vi "Lab Panel V4.7.vi"() -> ()   [LabVIEW 2013]
uses:
  <vilib>/Platform/TimedLoop/XDataNode/timing_clust.ctl
  <vilib>/Platform/TimedLoop/XDataNode/nitl_modes.ctl
  <vilib>/Platform/TimedLoop/XDataNode/wakeup.ctl
  Global 1.vi
  <vilib>/platform/TimedLoop/XDataNode/XDataNode.xnode
  <vilib>/Platform/TimedLoop/XDataNode/XDNodeRunTimeDep.lvlib
panel:
  in  "ADMIN PAGE":bool
  out "TEMP update":bool
  out "AI update":bool
  in  "Tab Control 2":T1(tab)
  out "SIG LAB05-2":T2 {"PF" format="%.2f"; "AMPS" format="%.1f"}
  out "SIG LAB05-1":T2 {"PF" format="%.2f"; "AMPS" format="%.1f"}
  out "SIG LAB04-2":T2 {"PF" format="%.2f"; "AMPS" format="%.1f"}
  out "SIG LAB04-1":T2 {"PF" format="%.2f"; "AMPS" format="%.1f"}
  out "SIG LAB03-2":T2 {"PF" format="%.2f"; "AMPS" format="%.1f"}
  out "SIG LAB03-1":T2 {"PF" format="%.2f"; "AMPS" format="%.1f"}
  out "SIG LAB02-2":T2 {"PF" format="%.2f"; "AMPS" format="%.1f"}
  in  "RUN LAB01-1":bool
  in  "O/I  LAB05-1":bool
  in  "O/I  LAB05-2":bool
  in  "O/I  LAB04-1":bool
  in  "O/I  LAB04-2":bool
  in  "O/I  LAB02-1":bool
  in  "O/I  LAB02-2":bool
  in  "O/I  LAB01-2":bool
  in  "O/I  LAB01-1":bool
  in  "O/I  LAB03-1":bool
  in  "RUN LAB05-2":bool
  in  "RUN LAB05-1":bool
  in  "RUN LAB04-2":bool
  in  "RUN LAB04-1":bool
  in  "RUN LAB03-2":bool
  in  "RUN LAB03-1":bool
  in  "RUN LAB02-2":bool
  in  "RUN LAB02-1":bool
  in  "RUN LAB01-2":bool
  in  "SELECT LAB05-2":T3(radio)
  in  "SELECT LAB05-1":T3(radio)
  in  "SELECT LAB04-2":T3(radio)
  in  "SELECT LAB04-1":T3(radio)
  in  "SELECT LAB03-2":T3(radio)
  in  "SELECT LAB03-1":T3(radio)
  in  "SELECT LAB02-2":T3(radio)
  in  "SELECT LAB02-1":T3(radio)
  in  "SELECT LAB01-2":T3(radio)
  in  "SELECT LAB01-1":T3(radio)
  in  "O/I  LAB03-2":bool
  out "SIG LAB01-1":T2 {"PF" format="%.2f"; "AMPS" format="%.1f"}
  out "SIG LAB01-2":T2 {"PF" format="%.2f"; "AMPS" format="%.1f"}
  out "SIG LAB02-1":T2 {"PF" format="%.2f"; "AMPS" format="%.1f"}
  out "DISP LAB05-2":T4 {"MINS" format="%.2g"}
  out "DISP LAB05-1":T4 {"MINS" format="%.2g"}
  out "DISP LAB04-2":T4 {"MINS" format="%.2g"}
  out "DISP LAB04-1":T4 {"MINS" format="%.2g"}
  out "DISP LAB03-2":T4 {"MINS" format="%.2g"}
  out "DISP LAB03-1":T4 {"MINS" format="%.2g"}
  in  "SET LAB05-2":T5={"NAME"="", "DESCRIPTION"="", "CYCLES"=5.0, "T-RISE mins"=0.0, "T-RISE deg C"=0.0} {"CYCLES" min=5.0 step=1.0}
  in  "SET LAB05-1":T5={"NAME"="", "DESCRIPTION"="", "CYCLES"=5.0, "T-RISE mins"=0.0, "T-RISE deg C"=0.0} {"CYCLES" min=5.0 step=1.0}
  in  "SET LAB04-2":T5={"NAME"="", "DESCRIPTION"="", "CYCLES"=5.0, "T-RISE mins"=0.0, "T-RISE deg C"=0.0} {"CYCLES" min=5.0 step=1.0}
  in  "SET LAB04-1":T5={"NAME"="", "DESCRIPTION"="", "CYCLES"=5.0, "T-RISE mins"=0.0, "T-RISE deg C"=0.0} {"CYCLES" min=5.0 step=1.0}
  in  "SET LAB03-2":T5={"NAME"="", "DESCRIPTION"="", "CYCLES"=5.0, "T-RISE mins"=0.0, "T-RISE deg C"=0.0} {"CYCLES" min=5.0 step=1.0}
  in  "SET LAB03-1":T5={"NAME"="", "DESCRIPTION"="", "CYCLES"=5.0, "T-RISE mins"=0.0, "T-RISE deg C"=0.0} {"CYCLES" min=5.0 step=1.0}
  out "DISP LAB02-2":T4 {"MINS" format="%.2g"}
  out "DISP LAB02-1":T4 {"MINS" format="%.2g"}
  in  "SET LAB02-2":T5={"NAME"="", "DESCRIPTION"="", "CYCLES"=5.0, "T-RISE mins"=0.0, "T-RISE deg C"=0.0} {"CYCLES" min=5.0 step=1.0}
  in  "SET LAB02-1":T5={"NAME"="", "DESCRIPTION"="", "CYCLES"=5.0, "T-RISE mins"=0.0, "T-RISE deg C"=0.0} {"CYCLES" min=5.0 step=1.0}
  out "RESULT LAB05-2":bool
  out "RESULT LAB05-1":bool
  out "RESULT LAB04-2":bool
  out "RESULT LAB04-1":bool
  out "RESULT LAB03-2":bool
  out "RESULT LAB03-1":bool
  out "RESULT LAB02-2":bool
  out "RESULT LAB02-1":bool
  out "RESULT LAB01-2":bool
  out "RESULT LAB01-1":bool
  in  "SET LAB01-1":T5={"NAME"="", "DESCRIPTION"="", "CYCLES"=5.0, "T-RISE mins"=0.0, "T-RISE deg C"=0.0} {"CYCLES" min=5.0 step=1.0}
  in  "SET LAB01-2":T5={"NAME"="", "DESCRIPTION"="", "CYCLES"=5.0, "T-RISE mins"=0.0, "T-RISE deg C"=0.0} {"CYCLES" min=5.0 step=1.0}
  out "DISP LAB01-1":T4 {"MINS" format="%.2g"}
  out "DISP LAB01-2":T4 {"MINS" format="%.2f"}
  out "TEMP RISE LAB05-2":cluster{"TL":dbl, "TN":dbl}
  out "TEMP RISE LAB05-1":cluster{"TL":dbl, "TN":dbl}
  out "TEMP RISE LAB04-2":cluster{"TL":dbl, "TN":dbl}
  out "TEMP RISE LAB04-1":cluster{"TL":dbl, "TN":dbl}
  out "TEMP RISE LAB03-2":cluster{"TL":dbl, "TN":dbl}
  out "TEMP RISE LAB03-1":cluster{"TL":dbl, "TN":dbl}
  out "TEMP RISE LAB02-2":cluster{"TL":dbl, "TN":dbl}
  out "TEMP RISE LAB02-1":cluster{"TL":dbl, "TN":dbl}
  out "TEMP RISE LAB01-2":cluster{"TL":dbl, "TN":dbl}
  out "TEMP RISE LAB01-1":cluster{"TL":dbl, "TN":dbl}
  in  "JIG OFF TIME (S)":dbl=2.0 min=2.0 max=10.0 step=0.5 format="%.1g"
  in  "JIG ON TIME (S)":dbl=1.0 min=1.0 max=10.0 step=0.5 format="%.1g"
  out "JIG LAB05-2":bool
  out "JIG LAB05-1":bool
  out "JIG LAB04-2":bool
  out "JIG LAB04-1":bool
  out "JIG LAB03-2":bool
  out "JIG LAB03-1":bool
  out "JIG LAB02-2":bool
  out "JIG LAB02-1":bool
  out "JIG LAB01-2":bool
  out "JIG LAB01-1":bool
  out "TEMP START LAB01-1":cluster{"TL":dbl, "TN":dbl}
  out "TEMP START LAB02-1":cluster{"TL":dbl, "TN":dbl}
  out "TEMP START LAB03-1":cluster{"TL":dbl, "TN":dbl}
  out "TEMP START LAB04-1":cluster{"TL":dbl, "TN":dbl}
  out "TEMP START LAB01-2":cluster{"TL":dbl, "TN":dbl}
  out "TEMP START LAB02-2":cluster{"TL":dbl, "TN":dbl}
  out "TEMP START LAB03-2":cluster{"TL":dbl, "TN":dbl}
  out "TEMP START LAB04-2":cluster{"TL":dbl, "TN":dbl}
  out "TEMP START LAB05-2":cluster{"TL":dbl, "TN":dbl}
  out "TEMP START LAB05-1":cluster{"TL":dbl, "TN":dbl}
  out "TEST VOLTS CHART":T6(graph)
  in  "Select  Cycle":enum32{"ON CYCLE", "OFF CYCLE"}(radio)
  out "TEST AMPS CHART":T6(graph)
  out "TEMPERATURE (N) CHART":T6(graph)
  out "TEMPERATURE (L) CHART":T6(graph)
  out "Message":string
  in  "MAIL SETTINGS":T7
  out "MAIL REPORT":string
  in  "TO (string):":string
  in  "Send Mail Now":bool
  in  "Auto Mail Send":bool
  in  "Network Directory":path
  out "CAL LAB01":T8 {"2 (TN) cal" min=0.0 step=0.01 format="%.2f"; "2 (TL) cal" min=0.0 step=0.01 format="%.2f"; "2 (PF) cal" min=0.0 step=0.01 format="%.2f"; "2 (V) cal" min=0.0 step=0.01 format="%.2f"; "2 (A) cal" min=0.0 step=0.01 format="%.2f"; "1 (TN) cal" min=0.0 step=0.01 format="%.2f"; "1 (TL) cal" min=0.0 step=0.01 format="%.2f"; "1 (PF) cal" min=0.0 step=0.01 format="%.2f"; "1 (V) cal" min=0.0 step=0.01 format="%.2f"; "1  (A) cal" min=0.0 step=0.01 format="%.2f"}
  out "CAL LAB03":T8 {"2 (TN) cal" min=0.0 step=0.01 format="%.2f"; "2 (TL) cal" min=0.0 step=0.01 format="%.2f"; "2 (PF) cal" min=0.0 step=0.01 format="%.2f"; "2 (V) cal" min=0.0 step=0.01 format="%.2f"; "2 (A) cal" min=0.0 step=0.01 format="%.2f"; "1 (TN) cal" min=0.0 step=0.01 format="%.2f"; "1 (TL) cal" min=0.0 step=0.01 format="%.2f"; "1 (PF) cal" min=0.0 step=0.01 format="%.2f"; "1 (V) cal" min=0.0 step=0.01 format="%.2f"; "1  (A) cal" min=0.0 step=0.01 format="%.2f"}
  out "CAL LAB02":T9 {"2 (TN) cal" min=0.0 step=0.01 format="%.2f"; "2 (TL) cal" min=0.0 step=0.01 format="%.2f"; "2 (PF) cal" min=0.0 step=0.01 format="%.2f"; "2 (V) cal" min=0.0 step=0.01 format="%.2f"; "2 (A) cal" min=0.0 step=0.01 format="%.2f"; "1 (TN) cal" min=0.0 step=0.01 format="%.2f"; "1 (TL) cal" min=0.0 step=0.01 format="%.2f"; "1 (PF) cal" min=0.0 step=0.01 format="%.2f"; "1 (V) cal" min=0.0 step=0.01 format="%.2f"; "1 (A) cal" min=0.0 step=0.01 format="%.2f"}
  out "CAL LAB05":T8 {"2 (TN) cal" min=0.0 step=0.01 format="%.2f"; "2 (TL) cal" min=0.0 step=0.01 format="%.2f"; "2 (PF) cal" min=0.0 step=0.01 format="%.2f"; "2 (V) cal" min=0.0 step=0.01 format="%.2f"; "2 (A) cal" min=0.0 step=0.01 format="%.2f"; "1 (TN) cal" min=0.0 step=0.01 format="%.2f"; "1 (TL) cal" min=0.0 step=0.01 format="%.2f"; "1 (PF) cal" min=0.0 step=0.01 format="%.2f"; "1 (V) cal" min=0.0 step=0.01 format="%.2f"; "1  (A) cal" min=0.0 step=0.01 format="%.2f"}
  out "CAL LAB04":T8 {"2 (TN) cal" min=0.0 step=0.01 format="%.2f"; "2 (TL) cal" min=0.0 step=0.01 format="%.2f"; "2 (PF) cal" min=0.0 step=0.01 format="%.2f"; "2 (V) cal" min=0.0 step=0.01 format="%.2f"; "2 (A) cal" min=0.0 step=0.01 format="%.2f"; "1 (TN) cal" min=0.0 step=0.01 format="%.2f"; "1 (TL) cal" min=0.0 step=0.01 format="%.2f"; "1 (PF) cal" min=0.0 step=0.01 format="%.2f"; "1 (V) cal" min=0.0 step=0.01 format="%.2f"; "1  (A) cal" min=0.0 step=0.01 format="%.2f"}
  out "calibration file error out":errorcluster
  in  "CALIBRATE":bool
  out "ON L05-2":cluster{"amps":dbl, "volts":dbl, "pf":dbl}
  out "ON L05-1":cluster{"amps":dbl, "volts":dbl, "pf":dbl}
  out "FAIL LAB05-2":cluster{"LO":dbl, "HI":dbl}
  out "FAIL LAB05-1":cluster{"LO":dbl, "HI":dbl}
  out "FAIL LAB04-2":cluster{"LO":dbl, "HI":dbl}
  out "FAIL LAB04-1":cluster{"LO":dbl, "HI":dbl}
  out "FAIL LAB03-2":cluster{"LO":dbl, "HI":dbl}
  out "FAIL LAB03-1":cluster{"LO":dbl, "HI":dbl}
  out "FAIL LAB02-2":cluster{"LO":dbl, "HI":dbl}
  out "FAIL LAB02-1":cluster{"LO":dbl, "HI":dbl}
  out "FAIL LAB01-2":cluster{"LO":dbl, "HI":dbl}
  out "FAIL LAB01-1":cluster{"LO":dbl, "HI":dbl}
  out "ON L01-1":cluster{"amps":dbl, "volts":dbl, "pf":dbl}
  out "ON L01-2":cluster{"amps":dbl, "volts":dbl, "pf":dbl}
  out "ON L02-1":cluster{"amps":dbl, "volts":dbl, "pf":dbl}
  out "ON L02-2":cluster{"amps":dbl, "volts":dbl, "pf":dbl}
  out "ON L03-1":cluster{"amps":dbl, "volts":dbl, "pf":dbl}
  out "ON L03-2":cluster{"amps":dbl, "volts":dbl, "pf":dbl}
  out "ON L04-1":cluster{"amps":dbl, "volts":dbl, "pf":dbl}
  out "ON L04-2":cluster{"amps":dbl, "volts":dbl, "pf":dbl}
  out "TEMP LA05":T10
  out "TEMP LA04":T10
  out "TEMP LA03":T10
  out "TEMP LA02":T10
  out "TEMP LA01":T10
  in  "Temp Value":dbl
  in  "Temp Delay Lps":dbl
  in  "SAMPLES":dbl
  in  "RATE (Hz)":dbl
  in  "JIG TEST":T11
  in  "C drive data root dir":path
  out "run lab05-2":bool
  out "run lab05-1":bool
  out "run lab04-2":bool
  out "run lab04-1":bool
  out "run lab03-2":bool
  out "run lab03-1":bool
  out "run lab02-2":bool
  out "run lab02-1":bool
  out "run lab01-2":bool
  out "run lab01-1":bool
  out "stop2":bool
  in  "Tab Control":T12(tab)
  out "LAB01-2 (GRAPH)":dynamicdata(graph)
  out "LAB01-1 (GRAPH)":dynamicdata(graph)
  out "LAB02-2 (GRAPH)":dynamicdata(graph)
  out "LAB02-1 (GRAPH)":dynamicdata(graph)
  out "LAB03-2 (GRAPH)":dynamicdata(graph)
  out "LAB03-1 (GRAPH)":dynamicdata(graph)
  out "LAB04-2 (GRAPH)":dynamicdata(graph)
  out "LAB04-1 (GRAPH)":dynamicdata(graph)
  out "LAB05-2 (GRAPH)":dynamicdata(graph)
  out "LAB05-1 (GRAPH)":dynamicdata(graph)
  out "LAB05 TEMP":T13
  out "LAB04 TEMP":T13
  out "LAB02 TEMP":T13
  out "LAB01 TEMP":T13
  out "LAB03 TEMP":T13
  out "Analog Error Array":errorcluster[](array[cluster])
  out "AI loop time":dbl format="%.6g"
  out "loops":dbl
  in  "loop  delay(mS)":dbl
  out "on loops":dbl
  out "off loops":dbl
  out "jig cycle":dbl
  out "TDMS LAB01-1":refnum<k34>
  out "data file error":errorcluster
  out "TDMS LAB02-1":refnum<k34>
  out "TDMS LAB01-2":refnum<k34>
  out "TDMS LAB02-2":refnum<k34>
  out "TDMS LAB03-1":refnum<k34>
  out "TDMS LAB03-2":refnum<k34>
  out "TDMS LAB04-1":refnum<k34>
  out "TDMS LAB04-2":refnum<k34>
  out "TDMS LAB05-1":refnum<k34>
  out "TDMS LAB05-2":refnum<k34>
  out "mail control":string
  out "File Time Stamp":timestamp
  in  "stop":bool
  in  "Select COM port":refnum<visa-resource-name>="COM6"
  out "COM port":refnum<visa-resource-name>="COM6"
  # "LAB01"
  # "LAB02"
  # "LAB05"
  # "LAB03"
  # "LAB04"
  # "LAB01"
  # "LAB02"
  # "LAB03"
  # "LAB04"
  # "LAB05"
  # "JIG SET"
  # "(Enter recipients address seperated by comma)"
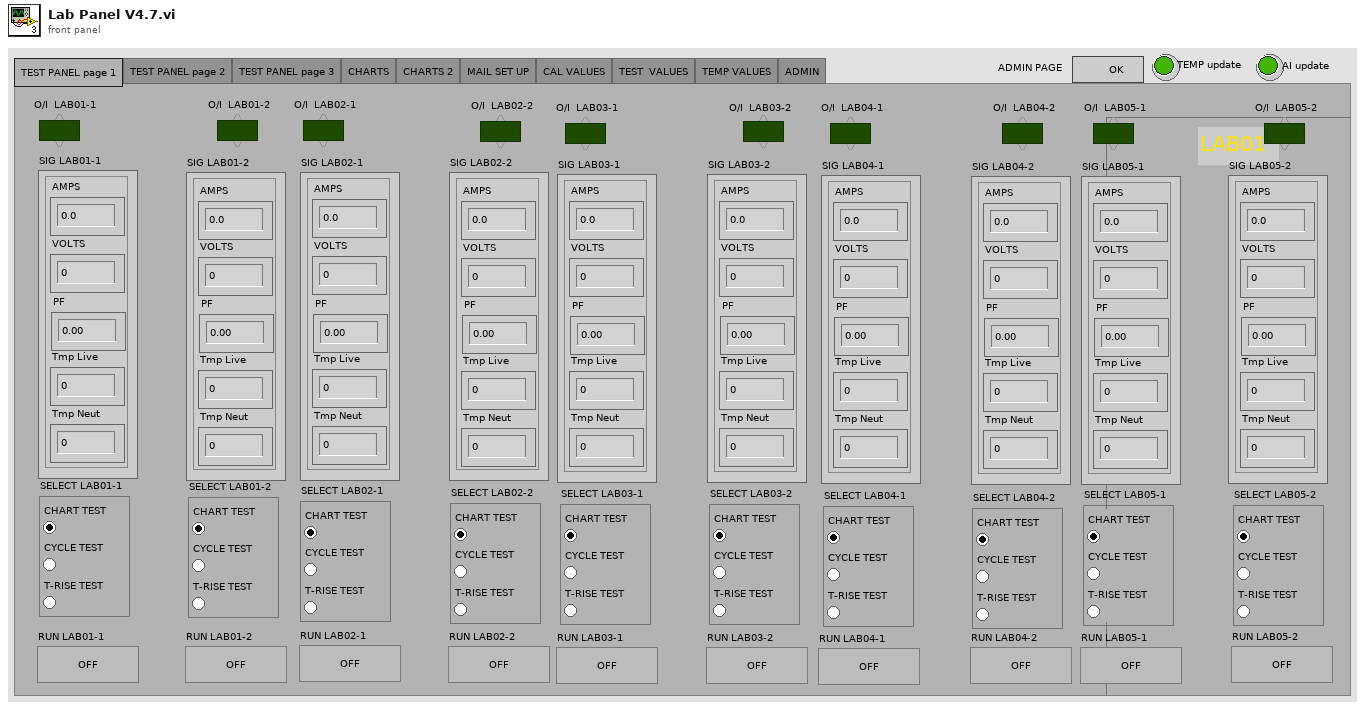
[diagram p1: front panel]
types:
  T1 = enum32{"TEST PANEL page 1", "TEST PANEL page 2", "TEST PANEL page 3", "CHARTS", "CHARTS 2", "MAIL SET UP", "CAL VALUES", "TEST  VALUES", "TEMP VALUES", "ADMIN"}
  T2 = cluster{"AMPS":dbl, "VOLTS":dbl, "PF":dbl, "Tmp Live":dbl, "Tmp Neut":dbl}
  T3 = enum32{"CHART TEST", "CYCLE TEST", "T-RISE TEST"}
  T4 = cluster{"CYCLE":dbl, "MINS":dbl, "STATUS":string}
  T5 = cluster{"NAME":string, "DESCRIPTION":string, "CYCLES":dbl, "T-RISE mins":dbl, "T-RISE deg C":dbl}
  T6 = cluster{"AMPS":dbl, "AMPS":dbl, "AMPS":dbl, "AMPS":dbl, "AMPS":dbl, "AMPS":dbl, "AMPS":dbl, "AMPS":dbl, "AMPS":dbl, "AMPS":dbl}
  T7 = cluster{"OUT SERVER ADDRESS":string, "FROM ACCOUNT":string, "USER NAME":string, "PASSWORD":string, "TEST MAIL":bool, "TEST MAIL STATUS":string, "mail error":errorcluster}
  T8 = cluster{"1  (A) cal":dbl, "1 (V) cal":dbl, "1 (PF) cal":dbl, "1 (TL) cal":dbl, "1 (TN) cal":dbl, "2 (A) cal":dbl, "2 (V) cal":dbl, "2 (PF) cal":dbl, "2 (TL) cal":dbl, "2 (TN) cal":dbl}
  T9 = cluster{"1 (A) cal":dbl, "1 (V) cal":dbl, "1 (PF) cal":dbl, "1 (TL) cal":dbl, "1 (TN) cal":dbl, "2 (A) cal":dbl, "2 (V) cal":dbl, "2 (PF) cal":dbl, "2 (TL) cal":dbl, "2 (TN) cal":dbl}
  T10 = cluster{"TL-1":dbl, "TN-1":dbl, "TL-2":dbl, "TN-2":dbl, "TL -1COUNT":dbl, "TN-1 COUNT":dbl, "TL-2 COUNT":dbl, "TN-2 COUNT":dbl}
  T11 = cluster{" LAB01-1":bool, " LAB01-2":bool, "LAB02-1":bool, " LAB02-2":bool, "LAB03-1":bool, "LAB03-2":bool, "LAB04-1":bool, "LAB04-2":bool, "LAB05-1":bool, "LAB05-2":bool}
  T12 = enum32{"LAB01", "LAB02", "LAB03", "LAB04", "LAB05", "TEMPERATURE", "ERROR"}
  T13 = cluster{"T1 Live":dbl, "T1 Neut":dbl, "T2 Live":dbl, "T2 Neut":dbl, "ID":dbl, "ER":dbl}
  T14 = enum8{"Enabled", "Disabled", "Disabled and Grayed Out"}
  T15 = typedef "XDNodeRunTimeDep.lvlib/timing_clust.ctl" = cluster{"Expected End [f-1]":u64, "Actual End [f-1]":u64, "Finished Late? [f-1]":bool, "Expected End [i-1]":u64, "Actual End [i-1]":u64, "Finished Late? [i-1]":bool, "Expected Start [i]":u64, "Actual Start [i]":u64, "Expected Start [f]":u64, "Actual Start [f]":u64, "Source Name":string, "Structure Name":string, "Period":i64, "Deadline":i64, "Offset":i64, "Start":i64, "Priority":i32, "Timeout":i32, "Mode":T16, "Wakeup Reason":T17, "Error":errorcluster, "Source Type":string, "Secondary Source Type":string, "Global End Time":u64, "Global Start Time":u64, "Frame Duration":u64, "Iteration Duration":u64, "Assigned CPU":i32, "I/O Scan Engine Mode":u32}
  T16 = typedef "XDNodeRunTimeDep.lvlib/nitl_modes.ctl" = enum32{"No Change", "Process missed periods, maintain original phase", "Discard missed periods, maintain original phase", "Process missed periods, ignore original phase", "Discard missed periods, ignore original phase"}
  T17 = typedef "XDNodeRunTimeDep.lvlib/wakeup.ctl" = enum32{"Normal", "Aborted", "Asynchronous wakeup", "Timing source error", "Timed loop error", "Timeout"}
  T18 = enum16{"open", "open or create", "create or replace", "create", "open (read-only)"}
  T19 = enum16{"open", "replace", "create", "open or create", "replace or create", "replace or create with confirmation"}
  T20 = cluster{"SET LAB01-1":cluster{"NAME":string, "DESCRIPTION":string, "CYCLES":dbl, "T-RISE mins":dbl, "T-RISE deg C":dbl}, "SET LAB01-2":cluster{"NAME":string, "DESCRIPTION":string, "CYCLES":dbl, "T-RISE mins":dbl, "T-RISE deg C":dbl}, "SET LAB02-1":cluster{"NAME":string, "DESCRIPTION":string, "CYCLES":dbl, "T-RISE mins":dbl, "T-RISE deg C":dbl}, "SET LAB02-2":cluster{"NAME":string, "DESCRIPTION":string, "CYCLES":dbl, "T-RISE mins":dbl, "T-RISE deg C":dbl}, "SET LAB03-1":cluster{"NAME":string, "DESCRIPTION":string, "CYCLES":dbl, "T-RISE mins":dbl, "T-RISE deg C":dbl}, "SET LAB03-2":cluster{"NAME":string, "DESCRIPTION":string, "CYCLES":dbl, "T-RISE mins":dbl, "T-RISE deg C":dbl}, "SET LAB04-1":cluster{"NAME":string, "DESCRIPTION":string, "CYCLES":dbl, "T-RISE mins":dbl, "T-RISE deg C":dbl}, "SET LAB04-2":cluster{"NAME":string, "DESCRIPTION":string, "CYCLES":dbl, "T-RISE mins":dbl, "T-RISE deg C":dbl}, "SET LAB05-1":cluster{"NAME":string, "DESCRIPTION":string, "CYCLES":dbl, "T-RISE mins":dbl, "T-RISE deg C":dbl}, "SET LAB05-2":cluster{"NAME":string, "DESCRIPTION":string, "CYCLES":dbl, "T-RISE mins":dbl, "T-RISE deg C":dbl}, "Network Directory":path, "C drive data root dir":path, "RATE (Hz)":dbl, "SAMPLES":dbl, "Select COM port":refnum<visa-resource-name>, "Temp Delay Lps":dbl, "Temp Value":dbl}
  T21 = cluster{"MAIL SETTINGS":cluster{"OUT SERVER ADDRESS":string, "FROM ACCOUNT":string, "USER NAME":string, "PASSWORD":string, "TEST MAIL":bool, "TEST MAIL STATUS":string, "mail error":errorcluster}, "Auto Mail Send":bool, string}
  T22 = cluster{"T1":dbl, "T2":dbl, "T3":dbl, "T4":dbl, "ID":dbl, "ER":dbl}
  T23 = cluster{"TP1-L":dbl, "TP1-N":dbl, "TP2-L":dbl, "TP2-N":dbl, "TP1-L COUNT":dbl, "TP1-N COUNT":dbl, "TP2-L COUNT":dbl, "TP2-N COUNT":dbl}
  T24 = cluster{"LAB01-1 (A)":dbl, "LAB01-1 (V)":dbl, "LAB01-1 (PF)":dbl, "LAB01-2 (A)":dbl, "LAB01-2 (V)":dbl, "LAB01-2 (PF)":dbl}
  T25 = cluster{"LAB02-1 (A)":dbl, "LAB02-1 (V)":dbl, "LAB02-1 (PF)":dbl, "LAB02-2 (A)":dbl, "LAB02-2 (V)":dbl, "LAB02-2 (PF)":dbl}
  T26 = cluster{"LAB03-1 (A)":dbl, "LAB03-1 (V)":dbl, "LAB03-1 (PF)":dbl, "LAB03-2 (A)":dbl, "LAB03-2 (V)":dbl, "LAB03-2 (PF)":dbl}
  T27 = cluster{"LAB04-1 (A)":dbl, "LAB04-1 (V)":dbl, "LAB04-1 (PF)":dbl, "LAB04-2 (A)":dbl, "LAB04-2 (V)":dbl, "LAB04-2 (PF)":dbl}
  T28 = cluster{"LAB05-1 (A)":dbl, "LAB05-1 (V)":dbl, "LAB05-1 (PF)":dbl, "LAB05-2 (A)":dbl, "LAB05-2 (V)":dbl, "LAB05-2 (PF)":dbl}
  T29 = cluster{"VOLTS":dbl, "VOLTS":dbl, "VOLTS":dbl, "VOLTS":dbl, "VOLTS":dbl, "VOLTS":dbl, "VOLTS":dbl, "VOLTS":dbl, "VOLTS":dbl, "VOLTS":dbl}
  T30 = cluster{"Tmp Live":dbl, "Tmp Live":dbl, "Tmp Live":dbl, "Tmp Live":dbl, "Tmp Live":dbl, "Tmp Live":dbl, "Tmp Live":dbl, "Tmp Live":dbl, "Tmp Live":dbl, "Tmp Live":dbl}
  T31 = cluster{"Tmp Neut":dbl, "Tmp Neut":dbl, "Tmp Neut":dbl, "Tmp Neut":dbl, "Tmp Neut":dbl, "Tmp Neut":dbl, "Tmp Neut":dbl, "Tmp Neut":dbl, "Tmp Neut":dbl, "Tmp Neut":dbl}
  T32 = cluster{"FAIL LAB01-1":cluster{"LO":dbl, "HI":dbl}, "SIG LAB01-1":cluster{"AMPS":dbl, "VOLTS":dbl, "PF":dbl, "Tmp Live":dbl, "Tmp Neut":dbl}, "TEMP START LAB01-1":cluster{"TL":dbl, "TN":dbl}, "DISP LAB01-1":cluster{"CYCLE":dbl, "MINS":dbl, "STATUS":string}, "SET LAB01-1":cluster{"NAME":string, "DESCRIPTION":string, "CYCLES":dbl, "T-RISE mins":dbl, "T-RISE deg C":dbl}, "TDMS LAB01-1":refnum<k34>}
  T33 = cluster{"FAIL LAB01-2":cluster{"LO":dbl, "HI":dbl}, "SIG LAB01-2":cluster{"AMPS":dbl, "VOLTS":dbl, "PF":dbl, "Tmp Live":dbl, "Tmp Neut":dbl}, "TEMP START LAB01-2":cluster{"TL":dbl, "TN":dbl}, "DISP LAB01-2":cluster{"CYCLE":dbl, "MINS":dbl, "STATUS":string}, "SET LAB01-2":cluster{"NAME":string, "DESCRIPTION":string, "CYCLES":dbl, "T-RISE mins":dbl, "T-RISE deg C":dbl}, "TDMS LAB01-2":refnum<k34>}
  T34 = cluster{"FAIL LAB02-1":cluster{"LO":dbl, "HI":dbl}, "SIG LAB02-1":cluster{"AMPS":dbl, "VOLTS":dbl, "PF":dbl, "Tmp Live":dbl, "Tmp Neut":dbl}, "TEMP START LAB02-1":cluster{"TL":dbl, "TN":dbl}, "DISP LAB02-1":cluster{"CYCLE":dbl, "MINS":dbl, "STATUS":string}, "SET LAB02-1":cluster{"NAME":string, "DESCRIPTION":string, "CYCLES":dbl, "T-RISE mins":dbl, "T-RISE deg C":dbl}, "TDMS LAB02-1":refnum<k34>}
  T35 = cluster{"FAIL LAB02-2":cluster{"LO":dbl, "HI":dbl}, "SIG LAB02-2":cluster{"AMPS":dbl, "VOLTS":dbl, "PF":dbl, "Tmp Live":dbl, "Tmp Neut":dbl}, "TEMP START LAB02-2":cluster{"TL":dbl, "TN":dbl}, "DISP LAB02-2":cluster{"CYCLE":dbl, "MINS":dbl, "STATUS":string}, "SET LAB02-2":cluster{"NAME":string, "DESCRIPTION":string, "CYCLES":dbl, "T-RISE mins":dbl, "T-RISE deg C":dbl}, "TDMS LAB02-2":refnum<k34>}
  T36 = cluster{"FAIL LAB03-1":cluster{"LO":dbl, "HI":dbl}, "SIG LAB03-1":cluster{"AMPS":dbl, "VOLTS":dbl, "PF":dbl, "Tmp Live":dbl, "Tmp Neut":dbl}, "TEMP START LAB03-1":cluster{"TL":dbl, "TN":dbl}, "DISP LAB03-1":cluster{"CYCLE":dbl, "MINS":dbl, "STATUS":string}, "SET LAB03-1":cluster{"NAME":string, "DESCRIPTION":string, "CYCLES":dbl, "T-RISE mins":dbl, "T-RISE deg C":dbl}, "TDMS LAB03-1":refnum<k34>}
  T37 = cluster{"FAIL LAB03-2":cluster{"LO":dbl, "HI":dbl}, "SIG LAB03-2":cluster{"AMPS":dbl, "VOLTS":dbl, "PF":dbl, "Tmp Live":dbl, "Tmp Neut":dbl}, "TEMP START LAB03-2":cluster{"TL":dbl, "TN":dbl}, "DISP LAB03-2":cluster{"CYCLE":dbl, "MINS":dbl, "STATUS":string}, "SET LAB03-2":cluster{"NAME":string, "DESCRIPTION":string, "CYCLES":dbl, "T-RISE mins":dbl, "T-RISE deg C":dbl}, "TDMS LAB03-2":refnum<k34>}
  T38 = cluster{"FAIL LAB04-1":cluster{"LO":dbl, "HI":dbl}, "SIG LAB04-1":cluster{"AMPS":dbl, "VOLTS":dbl, "PF":dbl, "Tmp Live":dbl, "Tmp Neut":dbl}, "TEMP START LAB04-1":cluster{"TL":dbl, "TN":dbl}, "DISP LAB04-1":cluster{"CYCLE":dbl, "MINS":dbl, "STATUS":string}, "SET LAB04-1":cluster{"NAME":string, "DESCRIPTION":string, "CYCLES":dbl, "T-RISE mins":dbl, "T-RISE deg C":dbl}, "TDMS LAB04-1":refnum<k34>}
  T39 = cluster{"FAIL LAB04-2":cluster{"LO":dbl, "HI":dbl}, "SIG LAB04-2":cluster{"AMPS":dbl, "VOLTS":dbl, "PF":dbl, "Tmp Live":dbl, "Tmp Neut":dbl}, "TEMP START LAB04-2":cluster{"TL":dbl, "TN":dbl}, "DISP LAB04-2":cluster{"CYCLE":dbl, "MINS":dbl, "STATUS":string}, "SET LAB04-2":cluster{"NAME":string, "DESCRIPTION":string, "CYCLES":dbl, "T-RISE mins":dbl, "T-RISE deg C":dbl}, "TDMS LAB04-2":refnum<k34>}
  T40 = cluster{"FAIL LAB05-1":cluster{"LO":dbl, "HI":dbl}, "SIG LAB05-1":cluster{"AMPS":dbl, "VOLTS":dbl, "PF":dbl, "Tmp Live":dbl, "Tmp Neut":dbl}, "TEMP START LAB05-1":cluster{"TL":dbl, "TN":dbl}, "DISP LAB05-1":cluster{"CYCLE":dbl, "MINS":dbl, "STATUS":string}, "SET LAB05-1":cluster{"NAME":string, "DESCRIPTION":string, "CYCLES":dbl, "T-RISE mins":dbl, "T-RISE deg C":dbl}, "TDMS LAB05-1":refnum<k34>}
  T41 = cluster{"FAIL LAB05-2":cluster{"LO":dbl, "HI":dbl}, "SIG LAB05-2":cluster{"AMPS":dbl, "VOLTS":dbl, "PF":dbl, "Tmp Live":dbl, "Tmp Neut":dbl}, "TEMP START LAB05-2":cluster{"TL":dbl, "TN":dbl}, "DISP LAB05-2":cluster{"CYCLE":dbl, "MINS":dbl, "STATUS":string}, "SET LAB05-2":cluster{"NAME":string, "DESCRIPTION":string, "CYCLES":dbl, "T-RISE mins":dbl, "T-RISE deg C":dbl}, "TDMS LAB05-2":refnum<k34>}
  T42 = cluster{"MAIL SETTINGS":cluster{"OUT SERVER ADDRESS":string, "FROM ACCOUNT":string, "USER NAME":string, "PASSWORD":string, "TEST MAIL":bool, "TEST MAIL STATUS":string, "mail error":errorcluster}, "Auto Mail Send":bool, "TO (string):":string}
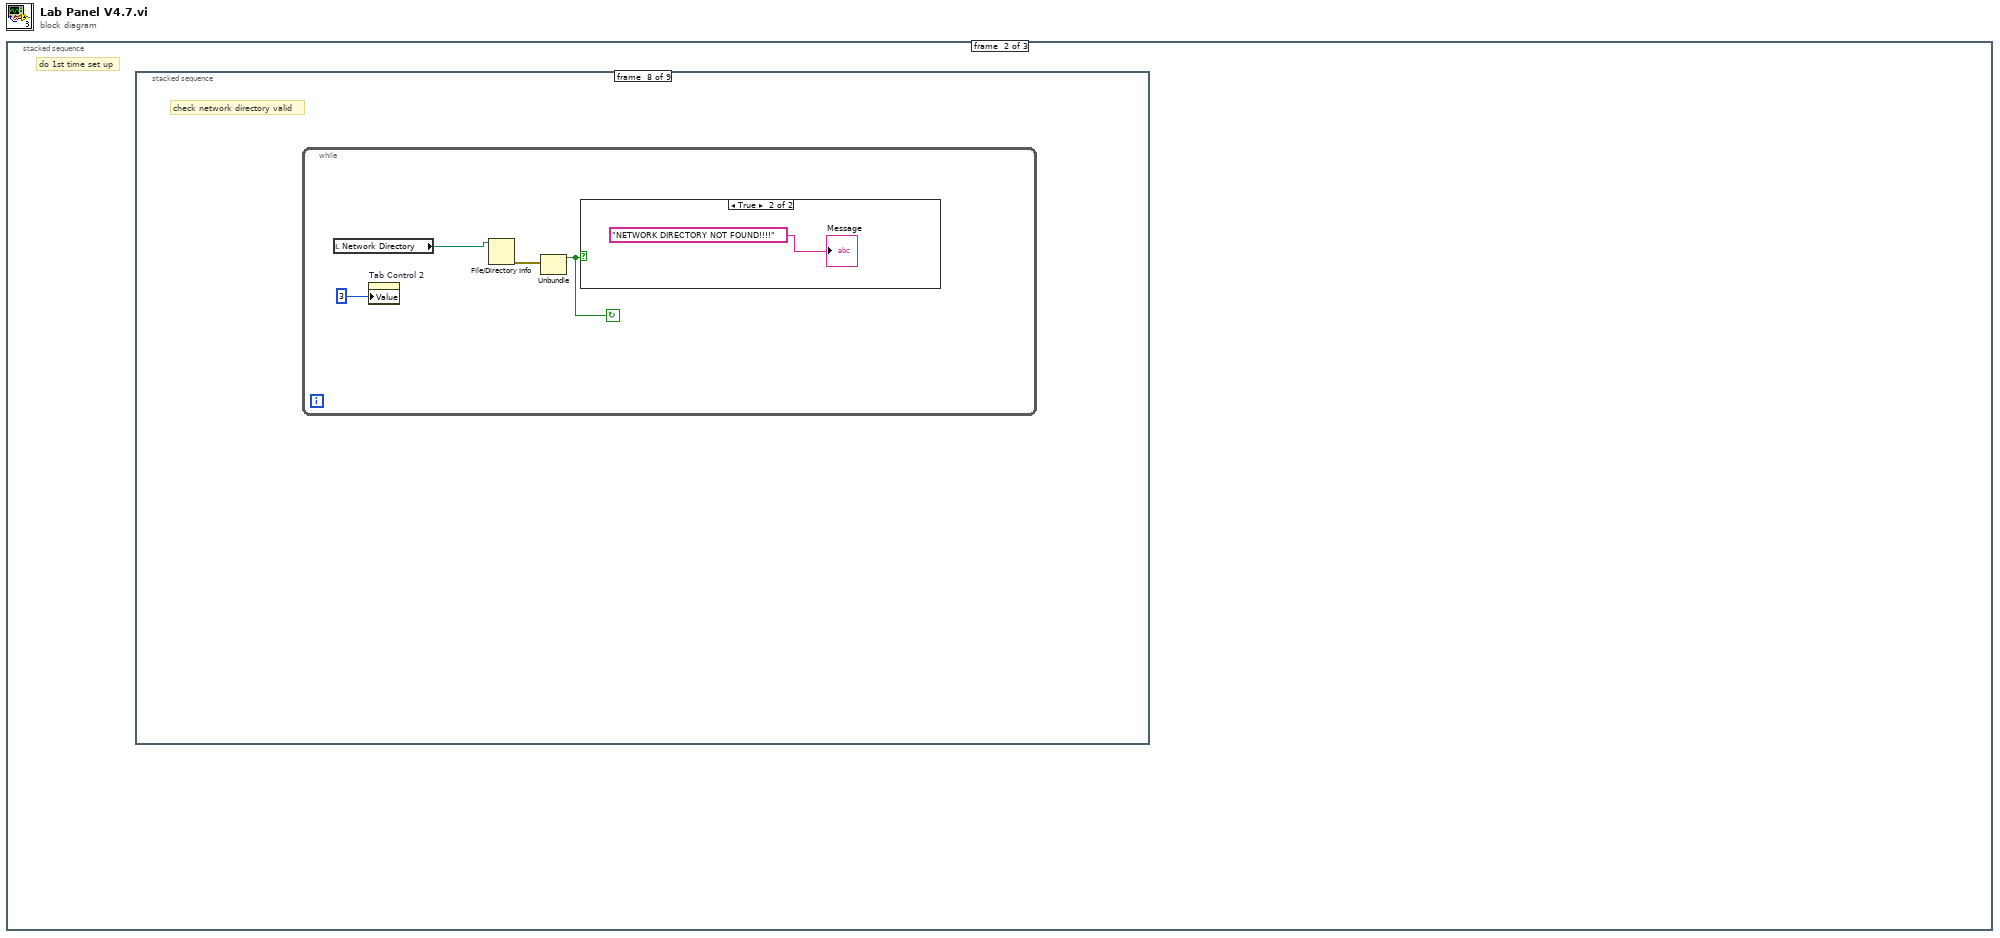
[diagram p0: block diagram]
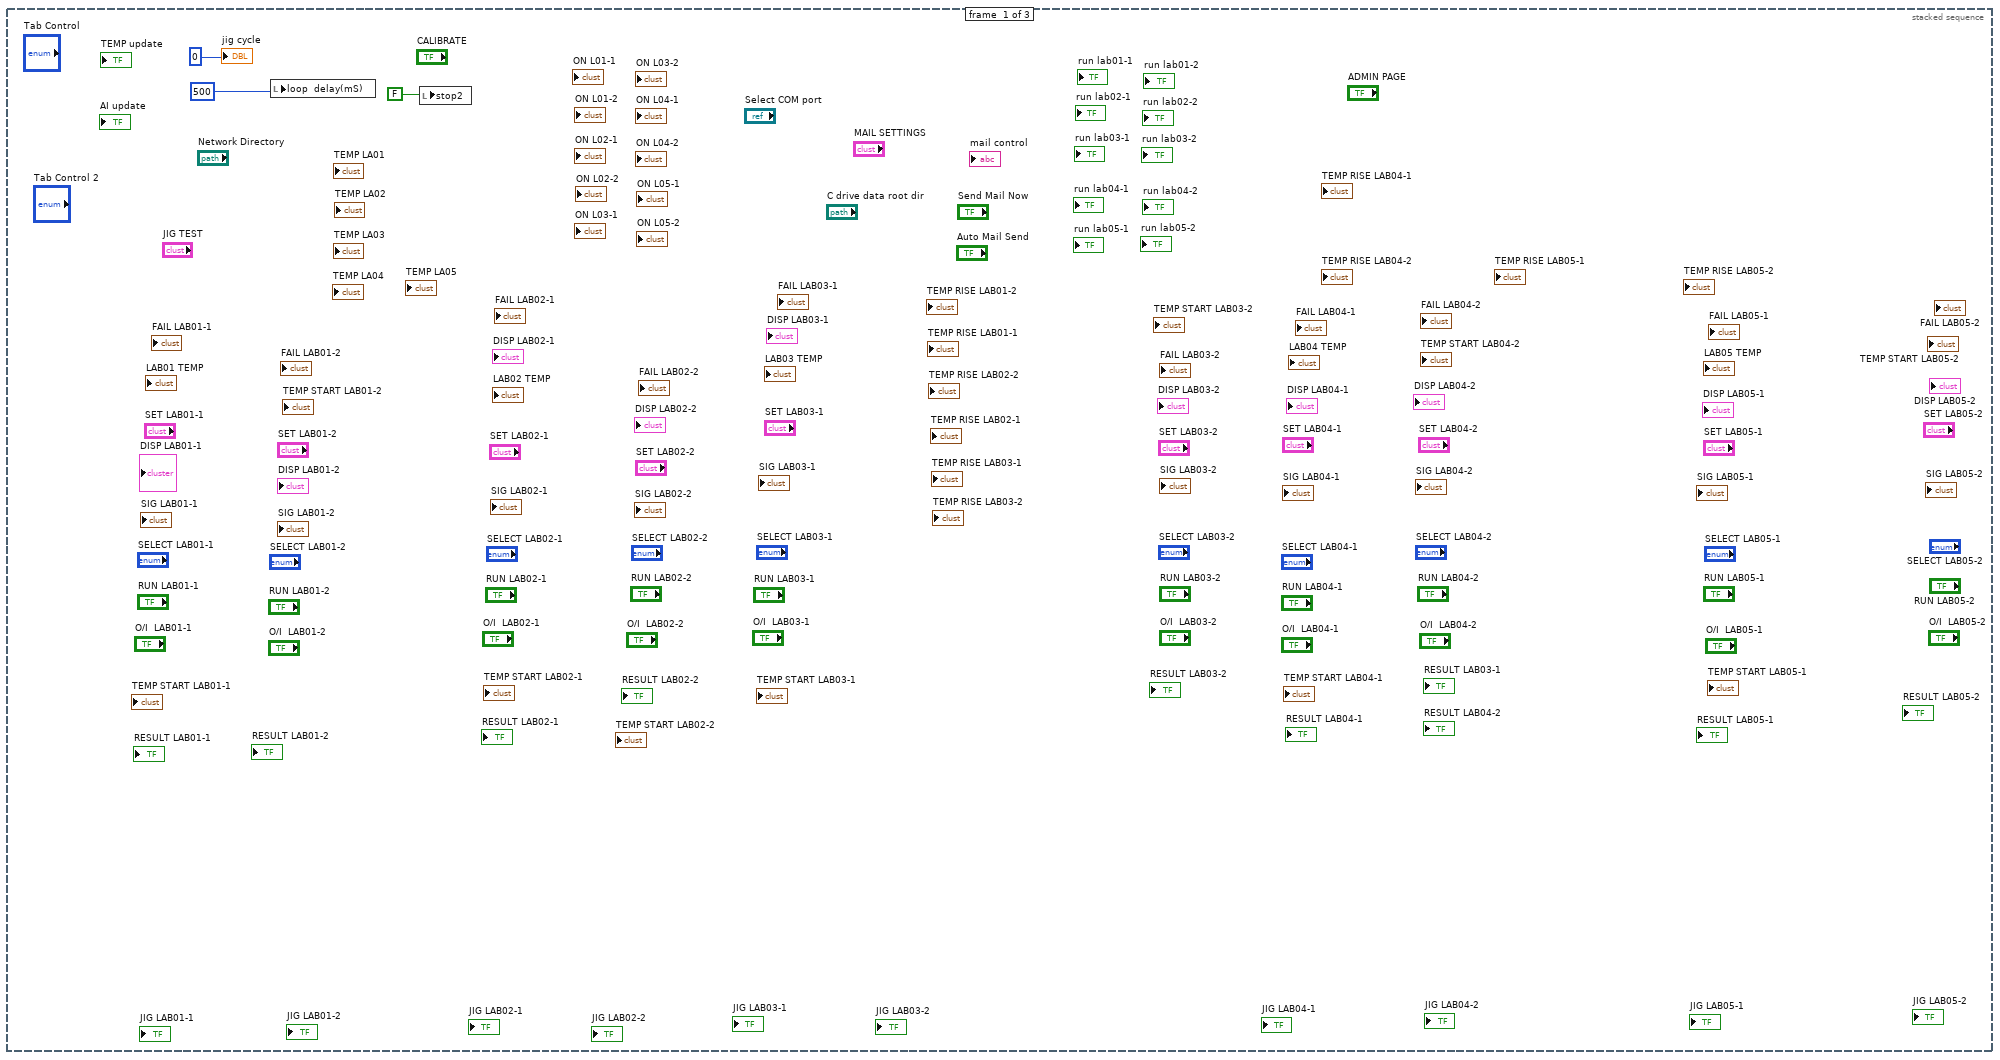
[diagram p2: hidden frame]
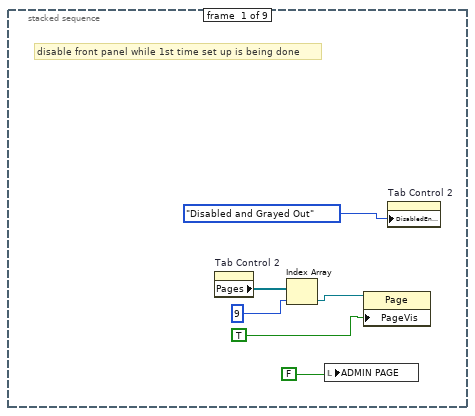
[diagram p3: hidden frame]
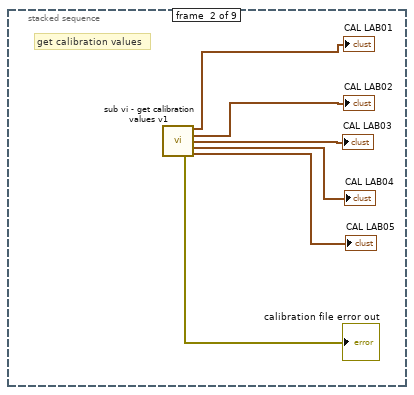
[diagram p4: hidden frame]
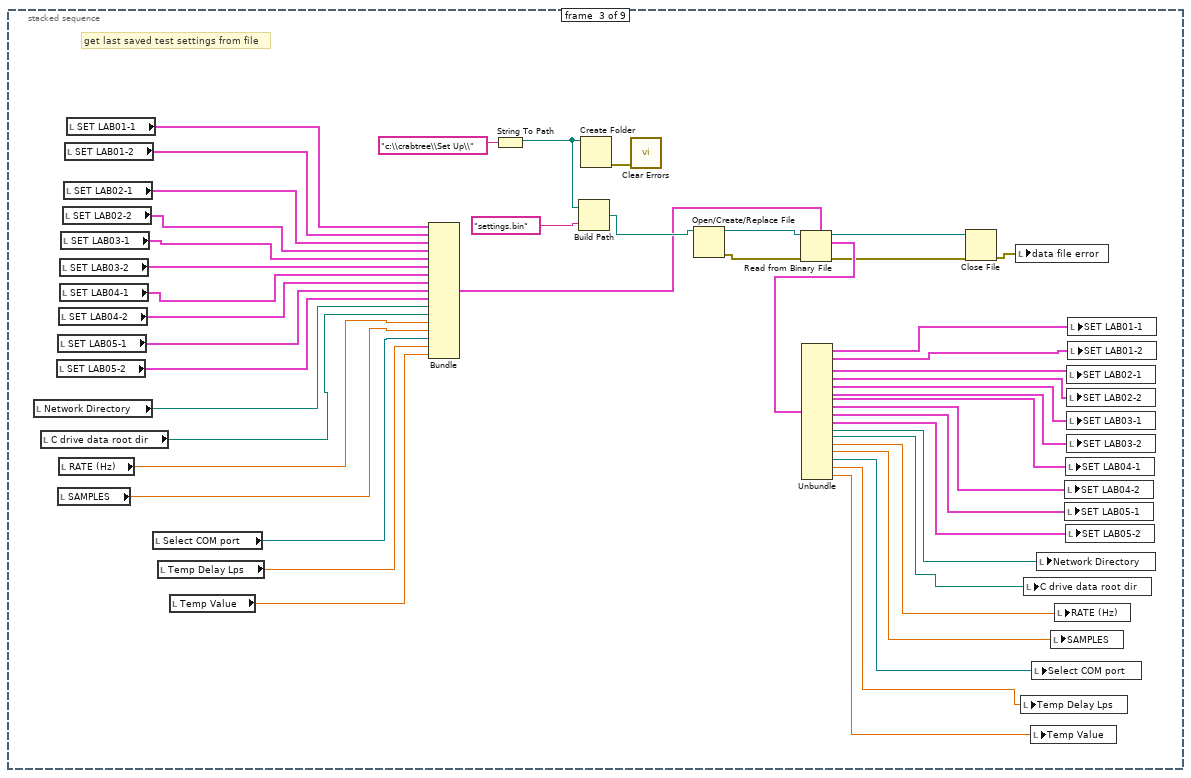
[diagram p5: hidden frame]
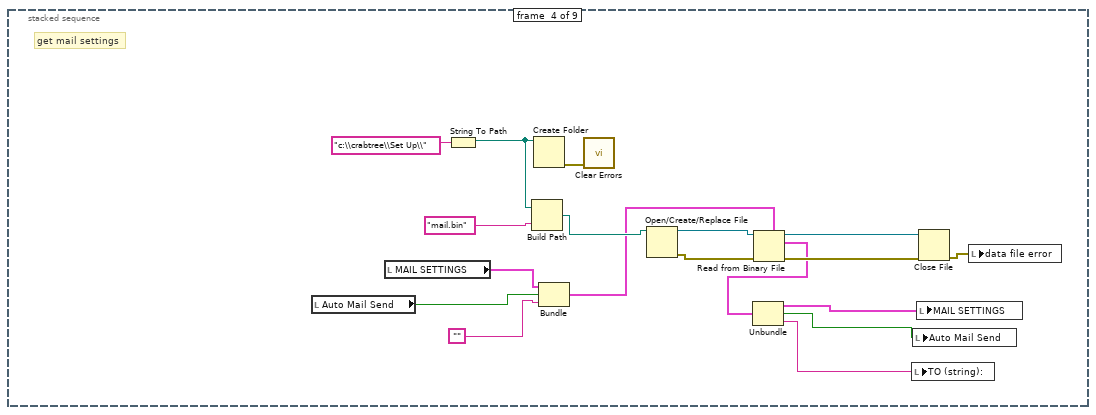
[diagram p6: hidden frame]
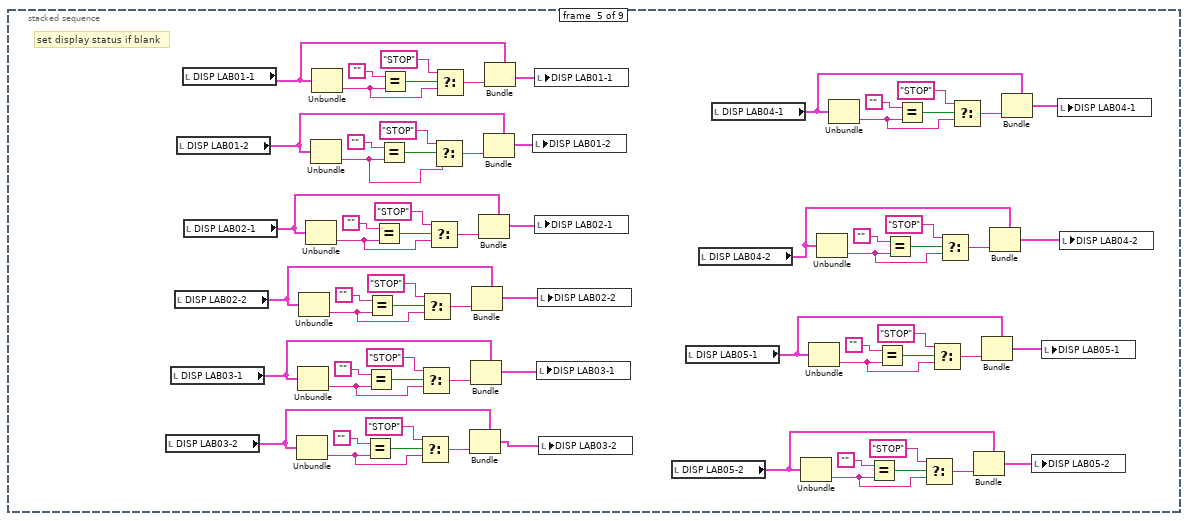
[diagram p7: hidden frame]
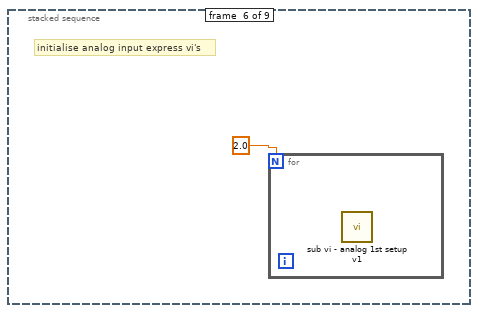
[diagram p8: hidden frame]
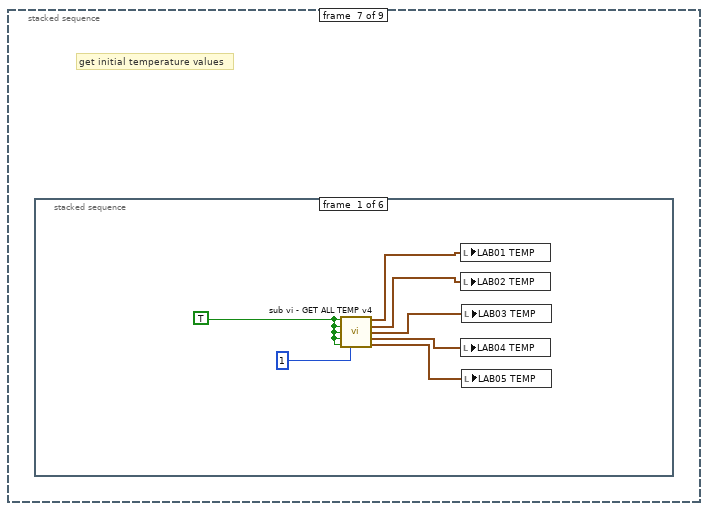
[diagram p9: hidden frame]
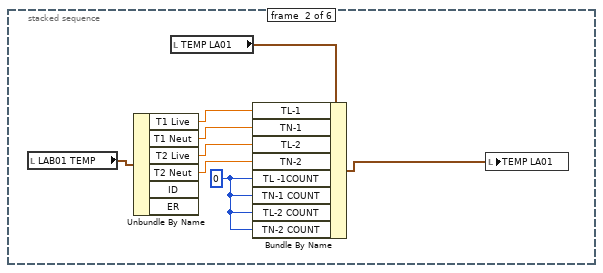
[diagram p10: hidden frame]
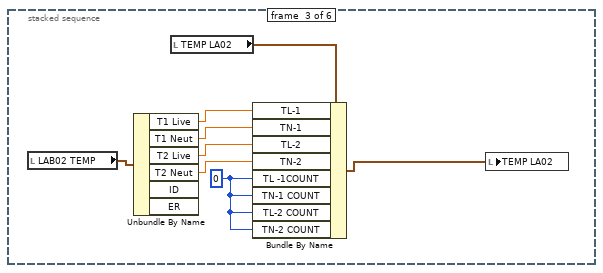
[diagram p11: hidden frame]
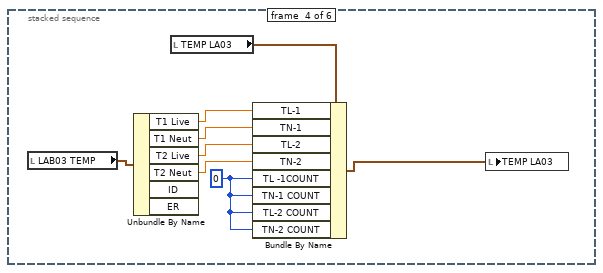
[diagram p12: hidden frame]
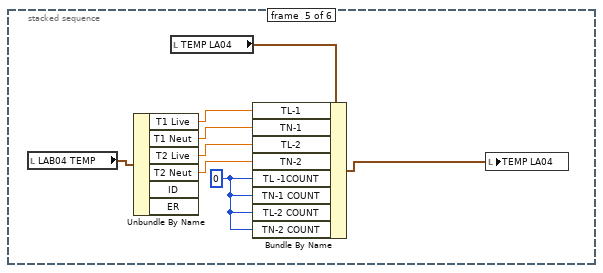
[diagram p13: hidden frame]
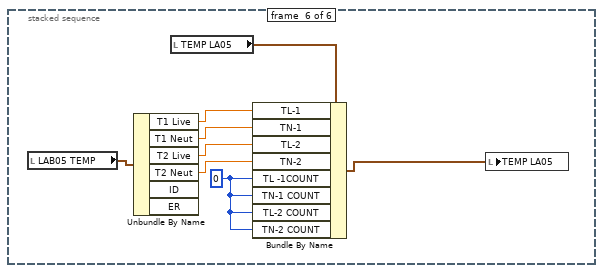
[diagram p14: hidden frame]
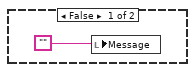
[diagram p15: hidden frame]
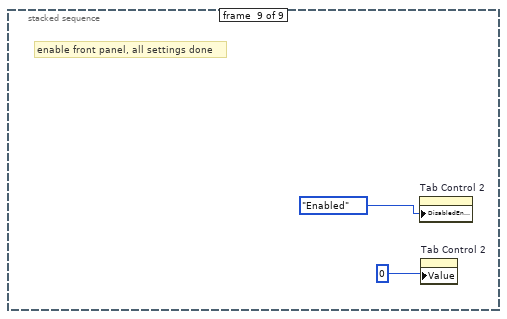
[diagram p16: hidden frame]
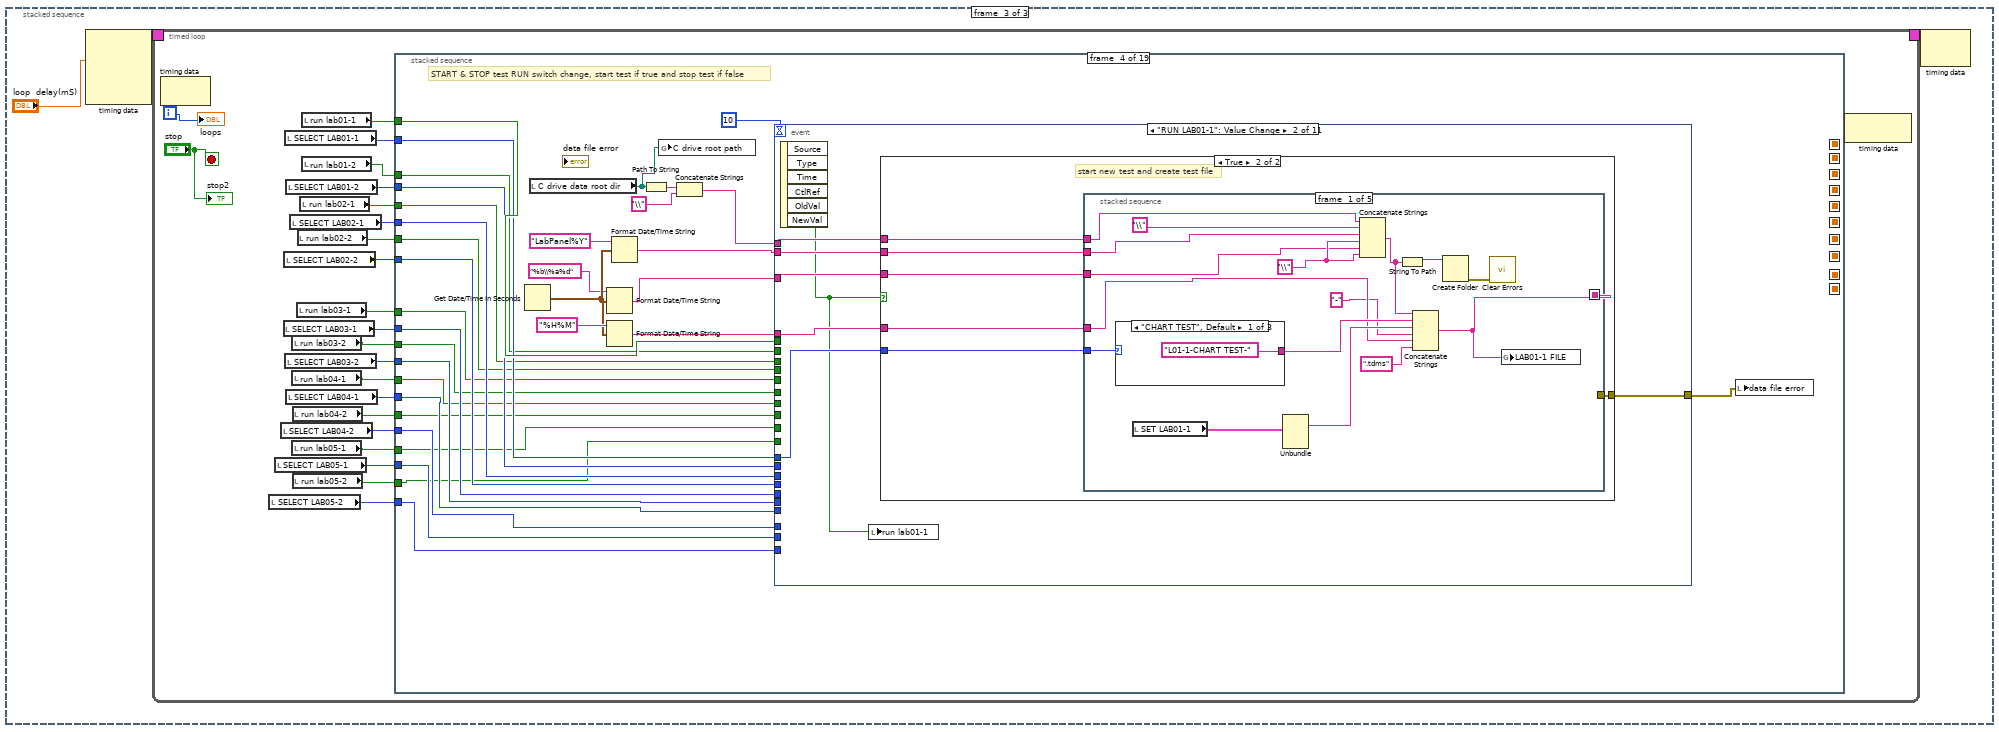
[diagram p17: hidden frame]
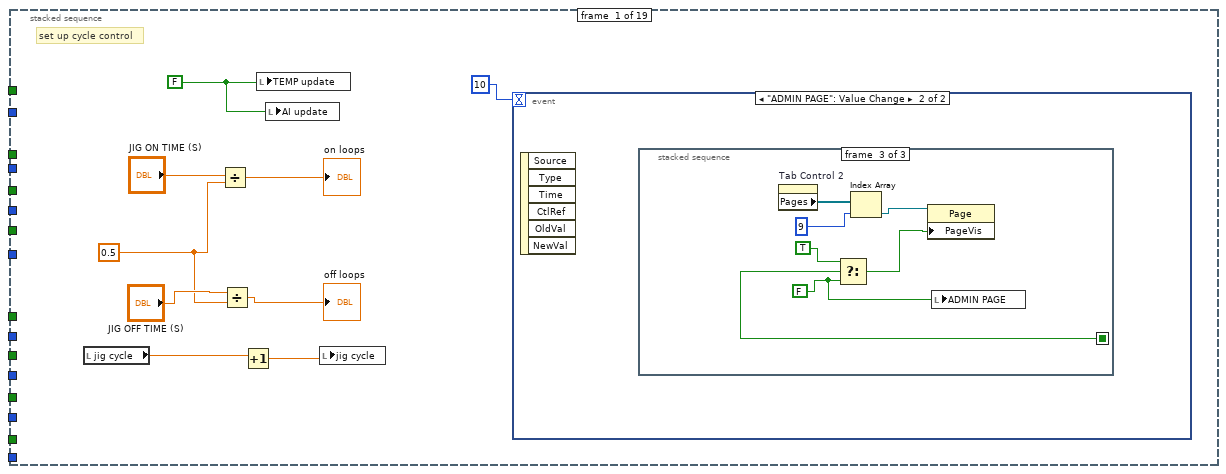
[diagram p18: hidden frame]
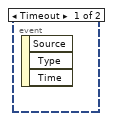
[diagram p19: hidden frame]
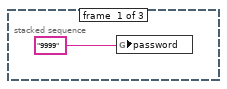
[diagram p20: hidden frame]
diagram:
  n1 = stacked-sequence {
    frame #0 {
      n2 = local write "loop  delay(mS)"(500) -> ()
      n3 = local write "stop2"(FALSE) -> ()
      "jig cycle" <- 0
    }
    frame #1 {
      # "do 1st time set up"
      n4 = stacked-sequence {
        frame #0 {
          # "disable front panel while 1st time set up is being done"
          n5 = property on="Tab Control 2" class="TabCtl (strict)"() -> ("Pages"=w8:refnum<vi>[])  [unwired: 2 in, 2 out]
          n6 = Index Array(array=w8, index=9) -> (element=w6:refnum<vi>)
          n7 = local write "ADMIN PAGE"(FALSE) -> ()
          n8 = property class="Page"(reference=w6, "PageVis"=TRUE) -> ()  [unwired: 1 in, 2 out]
          n9 = property on="Tab Control 2" class="TabCtl (strict)"("DisabledEnum"=T14."Disabled and Grayed Out" ("Disabled")) -> ()  [unwired: 2 in, 2 out]
        }
        frame #1 {
          # "get calibration values"
          n10 = call "sub vi - get calibration values v1.vi"() -> ("LAB01 (CAL)"=→"CAL LAB01":T8, "LAB02 (CAL)"=→"CAL LAB02":T9, "LAB03 (CAL)"=→"CAL LAB03":T8, "LAB04 (CAL)"=→"CAL LAB04":T8, "calibration file error out"=→"calibration file error out":errorcluster, "LAB05 (CAL)"=→"CAL LAB05":T8)  [unwired: 10 in]
        }
        frame #2 {
          # "get last saved test settings from file"
          n11 = local read "Network Directory"() -> (w28:path)
          n12 = local read "C drive data root dir"() -> (w26:path)
          n13 = local read "SET LAB05-2"() -> (w58:T5)
          n14 = local read "SET LAB05-1"() -> (w59:T5)
          n15 = local read "SAMPLES"() -> (w24:dbl)
          n16 = local read "SET LAB04-2"() -> (w60:T5)
          n17 = local read "RATE (Hz)"() -> (w25:dbl)
          n18 = local read "SET LAB03-2"() -> (w57:T5)
          n19 = local read "SET LAB04-1"() -> (w61:T5)
          n20 = local read "SET LAB03-1"() -> (w56:T5)
          n21 = local read "SET LAB02-2"() -> (w55:T5)
          n22 = local read "SET LAB02-1"() -> (w54:T5)
          n23 = local read "SET LAB01-2"() -> (w53:T5)
          n24 = local read "SET LAB01-1"() -> (w52:T5)
          n25 = local read "Select COM port"() -> (w20:refnum<visa-resource-name>)
          n26 = local read "Temp Delay Lps"() -> (w19:dbl)
          n27 = local read "Temp Value"() -> (w18:dbl)
          n28 = Bundle("SET LAB01-1"=w52, "SET LAB01-2"=w53, "SET LAB02-1"=w54, "SET LAB02-2"=w55, "SET LAB03-1"=w56, "SET LAB03-2"=w57, "SET LAB04-1"=w61, "SET LAB04-2"=w60, "SET LAB05-1"=w59, "SET LAB05-2"=w58, "Network Directory"=w28, "C drive data root dir"=w26, "RATE (Hz)"=w25, "SAMPLES"=w24, "Select COM port"=w20, "Temp Delay Lps"=w19, "Temp Value"=w18) -> (w45:T20)  [unwired: 1 in]
          n29 = String To Path(string="c:\\crabtree\\Set Up\\") -> (path=w49:path)
          n30 = Build Path(base path=w49, name or relative path="settings.bin") -> (appended path=w47:path)
          n31 = Create Folder(path (use dialog)=w49) -> (error out=w51:errorcluster)  [unwired: 2 in, 2 out]
          n32 = call <vilib>:"Clear Errors.vi"("error in (no error)"=w51) -> ()  [unwired: 6 in, 1 out]
          n33 = Open/Create/Replace File(file path (use dialog)=w47) -> (refnum out=w44:refnum<file>, error out=w46:errorcluster)  [unwired: 5 in, 1 out]
          n34 = Read from Binary File(5:w45, 8:w46, 11:w44) -> (0:w41:errorcluster, 2:w43:T20, 3:w42:refnum<file>)  [unwired: 3 in, 1 out]
          n35 = Unbundle(w43) -> ("SET LAB01-1"=w39:T5, "SET LAB01-2"=w38:T5, "SET LAB02-1"=w37:T5, "SET LAB02-2"=w36:T5, "SET LAB03-1"=w35:T5, "SET LAB03-2"=w34:T5, "SET LAB04-1"=w33:T5, "SET LAB04-2"=w32:T5, "SET LAB05-1"=w31:T5, "SET LAB05-2"=w30:T5, "Network Directory"=w29:path, "C drive data root dir"=w27:path, "RATE (Hz)"=w22:dbl, "SAMPLES"=w23:dbl, "Select COM port"=w21:refnum<visa-resource-name>, "Temp Delay Lps"=w17:dbl, "Temp Value"=w16:dbl)
          n36 = Close File(refnum=w42, error in=w41) -> (error out=w40:errorcluster)  [unwired: 1 out]
          n37 = local write "data file error"(w40) -> ()
          n38 = local write "Temp Delay Lps"(w17) -> ()
          n39 = local write "C drive data root dir"(w27) -> ()
          n40 = local write "Temp Value"(w16) -> ()
          n41 = local write "Select COM port"(w21) -> ()
          n42 = local write "Network Directory"(w29) -> ()
          n43 = local write "SAMPLES"(w23) -> ()
          n44 = local write "RATE (Hz)"(w22) -> ()
          n45 = local write "SET LAB04-2"(w32) -> ()
          n46 = local write "SET LAB05-1"(w31) -> ()
          n47 = local write "SET LAB04-1"(w33) -> ()
          n48 = local write "SET LAB05-2"(w30) -> ()
          n49 = local write "SET LAB02-1"(w37) -> ()
          n50 = local write "SET LAB02-2"(w36) -> ()
          n51 = local write "SET LAB03-1"(w35) -> ()
          n52 = local write "SET LAB03-2"(w34) -> ()
          n53 = local write "SET LAB01-1"(w39) -> ()
          n54 = local write "SET LAB01-2"(w38) -> ()
        }
        frame #3 {
          # "get mail settings"
          n55 = local read "Auto Mail Send"() -> (w65:bool)
          n56 = local read "MAIL SETTINGS"() -> (w69:T7)
          n57 = String To Path(string="c:\\crabtree\\Set Up\\") -> (path=w77:path)
          n58 = Build Path(base path=w77, name or relative path="mail.bin") -> (appended path=w75:path)
          n59 = Create Folder(path (use dialog)=w77) -> (error out=w79:errorcluster)  [unwired: 2 in, 2 out]
          n60 = Bundle("MAIL SETTINGS"=w69, "Auto Mail Send"=w65, "") -> (w68:T21)  [unwired: 1 in]
          n61 = call <vilib>:"Clear Errors.vi"("error in (no error)"=w79) -> ()  [unwired: 6 in, 1 out]
          n62 = Open/Create/Replace File(file path (use dialog)=w75) -> (refnum out=w73:refnum<file>, error out=w74:errorcluster)  [unwired: 5 in, 1 out]
          n63 = Read from Binary File(5:w68, 8:w74, 11:w73) -> (0:w71:errorcluster, 2:w67:T21, 3:w72:refnum<file>)  [unwired: 3 in, 1 out]
          n64 = Unbundle(w67) -> ("MAIL SETTINGS"=w66:T7, "Auto Mail Send"=w64:bool, w63:string)
          n65 = local write "TO (string):"(w63) -> ()
          n66 = local write "Auto Mail Send"(w64) -> ()
          n67 = local write "MAIL SETTINGS"(w66) -> ()
          n68 = Close File(refnum=w72, error in=w71) -> (error out=w70:errorcluster)  [unwired: 1 out]
          n69 = local write "data file error"(w70) -> ()
        }
        frame #4 {
          # "set display status if blank"
          n70 = local read "DISP LAB03-2"() -> (w109:T4)
          n71 = local read "DISP LAB03-1"() -> (w116:T4)
          n72 = local read "DISP LAB02-2"() -> (w123:T4)
          n73 = local read "DISP LAB01-2"() -> (w136:T4)
          n74 = local read "DISP LAB01-1"() -> (w145:T4)
          n75 = local read "DISP LAB02-1"() -> (w130:T4)
          n76 = Unbundle(w109) -> ("STATUS"=w111:string)  [unwired: 2 out]
          n77 = Unbundle(w116) -> ("STATUS"=w118:string)  [unwired: 2 out]
          n78 = Unbundle(w123) -> ("STATUS"=w125:string)  [unwired: 2 out]
          n79 = Unbundle(w130) -> ("STATUS"=w132:string)  [unwired: 2 out]
          n80 = Unbundle(w136) -> ("STATUS"=w139:string)  [unwired: 2 out]
          n81 = Unbundle(w145) -> ("STATUS"=w146:string)  [unwired: 2 out]
          n82 = Equal?(x="", y=w111) -> (x = y?=w113:bool)
          n83 = Equal?(x="", y=w118) -> (x = y?=w120:bool)
          n84 = Equal?(x="", y=w125) -> (x = y?=w127:bool)
          n85 = Equal?(x="", y=w132) -> (x = y?=w134:bool)
          n86 = Equal?(x="", y=w139) -> (x = y?=w141:bool)
          n87 = Equal?(x="", y=w146) -> (x = y?=w148:bool)
          n88 = Select(t="STOP", s=w113, f=w111) -> (s? t:f=w110:string)
          n89 = Select(t="STOP", s=w120, f=w118) -> (s? t:f=w117:string)
          n90 = Select(t="STOP", s=w127, f=w125) -> (s? t:f=w124:string)
          n91 = Select(t="STOP", s=w134, f=w132) -> (s? t:f=w131:string)
          n92 = Select(t="STOP", s=w141, f=w139) -> (s? t:f=w138:string)
          n93 = Select(t="STOP", s=w148, f=w146) -> (s? t:f=w144:string)
          n94 = Bundle(cluster=w109, "STATUS"=w110) -> (w108:T4)  [unwired: 2 in]
          n95 = Bundle(cluster=w116, "STATUS"=w117) -> (w115:T4)  [unwired: 2 in]
          n96 = Bundle(cluster=w123, "STATUS"=w124) -> (w122:T4)  [unwired: 2 in]
          n97 = Bundle(cluster=w130, "STATUS"=w131) -> (w129:T4)  [unwired: 2 in]
          n98 = Bundle(cluster=w136, "STATUS"=w138) -> (w137:T4)  [unwired: 2 in]
          n99 = Bundle(cluster=w145, "STATUS"=w144) -> (w143:T4)  [unwired: 2 in]
          n100 = local write "DISP LAB01-2"(w137) -> ()
          n101 = local write "DISP LAB01-1"(w143) -> ()
          n102 = local write "DISP LAB02-1"(w129) -> ()
          n103 = local write "DISP LAB03-1"(w115) -> ()
          n104 = local write "DISP LAB02-2"(w122) -> ()
          n105 = local write "DISP LAB03-2"(w108) -> ()
          n106 = local read "DISP LAB05-2"() -> (w81:T4)
          n107 = local read "DISP LAB05-1"() -> (w88:T4)
          n108 = local read "DISP LAB04-2"() -> (w90:T4)
          n109 = local read "DISP LAB04-1"() -> (w92:T4)
          n110 = Unbundle(w81) -> ("STATUS"=w83:string)  [unwired: 2 out]
          n111 = Unbundle(w88) -> ("STATUS"=w94:string)  [unwired: 2 out]
          n112 = Unbundle(w90) -> ("STATUS"=w99:string)  [unwired: 2 out]
          n113 = Unbundle(w92) -> ("STATUS"=w104:string)  [unwired: 2 out]
          n114 = Equal?(x="", y=w83) -> (x = y?=w85:bool)
          n115 = Equal?(x="", y=w94) -> (x = y?=w96:bool)
          n116 = Equal?(x="", y=w99) -> (x = y?=w101:bool)
          n117 = Equal?(x="", y=w104) -> (x = y?=w106:bool)
          n118 = Select(t="STOP", s=w85, f=w83) -> (s? t:f=w82:string)
          n119 = Select(t="STOP", s=w96, f=w94) -> (s? t:f=w93:string)
          n120 = Select(t="STOP", s=w101, f=w99) -> (s? t:f=w98:string)
          n121 = Select(t="STOP", s=w106, f=w104) -> (s? t:f=w103:string)
          n122 = Bundle(cluster=w81, "STATUS"=w82) -> (w80:T4)  [unwired: 2 in]
          n123 = Bundle(cluster=w88, "STATUS"=w93) -> (w87:T4)  [unwired: 2 in]
          n124 = Bundle(cluster=w90, "STATUS"=w98) -> (w89:T4)  [unwired: 2 in]
          n125 = Bundle(cluster=w92, "STATUS"=w103) -> (w91:T4)  [unwired: 2 in]
          n126 = local write "DISP LAB05-2"(w80) -> ()
          n127 = local write "DISP LAB05-1"(w87) -> ()
          n128 = local write "DISP LAB04-1"(w91) -> ()
          n129 = local write "DISP LAB04-2"(w89) -> ()
        }
        frame #5 {
          # "initialise analog input express vi's"
          n130 = for {
            N: 2.0 -> [_]
            n131 = call "sub vi - analog 1st setup v1.vi"() -> ()  [unwired: 11 in, 5 out]
          }
        }
        frame #6 {
          # "get initial temperature values"
          n132 = stacked-sequence {
            frame #0 {
              w157 = TRUE
              n133 = call "sub vi - GET ALL TEMP v4.vi"("LA01-EN"=w157, "LA02-EN"=w157, "LA03-EN"=w157, "LA04-EN"=w157, "LA05-EN"=w157, "Gen Cal Value"=1) -> ("LA01 TEMP"=w155:T22, "LA02 TEMP"=w154:T22, "LA03 TEMP"=w153:T22, "LA04 TEMP"=w152:T22, "LA05 TEMP"=w151:T22)  [unwired: 4 in, 1 out]
              n134 = local write "LAB01 TEMP"(w155) -> ()
              n135 = local write "LAB02 TEMP"(w154) -> ()
              n136 = local write "LAB04 TEMP"(w152) -> ()
              n137 = local write "LAB03 TEMP"(w153) -> ()
              n138 = local write "LAB05 TEMP"(w151) -> ()
            }
            frame #1 {
              w158 = 0
              n139 = local read "LAB01 TEMP"() -> (w164:T13)
              n140 = Unbundle By Name(w164) -> ("T1 Live"=w163:dbl, "T1 Neut"=w162:dbl, "T2 Live"=w161:dbl, "T2 Neut"=w160:dbl)  [unwired: 2 out]
              n141 = local read "TEMP LA01"() -> (w165:T10)
              n142 = Bundle By Name(cluster=w165, "TL-1"=w163, "TN-1"=w162, "TL-2"=w161, "TN-2"=w160, "TL -1COUNT"=w158, "TN-1 COUNT"=w158, "TL-2 COUNT"=w158, "TN-2 COUNT"=w158) -> (w159:T10)
              n143 = local write "TEMP LA01"(w159) -> ()
            }
            frame #2 {
              w166 = 0
              n144 = local read "LAB02 TEMP"() -> (w172:T13)
              n145 = Unbundle By Name(w172) -> ("T1 Live"=w171:dbl, "T1 Neut"=w170:dbl, "T2 Live"=w169:dbl, "T2 Neut"=w168:dbl)  [unwired: 2 out]
              n146 = local read "TEMP LA02"() -> (w173:T10)
              n147 = Bundle By Name(cluster=w173, "TL-1"=w171, "TN-1"=w170, "TL-2"=w169, "TN-2"=w168, "TL -1COUNT"=w166, "TN-1 COUNT"=w166, "TL-2 COUNT"=w166, "TN-2 COUNT"=w166) -> (w167:T10)
              n148 = local write "TEMP LA02"(w167) -> ()
            }
            frame #3 {
              w174 = 0
              n149 = local read "LAB03 TEMP"() -> (w180:T13)
              n150 = Unbundle By Name(w180) -> ("T1 Live"=w179:dbl, "T1 Neut"=w178:dbl, "T2 Live"=w177:dbl, "T2 Neut"=w176:dbl)  [unwired: 2 out]
              n151 = local read "TEMP LA03"() -> (w181:T10)
              n152 = Bundle By Name(cluster=w181, "TL-1"=w179, "TN-1"=w178, "TL-2"=w177, "TN-2"=w176, "TL -1COUNT"=w174, "TN-1 COUNT"=w174, "TL-2 COUNT"=w174, "TN-2 COUNT"=w174) -> (w175:T10)
              n153 = local write "TEMP LA03"(w175) -> ()
            }
            frame #4 {
              w182 = 0
              n154 = local read "LAB04 TEMP"() -> (w188:T13)
              n155 = Unbundle By Name(w188) -> ("T1 Live"=w187:dbl, "T1 Neut"=w186:dbl, "T2 Live"=w185:dbl, "T2 Neut"=w184:dbl)  [unwired: 2 out]
              n156 = local read "TEMP LA04"() -> (w189:T10)
              n157 = Bundle By Name(cluster=w189, "TL-1"=w187, "TN-1"=w186, "TL-2"=w185, "TN-2"=w184, "TL -1COUNT"=w182, "TN-1 COUNT"=w182, "TL-2 COUNT"=w182, "TN-2 COUNT"=w182) -> (w183:T10)
              n158 = local write "TEMP LA04"(w183) -> ()
            }
            frame #5 {
              w190 = 0
              n159 = local read "LAB05 TEMP"() -> (w196:T13)
              n160 = Unbundle By Name(w196) -> ("T1 Live"=w195:dbl, "T1 Neut"=w194:dbl, "T2 Live"=w193:dbl, "T2 Neut"=w192:dbl)  [unwired: 2 out]
              n161 = local read "TEMP LA05"() -> (w197:T10)
              n162 = Bundle By Name(cluster=w197, "TL-1"=w195, "TN-1"=w194, "TL-2"=w193, "TN-2"=w192, "TL -1COUNT"=w190, "TN-1 COUNT"=w190, "TL-2 COUNT"=w190, "TN-2 COUNT"=w190) -> (w191:T10)
              n163 = local write "TEMP LA05"(w191) -> ()
            }
          }
        }
        frame #7 {
          # "check network directory valid"
          n164 = while {
            stop <- w198 continue-if-true
            n165 = local read "Network Directory"() -> (w200:path)
            n166 = property on="Tab Control 2" class="TabCtl (strict)"("Value"=3) -> ()  [unwired: 2 in, 2 out]
            n167 = File/Directory Info(path=w200) -> (error out=w201:errorcluster)  [unwired: 1 in, 6 out]
            n168 = Unbundle(w201) -> ("status"=w198:bool)  [unwired: 2 out]
            n169 = case shown="True" w198 {
              frame False {
                n170 = local write "Message"("") -> ()
              }
              frame True {
                "Message" <- "NETWORK DIRECTORY NOT FOUND!!!!"
              }
            }
          }
        }
        frame #8 {
          # "enable front panel, all settings done"
          n171 = property on="Tab Control 2" class="TabCtl (strict)"("DisabledEnum"=T14."Enabled" ("Disabled")) -> ()  [unwired: 2 in, 2 out]
          n172 = property on="Tab Control 2" class="TabCtl (strict)"("Value"=0) -> ()  [unwired: 2 in, 2 out]
        }
      }
    }
    frame #2 {
      n173 = node-c288("loop  delay(mS)") -> (w208:T15)  [unwired: 3 in]
      n174 = timed-loop {
        timing: w208 -> [_]
        timing-out: [_] -> w207
        i -> [w230]
        stop <- "stop" stop-if-true
        n175 = node-c288() -> ()  [unwired: 1 in, 1 out]
        n176 = local read "SELECT LAB05-2"() -> (w210:T3)
        n177 = local read "SELECT LAB05-1"() -> (w211:T3)
        n178 = local read "SELECT LAB04-2"() -> (w212:T3)
        n179 = local read "SELECT LAB03-1"() -> (w215:T3)
        n180 = local read "SELECT LAB02-2"() -> (w216:T3)
        n181 = local read "SELECT LAB01-1"() -> (w219:T3)
        n182 = local read "SELECT LAB03-2"() -> (w214:T3)
        n183 = local read "SELECT LAB01-2"() -> (w218:T3)
        n184 = local read "SELECT LAB04-1"() -> (w213:T3)
        n185 = local read "SELECT LAB02-1"() -> (w217:T3)
        n186 = local read "run lab03-2"() -> (w224:bool)
        n187 = local read "run lab04-1"() -> (w223:bool)
        n188 = local read "run lab05-1"() -> (w221:bool)
        n189 = local read "run lab04-2"() -> (w222:bool)
        n190 = local read "run lab05-2"() -> (w220:bool)
        n191 = local read "run lab03-1"() -> (w225:bool)
        n192 = local read "run lab02-2"() -> (w226:bool)
        n193 = local read "run lab02-1"() -> (w227:bool)
        n194 = local read "run lab01-1"() -> (w229:bool)
        n195 = local read "run lab01-2"() -> (w228:bool)
        n196 = stacked-sequence {
          seq-local: [_ w292 _ _ _ _ _ _ _ _ _ _ _ _ _ _ _ _ _] -> [_ _ _ _ _ w1827 _ _ _ _ _ _ _ _ _ _ _ _ _]
          seq-local: [_ w291 _ _ _ _ _ _ _ _ _ _ _ _ _ _ _ _ _] -> [_ _ _ _ _ w1826 _ _ _ _ _ _ _ _ _ _ _ _ _]
          seq-local: [_ w278 _ _ _ _ _ _ _ _ _ _ _ _ _ _ _ _ _] -> [_ _ _ _ _ w1825 _ _ _ _ _ _ _ _ _ _ _ _ _]
          seq-local: [_ w277 _ _ _ _ _ _ _ _ _ _ _ _ _ _ _ _ _] -> [_ _ _ _ _ w1824 _ _ _ _ _ _ _ _ _ _ _ _ _]
          seq-local: [_ w276 _ _ _ _ _ _ _ _ _ _ _ _ _ _ _ _ _] -> [_ _ _ _ _ w1823 _ _ _ _ _ _ _ _ _ _ _ _ _]
          seq-local: [_ w275 _ _ _ _ _ _ _ _ _ _ _ _ _ _ _ _ _] -> [_ _ _ _ _ w1822 _ _ _ _ _ _ _ _ _ _ _ _ _]
          seq-local: [_ w274 _ _ _ _ _ _ _ _ _ _ _ _ _ _ _ _ _] -> [_ _ _ _ _ w1821 _ _ _ _ _ _ _ _ _ _ _ _ _]
          seq-local: [_ w273 _ _ _ _ _ _ _ _ _ _ _ _ _ _ _ _ _] -> [_ _ _ _ _ w1820 _ _ _ _ _ _ _ _ _ _ _ _ _]
          seq-local: [_ w272 _ _ _ _ _ _ _ _ _ _ _ _ _ _ _ _ _] -> [_ _ _ _ _ w1819 _ _ _ _ _ _ _ _ _ _ _ _ _]
          seq-local: [_ w271 _ _ _ _ _ _ _ _ _ _ _ _ _ _ _ _ _] -> [_ _ _ _ _ w1818 _ _ _ _ _ _ _ _ _ _ _ _ _]
          tunnel: w229 -> [_ _ w308 w473 w1417 w1847 w2157 w2402 _ _ _ _ _ w2890 _ w3817 _ _ w4097]
          tunnel: w228 -> [_ _ w307 w471 w1416 w1846 w2158 w2401 _ _ _ _ _ w2889 _ w3815 _ _ w4096]
          tunnel: w227 -> [_ _ w306 w469 w1415 w1845 w2156 w2400 _ _ _ _ _ w2888 _ w3813 _ _ w4095]
          tunnel: w226 -> [_ _ w305 w467 w1414 w1844 w2155 w2399 _ _ _ _ _ w2887 _ w3811 _ _ w4094]
          tunnel: w225 -> [_ _ w304 w465 w1413 w1843 w2154 w2398 _ _ _ _ _ w2886 _ w3809 _ _ w4093]
          tunnel: w224 -> [_ _ w303 w463 w1412 w1842 w2153 w2397 _ _ _ _ _ w2885 _ w3807 _ _ w4092]
          tunnel: w223 -> [_ _ w302 w461 w1411 w1841 w2152 w2396 _ _ _ _ _ w2884 _ w3805 _ _ w4091]
          tunnel: w222 -> [_ _ w301 w459 w1410 w1840 w2151 w2395 _ _ _ _ _ w2883 _ w3803 _ _ w4090]
          tunnel: w221 -> [_ _ w300 w457 w1409 w1839 w2150 w2394 _ _ _ _ _ w2882 _ w3801 _ _ w4089]
          tunnel: w220 -> [_ _ w299 w455 w1408 w1838 w2149 w2393 _ _ _ _ _ w2881 _ w3799 _ _ w4088]
          tunnel: w219 -> [_ _ _ w472 w1407 w1837 _ _ _ _ _ _ _ _ _ w3819 _ _ _]
          tunnel: w218 -> [_ _ _ w470 w1406 w1836 _ _ _ _ _ _ _ _ _ w3814 _ _ _]
          tunnel: w217 -> [_ _ _ w468 w1405 w1835 _ _ _ _ _ _ _ _ _ w3812 _ _ _]
          tunnel: w216 -> [_ _ _ w466 w1404 w1834 _ _ _ _ _ _ _ _ _ w3810 _ _ _]
          tunnel: w215 -> [_ _ _ w464 w1403 w1833 _ _ _ _ _ _ _ _ _ w3808 _ _ _]
          tunnel: w214 -> [_ _ _ w462 w1402 w1832 _ _ _ _ _ _ _ _ _ w3806 _ _ _]
          tunnel: w213 -> [_ _ _ w460 w1401 w1831 _ _ _ _ _ _ _ _ _ w3804 _ _ _]
          tunnel: w212 -> [_ _ _ w458 w1400 w1830 _ _ _ _ _ _ _ _ _ w3802 _ _ _]
          tunnel: w211 -> [_ _ _ w456 w1399 w1829 _ _ _ _ _ _ _ _ _ w3800 _ _ _]
          tunnel: w210 -> [_ _ _ w454 w1398 w1828 _ _ _ _ _ _ _ _ _ w3798 _ _ _]
          frame #0 {
            w234 = FALSE
            w239 = 0.5
            # "set up cycle control"
            n197 = local read "jig cycle"() -> (w238:dbl)
            n198 = Divide(x="JIG ON TIME (S)", y=w239) -> (x/y=→"on loops":dbl)
            n199 = Divide(x="JIG OFF TIME (S)", y=w239) -> (x/y=→"off loops":dbl)
            n200 = Increment(x=w238) -> (x+1=w237:dbl)
            n201 = local write "TEMP update"(w234) -> ()
            n202 = local write "AI update"(w234) -> ()
            n203 = local write "jig cycle"(w237) -> ()
            n204 = event shown="[1] \"ADMIN PAGE\": Value Change" {
              selector: _ -> [_ _]
              dyn-events: _ -> [_ _]
              timeout: 10 -> [_ _]
              event Timeout {
                n205 = event-data() -> ()  [unwired: 1 in, 3 out]
              }
              event "ADMIN PAGE": Value Change {
                n206 = event-data() -> ()  [unwired: 1 in, 6 out]
                n207 = stacked-sequence {
                  seq-local: [_ w243 _] -> [_ _ w244]
                  frame #0 {
                    n208 = global write "Global 1.vi" "password"("9999") -> ()
                  }
                  frame #1 {
                    n209 = call "sub vi - password 1.vi"() -> ("RESULT"=w243:bool)  [unwired: 11 in]
                  }
                  frame #2 {
                    w246 = FALSE
                    n210 = property on="Tab Control 2" class="TabCtl (strict)"() -> ("Pages"=w250:refnum<vi>[])  [unwired: 2 in, 2 out]
                    n211 = Select(t=TRUE, s=w244, f=w246) -> (s? t:f=w245:bool)
                    n212 = Index Array(array=w250, index=9) -> (element=w248:refnum<vi>)
                    n213 = property class="Page"(reference=w248, "PageVis"=w245) -> ()  [unwired: 1 in, 2 out]
                    n214 = local write "ADMIN PAGE"(w246) -> ()
                  }
                }
              }
            }
          }
          frame #1 {
            w288 = 60.0
            # "convert temperature rise minutes to cycles"
            n215 = local read "SET LAB05-2"() -> (w252:T5)
            n216 = local read "SET LAB05-1"() -> (w254:T5)
            n217 = local read "SET LAB04-2"() -> (w256:T5)
            n218 = local read "SET LAB01-1"() -> (w270:T5)
            n219 = local read "SET LAB01-2"() -> (w268:T5)
            n220 = local read "SET LAB02-2"() -> (w264:T5)
            n221 = local read "SET LAB04-1"() -> (w258:T5)
            n222 = local read "SET LAB03-1"() -> (w262:T5)
            n223 = local read "SET LAB03-2"() -> (w260:T5)
            n224 = local read "SET LAB02-1"() -> (w266:T5)
            n225 = local read "JIG OFF TIME (S)"() -> (w293:dbl)
            n226 = local read "JIG ON TIME (S)"() -> (w294:dbl)
            n227 = Unbundle(w252) -> ("T-RISE mins"=w251:dbl)  [unwired: 4 out]
            n228 = Unbundle(w254) -> ("T-RISE mins"=w253:dbl)  [unwired: 4 out]
            n229 = Unbundle(w270) -> ("T-RISE mins"=w269:dbl)  [unwired: 4 out]
            n230 = Unbundle(w256) -> ("T-RISE mins"=w255:dbl)  [unwired: 4 out]
            n231 = Unbundle(w268) -> ("T-RISE mins"=w267:dbl)  [unwired: 4 out]
            n232 = Unbundle(w266) -> ("T-RISE mins"=w265:dbl)  [unwired: 4 out]
            n233 = Unbundle(w258) -> ("T-RISE mins"=w257:dbl)  [unwired: 4 out]
            n234 = Unbundle(w264) -> ("T-RISE mins"=w263:dbl)  [unwired: 4 out]
            n235 = Unbundle(w260) -> ("T-RISE mins"=w259:dbl)  [unwired: 4 out]
            n236 = Unbundle(w262) -> ("T-RISE mins"=w261:dbl)  [unwired: 4 out]
            n237 = Add(x=w294, y=w293) -> (x+y=w287:dbl)
            n238 = Multiply(x=w288, y=w259) -> (x*y=w283:dbl)
            n239 = Multiply(x=w288, y=w257) -> (x*y=w282:dbl)
            n240 = Multiply(x=w288, y=w255) -> (x*y=w281:dbl)
            n241 = Multiply(x=w288, y=w253) -> (x*y=w280:dbl)
            n242 = Multiply(x=w288, y=w251) -> (x*y=w279:dbl)
            n243 = Multiply(x=w288, y=w267) -> (x*y=w289:dbl)
            n244 = Multiply(x=w288, y=w261) -> (x*y=w284:dbl)
            n245 = Multiply(x=w288, y=w269) -> (x*y=w290:dbl)
            n246 = Multiply(x=w288, y=w265) -> (x*y=w286:dbl)
            n247 = Multiply(x=w288, y=w263) -> (x*y=w285:dbl)
            n248 = Divide(x=w280, y=w287) -> (x/y=w272:dbl)
            n249 = Divide(x=w281, y=w287) -> (x/y=w273:dbl)
            n250 = Divide(x=w282, y=w287) -> (x/y=w274:dbl)
            n251 = Divide(x=w279, y=w287) -> (x/y=w271:dbl)
            n252 = Divide(x=w284, y=w287) -> (x/y=w276:dbl)
            n253 = Divide(x=w290, y=w287) -> (x/y=w292:dbl)
            n254 = Divide(x=w289, y=w287) -> (x/y=w291:dbl)
            n255 = Divide(x=w286, y=w287) -> (x/y=w278:dbl)
            n256 = Divide(x=w285, y=w287) -> (x/y=w277:dbl)
            n257 = Divide(x=w283, y=w287) -> (x/y=w275:dbl)
          }
          frame #2 {
            # "control cycle loops"
            n258 = local read "JIG OFF TIME (S)"() -> (w297:dbl)
            n259 = local read "JIG ON TIME (S)"() -> (w296:dbl)
            n260 = local read "jig cycle"() -> (w310:dbl)
            n261 = local read "on loops"() -> (w312:dbl)
            n262 = local read "off loops"() -> (w311:dbl)
            n263 = Add(x=w297, y=w296) -> (x+y=w295:dbl)
            n264 = Add(x=w312, y=w311) -> (x+y=w298:dbl)
            n265 = Greater Or Equal?(x=w310, y=w298) -> (x >= y?=w309:bool)
            n266 = case shown="True" w309 {
              tunnel: w308 -> [_ w323]
              tunnel: w307 -> [_ w322]
              tunnel: w306 -> [_ w321]
              tunnel: w305 -> [_ w320]
              tunnel: w304 -> [_ w319]
              tunnel: w303 -> [_ w318]
              tunnel: w302 -> [_ w317]
              tunnel: w301 -> [_ w316]
              tunnel: w300 -> [_ w315]
              tunnel: w299 -> [_ w314]
              tunnel: w295 -> [_ w313]
              frame False {
              }
              frame True {
                # "increment cycle value and convert cycles to minutes for temp rise"
                n267 = stacked-sequence {
                  tunnel: w323 -> [w333 _ _ _ _ _ _ _ _ _]
                  tunnel: w322 -> [_ w345 _ _ _ _ _ _ _ _]
                  tunnel: w321 -> [_ _ w357 _ _ _ _ _ _ _]
                  tunnel: w320 -> [_ _ _ w369 _ _ _ _ _ _]
                  tunnel: w319 -> [_ _ _ _ w381 _ _ _ _ _]
                  tunnel: w318 -> [_ _ _ _ _ w393 _ _ _ _]
                  tunnel: w317 -> [_ _ _ _ _ _ w405 _ _ _]
                  tunnel: w316 -> [_ _ _ _ _ _ _ w417 _ _]
                  tunnel: w315 -> [_ _ _ _ _ _ _ _ w429 _]
                  tunnel: w314 -> [_ _ _ _ _ _ _ _ _ w441]
                  tunnel: w313 -> [w330 w342 w354 w366 w378 w390 w402 w414 w426 w438]
                  frame #0 {
                    # "LAB01-1"
                    n268 = local read "DISP LAB01-1"() -> (w328:T4)
                    n269 = Unbundle(w328) -> ("CYCLE"=w329:dbl)  [unwired: 2 out]
                    n270 = case shown="True" w333 {
                      tunnel: w329 -> [w334 w336]
                      tunnel: [w334 w335] -> w327
                      frame False {
                      }
                      frame True {
                        n271 = Increment(x=w336) -> (x+1=w335:dbl)
                      }
                    }
                    n272 = Multiply(x=w327, y=w330) -> (x*y=w331:dbl)
                    n273 = Divide(x=w331, y=60.0) -> (x/y=w326:dbl)
                    n274 = Bundle(cluster=w328, "CYCLE"=w327, "MINS"=w326) -> (w325:T4)  [unwired: 1 in]
                    n275 = local write "DISP LAB01-1"(w325) -> ()
                  }
                  frame #1 {
                    # "update cycle value"
                    # "LAB01-2"
                    n276 = local read "DISP LAB01-2"() -> (w340:T4)
                    n277 = Unbundle(w340) -> ("CYCLE"=w341:dbl)  [unwired: 2 out]
                    n278 = case shown="True" w345 {
                      tunnel: w341 -> [w346 w348]
                      tunnel: [w346 w347] -> w338
                      frame False {
                      }
                      frame True {
                        n279 = Increment(x=w348) -> (x+1=w347:dbl)
                      }
                    }
                    n280 = Multiply(x=w338, y=w342) -> (x*y=w343:dbl)
                    n281 = Divide(x=w343, y=60.0) -> (x/y=w337:dbl)
                    n282 = Bundle(cluster=w340, "CYCLE"=w338, "MINS"=w337) -> (w339:T4)  [unwired: 1 in]
                    n283 = local write "DISP LAB01-2"(w339) -> ()
                  }
                  frame #2 {
                    # "update cycle value"
                    # "LAB02-1"
                    n284 = local read "DISP LAB02-1"() -> (w352:T4)
                    n285 = Unbundle(w352) -> ("CYCLE"=w353:dbl)  [unwired: 2 out]
                    n286 = case shown="True" w357 {
                      tunnel: [w358 w360] -> w350
                      tunnel: w353 -> [w358 w359]
                      frame False {
                      }
                      frame True {
                        n287 = Increment(x=w359) -> (x+1=w360:dbl)
                      }
                    }
                    n288 = Multiply(x=w350, y=w354) -> (x*y=w355:dbl)
                    n289 = Divide(x=w355, y=60.0) -> (x/y=w349:dbl)
                    n290 = Bundle(cluster=w352, "CYCLE"=w350, "MINS"=w349) -> (w351:T4)  [unwired: 1 in]
                    n291 = local write "DISP LAB02-1"(w351) -> ()
                  }
                  frame #3 {
                    # "update cycle value"
                    # "LAB02-2"
                    n292 = local read "DISP LAB02-2"() -> (w364:T4)
                    n293 = Unbundle(w364) -> ("CYCLE"=w365:dbl)  [unwired: 2 out]
                    n294 = case shown="True" w369 {
                      tunnel: [w370 w372] -> w363
                      tunnel: w365 -> [w370 w371]
                      frame False {
                      }
                      frame True {
                        n295 = Increment(x=w371) -> (x+1=w372:dbl)
                      }
                    }
                    n296 = Multiply(x=w363, y=w366) -> (x*y=w367:dbl)
                    n297 = Divide(x=w367, y=60.0) -> (x/y=w362:dbl)
                    n298 = Bundle(cluster=w364, "CYCLE"=w363, "MINS"=w362) -> (w361:T4)  [unwired: 1 in]
                    n299 = local write "DISP LAB02-2"(w361) -> ()
                  }
                  frame #4 {
                    # "update cycle value"
                    # "LAB03-1"
                    n300 = local read "DISP LAB03-1"() -> (w376:T4)
                    n301 = Unbundle(w376) -> ("CYCLE"=w377:dbl)  [unwired: 2 out]
                    n302 = case shown="True" w381 {
                      tunnel: [w382 w384] -> w373
                      tunnel: w377 -> [w382 w383]
                      frame False {
                      }
                      frame True {
                        n303 = Increment(x=w383) -> (x+1=w384:dbl)
                      }
                    }
                    n304 = Multiply(x=w373, y=w378) -> (x*y=w379:dbl)
                    n305 = Divide(x=w379, y=60.0) -> (x/y=w374:dbl)
                    n306 = Bundle(cluster=w376, "CYCLE"=w373, "MINS"=w374) -> (w375:T4)  [unwired: 1 in]
                    n307 = local write "DISP LAB03-1"(w375) -> ()
                  }
                  frame #5 {
                    # "update cycle value"
                    # "LAB03-2"
                    n308 = local read "DISP LAB03-2"() -> (w388:T4)
                    n309 = Unbundle(w388) -> ("CYCLE"=w389:dbl)  [unwired: 2 out]
                    n310 = case shown="False" w393 {
                      tunnel: [w394 w396] -> w387
                      tunnel: w389 -> [w394 w395]
                      frame False {
                      }
                      frame True {
                        n311 = Increment(x=w395) -> (x+1=w396:dbl)
                      }
                    }
                    n312 = Multiply(x=w387, y=w390) -> (x*y=w391:dbl)
                    n313 = Divide(x=w391, y=60.0) -> (x/y=w386:dbl)
                    n314 = Bundle(cluster=w388, "CYCLE"=w387, "MINS"=w386) -> (w385:T4)  [unwired: 1 in]
                    n315 = local write "DISP LAB03-2"(w385) -> ()
                  }
                  frame #6 {
                    # "update cycle value"
                    # "LAB04-1"
                    n316 = local read "DISP LAB04-1"() -> (w400:T4)
                    n317 = Unbundle(w400) -> ("CYCLE"=w401:dbl)  [unwired: 2 out]
                    n318 = case shown="True" w405 {
                      tunnel: [w406 w408] -> w398
                      tunnel: w401 -> [w406 w407]
                      frame False {
                      }
                      frame True {
                        n319 = Increment(x=w407) -> (x+1=w408:dbl)
                      }
                    }
                    n320 = Multiply(x=w398, y=w402) -> (x*y=w403:dbl)
                    n321 = Divide(x=w403, y=60.0) -> (x/y=w397:dbl)
                    n322 = Bundle(cluster=w400, "CYCLE"=w398, "MINS"=w397) -> (w399:T4)  [unwired: 1 in]
                    n323 = local write "DISP LAB04-1"(w399) -> ()
                  }
                  frame #7 {
                    # "update cycle value"
                    # "LAB04-2"
                    n324 = local read "DISP LAB04-2"() -> (w412:T4)
                    n325 = Unbundle(w412) -> ("CYCLE"=w413:dbl)  [unwired: 2 out]
                    n326 = case shown="True" w417 {
                      tunnel: [w418 w420] -> w410
                      tunnel: w413 -> [w418 w419]
                      frame False {
                      }
                      frame True {
                        n327 = Increment(x=w419) -> (x+1=w420:dbl)
                      }
                    }
                    n328 = Multiply(x=w410, y=w414) -> (x*y=w416:dbl)
                    n329 = Divide(x=w416, y=60.0) -> (x/y=w409:dbl)
                    n330 = Bundle(cluster=w412, "CYCLE"=w410, "MINS"=w409) -> (w411:T4)  [unwired: 1 in]
                    n331 = local write "DISP LAB04-2"(w411) -> ()
                  }
                  frame #8 {
                    # "update cycle value"
                    # "LAB05-1"
                    n332 = local read "DISP LAB05-1"() -> (w424:T4)
                    n333 = Unbundle(w424) -> ("CYCLE"=w425:dbl)  [unwired: 2 out]
                    n334 = case shown="True" w429 {
                      tunnel: [w430 w432] -> w422
                      tunnel: w425 -> [w430 w431]
                      frame False {
                      }
                      frame True {
                        n335 = Increment(x=w431) -> (x+1=w432:dbl)
                      }
                    }
                    n336 = Multiply(x=w422, y=w426) -> (x*y=w427:dbl)
                    n337 = Divide(x=w427, y=60.0) -> (x/y=w421:dbl)
                    n338 = Bundle(cluster=w424, "CYCLE"=w422, "MINS"=w421) -> (w423:T4)  [unwired: 1 in]
                    n339 = local write "DISP LAB05-1"(w423) -> ()
                  }
                  frame #9 {
                    # "update cycle value"
                    # "LAB05-2"
                    n340 = local read "DISP LAB05-2"() -> (w437:T4)
                    n341 = Unbundle(w437) -> ("CYCLE"=w436:dbl)  [unwired: 2 out]
                    n342 = case shown="True" w441 {
                      tunnel: [w442 w444] -> w435
                      tunnel: w436 -> [w442 w443]
                      frame False {
                      }
                      frame True {
                        n343 = Increment(x=w443) -> (x+1=w444:dbl)
                      }
                    }
                    n344 = Multiply(x=w435, y=w438) -> (x*y=w439:dbl)
                    n345 = Divide(x=w439, y=60.0) -> (x/y=w434:dbl)
                    n346 = Bundle(cluster=w437, "CYCLE"=w435, "MINS"=w434) -> (w433:T4)  [unwired: 1 in]
                    n347 = local write "DISP LAB05-2"(w433) -> ()
                  }
                }
                n348 = local write "jig cycle"(0) -> ()
              }
            }
          }
          frame #3 {
            # "START & STOP test RUN switch change, start test if true and stop test if false"
            n349 = Get Date/Time In Seconds() -> (seconds since 1Jan1904=w452:timestamp)
            n350 = local read "C drive data root dir"() -> (w445:path)
            n351 = Format Date/Time String(time format string (%c)="%b\\%a%d", seconds (now)=w452) -> (date/time string=w476:string)  [unwired: 1 in]
            n352 = Format Date/Time String(time format string (%c)="%H%M", seconds (now)=w452) -> (date/time string=w474:string)  [unwired: 1 in]
            n353 = Format Date/Time String(time format string (%c)="LabPanel%Y", seconds (now)=w452) -> (date/time string=w451:string)  [unwired: 1 in]
            n354 = Path To String(path=w445) -> (string=w448:string)
            n355 = global write "Global 1.vi" "C drive root path"(w445) -> ()
            n356 = Concatenate Strings(w448, "\\") -> (w446:string)
            n357 = event shown="[1] \"RUN LAB01-1\": Value Change" {
              selector: _ -> [_ _ _ _ _ _ _ _ _ _ _]
              dyn-events: _ -> [_ _ _ _ _ _ _ _ _ _ _]
              timeout: 10 -> [_ _ _ _ _ _ _ _ _ _ _]
              tunnel: w446 -> [_ w484 w576 w668 w760 w852 w944 w1036 w1128 w1220 w1312]
              tunnel: w476 -> [_ w483 w575 w667 w759 w851 w943 w1035 w1127 w1219 w1311]
              tunnel: w474 -> [_ w481 w574 w666 w758 w850 w942 w1034 w1126 w1218 w1310]
              tunnel: w472 -> [_ w482 _ _ _ _ _ _ _ _ _]
              tunnel: w473 -> [_ _ _ _ _ _ _ _ _ _ _]
              tunnel: w471 -> [_ _ _ _ _ _ _ _ _ _ _]
              tunnel: w470 -> [_ _ w573 _ _ _ _ _ _ _ _]
              tunnel: w469 -> [_ _ _ _ _ _ _ _ _ _ _]
              tunnel: w468 -> [_ _ _ w665 _ _ _ _ _ _ _]
              tunnel: w467 -> [_ _ _ _ _ _ _ _ _ _ _]
              tunnel: w466 -> [_ _ _ _ w757 _ _ _ _ _ _]
              tunnel: w465 -> [_ _ _ _ _ _ _ _ _ _ _]
              tunnel: w464 -> [_ _ _ _ _ w849 _ _ _ _ _]
              tunnel: w463 -> [_ _ _ _ _ _ _ _ _ _ _]
              tunnel: w462 -> [_ _ _ _ _ _ w941 _ _ _ _]
              tunnel: w461 -> [_ _ _ _ _ _ _ _ _ _ _]
              tunnel: w460 -> [_ _ _ _ _ _ _ w1033 _ _ _]
              tunnel: w459 -> [_ _ _ _ _ _ _ _ _ _ _]
              tunnel: w458 -> [_ _ _ _ _ _ _ _ w1125 _ _]
              tunnel: w457 -> [_ _ _ _ _ _ _ _ _ _ _]
              tunnel: w456 -> [_ _ _ _ _ _ _ _ _ w1217 _]
              tunnel: w455 -> [_ _ _ _ _ _ _ _ _ _ _]
              tunnel: w454 -> [_ _ _ _ _ _ _ _ _ _ w1309]
              tunnel: w451 -> [_ w480 w572 w664 w756 w848 w940 w1032 w1124 w1216 w1308]
              tunnel: [_ w479 w571 w663 w755 w847 w939 w1031 w1123 w1215 w1307] -> w449
              event Timeout {
                n358 = event-data() -> ()  [unwired: 1 in, 3 out]
              }
              event "RUN LAB01-1": Value Change {
                n359 = event-data() -> ("NewVal"=w478:bool)  [unwired: 1 in, 5 out]
                n360 = local write "run lab01-1"(w478) -> ()
                n361 = case shown="True" w478 {
                  tunnel: w484 -> [_ w517]
                  tunnel: w483 -> [_ w516]
                  tunnel: w482 -> [w486 w515]
                  tunnel: w481 -> [_ w514]
                  tunnel: w480 -> [_ w513]
                  tunnel: [w485 w512] -> w479
                  frame False {
                    # "stop test"
                    n362 = stacked-sequence {
                      tunnel: w486 -> [_ w498 _ _]
                      tunnel: [_ w490 _ _] -> w485
                      frame #0 {
                        n363 = local read "DISP LAB01-1"() -> (w489:T4)
                        n364 = Bundle(cluster=w489, "STATUS"="STOP") -> (w487:T4)  [unwired: 2 in]
                        n365 = local write "DISP LAB01-1"(w487) -> ()
                      }
                      frame #1 {
                        n366 = local read "DISP LAB01-1"() -> (w497:T4)
                        n367 = Unbundle(w497) -> ("CYCLE"=w495:dbl, "MINS"=w496:dbl)  [unwired: 1 out]
                        n368 = case shown="\"CYCLE TEST\"" w498 {
                          tunnel: w496 -> [_ _ w505]
                          tunnel: w495 -> [w503 w504 _]
                          tunnel: [w503 w504 w505] -> w494
                          frame "CHART TEST", Default {
                          }
                          frame "CYCLE TEST" {
                          }
                          frame "T-RISE TEST" {
                          }
                        }
                        n369 = local read "TDMS LAB01-1"() -> (w502:refnum<k34>)
                        n370 = Build Array("STOPPED") -> (w499:string[])
                        n371 = Build Array(w494) -> (w493:dbl[])
                        n372 = TDMS Write(0:w502, 5:"TEST RESULT", 7:w499, 9:w493) -> (4:w491:refnum<k34>, 15:w492:errorcluster)  [unwired: 2 in, 2 out]
                        n373 = TDMS Close(8:w492, 11:w491) -> (0:w490:errorcluster)  [unwired: 1 out]
                      }
                      frame #2 {
                        n374 = stacked-sequence {
                          tunnel: "LAB01-1" -> [w508 w510]
                          frame #0 {
                            n375 = call "sub vi - defrag tdms v1.vi"("panel id"=w508) -> ("error out"=w507:errorcluster)  [unwired: 10 in]
                            n376 = local write "data file error"(w507) -> ()
                          }
                          frame #1 {
                            n377 = call "Save data file to network drive v1.vi"("panel id"=w510) -> ("network file save error"=w509:errorcluster)  [unwired: 9 in, 1 out]
                            n378 = local write "RESULT LAB01-1"(FALSE) -> ()
                            n379 = local write "data file error"(w509) -> ()
                          }
                        }
                      }
                      frame #3 {
                      }
                    }
                  }
                  frame True {
                    # "start new test and create test file"
                    n380 = stacked-sequence {
                      seq-local: [w518 _ _ _ _] -> [_ w539 _ _ _]
                      tunnel: w517 -> [w523 _ _ _ _]
                      tunnel: w516 -> [w519 _ _ _ _]
                      tunnel: w515 -> [w533 _ _ _ _]
                      tunnel: w514 -> [w526 _ _ _ _]
                      tunnel: w513 -> [w521 _ _ _ _]
                      tunnel: [_ w540 _ _ _] -> w512
                      frame #0 {
                        w520 = "\\"
                        n381 = case shown="\"CHART TEST\", Default" w533 {
                          tunnel: ["L01-1-CHART TEST-" "L01-1-CYCLE TEST-" "L01-1-T-RISE TEST-"] -> w529
                          frame "CHART TEST", Default {
                          }
                          frame "CYCLE TEST" {
                          }
                          frame "T-RISE TEST" {
                          }
                        }
                        n382 = local read "SET LAB01-1"() -> (w528:T5)
                        n383 = Unbundle(w528) -> ("DESCRIPTION"=w527:string)  [unwired: 4 out]
                        n384 = Concatenate Strings(w523, "\\", w521, w520, w519, w520) -> (w530:string)
                        n385 = String To Path(string=w530) -> (path=w532:path)
                        n386 = Concatenate Strings(w530, w529, w527, "-", w526, ".tdms") -> (w518:string)
                        n387 = Create Folder(path (use dialog)=w532) -> (error out=w531:errorcluster)  [unwired: 2 in, 2 out]
                        n388 = call <vilib>:"Clear Errors.vi"("error in (no error)"=w531) -> ()  [unwired: 6 in, 1 out]
                        n389 = global write "Global 1.vi" "LAB01-1 FILE"(w518) -> ()
                      }
                      frame #1 {
                        n390 = String To Path(string=w539) -> (path=w537:path)
                        n391 = TDMS Open(5:FALSE, 6:FALSE, 10:T18."create or replace" ("operation (0:open)"), 11:w537) -> (0:w540:errorcluster, 3:→"TDMS LAB01-1":refnum<k34>)  [unwired: 3 in]
                      }
                      frame #2 {
                        n392 = local read "TDMS LAB01-1"() -> (w560:refnum<k34>)
                        n393 = local read "SET LAB01-1"() -> (w549:T5)
                        n394 = Build Array("Testers Name", "Description", "Set Test Cycles", "T-Rise minutes", "T-Rise Deg C") -> (w550:string[])
                        n395 = Unbundle(w549) -> ("NAME"=w548:string, "DESCRIPTION"=w547:string, "CYCLES"=w546:dbl, "T-RISE mins"=w545:dbl, "T-RISE deg C"=w544:dbl)
                        n396 = Number To Decimal String(number=w546) -> (decimal integer string=w559:string)  [unwired: 1 in]
                        n397 = Number To Decimal String(number=w545) -> (decimal integer string=w558:string)  [unwired: 1 in]
                        n398 = Number To Decimal String(number=w544) -> (decimal integer string=w557:string)  [unwired: 1 in]
                        n399 = Build Array(w548, w547, w559, w558, w557) -> (w556:string[])
                        n400 = TDMS Set Properties(5:w556, 7:w550, 11:w560) -> ()  [unwired: 3 in, 4 out]
                      }
                      frame #3 {
                        w561 = 0.0
                        n401 = local read "DISP LAB01-1"() -> (w564:T4)
                        n402 = Bundle(cluster=w564, "CYCLE"=w561, "MINS"=w561, "STATUS"="RUN") -> (w563:T4)
                        n403 = local write "DISP LAB01-1"(w563) -> ()
                      }
                      frame #4 {
                        n404 = local read "SIG LAB01-1"() -> (w567:T2)
                        n405 = local read "TEMP START LAB01-1"() -> (w569:cluster{"TL":dbl, "TN":dbl})
                        n406 = Unbundle(w567) -> ("Tmp Live"=w566:dbl, "Tmp Neut"=w565:dbl)  [unwired: 3 out]
                        n407 = Bundle(cluster=w569, "TL"=w566, "TN"=w565) -> (w568:cluster{"TL":dbl, "TN":dbl})
                        n408 = local write "TEMP START LAB01-1"(w568) -> ()
                      }
                    }
                  }
                }
              }
              event "RUN LAB01-2": Value Change {
                n409 = event-data() -> ("NewVal"=w570:bool)  [unwired: 1 in, 5 out]
                n410 = local write "run lab01-2"(w570) -> ()
                n411 = case shown="True" w570 {
                  tunnel: w576 -> [_ w609]
                  tunnel: w575 -> [_ w608]
                  tunnel: w573 -> [w578 w607]
                  tunnel: w574 -> [_ w606]
                  tunnel: w572 -> [_ w605]
                  tunnel: [w577 w604] -> w571
                  frame False {
                    # "stop test"
                    n412 = stacked-sequence {
                      tunnel: w578 -> [w587 _]
                      tunnel: [w579 _] -> w577
                      frame #0 {
                        n413 = local read "DISP LAB01-2"() -> (w586:T4)
                        n414 = Unbundle(w586) -> ("CYCLE"=w584:dbl, "MINS"=w585:dbl)  [unwired: 1 out]
                        n415 = case shown="\"CHART TEST\", Default" w587 {
                          tunnel: w585 -> [_ _ w594]
                          tunnel: w584 -> [w592 w593 _]
                          tunnel: [w592 w593 w594] -> w583
                          frame "CHART TEST", Default {
                          }
                          frame "CYCLE TEST" {
                          }
                          frame "T-RISE TEST" {
                          }
                        }
                        n416 = local read "TDMS LAB01-2"() -> (w591:refnum<k34>)
                        n417 = Build Array("STOPPED") -> (w588:string[])
                        n418 = Build Array(w583) -> (w582:dbl[])
                        n419 = TDMS Write(0:w591, 5:"TEST RESULT", 7:w588, 9:w582) -> (4:w580:refnum<k34>, 15:w581:errorcluster)  [unwired: 2 in, 2 out]
                        n420 = TDMS Close(8:w581, 11:w580) -> (0:w579:errorcluster)  [unwired: 1 out]
                      }
                      frame #1 {
                        n421 = local read "DISP LAB01-2"() -> (w598:T4)
                        n422 = stacked-sequence {
                          tunnel: "LAB01-2" -> [w600 w602]
                          frame #0 {
                            n423 = call "sub vi - defrag tdms v1.vi"("panel id"=w600) -> ("error out"=w599:errorcluster)  [unwired: 10 in]
                            n424 = local write "data file error"(w599) -> ()
                          }
                          frame #1 {
                            n425 = call "Save data file to network drive v1.vi"("panel id"=w602) -> ("network file save error"=w601:errorcluster)  [unwired: 9 in, 1 out]
                            n426 = local write "RESULT LAB01-2"(FALSE) -> ()
                            n427 = local write "data file error"(w601) -> ()
                          }
                        }
                        n428 = Bundle(cluster=w598, "STATUS"="STOP") -> (w596:T4)  [unwired: 2 in]
                        n429 = local write "DISP LAB01-2"(w596) -> ()
                      }
                    }
                  }
                  frame True {
                    # "start new test and create test file"
                    n430 = stacked-sequence {
                      seq-local: [w610 _ _ _ _] -> [_ w635 _ _ _]
                      tunnel: w609 -> [w615 _ _ _ _]
                      tunnel: w608 -> [w612 _ _ _ _]
                      tunnel: w607 -> [w625 _ _ _ _]
                      tunnel: w606 -> [w618 _ _ _ _]
                      tunnel: w605 -> [w613 _ _ _ _]
                      tunnel: [_ w629 _ _ _] -> w604
                      frame #0 {
                        w611 = "\\"
                        n431 = local read "SET LAB01-2"() -> (w620:T5)
                        n432 = case shown="\"CYCLE TEST\"" w625 {
                          tunnel: ["L01-2-CHART TEST-" "L01-2-CYCLE TEST-" "L01-2-T-RISE TEST-"] -> w621
                          frame "CHART TEST", Default {
                          }
                          frame "CYCLE TEST" {
                          }
                          frame "T-RISE TEST" {
                          }
                        }
                        n433 = Unbundle(w620) -> ("DESCRIPTION"=w619:string)  [unwired: 4 out]
                        n434 = Concatenate Strings(w615, "\\", w613, w611, w612, w611) -> (w622:string)
                        n435 = String To Path(string=w622) -> (path=w624:path)
                        n436 = Concatenate Strings(w622, w621, w619, "-", w618, ".tdms") -> (w610:string)
                        n437 = Create Folder(path (use dialog)=w624) -> (error out=w623:errorcluster)  [unwired: 2 in, 2 out]
                        n438 = global write "Global 1.vi" "LAB01-2 FILE"(w610) -> ()
                        n439 = call <vilib>:"Clear Errors.vi"("error in (no error)"=w623) -> ()  [unwired: 6 in, 1 out]
                      }
                      frame #1 {
                        n440 = String To Path(string=w635) -> (path=w630:path)
                        n441 = TDMS Open(5:FALSE, 6:FALSE, 10:T18."create or replace" ("operation (0:open)"), 11:w630) -> (0:w629:errorcluster, 3:→"TDMS LAB01-2":refnum<k34>)  [unwired: 3 in]
                      }
                      frame #2 {
                        n442 = local read "SET LAB01-2"() -> (w641:T5)
                        n443 = local read "TDMS LAB01-2"() -> (w652:refnum<k34>)
                        n444 = Build Array("Testers Name", "Description", "Set Test Cycles", "T-Rise minutes", "T-Rise Deg C") -> (w642:string[])
                        n445 = Unbundle(w641) -> ("NAME"=w640:string, "DESCRIPTION"=w639:string, "CYCLES"=w638:dbl, "T-RISE mins"=w637:dbl, "T-RISE deg C"=w636:dbl)
                        n446 = Number To Decimal String(number=w638) -> (decimal integer string=w651:string)  [unwired: 1 in]
                        n447 = Number To Decimal String(number=w637) -> (decimal integer string=w650:string)  [unwired: 1 in]
                        n448 = Number To Decimal String(number=w636) -> (decimal integer string=w649:string)  [unwired: 1 in]
                        n449 = Build Array(w640, w639, w651, w650, w649) -> (w648:string[])
                        n450 = TDMS Set Properties(5:w648, 7:w642, 11:w652) -> ()  [unwired: 3 in, 4 out]
                      }
                      frame #3 {
                        w654 = 0.0
                        n451 = local read "DISP LAB01-2"() -> (w656:T4)
                        n452 = Bundle(cluster=w656, "CYCLE"=w654, "MINS"=w654, "STATUS"="RUN") -> (w655:T4)
                        n453 = local write "DISP LAB01-2"(w655) -> ()
                      }
                      frame #4 {
                        n454 = local read "SIG LAB01-2"() -> (w659:T2)
                        n455 = local read "TEMP START LAB01-2"() -> (w661:cluster{"TL":dbl, "TN":dbl})
                        n456 = Unbundle(w659) -> ("Tmp Live"=w658:dbl, "Tmp Neut"=w657:dbl)  [unwired: 3 out]
                        n457 = Bundle(cluster=w661, "TL"=w658, "TN"=w657) -> (w660:cluster{"TL":dbl, "TN":dbl})
                        n458 = local write "TEMP START LAB01-2"(w660) -> ()
                      }
                    }
                  }
                }
              }
              event "RUN LAB02-1": Value Change {
                n459 = event-data() -> ("NewVal"=w662:bool)  [unwired: 1 in, 5 out]
                n460 = local write "run lab02-1"(w662) -> ()
                n461 = case shown="True" w662 {
                  tunnel: w668 -> [_ w701]
                  tunnel: w667 -> [_ w700]
                  tunnel: w665 -> [w670 w699]
                  tunnel: w666 -> [_ w698]
                  tunnel: w664 -> [_ w697]
                  tunnel: [w669 w696] -> w663
                  frame False {
                    # "stop test"
                    n462 = stacked-sequence {
                      tunnel: w670 -> [w679 _]
                      tunnel: [w671 _] -> w669
                      frame #0 {
                        n463 = local read "DISP LAB02-1"() -> (w678:T4)
                        n464 = Unbundle(w678) -> ("CYCLE"=w676:dbl, "MINS"=w677:dbl)  [unwired: 1 out]
                        n465 = case shown="\"CYCLE TEST\"" w679 {
                          tunnel: w677 -> [_ _ w686]
                          tunnel: w676 -> [w684 w685 _]
                          tunnel: [w684 w685 w686] -> w675
                          frame "CHART TEST", Default {
                          }
                          frame "CYCLE TEST" {
                          }
                          frame "T-RISE TEST" {
                          }
                        }
                        n466 = local read "TDMS LAB02-1"() -> (w683:refnum<k34>)
                        n467 = Build Array("STOPPED") -> (w680:string[])
                        n468 = Build Array(w675) -> (w674:dbl[])
                        n469 = TDMS Write(0:w683, 5:"TEST RESULT", 7:w680, 9:w674) -> (4:w672:refnum<k34>, 15:w673:errorcluster)  [unwired: 2 in, 2 out]
                        n470 = TDMS Close(8:w673, 11:w672) -> (0:w671:errorcluster)  [unwired: 1 out]
                      }
                      frame #1 {
                        n471 = local read "DISP LAB02-1"() -> (w690:T4)
                        n472 = stacked-sequence {
                          tunnel: "LAB02-1" -> [w692 w694]
                          frame #0 {
                            n473 = call "sub vi - defrag tdms v1.vi"("panel id"=w692) -> ("error out"=w691:errorcluster)  [unwired: 10 in]
                            n474 = local write "data file error"(w691) -> ()
                          }
                          frame #1 {
                            n475 = local write "RESULT LAB02-1"(FALSE) -> ()
                            n476 = call "Save data file to network drive v1.vi"("panel id"=w694) -> ("network file save error"=w693:errorcluster)  [unwired: 9 in, 1 out]
                            n477 = local write "data file error"(w693) -> ()
                          }
                        }
                        n478 = Bundle(cluster=w690, "STATUS"="STOP") -> (w688:T4)  [unwired: 2 in]
                        n479 = local write "DISP LAB02-1"(w688) -> ()
                      }
                    }
                  }
                  frame True {
                    # "start new test and create test file"
                    n480 = stacked-sequence {
                      seq-local: [w702 _ _ _ _] -> [_ w727 _ _ _]
                      tunnel: w701 -> [w707 _ _ _ _]
                      tunnel: w700 -> [w704 _ _ _ _]
                      tunnel: w699 -> [w717 _ _ _ _]
                      tunnel: w698 -> [w710 _ _ _ _]
                      tunnel: w697 -> [w705 _ _ _ _]
                      tunnel: [_ w721 _ _ _] -> w696
                      frame #0 {
                        w703 = "\\"
                        n481 = local read "SET LAB02-1"() -> (w712:T5)
                        n482 = case shown="\"CYCLE TEST\"" w717 {
                          tunnel: ["L02-1-CHART TEST-" "L02-1-CYCLE TEST-" "L02-1-T-RISE TEST-"] -> w713
                          frame "CHART TEST", Default {
                          }
                          frame "CYCLE TEST" {
                          }
                          frame "T-RISE TEST" {
                          }
                        }
                        n483 = Unbundle(w712) -> ("DESCRIPTION"=w711:string)  [unwired: 4 out]
                        n484 = Concatenate Strings(w707, "\\", w705, w703, w704, w703) -> (w714:string)
                        n485 = String To Path(string=w714) -> (path=w716:path)
                        n486 = Concatenate Strings(w714, w713, w711, "-", w710, ".tdms") -> (w702:string)
                        n487 = Create Folder(path (use dialog)=w716) -> (error out=w715:errorcluster)  [unwired: 2 in, 2 out]
                        n488 = global write "Global 1.vi" "LAB02-1 FILE"(w702) -> ()
                        n489 = call <vilib>:"Clear Errors.vi"("error in (no error)"=w715) -> ()  [unwired: 6 in, 1 out]
                      }
                      frame #1 {
                        n490 = String To Path(string=w727) -> (path=w722:path)
                        n491 = TDMS Open(5:FALSE, 6:FALSE, 10:T18."create or replace" ("operation (0:open)"), 11:w722) -> (0:w721:errorcluster, 3:→"TDMS LAB02-1":refnum<k34>)  [unwired: 3 in]
                      }
                      frame #2 {
                        n492 = local read "SET LAB02-1"() -> (w733:T5)
                        n493 = local read "TDMS LAB02-1"() -> (w744:refnum<k34>)
                        n494 = Build Array("Testers Name", "Description", "Set Test Cycles", "T-Rise minutes", "T-Rise Deg C") -> (w734:string[])
                        n495 = Unbundle(w733) -> ("NAME"=w732:string, "DESCRIPTION"=w731:string, "CYCLES"=w730:dbl, "T-RISE mins"=w729:dbl, "T-RISE deg C"=w728:dbl)
                        n496 = Number To Decimal String(number=w730) -> (decimal integer string=w743:string)  [unwired: 1 in]
                        n497 = Number To Decimal String(number=w729) -> (decimal integer string=w742:string)  [unwired: 1 in]
                        n498 = Number To Decimal String(number=w728) -> (decimal integer string=w741:string)  [unwired: 1 in]
                        n499 = Build Array(w732, w731, w743, w742, w741) -> (w740:string[])
                        n500 = TDMS Set Properties(5:w740, 7:w734, 11:w744) -> ()  [unwired: 3 in, 4 out]
                      }
                      frame #3 {
                        w746 = 0.0
                        n501 = local read "DISP LAB02-1"() -> (w748:T4)
                        n502 = Bundle(cluster=w748, "CYCLE"=w746, "MINS"=w746, "STATUS"="RUN") -> (w747:T4)
                        n503 = local write "DISP LAB02-1"(w747) -> ()
                      }
                      frame #4 {
                        n504 = local read "SIG LAB02-1"() -> (w751:T2)
                        n505 = local read "TEMP START LAB02-1"() -> (w753:cluster{"TL":dbl, "TN":dbl})
                        n506 = Unbundle(w751) -> ("Tmp Live"=w750:dbl, "Tmp Neut"=w749:dbl)  [unwired: 3 out]
                        n507 = Bundle(cluster=w753, "TL"=w750, "TN"=w749) -> (w752:cluster{"TL":dbl, "TN":dbl})
                        n508 = local write "TEMP START LAB02-1"(w752) -> ()
                      }
                    }
                  }
                }
              }
              event "RUN LAB02-2": Value Change {
                n509 = event-data() -> ("NewVal"=w754:bool)  [unwired: 1 in, 5 out]
                n510 = local write "run lab02-2"(w754) -> ()
                n511 = case shown="True" w754 {
                  tunnel: w760 -> [_ w793]
                  tunnel: w759 -> [_ w792]
                  tunnel: w757 -> [w762 w791]
                  tunnel: w758 -> [_ w790]
                  tunnel: w756 -> [_ w789]
                  tunnel: [w761 w788] -> w755
                  frame False {
                    # "stop test"
                    n512 = stacked-sequence {
                      tunnel: w762 -> [w771 _]
                      tunnel: [w763 _] -> w761
                      frame #0 {
                        n513 = local read "DISP LAB02-2"() -> (w770:T4)
                        n514 = Unbundle(w770) -> ("CYCLE"=w768:dbl, "MINS"=w769:dbl)  [unwired: 1 out]
                        n515 = case shown="\"CYCLE TEST\"" w771 {
                          tunnel: w769 -> [_ _ w778]
                          tunnel: w768 -> [w776 w777 _]
                          tunnel: [w776 w777 w778] -> w767
                          frame "CHART TEST", Default {
                          }
                          frame "CYCLE TEST" {
                          }
                          frame "T-RISE TEST" {
                          }
                        }
                        n516 = local read "TDMS LAB02-2"() -> (w775:refnum<k34>)
                        n517 = Build Array("STOPPED") -> (w772:string[])
                        n518 = Build Array(w767) -> (w766:dbl[])
                        n519 = TDMS Write(0:w775, 5:"TEST RESULT", 7:w772, 9:w766) -> (4:w764:refnum<k34>, 15:w765:errorcluster)  [unwired: 2 in, 2 out]
                        n520 = TDMS Close(8:w765, 11:w764) -> (0:w763:errorcluster)  [unwired: 1 out]
                      }
                      frame #1 {
                        n521 = local read "DISP LAB02-2"() -> (w782:T4)
                        n522 = stacked-sequence {
                          tunnel: "LAB02-2" -> [w784 w786]
                          frame #0 {
                            n523 = call "sub vi - defrag tdms v1.vi"("panel id"=w784) -> ("error out"=w783:errorcluster)  [unwired: 10 in]
                            n524 = local write "data file error"(w783) -> ()
                          }
                          frame #1 {
                            n525 = call "Save data file to network drive v1.vi"("panel id"=w786) -> ("network file save error"=w785:errorcluster)  [unwired: 9 in, 1 out]
                            n526 = local write "RESULT LAB02-2"(FALSE) -> ()
                            n527 = local write "data file error"(w785) -> ()
                          }
                        }
                        n528 = Bundle(cluster=w782, "STATUS"="STOP") -> (w780:T4)  [unwired: 2 in]
                        n529 = local write "DISP LAB02-2"(w780) -> ()
                      }
                    }
                  }
                  frame True {
                    # "start new test and create test file"
                    n530 = stacked-sequence {
                      seq-local: [w794 _ _ _ _] -> [_ w819 _ _ _]
                      tunnel: w793 -> [w799 _ _ _ _]
                      tunnel: w792 -> [w796 _ _ _ _]
                      tunnel: w791 -> [w809 _ _ _ _]
                      tunnel: w790 -> [w802 _ _ _ _]
                      tunnel: w789 -> [w797 _ _ _ _]
                      tunnel: [_ w813 _ _ _] -> w788
                      frame #0 {
                        w795 = "\\"
                        n531 = local read "SET LAB02-2"() -> (w804:T5)
                        n532 = case shown="\"CYCLE TEST\"" w809 {
                          tunnel: ["L02-2-CHART TEST-" "L02-2-CYCLE TEST-" "L02-2-T-RISE TEST-"] -> w805
                          frame "CHART TEST", Default {
                          }
                          frame "CYCLE TEST" {
                          }
                          frame "T-RISE TEST" {
                          }
                        }
                        n533 = Unbundle(w804) -> ("DESCRIPTION"=w803:string)  [unwired: 4 out]
                        n534 = Concatenate Strings(w799, "\\", w797, w795, w796, w795) -> (w806:string)
                        n535 = String To Path(string=w806) -> (path=w808:path)
                        n536 = Concatenate Strings(w806, w805, w803, "-", w802, ".tdms") -> (w794:string)
                        n537 = Create Folder(path (use dialog)=w808) -> (error out=w807:errorcluster)  [unwired: 2 in, 2 out]
                        n538 = global write "Global 1.vi" "LAB02-2 FILE"(w794) -> ()
                        n539 = call <vilib>:"Clear Errors.vi"("error in (no error)"=w807) -> ()  [unwired: 6 in, 1 out]
                      }
                      frame #1 {
                        n540 = String To Path(string=w819) -> (path=w814:path)
                        n541 = TDMS Open(5:FALSE, 6:FALSE, 10:T18."create or replace" ("operation (0:open)"), 11:w814) -> (0:w813:errorcluster, 3:→"TDMS LAB02-2":refnum<k34>)  [unwired: 3 in]
                      }
                      frame #2 {
                        n542 = local read "SET LAB02-2"() -> (w825:T5)
                        n543 = local read "TDMS LAB02-2"() -> (w836:refnum<k34>)
                        n544 = Build Array("Testers Name", "Description", "Set Test Cycles", "T-Rise minutes", "T-Rise Deg C") -> (w826:string[])
                        n545 = Unbundle(w825) -> ("NAME"=w824:string, "DESCRIPTION"=w823:string, "CYCLES"=w822:dbl, "T-RISE mins"=w821:dbl, "T-RISE deg C"=w820:dbl)
                        n546 = Number To Decimal String(number=w822) -> (decimal integer string=w835:string)  [unwired: 1 in]
                        n547 = Number To Decimal String(number=w821) -> (decimal integer string=w834:string)  [unwired: 1 in]
                        n548 = Number To Decimal String(number=w820) -> (decimal integer string=w833:string)  [unwired: 1 in]
                        n549 = Build Array(w824, w823, w835, w834, w833) -> (w832:string[])
                        n550 = TDMS Set Properties(5:w832, 7:w826, 11:w836) -> ()  [unwired: 3 in, 4 out]
                      }
                      frame #3 {
                        w838 = 0.0
                        n551 = local read "DISP LAB02-2"() -> (w840:T4)
                        n552 = Bundle(cluster=w840, "CYCLE"=w838, "MINS"=w838, "STATUS"="RUN") -> (w839:T4)
                        n553 = local write "DISP LAB02-2"(w839) -> ()
                      }
                      frame #4 {
                        n554 = local read "SIG LAB02-2"() -> (w843:T2)
                        n555 = local read "TEMP START LAB02-2"() -> (w845:cluster{"TL":dbl, "TN":dbl})
                        n556 = Unbundle(w843) -> ("Tmp Live"=w842:dbl, "Tmp Neut"=w841:dbl)  [unwired: 3 out]
                        n557 = Bundle(cluster=w845, "TL"=w842, "TN"=w841) -> (w844:cluster{"TL":dbl, "TN":dbl})
                        n558 = local write "TEMP START LAB02-2"(w844) -> ()
                      }
                    }
                  }
                }
              }
              event "RUN LAB03-1": Value Change {
                n559 = event-data() -> ("NewVal"=w846:bool)  [unwired: 1 in, 5 out]
                n560 = local write "run lab03-1"(w846) -> ()
                n561 = case shown="True" w846 {
                  tunnel: w852 -> [_ w885]
                  tunnel: w851 -> [_ w884]
                  tunnel: w849 -> [w854 w883]
                  tunnel: w850 -> [_ w882]
                  tunnel: w848 -> [_ w881]
                  tunnel: [w853 w880] -> w847
                  frame False {
                    # "stop test"
                    n562 = stacked-sequence {
                      tunnel: w854 -> [w863 _]
                      tunnel: [w855 _] -> w853
                      frame #0 {
                        n563 = local read "DISP LAB03-1"() -> (w862:T4)
                        n564 = Unbundle(w862) -> ("CYCLE"=w860:dbl, "MINS"=w861:dbl)  [unwired: 1 out]
                        n565 = case shown="\"CYCLE TEST\"" w863 {
                          tunnel: w861 -> [_ _ w870]
                          tunnel: w860 -> [w868 w869 _]
                          tunnel: [w868 w869 w870] -> w859
                          frame "CHART TEST", Default {
                          }
                          frame "CYCLE TEST" {
                          }
                          frame "T-RISE TEST" {
                          }
                        }
                        n566 = local read "TDMS LAB03-1"() -> (w867:refnum<k34>)
                        n567 = Build Array("STOPPED") -> (w864:string[])
                        n568 = Build Array(w859) -> (w858:dbl[])
                        n569 = TDMS Write(0:w867, 5:"TEST RESULT", 7:w864, 9:w858) -> (4:w856:refnum<k34>, 15:w857:errorcluster)  [unwired: 2 in, 2 out]
                        n570 = TDMS Close(8:w857, 11:w856) -> (0:w855:errorcluster)  [unwired: 1 out]
                      }
                      frame #1 {
                        n571 = local read "DISP LAB03-1"() -> (w874:T4)
                        n572 = stacked-sequence {
                          tunnel: "LAB03-1" -> [w876 w878]
                          frame #0 {
                            n573 = call "sub vi - defrag tdms v1.vi"("panel id"=w876) -> ("error out"=w875:errorcluster)  [unwired: 10 in]
                            n574 = local write "data file error"(w875) -> ()
                          }
                          frame #1 {
                            n575 = call "Save data file to network drive v1.vi"("panel id"=w878) -> ("network file save error"=w877:errorcluster)  [unwired: 9 in, 1 out]
                            n576 = local write "RESULT LAB03-1"(FALSE) -> ()
                            n577 = local write "data file error"(w877) -> ()
                          }
                        }
                        n578 = Bundle(cluster=w874, "STATUS"="STOP") -> (w872:T4)  [unwired: 2 in]
                        n579 = local write "DISP LAB03-1"(w872) -> ()
                      }
                    }
                  }
                  frame True {
                    # "start new test and create test file"
                    n580 = stacked-sequence {
                      seq-local: [w886 _ _ _ _] -> [_ w911 _ _ _]
                      tunnel: w885 -> [w891 _ _ _ _]
                      tunnel: w884 -> [w888 _ _ _ _]
                      tunnel: w883 -> [w901 _ _ _ _]
                      tunnel: w882 -> [w894 _ _ _ _]
                      tunnel: w881 -> [w889 _ _ _ _]
                      tunnel: [_ w905 _ _ _] -> w880
                      frame #0 {
                        w887 = "\\"
                        n581 = local read "SET LAB03-1"() -> (w896:T5)
                        n582 = case shown="\"T-RISE TEST\"" w901 {
                          tunnel: ["L03-1-CHART TEST-" "L03-1-CYCLE TEST-" "L03-1-T-RISE TEST-"] -> w897
                          frame "CHART TEST", Default {
                          }
                          frame "CYCLE TEST" {
                          }
                          frame "T-RISE TEST" {
                          }
                        }
                        n583 = Unbundle(w896) -> ("DESCRIPTION"=w895:string)  [unwired: 4 out]
                        n584 = Concatenate Strings(w891, "\\", w889, w887, w888, w887) -> (w898:string)
                        n585 = String To Path(string=w898) -> (path=w900:path)
                        n586 = Concatenate Strings(w898, w897, w895, "-", w894, ".tdms") -> (w886:string)
                        n587 = Create Folder(path (use dialog)=w900) -> (error out=w899:errorcluster)  [unwired: 2 in, 2 out]
                        n588 = global write "Global 1.vi" "LAB03-1 FILE"(w886) -> ()
                        n589 = call <vilib>:"Clear Errors.vi"("error in (no error)"=w899) -> ()  [unwired: 6 in, 1 out]
                      }
                      frame #1 {
                        n590 = String To Path(string=w911) -> (path=w906:path)
                        n591 = TDMS Open(5:FALSE, 6:FALSE, 10:T18."create or replace" ("operation (0:open)"), 11:w906) -> (0:w905:errorcluster, 3:→"TDMS LAB03-1":refnum<k34>)  [unwired: 3 in]
                      }
                      frame #2 {
                        n592 = local read "SET LAB03-1"() -> (w917:T5)
                        n593 = local read "TDMS LAB03-1"() -> (w928:refnum<k34>)
                        n594 = Build Array("Testers Name", "Description", "Set Test Cycles", "T-Rise minutes", "T-Rise Deg C") -> (w918:string[])
                        n595 = Unbundle(w917) -> ("NAME"=w916:string, "DESCRIPTION"=w915:string, "CYCLES"=w914:dbl, "T-RISE mins"=w913:dbl, "T-RISE deg C"=w912:dbl)
                        n596 = Number To Decimal String(number=w914) -> (decimal integer string=w927:string)  [unwired: 1 in]
                        n597 = Number To Decimal String(number=w913) -> (decimal integer string=w926:string)  [unwired: 1 in]
                        n598 = Number To Decimal String(number=w912) -> (decimal integer string=w925:string)  [unwired: 1 in]
                        n599 = Build Array(w916, w915, w927, w926, w925) -> (w924:string[])
                        n600 = TDMS Set Properties(5:w924, 7:w918, 11:w928) -> ()  [unwired: 3 in, 4 out]
                      }
                      frame #3 {
                        w930 = 0.0
                        n601 = local read "DISP LAB03-1"() -> (w932:T4)
                        n602 = Bundle(cluster=w932, "CYCLE"=w930, "MINS"=w930, "STATUS"="RUN") -> (w931:T4)
                        n603 = local write "DISP LAB03-1"(w931) -> ()
                      }
                      frame #4 {
                        n604 = local read "SIG LAB03-1"() -> (w935:T2)
                        n605 = local read "TEMP START LAB03-1"() -> (w937:cluster{"TL":dbl, "TN":dbl})
                        n606 = Unbundle(w935) -> ("Tmp Live"=w934:dbl, "Tmp Neut"=w933:dbl)  [unwired: 3 out]
                        n607 = Bundle(cluster=w937, "TL"=w934, "TN"=w933) -> (w936:cluster{"TL":dbl, "TN":dbl})
                        n608 = local write "TEMP START LAB03-1"(w936) -> ()
                      }
                    }
                  }
                }
              }
              event "RUN LAB03-2": Value Change {
                n609 = event-data() -> ("NewVal"=w938:bool)  [unwired: 1 in, 5 out]
                n610 = local write "run lab03-2"(w938) -> ()
                n611 = case shown="True" w938 {
                  tunnel: w944 -> [_ w977]
                  tunnel: w943 -> [_ w976]
                  tunnel: w941 -> [w946 w975]
                  tunnel: w942 -> [_ w974]
                  tunnel: w940 -> [_ w973]
                  tunnel: [w945 w972] -> w939
                  frame False {
                    # "stop test"
                    n612 = stacked-sequence {
                      tunnel: w946 -> [w955 _]
                      tunnel: [w947 _] -> w945
                      frame #0 {
                        n613 = local read "DISP LAB03-2"() -> (w954:T4)
                        n614 = Unbundle(w954) -> ("CYCLE"=w952:dbl, "MINS"=w953:dbl)  [unwired: 1 out]
                        n615 = case shown="\"CYCLE TEST\"" w955 {
                          tunnel: w953 -> [_ _ w962]
                          tunnel: w952 -> [w960 w961 _]
                          tunnel: [w960 w961 w962] -> w951
                          frame "CHART TEST", Default {
                          }
                          frame "CYCLE TEST" {
                          }
                          frame "T-RISE TEST" {
                          }
                        }
                        n616 = local read "TDMS LAB03-2"() -> (w959:refnum<k34>)
                        n617 = Build Array("STOPPED") -> (w956:string[])
                        n618 = Build Array(w951) -> (w950:dbl[])
                        n619 = TDMS Write(0:w959, 5:"TEST RESULT", 7:w956, 9:w950) -> (4:w948:refnum<k34>, 15:w949:errorcluster)  [unwired: 2 in, 2 out]
                        n620 = TDMS Close(8:w949, 11:w948) -> (0:w947:errorcluster)  [unwired: 1 out]
                      }
                      frame #1 {
                        n621 = local read "DISP LAB03-2"() -> (w966:T4)
                        n622 = stacked-sequence {
                          tunnel: "LAB03-2" -> [w968 w970]
                          frame #0 {
                            n623 = call "sub vi - defrag tdms v1.vi"("panel id"=w968) -> ("error out"=w967:errorcluster)  [unwired: 10 in]
                            n624 = local write "data file error"(w967) -> ()
                          }
                          frame #1 {
                            n625 = call "Save data file to network drive v1.vi"("panel id"=w970) -> ("network file save error"=w969:errorcluster)  [unwired: 9 in, 1 out]
                            n626 = local write "RESULT LAB03-2"(FALSE) -> ()
                            n627 = local write "data file error"(w969) -> ()
                          }
                        }
                        n628 = Bundle(cluster=w966, "STATUS"="STOP") -> (w964:T4)  [unwired: 2 in]
                        n629 = local write "DISP LAB03-2"(w964) -> ()
                      }
                    }
                  }
                  frame True {
                    # "start new test and create test file"
                    n630 = stacked-sequence {
                      seq-local: [w978 _ _ _ _] -> [_ w1003 _ _ _]
                      tunnel: w977 -> [w983 _ _ _ _]
                      tunnel: w976 -> [w980 _ _ _ _]
                      tunnel: w975 -> [w993 _ _ _ _]
                      tunnel: w974 -> [w986 _ _ _ _]
                      tunnel: w973 -> [w981 _ _ _ _]
                      tunnel: [_ w997 _ _ _] -> w972
                      frame #0 {
                        w979 = "\\"
                        n631 = local read "SET LAB03-2"() -> (w988:T5)
                        n632 = case shown="\"T-RISE TEST\"" w993 {
                          tunnel: ["L03-2-CHART TEST-" "L03-2-CYCLE TEST-" "L03-2-T-RISE TEST-"] -> w989
                          frame "CHART TEST", Default {
                          }
                          frame "CYCLE TEST" {
                          }
                          frame "T-RISE TEST" {
                          }
                        }
                        n633 = Unbundle(w988) -> ("DESCRIPTION"=w987:string)  [unwired: 4 out]
                        n634 = Concatenate Strings(w983, "\\", w981, w979, w980, w979) -> (w990:string)
                        n635 = String To Path(string=w990) -> (path=w992:path)
                        n636 = Concatenate Strings(w990, w989, w987, "-", w986, ".tdms") -> (w978:string)
                        n637 = Create Folder(path (use dialog)=w992) -> (error out=w991:errorcluster)  [unwired: 2 in, 2 out]
                        n638 = global write "Global 1.vi" "LAB03-2 FILE"(w978) -> ()
                        n639 = call <vilib>:"Clear Errors.vi"("error in (no error)"=w991) -> ()  [unwired: 6 in, 1 out]
                      }
                      frame #1 {
                        n640 = String To Path(string=w1003) -> (path=w998:path)
                        n641 = TDMS Open(5:FALSE, 6:FALSE, 10:T18."create or replace" ("operation (0:open)"), 11:w998) -> (0:w997:errorcluster, 3:→"TDMS LAB03-2":refnum<k34>)  [unwired: 3 in]
                      }
                      frame #2 {
                        n642 = local read "SET LAB03-2"() -> (w1009:T5)
                        n643 = local read "TDMS LAB03-2"() -> (w1020:refnum<k34>)
                        n644 = Build Array("Testers Name", "Description", "Set Test Cycles", "T-Rise minutes", "T-Rise Deg C") -> (w1010:string[])
                        n645 = Unbundle(w1009) -> ("NAME"=w1008:string, "DESCRIPTION"=w1007:string, "CYCLES"=w1006:dbl, "T-RISE mins"=w1005:dbl, "T-RISE deg C"=w1004:dbl)
                        n646 = Number To Decimal String(number=w1006) -> (decimal integer string=w1019:string)  [unwired: 1 in]
                        n647 = Number To Decimal String(number=w1005) -> (decimal integer string=w1018:string)  [unwired: 1 in]
                        n648 = Number To Decimal String(number=w1004) -> (decimal integer string=w1017:string)  [unwired: 1 in]
                        n649 = Build Array(w1008, w1007, w1019, w1018, w1017) -> (w1016:string[])
                        n650 = TDMS Set Properties(5:w1016, 7:w1010, 11:w1020) -> ()  [unwired: 3 in, 4 out]
                      }
                      frame #3 {
                        w1022 = 0.0
                        n651 = local read "DISP LAB03-2"() -> (w1024:T4)
                        n652 = Bundle(cluster=w1024, "CYCLE"=w1022, "MINS"=w1022, "STATUS"="RUN") -> (w1023:T4)
                        n653 = local write "DISP LAB03-2"(w1023) -> ()
                      }
                      frame #4 {
                        n654 = local read "SIG LAB03-2"() -> (w1027:T2)
                        n655 = local read "TEMP START LAB03-2"() -> (w1029:cluster{"TL":dbl, "TN":dbl})
                        n656 = Unbundle(w1027) -> ("Tmp Live"=w1026:dbl, "Tmp Neut"=w1025:dbl)  [unwired: 3 out]
                        n657 = Bundle(cluster=w1029, "TL"=w1026, "TN"=w1025) -> (w1028:cluster{"TL":dbl, "TN":dbl})
                        n658 = local write "TEMP START LAB03-2"(w1028) -> ()
                      }
                    }
                  }
                }
              }
              event "RUN LAB04-1": Value Change {
                n659 = event-data() -> ("NewVal"=w1030:bool)  [unwired: 1 in, 5 out]
                n660 = local write "run lab04-1"(w1030) -> ()
                n661 = case shown="True" w1030 {
                  tunnel: w1036 -> [_ w1069]
                  tunnel: w1035 -> [_ w1068]
                  tunnel: w1033 -> [w1038 w1067]
                  tunnel: w1034 -> [_ w1066]
                  tunnel: w1032 -> [_ w1065]
                  tunnel: [w1037 w1064] -> w1031
                  frame False {
                    # "stop test"
                    n662 = stacked-sequence {
                      tunnel: w1038 -> [w1047 _]
                      tunnel: [w1039 _] -> w1037
                      frame #0 {
                        n663 = local read "DISP LAB04-1"() -> (w1046:T4)
                        n664 = Unbundle(w1046) -> ("CYCLE"=w1044:dbl, "MINS"=w1045:dbl)  [unwired: 1 out]
                        n665 = case shown="\"CYCLE TEST\"" w1047 {
                          tunnel: w1045 -> [_ _ w1054]
                          tunnel: w1044 -> [w1052 w1053 _]
                          tunnel: [w1052 w1053 w1054] -> w1043
                          frame "CHART TEST", Default {
                          }
                          frame "CYCLE TEST" {
                          }
                          frame "T-RISE TEST" {
                          }
                        }
                        n666 = local read "TDMS LAB04-1"() -> (w1051:refnum<k34>)
                        n667 = Build Array("STOPPED") -> (w1048:string[])
                        n668 = Build Array(w1043) -> (w1042:dbl[])
                        n669 = TDMS Write(0:w1051, 5:"TEST RESULT", 7:w1048, 9:w1042) -> (4:w1040:refnum<k34>, 15:w1041:errorcluster)  [unwired: 2 in, 2 out]
                        n670 = TDMS Close(8:w1041, 11:w1040) -> (0:w1039:errorcluster)  [unwired: 1 out]
                      }
                      frame #1 {
                        n671 = local read "DISP LAB04-1"() -> (w1058:T4)
                        n672 = stacked-sequence {
                          tunnel: "LAB04-1" -> [w1060 w1062]
                          frame #0 {
                            n673 = call "sub vi - defrag tdms v1.vi"("panel id"=w1060) -> ("error out"=w1059:errorcluster)  [unwired: 10 in]
                            n674 = local write "data file error"(w1059) -> ()
                          }
                          frame #1 {
                            n675 = call "Save data file to network drive v1.vi"("panel id"=w1062) -> ("network file save error"=w1061:errorcluster)  [unwired: 9 in, 1 out]
                            n676 = local write "RESULT LAB04-1"(FALSE) -> ()
                            n677 = local write "data file error"(w1061) -> ()
                          }
                        }
                        n678 = Bundle(cluster=w1058, "STATUS"="STOP") -> (w1056:T4)  [unwired: 2 in]
                        n679 = local write "DISP LAB04-1"(w1056) -> ()
                      }
                    }
                  }
                  frame True {
                    # "start new test and create test file"
                    n680 = stacked-sequence {
                      seq-local: [w1070 _ _ _ _] -> [_ w1095 _ _ _]
                      tunnel: w1069 -> [w1075 _ _ _ _]
                      tunnel: w1068 -> [w1071 _ _ _ _]
                      tunnel: w1067 -> [w1085 _ _ _ _]
                      tunnel: w1066 -> [w1078 _ _ _ _]
                      tunnel: w1065 -> [w1073 _ _ _ _]
                      tunnel: [_ w1089 _ _ _] -> w1064
                      frame #0 {
                        w1072 = "\\"
                        n681 = local read "SET LAB04-1"() -> (w1080:T5)
                        n682 = case shown="\"CYCLE TEST\"" w1085 {
                          tunnel: ["L04-1-CHART TEST-" "L04-1-CYCLE TEST-" "L04-1-T-RISE TEST-"] -> w1081
                          frame "CHART TEST", Default {
                          }
                          frame "CYCLE TEST" {
                          }
                          frame "T-RISE TEST" {
                          }
                        }
                        n683 = Unbundle(w1080) -> ("DESCRIPTION"=w1079:string)  [unwired: 4 out]
                        n684 = Concatenate Strings(w1075, "\\", w1073, w1072, w1071, w1072) -> (w1082:string)
                        n685 = String To Path(string=w1082) -> (path=w1084:path)
                        n686 = Concatenate Strings(w1082, w1081, w1079, "-", w1078, ".tdms") -> (w1070:string)
                        n687 = Create Folder(path (use dialog)=w1084) -> (error out=w1083:errorcluster)  [unwired: 2 in, 2 out]
                        n688 = global write "Global 1.vi" "LAB04-1 FILE"(w1070) -> ()
                        n689 = call <vilib>:"Clear Errors.vi"("error in (no error)"=w1083) -> ()  [unwired: 6 in, 1 out]
                      }
                      frame #1 {
                        n690 = String To Path(string=w1095) -> (path=w1090:path)
                        n691 = TDMS Open(5:FALSE, 6:FALSE, 10:T18."create or replace" ("operation (0:open)"), 11:w1090) -> (0:w1089:errorcluster, 3:→"TDMS LAB04-1":refnum<k34>)  [unwired: 3 in]
                      }
                      frame #2 {
                        n692 = local read "SET LAB04-1"() -> (w1101:T5)
                        n693 = local read "TDMS LAB04-1"() -> (w1112:refnum<k34>)
                        n694 = Build Array("Testers Name", "Description", "Set Test Cycles", "T-Rise minutes", "T-Rise Deg C") -> (w1102:string[])
                        n695 = Unbundle(w1101) -> ("NAME"=w1100:string, "DESCRIPTION"=w1099:string, "CYCLES"=w1098:dbl, "T-RISE mins"=w1097:dbl, "T-RISE deg C"=w1096:dbl)
                        n696 = Number To Decimal String(number=w1098) -> (decimal integer string=w1111:string)  [unwired: 1 in]
                        n697 = Number To Decimal String(number=w1097) -> (decimal integer string=w1110:string)  [unwired: 1 in]
                        n698 = Number To Decimal String(number=w1096) -> (decimal integer string=w1109:string)  [unwired: 1 in]
                        n699 = Build Array(w1100, w1099, w1111, w1110, w1109) -> (w1108:string[])
                        n700 = TDMS Set Properties(5:w1108, 7:w1102, 11:w1112) -> ()  [unwired: 3 in, 4 out]
                      }
                      frame #3 {
                        w1114 = 0.0
                        n701 = local read "DISP LAB04-1"() -> (w1116:T4)
                        n702 = Bundle(cluster=w1116, "CYCLE"=w1114, "MINS"=w1114, "STATUS"="RUN") -> (w1115:T4)
                        n703 = local write "DISP LAB04-1"(w1115) -> ()
                      }
                      frame #4 {
                        n704 = local read "SIG LAB04-1"() -> (w1119:T2)
                        n705 = local read "TEMP START LAB04-1"() -> (w1121:cluster{"TL":dbl, "TN":dbl})
                        n706 = Unbundle(w1119) -> ("Tmp Live"=w1118:dbl, "Tmp Neut"=w1117:dbl)  [unwired: 3 out]
                        n707 = Bundle(cluster=w1121, "TL"=w1118, "TN"=w1117) -> (w1120:cluster{"TL":dbl, "TN":dbl})
                        n708 = local write "TEMP START LAB04-1"(w1120) -> ()
                      }
                    }
                  }
                }
              }
              event "RUN LAB04-2": Value Change {
                n709 = event-data() -> ("NewVal"=w1122:bool)  [unwired: 1 in, 5 out]
                n710 = local write "run lab04-2"(w1122) -> ()
                n711 = case shown="True" w1122 {
                  tunnel: w1128 -> [_ w1161]
                  tunnel: w1127 -> [_ w1160]
                  tunnel: w1125 -> [w1130 w1159]
                  tunnel: w1126 -> [_ w1158]
                  tunnel: w1124 -> [_ w1157]
                  tunnel: [w1129 w1156] -> w1123
                  frame False {
                    # "stop test"
                    n712 = stacked-sequence {
                      tunnel: w1130 -> [w1139 _]
                      tunnel: [w1131 _] -> w1129
                      frame #0 {
                        n713 = local read "DISP LAB04-2"() -> (w1138:T4)
                        n714 = Unbundle(w1138) -> ("CYCLE"=w1136:dbl, "MINS"=w1137:dbl)  [unwired: 1 out]
                        n715 = case shown="\"CYCLE TEST\"" w1139 {
                          tunnel: w1137 -> [_ _ w1146]
                          tunnel: w1136 -> [w1144 w1145 _]
                          tunnel: [w1144 w1145 w1146] -> w1135
                          frame "CHART TEST", Default {
                          }
                          frame "CYCLE TEST" {
                          }
                          frame "T-RISE TEST" {
                          }
                        }
                        n716 = local read "TDMS LAB04-2"() -> (w1143:refnum<k34>)
                        n717 = Build Array("STOPPED") -> (w1140:string[])
                        n718 = Build Array(w1135) -> (w1134:dbl[])
                        n719 = TDMS Write(0:w1143, 5:"TEST RESULT", 7:w1140, 9:w1134) -> (4:w1132:refnum<k34>, 15:w1133:errorcluster)  [unwired: 2 in, 2 out]
                        n720 = TDMS Close(8:w1133, 11:w1132) -> (0:w1131:errorcluster)  [unwired: 1 out]
                      }
                      frame #1 {
                        n721 = local read "DISP LAB04-2"() -> (w1150:T4)
                        n722 = stacked-sequence {
                          tunnel: "LAB04-2" -> [w1152 w1154]
                          frame #0 {
                            n723 = call "sub vi - defrag tdms v1.vi"("panel id"=w1152) -> ("error out"=w1151:errorcluster)  [unwired: 10 in]
                            n724 = local write "data file error"(w1151) -> ()
                          }
                          frame #1 {
                            n725 = call "Save data file to network drive v1.vi"("panel id"=w1154) -> ("network file save error"=w1153:errorcluster)  [unwired: 9 in, 1 out]
                            n726 = local write "RESULT LAB04-2"(FALSE) -> ()
                            n727 = local write "data file error"(w1153) -> ()
                          }
                        }
                        n728 = Bundle(cluster=w1150, "STATUS"="STOP") -> (w1148:T4)  [unwired: 2 in]
                        n729 = local write "DISP LAB04-2"(w1148) -> ()
                      }
                    }
                  }
                  frame True {
                    # "start new test and create test file"
                    n730 = stacked-sequence {
                      seq-local: [w1162 _ _ _ _] -> [_ w1187 _ _ _]
                      tunnel: w1161 -> [w1167 _ _ _ _]
                      tunnel: w1160 -> [w1163 _ _ _ _]
                      tunnel: w1159 -> [w1177 _ _ _ _]
                      tunnel: w1158 -> [w1170 _ _ _ _]
                      tunnel: w1157 -> [w1165 _ _ _ _]
                      tunnel: [_ w1181 _ _ _] -> w1156
                      frame #0 {
                        w1164 = "\\"
                        n731 = local read "SET LAB04-2"() -> (w1172:T5)
                        n732 = case shown="\"CHART TEST\", Default" w1177 {
                          tunnel: ["L04-2-CHART TEST-" "L04-2-CYCLE TEST-" "L04-2-T-RISE TEST-"] -> w1173
                          frame "CHART TEST", Default {
                          }
                          frame "CYCLE TEST" {
                          }
                          frame "T-RISE TEST" {
                          }
                        }
                        n733 = Unbundle(w1172) -> ("DESCRIPTION"=w1171:string)  [unwired: 4 out]
                        n734 = Concatenate Strings(w1167, "\\", w1165, w1164, w1163, w1164) -> (w1174:string)
                        n735 = String To Path(string=w1174) -> (path=w1176:path)
                        n736 = Concatenate Strings(w1174, w1173, w1171, "-", w1170, ".tdms") -> (w1162:string)
                        n737 = Create Folder(path (use dialog)=w1176) -> (error out=w1175:errorcluster)  [unwired: 2 in, 2 out]
                        n738 = global write "Global 1.vi" "LAB04-2 FILE"(w1162) -> ()
                        n739 = call <vilib>:"Clear Errors.vi"("error in (no error)"=w1175) -> ()  [unwired: 6 in, 1 out]
                      }
                      frame #1 {
                        n740 = String To Path(string=w1187) -> (path=w1182:path)
                        n741 = TDMS Open(5:FALSE, 6:FALSE, 10:T18."create or replace" ("operation (0:open)"), 11:w1182) -> (0:w1181:errorcluster, 3:→"TDMS LAB04-2":refnum<k34>)  [unwired: 3 in]
                      }
                      frame #2 {
                        n742 = local read "SET LAB04-2"() -> (w1193:T5)
                        n743 = local read "TDMS LAB04-2"() -> (w1204:refnum<k34>)
                        n744 = Build Array("Testers Name", "Description", "Set Test Cycles", "T-Rise minutes", "T-Rise Deg C") -> (w1194:string[])
                        n745 = Unbundle(w1193) -> ("NAME"=w1192:string, "DESCRIPTION"=w1191:string, "CYCLES"=w1190:dbl, "T-RISE mins"=w1189:dbl, "T-RISE deg C"=w1188:dbl)
                        n746 = Number To Decimal String(number=w1190) -> (decimal integer string=w1203:string)  [unwired: 1 in]
                        n747 = Number To Decimal String(number=w1189) -> (decimal integer string=w1202:string)  [unwired: 1 in]
                        n748 = Number To Decimal String(number=w1188) -> (decimal integer string=w1201:string)  [unwired: 1 in]
                        n749 = Build Array(w1192, w1191, w1203, w1202, w1201) -> (w1200:string[])
                        n750 = TDMS Set Properties(5:w1200, 7:w1194, 11:w1204) -> ()  [unwired: 3 in, 4 out]
                      }
                      frame #3 {
                        w1206 = 0.0
                        n751 = local read "DISP LAB04-2"() -> (w1208:T4)
                        n752 = Bundle(cluster=w1208, "CYCLE"=w1206, "MINS"=w1206, "STATUS"="RUN") -> (w1207:T4)
                        n753 = local write "DISP LAB04-2"(w1207) -> ()
                      }
                      frame #4 {
                        n754 = local read "SIG LAB04-2"() -> (w1211:T2)
                        n755 = local read "TEMP START LAB04-2"() -> (w1213:cluster{"TL":dbl, "TN":dbl})
                        n756 = Unbundle(w1211) -> ("Tmp Live"=w1210:dbl, "Tmp Neut"=w1209:dbl)  [unwired: 3 out]
                        n757 = Bundle(cluster=w1213, "TL"=w1210, "TN"=w1209) -> (w1212:cluster{"TL":dbl, "TN":dbl})
                        n758 = local write "TEMP START LAB04-2"(w1212) -> ()
                      }
                    }
                  }
                }
              }
              event "RUN LAB05-1": Value Change {
                n759 = event-data() -> ("NewVal"=w1214:bool)  [unwired: 1 in, 5 out]
                n760 = local write "run lab05-1"(w1214) -> ()
                n761 = case shown="True" w1214 {
                  tunnel: w1220 -> [_ w1253]
                  tunnel: w1219 -> [_ w1252]
                  tunnel: w1217 -> [w1222 w1251]
                  tunnel: w1218 -> [_ w1250]
                  tunnel: w1216 -> [_ w1249]
                  tunnel: [w1221 w1248] -> w1215
                  frame False {
                    # "stop test"
                    n762 = stacked-sequence {
                      tunnel: w1222 -> [w1231 _]
                      tunnel: [w1223 _] -> w1221
                      frame #0 {
                        n763 = local read "DISP LAB05-1"() -> (w1230:T4)
                        n764 = Unbundle(w1230) -> ("CYCLE"=w1228:dbl, "MINS"=w1229:dbl)  [unwired: 1 out]
                        n765 = case shown="\"CYCLE TEST\"" w1231 {
                          tunnel: w1229 -> [_ _ w1238]
                          tunnel: w1228 -> [w1236 w1237 _]
                          tunnel: [w1236 w1237 w1238] -> w1227
                          frame "CHART TEST", Default {
                          }
                          frame "CYCLE TEST" {
                          }
                          frame "T-RISE TEST" {
                          }
                        }
                        n766 = local read "TDMS LAB05-1"() -> (w1235:refnum<k34>)
                        n767 = Build Array("STOPPED") -> (w1232:string[])
                        n768 = Build Array(w1227) -> (w1226:dbl[])
                        n769 = TDMS Write(0:w1235, 5:"TEST RESULT", 7:w1232, 9:w1226) -> (4:w1224:refnum<k34>, 15:w1225:errorcluster)  [unwired: 2 in, 2 out]
                        n770 = TDMS Close(8:w1225, 11:w1224) -> (0:w1223:errorcluster)  [unwired: 1 out]
                      }
                      frame #1 {
                        n771 = local read "DISP LAB05-1"() -> (w1242:T4)
                        n772 = stacked-sequence {
                          tunnel: "LAB05-1" -> [w1244 w1246]
                          frame #0 {
                            n773 = call "sub vi - defrag tdms v1.vi"("panel id"=w1244) -> ("error out"=w1243:errorcluster)  [unwired: 10 in]
                            n774 = local write "data file error"(w1243) -> ()
                          }
                          frame #1 {
                            n775 = call "Save data file to network drive v1.vi"("panel id"=w1246) -> ("network file save error"=w1245:errorcluster)  [unwired: 9 in, 1 out]
                            n776 = local write "RESULT LAB05-1"(FALSE) -> ()
                            n777 = local write "data file error"(w1245) -> ()
                          }
                        }
                        n778 = Bundle(cluster=w1242, "STATUS"="STOP") -> (w1240:T4)  [unwired: 2 in]
                        n779 = local write "DISP LAB05-1"(w1240) -> ()
                      }
                    }
                  }
                  frame True {
                    # "start new test and create test file"
                    n780 = stacked-sequence {
                      seq-local: [w1254 _ _ _ _] -> [_ w1279 _ _ _]
                      tunnel: w1253 -> [w1259 _ _ _ _]
                      tunnel: w1252 -> [w1255 _ _ _ _]
                      tunnel: w1251 -> [w1269 _ _ _ _]
                      tunnel: w1250 -> [w1262 _ _ _ _]
                      tunnel: w1249 -> [w1257 _ _ _ _]
                      tunnel: [_ w1273 _ _ _] -> w1248
                      frame #0 {
                        w1256 = "\\"
                        n781 = local read "SET LAB05-1"() -> (w1264:T5)
                        n782 = case shown="\"CYCLE TEST\"" w1269 {
                          tunnel: ["L05-1-CHART TEST-" "L05-1-CYCLE TEST-" "L05-1-T-RISE TEST-"] -> w1265
                          frame "CHART TEST", Default {
                          }
                          frame "CYCLE TEST" {
                          }
                          frame "T-RISE TEST" {
                          }
                        }
                        n783 = Unbundle(w1264) -> ("DESCRIPTION"=w1263:string)  [unwired: 4 out]
                        n784 = Concatenate Strings(w1259, "\\", w1257, w1256, w1255, w1256) -> (w1266:string)
                        n785 = String To Path(string=w1266) -> (path=w1268:path)
                        n786 = Concatenate Strings(w1266, w1265, w1263, "-", w1262, ".tdms") -> (w1254:string)
                        n787 = Create Folder(path (use dialog)=w1268) -> (error out=w1267:errorcluster)  [unwired: 2 in, 2 out]
                        n788 = global write "Global 1.vi" "LAB05-1 FILE"(w1254) -> ()
                        n789 = call <vilib>:"Clear Errors.vi"("error in (no error)"=w1267) -> ()  [unwired: 6 in, 1 out]
                      }
                      frame #1 {
                        n790 = String To Path(string=w1279) -> (path=w1274:path)
                        n791 = TDMS Open(5:FALSE, 6:FALSE, 10:T18."create or replace" ("operation (0:open)"), 11:w1274) -> (0:w1273:errorcluster, 3:→"TDMS LAB05-1":refnum<k34>)  [unwired: 3 in]
                      }
                      frame #2 {
                        n792 = local read "SET LAB05-1"() -> (w1285:T5)
                        n793 = local read "TDMS LAB05-1"() -> (w1296:refnum<k34>)
                        n794 = Build Array("Testers Name", "Description", "Set Test Cycles", "T-Rise minutes", "T-Rise Deg C") -> (w1286:string[])
                        n795 = Unbundle(w1285) -> ("NAME"=w1284:string, "DESCRIPTION"=w1283:string, "CYCLES"=w1282:dbl, "T-RISE mins"=w1281:dbl, "T-RISE deg C"=w1280:dbl)
                        n796 = Number To Decimal String(number=w1282) -> (decimal integer string=w1295:string)  [unwired: 1 in]
                        n797 = Number To Decimal String(number=w1281) -> (decimal integer string=w1294:string)  [unwired: 1 in]
                        n798 = Number To Decimal String(number=w1280) -> (decimal integer string=w1293:string)  [unwired: 1 in]
                        n799 = Build Array(w1284, w1283, w1295, w1294, w1293) -> (w1292:string[])
                        n800 = TDMS Set Properties(5:w1292, 7:w1286, 11:w1296) -> ()  [unwired: 3 in, 4 out]
                      }
                      frame #3 {
                        w1298 = 0.0
                        n801 = local read "DISP LAB05-1"() -> (w1300:T4)
                        n802 = Bundle(cluster=w1300, "CYCLE"=w1298, "MINS"=w1298, "STATUS"="RUN") -> (w1299:T4)
                        n803 = local write "DISP LAB05-1"(w1299) -> ()
                      }
                      frame #4 {
                        n804 = local read "SIG LAB05-1"() -> (w1303:T2)
                        n805 = local read "TEMP START LAB05-1"() -> (w1305:cluster{"TL":dbl, "TN":dbl})
                        n806 = Unbundle(w1303) -> ("Tmp Live"=w1302:dbl, "Tmp Neut"=w1301:dbl)  [unwired: 3 out]
                        n807 = Bundle(cluster=w1305, "TL"=w1302, "TN"=w1301) -> (w1304:cluster{"TL":dbl, "TN":dbl})
                        n808 = local write "TEMP START LAB05-1"(w1304) -> ()
                      }
                    }
                  }
                }
              }
              event "RUN LAB05-2": Value Change {
                n809 = event-data() -> ("NewVal"=w1306:bool)  [unwired: 1 in, 5 out]
                n810 = local write "run lab05-2"(w1306) -> ()
                n811 = case shown="True" w1306 {
                  tunnel: w1312 -> [_ w1345]
                  tunnel: w1311 -> [_ w1344]
                  tunnel: w1309 -> [w1314 w1343]
                  tunnel: w1310 -> [_ w1342]
                  tunnel: w1308 -> [_ w1341]
                  tunnel: [w1313 w1340] -> w1307
                  frame False {
                    # "stop test"
                    n812 = stacked-sequence {
                      tunnel: w1314 -> [w1323 _]
                      tunnel: [w1315 _] -> w1313
                      frame #0 {
                        n813 = local read "DISP LAB05-2"() -> (w1322:T4)
                        n814 = Unbundle(w1322) -> ("CYCLE"=w1320:dbl, "MINS"=w1321:dbl)  [unwired: 1 out]
                        n815 = case shown="\"CYCLE TEST\"" w1323 {
                          tunnel: w1321 -> [_ _ w1330]
                          tunnel: w1320 -> [w1328 w1329 _]
                          tunnel: [w1328 w1329 w1330] -> w1319
                          frame "CHART TEST", Default {
                          }
                          frame "CYCLE TEST" {
                          }
                          frame "T-RISE TEST" {
                          }
                        }
                        n816 = local read "TDMS LAB05-2"() -> (w1327:refnum<k34>)
                        n817 = Build Array("STOPPED") -> (w1324:string[])
                        n818 = Build Array(w1319) -> (w1318:dbl[])
                        n819 = TDMS Write(0:w1327, 5:"TEST RESULT", 7:w1324, 9:w1318) -> (4:w1316:refnum<k34>, 15:w1317:errorcluster)  [unwired: 2 in, 2 out]
                        n820 = TDMS Close(8:w1317, 11:w1316) -> (0:w1315:errorcluster)  [unwired: 1 out]
                      }
                      frame #1 {
                        n821 = local read "DISP LAB05-2"() -> (w1334:T4)
                        n822 = stacked-sequence {
                          tunnel: "LAB05-2" -> [w1336 w1338]
                          frame #0 {
                            n823 = call "sub vi - defrag tdms v1.vi"("panel id"=w1336) -> ("error out"=w1335:errorcluster)  [unwired: 10 in]
                            n824 = local write "data file error"(w1335) -> ()
                          }
                          frame #1 {
                            n825 = local write "RESULT LAB05-2"(FALSE) -> ()
                            n826 = call "Save data file to network drive v1.vi"("panel id"=w1338) -> ("network file save error"=w1337:errorcluster)  [unwired: 9 in, 1 out]
                            n827 = local write "data file error"(w1337) -> ()
                          }
                        }
                        n828 = Bundle(cluster=w1334, "STATUS"="STOP") -> (w1332:T4)  [unwired: 2 in]
                        n829 = local write "DISP LAB05-2"(w1332) -> ()
                      }
                    }
                  }
                  frame True {
                    # "start new test and create test file"
                    n830 = stacked-sequence {
                      seq-local: [w1346 _ _ _ _] -> [_ w1371 _ _ _]
                      tunnel: w1345 -> [w1351 _ _ _ _]
                      tunnel: w1344 -> [w1347 _ _ _ _]
                      tunnel: w1343 -> [w1361 _ _ _ _]
                      tunnel: w1342 -> [w1354 _ _ _ _]
                      tunnel: w1341 -> [w1349 _ _ _ _]
                      tunnel: [_ w1365 _ _ _] -> w1340
                      frame #0 {
                        w1348 = "\\"
                        n831 = local read "SET LAB05-2"() -> (w1356:T5)
                        n832 = case shown="\"CYCLE TEST\"" w1361 {
                          tunnel: ["L05-2-CHART TEST-" "L05-2-CYCLE TEST-" "L05-2-T-RISE TEST-"] -> w1357
                          frame "CHART TEST", Default {
                          }
                          frame "CYCLE TEST" {
                          }
                          frame "T-RISE TEST" {
                          }
                        }
                        n833 = Unbundle(w1356) -> ("DESCRIPTION"=w1355:string)  [unwired: 4 out]
                        n834 = Concatenate Strings(w1351, "\\", w1349, w1348, w1347, w1348) -> (w1358:string)
                        n835 = String To Path(string=w1358) -> (path=w1360:path)
                        n836 = Concatenate Strings(w1358, w1357, w1355, "-", w1354, ".tdms") -> (w1346:string)
                        n837 = Create Folder(path (use dialog)=w1360) -> (error out=w1359:errorcluster)  [unwired: 2 in, 2 out]
                        n838 = global write "Global 1.vi" "LAB05-2 FILE"(w1346) -> ()
                        n839 = call <vilib>:"Clear Errors.vi"("error in (no error)"=w1359) -> ()  [unwired: 6 in, 1 out]
                      }
                      frame #1 {
                        n840 = String To Path(string=w1371) -> (path=w1366:path)
                        n841 = TDMS Open(5:FALSE, 6:FALSE, 10:T18."create or replace" ("operation (0:open)"), 11:w1366) -> (0:w1365:errorcluster, 3:→"TDMS LAB05-2":refnum<k34>)  [unwired: 3 in]
                      }
                      frame #2 {
                        n842 = local read "SET LAB05-2"() -> (w1377:T5)
                        n843 = local read "TDMS LAB05-2"() -> (w1388:refnum<k34>)
                        n844 = Build Array("Testers Name", "Description", "Set Test Cycles", "T-Rise minutes", "T-Rise Deg C") -> (w1378:string[])
                        n845 = Unbundle(w1377) -> ("NAME"=w1376:string, "DESCRIPTION"=w1375:string, "CYCLES"=w1374:dbl, "T-RISE mins"=w1373:dbl, "T-RISE deg C"=w1372:dbl)
                        n846 = Number To Decimal String(number=w1374) -> (decimal integer string=w1387:string)  [unwired: 1 in]
                        n847 = Number To Decimal String(number=w1373) -> (decimal integer string=w1386:string)  [unwired: 1 in]
                        n848 = Number To Decimal String(number=w1372) -> (decimal integer string=w1385:string)  [unwired: 1 in]
                        n849 = Build Array(w1376, w1375, w1387, w1386, w1385) -> (w1384:string[])
                        n850 = TDMS Set Properties(5:w1384, 7:w1378, 11:w1388) -> ()  [unwired: 3 in, 4 out]
                      }
                      frame #3 {
                        w1390 = 0.0
                        n851 = local read "DISP LAB05-2"() -> (w1392:T4)
                        n852 = Bundle(cluster=w1392, "CYCLE"=w1390, "MINS"=w1390, "STATUS"="RUN") -> (w1391:T4)
                        n853 = local write "DISP LAB05-2"(w1391) -> ()
                      }
                      frame #4 {
                        n854 = local read "SIG LAB05-2"() -> (w1395:T2)
                        n855 = local read "TEMP START LAB05-2"() -> (w1397:cluster{"TL":dbl, "TN":dbl})
                        n856 = Unbundle(w1395) -> ("Tmp Live"=w1394:dbl, "Tmp Neut"=w1393:dbl)  [unwired: 3 out]
                        n857 = Bundle(cluster=w1397, "TL"=w1394, "TN"=w1393) -> (w1396:cluster{"TL":dbl, "TN":dbl})
                        n858 = local write "TEMP START LAB05-2"(w1396) -> ()
                      }
                    }
                  }
                }
              }
            }
            n859 = local write "data file error"(w449) -> ()
          }
          frame #4 {
            # "check if test cycles reached for cycle tests, if so then test pass"
            n860 = stacked-sequence {
              tunnel: w1417 -> [_ _ _ _ _ _ _ _ _ _]
              tunnel: w1416 -> [_ _ _ _ _ _ _ _ _ _]
              tunnel: w1415 -> [_ _ _ _ _ _ _ _ _ _]
              tunnel: w1414 -> [_ _ _ _ _ _ _ _ _ _]
              tunnel: w1413 -> [_ _ _ _ _ _ _ _ _ _]
              tunnel: w1412 -> [_ _ _ _ _ _ _ _ _ _]
              tunnel: w1411 -> [_ _ _ _ _ _ _ _ _ _]
              tunnel: w1410 -> [_ _ _ _ _ _ _ _ _ _]
              tunnel: w1409 -> [_ _ _ _ _ _ _ _ _ _]
              tunnel: w1408 -> [_ _ _ _ _ _ _ _ _ _]
              tunnel: w1407 -> [w1423 _ _ _ _ _ _ _ _ _]
              tunnel: w1406 -> [_ w1458 _ _ _ _ _ _ _ _]
              tunnel: w1405 -> [_ _ w1498 _ _ _ _ _ _ _]
              tunnel: w1404 -> [_ _ _ w1538 _ _ _ _ _ _]
              tunnel: w1403 -> [_ _ _ _ w1578 _ _ _ _ _]
              tunnel: w1402 -> [_ _ _ _ _ w1618 _ _ _ _]
              tunnel: w1401 -> [_ _ _ _ _ _ w1658 _ _ _]
              tunnel: w1400 -> [_ _ _ _ _ _ _ w1698 _ _]
              tunnel: w1399 -> [_ _ _ _ _ _ _ _ w1738 _]
              tunnel: w1398 -> [_ _ _ _ _ _ _ _ _ w1778]
              frame #0 {
                # "LAB01-1"
                n861 = Less?(x=w1423, y=2) -> (x < y?=w1421:bool)
                n862 = local read "DISP LAB01-1"() -> (w1424:T4)
                n863 = Unbundle(w1424) -> ("STATUS"=w1418:string)  [unwired: 2 out]
                n864 = Equal?(x=w1418, y="RUN") -> (x = y?=w1420:bool)
                n865 = And(x=w1420, y=w1421) -> (x .and. y?=w1419:bool)
                n866 = case shown="True" w1419 {
                  tunnel: w1424 -> [_ w1429]
                  tunnel: w1423 -> [_ w1433]
                  frame False {
                  }
                  frame True {
                    n867 = local read "SET LAB01-1"() -> (w1435:T5)
                    n868 = local read "TDMS LAB01-1"() -> (w1428:refnum<k34>)
                    n869 = Unbundle(w1435) -> ("CYCLES"=w1426:dbl, "T-RISE mins"=w1432:dbl)  [unwired: 3 out]
                    n870 = case shown="\"CYCLE TEST\"" w1433 {
                      tunnel: w1432 -> [_ _ w1442]
                      tunnel: [w1437 w1439 w1442] -> w1431
                      tunnel: w1426 -> [w1437 w1439 _]
                      tunnel: ["CHART PASS" "CYCLE PASS" "T-RISE PASS"] -> w1430
                      frame "CHART TEST", Default {
                      }
                      frame "CYCLE TEST" {
                      }
                      frame "T-RISE TEST" {
                      }
                    }
                    n871 = Unbundle(w1429) -> ("CYCLE"=w1434:dbl)  [unwired: 2 out]
                    n872 = Increment(x=w1426) -> (x+1=w1427:dbl)
                    n873 = Greater Or Equal?(x=w1434, y=w1427) -> (x >= y?=w1436:bool)
                    n874 = case shown="True" w1436 {
                      tunnel: w1431 -> [w1446 _]
                      tunnel: w1430 -> [w1445 _]
                      tunnel: w1429 -> [w1444 _]
                      tunnel: w1428 -> [w1443 _]
                      frame True {
                        n875 = stacked-sequence {
                          tunnel: w1446 -> [w1450 _]
                          tunnel: w1445 -> [w1448 w1454]
                          tunnel: w1444 -> [_ w1457]
                          tunnel: w1443 -> [w1447 _]
                          frame #0 {
                            n876 = Build Array(w1448) -> (w1451:string[])
                            n877 = Build Array(w1450) -> (w1449:dbl[])
                            n878 = TDMS Write(0:w1447, 5:"TEST PASS", 7:w1451, 9:w1449) -> (15:w1453:errorcluster)  [unwired: 2 in, 3 out]
                            n879 = local write "data file error"(w1453) -> ()
                          }
                          frame #1 {
                            n880 = Bundle(cluster=w1457, "STATUS"=w1454) -> (w1455:T4)  [unwired: 2 in]
                            n881 = local write "RESULT LAB01-1"(TRUE) -> ()
                            n882 = local write "DISP LAB01-1"(w1455) -> ()
                          }
                        }
                      }
                      frame False {
                      }
                    }
                  }
                }
              }
              frame #1 {
                # "LAB01-2"
                n883 = Less?(x=w1458, y=2) -> (x < y?=w1461:bool)
                n884 = local read "DISP LAB01-2"() -> (w1463:T4)
                n885 = Unbundle(w1463) -> ("STATUS"=w1464:string)  [unwired: 2 out]
                n886 = Equal?(x=w1464, y="RUN") -> (x = y?=w1460:bool)
                n887 = And(x=w1460, y=w1461) -> (x .and. y?=w1459:bool)
                n888 = case shown="True" w1459 {
                  tunnel: w1463 -> [_ w1469]
                  tunnel: w1458 -> [_ w1473]
                  frame False {
                  }
                  frame True {
                    n889 = local read "SET LAB01-2"() -> (w1475:T5)
                    n890 = local read "TDMS LAB01-2"() -> (w1468:refnum<k34>)
                    n891 = Unbundle(w1475) -> ("CYCLES"=w1466:dbl, "T-RISE mins"=w1472:dbl)  [unwired: 3 out]
                    n892 = case shown="\"T-RISE TEST\"" w1473 {
                      tunnel: w1472 -> [_ _ w1482]
                      tunnel: [w1477 w1479 w1482] -> w1471
                      tunnel: w1466 -> [w1477 w1479 _]
                      tunnel: ["CHART PASS" "CYCLE PASS" "T-RISE PASS"] -> w1470
                      frame "CHART TEST", Default {
                      }
                      frame "CYCLE TEST" {
                      }
                      frame "T-RISE TEST" {
                      }
                    }
                    n893 = Unbundle(w1469) -> ("CYCLE"=w1474:dbl)  [unwired: 2 out]
                    n894 = Increment(x=w1466) -> (x+1=w1467:dbl)
                    n895 = Greater Or Equal?(x=w1474, y=w1467) -> (x >= y?=w1476:bool)
                    n896 = case shown="True" w1476 {
                      tunnel: w1471 -> [w1486 _]
                      tunnel: w1470 -> [w1485 _]
                      tunnel: w1469 -> [w1484 _]
                      tunnel: w1468 -> [w1483 _]
                      frame True {
                        n897 = stacked-sequence {
                          tunnel: w1486 -> [w1490 _]
                          tunnel: w1485 -> [w1488 w1494]
                          tunnel: w1484 -> [_ w1497]
                          tunnel: w1483 -> [w1487 _]
                          frame #0 {
                            n898 = Build Array(w1488) -> (w1491:string[])
                            n899 = Build Array(w1490) -> (w1489:dbl[])
                            n900 = TDMS Write(0:w1487, 5:"TEST PASS", 7:w1491, 9:w1489) -> (15:w1493:errorcluster)  [unwired: 2 in, 3 out]
                            n901 = local write "data file error"(w1493) -> ()
                          }
                          frame #1 {
                            n902 = Bundle(cluster=w1497, "STATUS"=w1494) -> (w1495:T4)  [unwired: 2 in]
                            n903 = local write "RESULT LAB01-2"(TRUE) -> ()
                            n904 = local write "DISP LAB01-2"(w1495) -> ()
                          }
                        }
                      }
                      frame False {
                      }
                    }
                  }
                }
              }
              frame #2 {
                # "LAB02-1"
                n905 = Less?(x=w1498, y=2) -> (x < y?=w1501:bool)
                n906 = local read "DISP LAB02-1"() -> (w1503:T4)
                n907 = Unbundle(w1503) -> ("STATUS"=w1504:string)  [unwired: 2 out]
                n908 = Equal?(x=w1504, y="RUN") -> (x = y?=w1500:bool)
                n909 = And(x=w1500, y=w1501) -> (x .and. y?=w1499:bool)
                n910 = case shown="True" w1499 {
                  tunnel: w1503 -> [_ w1509]
                  tunnel: w1498 -> [_ w1513]
                  frame False {
                  }
                  frame True {
                    n911 = local read "SET LAB02-1"() -> (w1515:T5)
                    n912 = local read "TDMS LAB02-1"() -> (w1508:refnum<k34>)
                    n913 = Unbundle(w1509) -> ("CYCLE"=w1514:dbl)  [unwired: 2 out]
                    n914 = Unbundle(w1515) -> ("CYCLES"=w1506:dbl, "T-RISE mins"=w1512:dbl)  [unwired: 3 out]
                    n915 = case shown="\"T-RISE TEST\"" w1513 {
                      tunnel: w1512 -> [_ _ w1522]
                      tunnel: [w1517 w1519 w1522] -> w1511
                      tunnel: w1506 -> [w1517 w1519 _]
                      tunnel: ["CHART PASS" "CYCLE PASS" "T-RISE PASS"] -> w1510
                      frame "CHART TEST", Default {
                      }
                      frame "CYCLE TEST" {
                      }
                      frame "T-RISE TEST" {
                      }
                    }
                    n916 = Increment(x=w1506) -> (x+1=w1507:dbl)
                    n917 = Greater Or Equal?(x=w1514, y=w1507) -> (x >= y?=w1516:bool)
                    n918 = case shown="True" w1516 {
                      tunnel: w1511 -> [w1526 _]
                      tunnel: w1510 -> [w1525 _]
                      tunnel: w1509 -> [w1524 _]
                      tunnel: w1508 -> [w1523 _]
                      frame True {
                        n919 = stacked-sequence {
                          tunnel: w1526 -> [w1530 _]
                          tunnel: w1525 -> [w1528 w1534]
                          tunnel: w1524 -> [_ w1537]
                          tunnel: w1523 -> [w1527 _]
                          frame #0 {
                            n920 = Build Array(w1528) -> (w1531:string[])
                            n921 = Build Array(w1530) -> (w1529:dbl[])
                            n922 = TDMS Write(0:w1527, 5:"TEST PASS", 7:w1531, 9:w1529) -> (15:w1533:errorcluster)  [unwired: 2 in, 3 out]
                            n923 = local write "data file error"(w1533) -> ()
                          }
                          frame #1 {
                            n924 = Bundle(cluster=w1537, "STATUS"=w1534) -> (w1535:T4)  [unwired: 2 in]
                            n925 = local write "RESULT LAB02-1"(TRUE) -> ()
                            n926 = local write "DISP LAB02-1"(w1535) -> ()
                          }
                        }
                      }
                      frame False {
                      }
                    }
                  }
                }
              }
              frame #3 {
                # "LAB02-2"
                n927 = Less?(x=w1538, y=2) -> (x < y?=w1541:bool)
                n928 = local read "DISP LAB02-2"() -> (w1543:T4)
                n929 = Unbundle(w1543) -> ("STATUS"=w1544:string)  [unwired: 2 out]
                n930 = Equal?(x=w1544, y="RUN") -> (x = y?=w1540:bool)
                n931 = And(x=w1540, y=w1541) -> (x .and. y?=w1539:bool)
                n932 = case shown="True" w1539 {
                  tunnel: w1543 -> [_ w1549]
                  tunnel: w1538 -> [_ w1553]
                  frame False {
                  }
                  frame True {
                    n933 = local read "SET LAB02-2"() -> (w1555:T5)
                    n934 = local read "TDMS LAB02-2"() -> (w1548:refnum<k34>)
                    n935 = Unbundle(w1549) -> ("CYCLE"=w1554:dbl)  [unwired: 2 out]
                    n936 = Unbundle(w1555) -> ("CYCLES"=w1546:dbl, "T-RISE mins"=w1552:dbl)  [unwired: 3 out]
                    n937 = case shown="\"T-RISE TEST\"" w1553 {
                      tunnel: w1552 -> [_ _ w1562]
                      tunnel: [w1557 w1559 w1562] -> w1551
                      tunnel: w1546 -> [w1557 w1559 _]
                      tunnel: ["CHART PASS" "CYCLE PASS" "T-RISE PASS"] -> w1550
                      frame "CHART TEST", Default {
                      }
                      frame "CYCLE TEST" {
                      }
                      frame "T-RISE TEST" {
                      }
                    }
                    n938 = Increment(x=w1546) -> (x+1=w1547:dbl)
                    n939 = Greater Or Equal?(x=w1554, y=w1547) -> (x >= y?=w1556:bool)
                    n940 = case shown="True" w1556 {
                      tunnel: w1551 -> [w1566 _]
                      tunnel: w1550 -> [w1565 _]
                      tunnel: w1549 -> [w1564 _]
                      tunnel: w1548 -> [w1563 _]
                      frame True {
                        n941 = stacked-sequence {
                          tunnel: w1566 -> [w1570 _]
                          tunnel: w1565 -> [w1568 w1574]
                          tunnel: w1564 -> [_ w1577]
                          tunnel: w1563 -> [w1567 _]
                          frame #0 {
                            n942 = Build Array(w1568) -> (w1571:string[])
                            n943 = Build Array(w1570) -> (w1569:dbl[])
                            n944 = TDMS Write(0:w1567, 5:"TEST PASS", 7:w1571, 9:w1569) -> (15:w1573:errorcluster)  [unwired: 2 in, 3 out]
                            n945 = local write "data file error"(w1573) -> ()
                          }
                          frame #1 {
                            n946 = Bundle(cluster=w1577, "STATUS"=w1574) -> (w1575:T4)  [unwired: 2 in]
                            n947 = local write "RESULT LAB02-2"(TRUE) -> ()
                            n948 = local write "DISP LAB02-2"(w1575) -> ()
                          }
                        }
                      }
                      frame False {
                      }
                    }
                  }
                }
              }
              frame #4 {
                # "LAB03-1"
                n949 = Less?(x=w1578, y=2) -> (x < y?=w1581:bool)
                n950 = local read "DISP LAB03-1"() -> (w1583:T4)
                n951 = Unbundle(w1583) -> ("STATUS"=w1584:string)  [unwired: 2 out]
                n952 = Equal?(x=w1584, y="RUN") -> (x = y?=w1580:bool)
                n953 = And(x=w1580, y=w1581) -> (x .and. y?=w1579:bool)
                n954 = case shown="True" w1579 {
                  tunnel: w1583 -> [_ w1589]
                  tunnel: w1578 -> [_ w1593]
                  frame False {
                  }
                  frame True {
                    n955 = local read "SET LAB03-1"() -> (w1595:T5)
                    n956 = local read "TDMS LAB03-1"() -> (w1588:refnum<k34>)
                    n957 = Unbundle(w1589) -> ("CYCLE"=w1594:dbl)  [unwired: 2 out]
                    n958 = Unbundle(w1595) -> ("CYCLES"=w1586:dbl, "T-RISE mins"=w1592:dbl)  [unwired: 3 out]
                    n959 = case shown="\"T-RISE TEST\"" w1593 {
                      tunnel: w1592 -> [_ _ w1602]
                      tunnel: [w1597 w1599 w1602] -> w1591
                      tunnel: w1586 -> [w1597 w1599 _]
                      tunnel: ["CHART PASS" "CYCLE PASS" "T-RISE PASS"] -> w1590
                      frame "CHART TEST", Default {
                      }
                      frame "CYCLE TEST" {
                      }
                      frame "T-RISE TEST" {
                      }
                    }
                    n960 = Increment(x=w1586) -> (x+1=w1587:dbl)
                    n961 = Greater Or Equal?(x=w1594, y=w1587) -> (x >= y?=w1596:bool)
                    n962 = case shown="True" w1596 {
                      tunnel: w1591 -> [w1606 _]
                      tunnel: w1590 -> [w1605 _]
                      tunnel: w1589 -> [w1604 _]
                      tunnel: w1588 -> [w1603 _]
                      frame True {
                        n963 = stacked-sequence {
                          tunnel: w1606 -> [w1610 _]
                          tunnel: w1605 -> [w1608 w1614]
                          tunnel: w1604 -> [_ w1617]
                          tunnel: w1603 -> [w1607 _]
                          frame #0 {
                            n964 = Build Array(w1608) -> (w1611:string[])
                            n965 = Build Array(w1610) -> (w1609:dbl[])
                            n966 = TDMS Write(0:w1607, 5:"TEST PASS", 7:w1611, 9:w1609) -> (15:w1613:errorcluster)  [unwired: 2 in, 3 out]
                            n967 = local write "data file error"(w1613) -> ()
                          }
                          frame #1 {
                            n968 = Bundle(cluster=w1617, "STATUS"=w1614) -> (w1615:T4)  [unwired: 2 in]
                            n969 = local write "RESULT LAB03-1"(TRUE) -> ()
                            n970 = local write "DISP LAB03-1"(w1615) -> ()
                          }
                        }
                      }
                      frame False {
                      }
                    }
                  }
                }
              }
              frame #5 {
                # "LAB03-2"
                n971 = Less?(x=w1618, y=2) -> (x < y?=w1621:bool)
                n972 = local read "DISP LAB03-2"() -> (w1623:T4)
                n973 = Unbundle(w1623) -> ("STATUS"=w1624:string)  [unwired: 2 out]
                n974 = Equal?(x=w1624, y="RUN") -> (x = y?=w1620:bool)
                n975 = And(x=w1620, y=w1621) -> (x .and. y?=w1619:bool)
                n976 = case shown="True" w1619 {
                  tunnel: w1623 -> [_ w1629]
                  tunnel: w1618 -> [_ w1633]
                  frame False {
                  }
                  frame True {
                    n977 = local read "SET LAB03-2"() -> (w1635:T5)
                    n978 = local read "TDMS LAB03-2"() -> (w1628:refnum<k34>)
                    n979 = Unbundle(w1629) -> ("CYCLE"=w1634:dbl)  [unwired: 2 out]
                    n980 = Unbundle(w1635) -> ("CYCLES"=w1626:dbl, "T-RISE mins"=w1632:dbl)  [unwired: 3 out]
                    n981 = case shown="\"T-RISE TEST\"" w1633 {
                      tunnel: w1632 -> [_ _ w1642]
                      tunnel: [w1637 w1639 w1642] -> w1631
                      tunnel: w1626 -> [w1637 w1639 _]
                      tunnel: ["CHART PASS" "CYCLE PASS" "T-RISE PASS"] -> w1630
                      frame "CHART TEST", Default {
                      }
                      frame "CYCLE TEST" {
                      }
                      frame "T-RISE TEST" {
                      }
                    }
                    n982 = Increment(x=w1626) -> (x+1=w1627:dbl)
                    n983 = Greater Or Equal?(x=w1634, y=w1627) -> (x >= y?=w1636:bool)
                    n984 = case shown="True" w1636 {
                      tunnel: w1631 -> [w1646 _]
                      tunnel: w1630 -> [w1645 _]
                      tunnel: w1629 -> [w1644 _]
                      tunnel: w1628 -> [w1643 _]
                      frame True {
                        n985 = stacked-sequence {
                          tunnel: w1646 -> [w1650 _]
                          tunnel: w1645 -> [w1648 w1654]
                          tunnel: w1644 -> [_ w1657]
                          tunnel: w1643 -> [w1647 _]
                          frame #0 {
                            n986 = Build Array(w1648) -> (w1651:string[])
                            n987 = Build Array(w1650) -> (w1649:dbl[])
                            n988 = TDMS Write(0:w1647, 5:"TEST PASS", 7:w1651, 9:w1649) -> (15:w1653:errorcluster)  [unwired: 2 in, 3 out]
                            n989 = local write "data file error"(w1653) -> ()
                          }
                          frame #1 {
                            n990 = Bundle(cluster=w1657, "STATUS"=w1654) -> (w1655:T4)  [unwired: 2 in]
                            n991 = local write "RESULT LAB03-2"(TRUE) -> ()
                            n992 = local write "DISP LAB03-2"(w1655) -> ()
                          }
                        }
                      }
                      frame False {
                      }
                    }
                  }
                }
              }
              frame #6 {
                # "LAB04-1"
                n993 = Less?(x=w1658, y=2) -> (x < y?=w1661:bool)
                n994 = local read "DISP LAB04-1"() -> (w1663:T4)
                n995 = Unbundle(w1663) -> ("STATUS"=w1664:string)  [unwired: 2 out]
                n996 = Equal?(x=w1664, y="RUN") -> (x = y?=w1660:bool)
                n997 = And(x=w1660, y=w1661) -> (x .and. y?=w1659:bool)
                n998 = case shown="True" w1659 {
                  tunnel: w1663 -> [_ w1669]
                  tunnel: w1658 -> [_ w1673]
                  frame False {
                  }
                  frame True {
                    n999 = local read "SET LAB04-1"() -> (w1675:T5)
                    n1000 = local read "TDMS LAB04-1"() -> (w1668:refnum<k34>)
                    n1001 = Unbundle(w1669) -> ("CYCLE"=w1674:dbl)  [unwired: 2 out]
                    n1002 = Unbundle(w1675) -> ("CYCLES"=w1666:dbl, "T-RISE mins"=w1672:dbl)  [unwired: 3 out]
                    n1003 = case shown="\"T-RISE TEST\"" w1673 {
                      tunnel: w1672 -> [_ _ w1682]
                      tunnel: [w1677 w1679 w1682] -> w1671
                      tunnel: w1666 -> [w1677 w1679 _]
                      tunnel: ["CHART PASS" "CYCLE PASS" "T-RISE PASS"] -> w1670
                      frame "CHART TEST", Default {
                      }
                      frame "CYCLE TEST" {
                      }
                      frame "T-RISE TEST" {
                      }
                    }
                    n1004 = Increment(x=w1666) -> (x+1=w1667:dbl)
                    n1005 = Greater Or Equal?(x=w1674, y=w1667) -> (x >= y?=w1676:bool)
                    n1006 = case shown="True" w1676 {
                      tunnel: w1671 -> [w1686 _]
                      tunnel: w1670 -> [w1685 _]
                      tunnel: w1669 -> [w1684 _]
                      tunnel: w1668 -> [w1683 _]
                      frame True {
                        n1007 = stacked-sequence {
                          tunnel: w1686 -> [w1690 _]
                          tunnel: w1685 -> [w1688 w1694]
                          tunnel: w1684 -> [_ w1697]
                          tunnel: w1683 -> [w1687 _]
                          frame #0 {
                            n1008 = Build Array(w1688) -> (w1691:string[])
                            n1009 = Build Array(w1690) -> (w1689:dbl[])
                            n1010 = TDMS Write(0:w1687, 5:"TEST PASS", 7:w1691, 9:w1689) -> (15:w1693:errorcluster)  [unwired: 2 in, 3 out]
                            n1011 = local write "data file error"(w1693) -> ()
                          }
                          frame #1 {
                            n1012 = Bundle(cluster=w1697, "STATUS"=w1694) -> (w1695:T4)  [unwired: 2 in]
                            n1013 = local write "RESULT LAB04-1"(TRUE) -> ()
                            n1014 = local write "DISP LAB04-1"(w1695) -> ()
                          }
                        }
                      }
                      frame False {
                      }
                    }
                  }
                }
              }
              frame #7 {
                # "LAB04-2"
                n1015 = Less?(x=w1698, y=2) -> (x < y?=w1701:bool)
                n1016 = local read "DISP LAB04-2"() -> (w1703:T4)
                n1017 = Unbundle(w1703) -> ("STATUS"=w1704:string)  [unwired: 2 out]
                n1018 = Equal?(x=w1704, y="RUN") -> (x = y?=w1700:bool)
                n1019 = And(x=w1700, y=w1701) -> (x .and. y?=w1699:bool)
                n1020 = case shown="True" w1699 {
                  tunnel: w1703 -> [_ w1709]
                  tunnel: w1698 -> [_ w1713]
                  frame False {
                  }
                  frame True {
                    n1021 = local read "SET LAB04-2"() -> (w1715:T5)
                    n1022 = local read "TDMS LAB04-2"() -> (w1708:refnum<k34>)
                    n1023 = Unbundle(w1709) -> ("CYCLE"=w1714:dbl)  [unwired: 2 out]
                    n1024 = Unbundle(w1715) -> ("CYCLES"=w1706:dbl, "T-RISE mins"=w1712:dbl)  [unwired: 3 out]
                    n1025 = case shown="\"T-RISE TEST\"" w1713 {
                      tunnel: w1712 -> [_ _ w1722]
                      tunnel: [w1717 w1719 w1722] -> w1711
                      tunnel: w1706 -> [w1717 w1719 _]
                      tunnel: ["CHART PASS" "CYCLE PASS" "T-RISE PASS"] -> w1710
                      frame "CHART TEST", Default {
                      }
                      frame "CYCLE TEST" {
                      }
                      frame "T-RISE TEST" {
                      }
                    }
                    n1026 = Increment(x=w1706) -> (x+1=w1707:dbl)
                    n1027 = Greater Or Equal?(x=w1714, y=w1707) -> (x >= y?=w1716:bool)
                    n1028 = case shown="True" w1716 {
                      tunnel: w1711 -> [w1726 _]
                      tunnel: w1710 -> [w1725 _]
                      tunnel: w1709 -> [w1724 _]
                      tunnel: w1708 -> [w1723 _]
                      frame True {
                        n1029 = stacked-sequence {
                          tunnel: w1726 -> [w1730 _]
                          tunnel: w1725 -> [w1728 w1734]
                          tunnel: w1724 -> [_ w1737]
                          tunnel: w1723 -> [w1727 _]
                          frame #0 {
                            n1030 = Build Array(w1728) -> (w1731:string[])
                            n1031 = Build Array(w1730) -> (w1729:dbl[])
                            n1032 = TDMS Write(0:w1727, 5:"TEST PASS", 7:w1731, 9:w1729) -> (15:w1733:errorcluster)  [unwired: 2 in, 3 out]
                            n1033 = local write "data file error"(w1733) -> ()
                          }
                          frame #1 {
                            n1034 = Bundle(cluster=w1737, "STATUS"=w1734) -> (w1735:T4)  [unwired: 2 in]
                            n1035 = local write "RESULT LAB04-2"(TRUE) -> ()
                            n1036 = local write "DISP LAB04-2"(w1735) -> ()
                          }
                        }
                      }
                      frame False {
                      }
                    }
                  }
                }
              }
              frame #8 {
                # "LAB05-1"
                n1037 = Less?(x=w1738, y=2) -> (x < y?=w1741:bool)
                n1038 = local read "DISP LAB05-1"() -> (w1743:T4)
                n1039 = Unbundle(w1743) -> ("STATUS"=w1744:string)  [unwired: 2 out]
                n1040 = Equal?(x=w1744, y="RUN") -> (x = y?=w1740:bool)
                n1041 = And(x=w1740, y=w1741) -> (x .and. y?=w1739:bool)
                n1042 = case shown="True" w1739 {
                  tunnel: w1743 -> [_ w1749]
                  tunnel: w1738 -> [_ w1753]
                  frame False {
                  }
                  frame True {
                    n1043 = local read "SET LAB05-1"() -> (w1755:T5)
                    n1044 = local read "TDMS LAB05-1"() -> (w1748:refnum<k34>)
                    n1045 = Unbundle(w1749) -> ("CYCLE"=w1754:dbl)  [unwired: 2 out]
                    n1046 = Unbundle(w1755) -> ("CYCLES"=w1746:dbl, "T-RISE mins"=w1752:dbl)  [unwired: 3 out]
                    n1047 = case shown="\"T-RISE TEST\"" w1753 {
                      tunnel: w1752 -> [_ _ w1762]
                      tunnel: [w1757 w1759 w1762] -> w1751
                      tunnel: w1746 -> [w1757 w1759 _]
                      tunnel: ["CHART PASS" "CYCLE PASS" "T-RISE PASS"] -> w1750
                      frame "CHART TEST", Default {
                      }
                      frame "CYCLE TEST" {
                      }
                      frame "T-RISE TEST" {
                      }
                    }
                    n1048 = Increment(x=w1746) -> (x+1=w1747:dbl)
                    n1049 = Greater Or Equal?(x=w1754, y=w1747) -> (x >= y?=w1756:bool)
                    n1050 = case shown="True" w1756 {
                      tunnel: w1751 -> [w1766 _]
                      tunnel: w1750 -> [w1765 _]
                      tunnel: w1749 -> [w1764 _]
                      tunnel: w1748 -> [w1763 _]
                      frame True {
                        n1051 = stacked-sequence {
                          tunnel: w1766 -> [w1770 _]
                          tunnel: w1765 -> [w1768 w1774]
                          tunnel: w1764 -> [_ w1777]
                          tunnel: w1763 -> [w1767 _]
                          frame #0 {
                            n1052 = Build Array(w1768) -> (w1771:string[])
                            n1053 = Build Array(w1770) -> (w1769:dbl[])
                            n1054 = TDMS Write(0:w1767, 5:"TEST PASS", 7:w1771, 9:w1769) -> (15:w1773:errorcluster)  [unwired: 2 in, 3 out]
                            n1055 = local write "data file error"(w1773) -> ()
                          }
                          frame #1 {
                            n1056 = Bundle(cluster=w1777, "STATUS"=w1774) -> (w1775:T4)  [unwired: 2 in]
                            n1057 = local write "RESULT LAB05-1"(TRUE) -> ()
                            n1058 = local write "DISP LAB05-1"(w1775) -> ()
                          }
                        }
                      }
                      frame False {
                      }
                    }
                  }
                }
              }
              frame #9 {
                # "LAB05-2"
                n1059 = Less?(x=w1778, y=2) -> (x < y?=w1781:bool)
                n1060 = local read "DISP LAB05-2"() -> (w1783:T4)
                n1061 = Unbundle(w1783) -> ("STATUS"=w1784:string)  [unwired: 2 out]
                n1062 = Equal?(x=w1784, y="RUN") -> (x = y?=w1780:bool)
                n1063 = And(x=w1780, y=w1781) -> (x .and. y?=w1779:bool)
                n1064 = case shown="True" w1779 {
                  tunnel: w1783 -> [_ w1789]
                  tunnel: w1778 -> [_ w1793]
                  frame False {
                  }
                  frame True {
                    n1065 = local read "SET LAB05-2"() -> (w1795:T5)
                    n1066 = local read "TDMS LAB05-2"() -> (w1788:refnum<k34>)
                    n1067 = Unbundle(w1789) -> ("CYCLE"=w1794:dbl)  [unwired: 2 out]
                    n1068 = Unbundle(w1795) -> ("CYCLES"=w1786:dbl, "T-RISE mins"=w1792:dbl)  [unwired: 3 out]
                    n1069 = case shown="\"T-RISE TEST\"" w1793 {
                      tunnel: w1792 -> [_ _ w1802]
                      tunnel: [w1797 w1799 w1802] -> w1791
                      tunnel: w1786 -> [w1797 w1799 _]
                      tunnel: ["CHART PASS" "CYCLE PASS" "T-RISE PASS"] -> w1790
                      frame "CHART TEST", Default {
                      }
                      frame "CYCLE TEST" {
                      }
                      frame "T-RISE TEST" {
                      }
                    }
                    n1070 = Increment(x=w1786) -> (x+1=w1787:dbl)
                    n1071 = Greater Or Equal?(x=w1794, y=w1787) -> (x >= y?=w1796:bool)
                    n1072 = case shown="True" w1796 {
                      tunnel: w1791 -> [w1806 _]
                      tunnel: w1790 -> [w1805 _]
                      tunnel: w1789 -> [w1804 _]
                      tunnel: w1788 -> [w1803 _]
                      frame True {
                        n1073 = stacked-sequence {
                          tunnel: w1806 -> [w1810 _]
                          tunnel: w1805 -> [w1808 w1814]
                          tunnel: w1804 -> [_ w1817]
                          tunnel: w1803 -> [w1807 _]
                          frame #0 {
                            n1074 = Build Array(w1808) -> (w1811:string[])
                            n1075 = Build Array(w1810) -> (w1809:dbl[])
                            n1076 = TDMS Write(0:w1807, 5:"TEST PASS", 7:w1811, 9:w1809) -> (15:w1813:errorcluster)  [unwired: 2 in, 3 out]
                            n1077 = local write "data file error"(w1813) -> ()
                          }
                          frame #1 {
                            n1078 = Bundle(cluster=w1817, "STATUS"=w1814) -> (w1815:T4)  [unwired: 2 in]
                            n1079 = local write "RESULT LAB05-2"(TRUE) -> ()
                            n1080 = local write "DISP LAB05-2"(w1815) -> ()
                          }
                        }
                      }
                      frame False {
                      }
                    }
                  }
                }
              }
            }
          }
          frame #5 {
            # "check if test cycles reached for temperature rise test"
            n1081 = stacked-sequence {
              tunnel: w1847 -> [_ _ _ _ _ _ _ _ _ _]
              tunnel: w1846 -> [_ _ _ _ _ _ _ _ _ _]
              tunnel: w1845 -> [_ _ _ _ _ _ _ _ _ _]
              tunnel: w1844 -> [_ _ _ _ _ _ _ _ _ _]
              tunnel: w1843 -> [_ _ _ _ _ _ _ _ _ _]
              tunnel: w1842 -> [_ _ _ _ _ _ _ _ _ _]
              tunnel: w1841 -> [_ _ _ _ _ _ _ _ _ _]
              tunnel: w1840 -> [_ _ _ _ _ _ _ _ _ _]
              tunnel: w1839 -> [_ _ _ _ _ _ _ _ _ _]
              tunnel: w1838 -> [_ _ _ _ _ _ _ _ _ _]
              tunnel: w1837 -> [w1853 _ _ _ _ _ _ _ _ _]
              tunnel: w1827 -> [w1848 _ _ _ _ _ _ _ _ _]
              tunnel: w1836 -> [_ w1879 _ _ _ _ _ _ _ _]
              tunnel: w1835 -> [_ _ w1909 _ _ _ _ _ _ _]
              tunnel: w1834 -> [_ _ _ w1939 _ _ _ _ _ _]
              tunnel: w1833 -> [_ _ _ _ w1969 _ _ _ _ _]
              tunnel: w1832 -> [_ _ _ _ _ w1999 _ _ _ _]
              tunnel: w1831 -> [_ _ _ _ _ _ w2029 _ _ _]
              tunnel: w1830 -> [_ _ _ _ _ _ _ w2059 _ _]
              tunnel: w1829 -> [_ _ _ _ _ _ _ _ w2089 _]
              tunnel: w1828 -> [_ _ _ _ _ _ _ _ _ w2119]
              tunnel: w1826 -> [_ w1878 _ _ _ _ _ _ _ _]
              tunnel: w1825 -> [_ _ w1908 _ _ _ _ _ _ _]
              tunnel: w1824 -> [_ _ _ w1938 _ _ _ _ _ _]
              tunnel: w1823 -> [_ _ _ _ w1968 _ _ _ _ _]
              tunnel: w1822 -> [_ _ _ _ _ w1998 _ _ _ _]
              tunnel: w1821 -> [_ _ _ _ _ _ w2028 _ _ _]
              tunnel: w1820 -> [_ _ _ _ _ _ _ w2058 _ _]
              tunnel: w1819 -> [_ _ _ _ _ _ _ _ w2088 _]
              tunnel: w1818 -> [_ _ _ _ _ _ _ _ _ w2118]
              frame #0 {
                # "LAB01-1"
                n1082 = Equal?(x=w1853, y=2) -> (x = y?=w1851:bool)
                n1083 = local read "DISP LAB01-1"() -> (w1854:T4)
                n1084 = Unbundle(w1854) -> ("STATUS"=w1855:string)  [unwired: 2 out]
                n1085 = Equal?(x=w1855, y="RUN") -> (x = y?=w1850:bool)
                n1086 = And(x=w1850, y=w1851) -> (x .and. y?=w1849:bool)
                n1087 = case shown="True" w1849 {
                  tunnel: w1854 -> [_ w1858]
                  tunnel: w1848 -> [_ w1861]
                  frame False {
                  }
                  frame True {
                    n1088 = local read "SET LAB01-1"() -> (w1860:T5)
                    n1089 = local read "TDMS LAB01-1"() -> (w1857:refnum<k34>)
                    n1090 = Unbundle(w1858) -> ("CYCLE"=w1862:dbl)  [unwired: 2 out]
                    n1091 = Unbundle(w1860) -> ("T-RISE mins"=w1859:dbl)  [unwired: 4 out]
                    n1092 = Greater Or Equal?(x=w1862, y=w1861) -> (x >= y?=w1863:bool)
                    n1093 = case shown="True" w1863 {
                      tunnel: w1859 -> [w1866 _]
                      tunnel: w1858 -> [w1865 _]
                      tunnel: w1857 -> [w1864 _]
                      frame True {
                        n1094 = stacked-sequence {
                          tunnel: w1866 -> [w1869 _]
                          tunnel: w1865 -> [_ w1874]
                          tunnel: w1864 -> [w1867 _]
                          frame #0 {
                            n1095 = Build Array("T-RISE") -> (w1871:string[])
                            n1096 = Build Array(w1869) -> (w1870:dbl[])
                            n1097 = TDMS Write(0:w1867, 5:"TEST PASS", 7:w1871, 9:w1870) -> (15:w1873:errorcluster)  [unwired: 2 in, 3 out]
                            n1098 = local write "data file error"(w1873) -> ()
                          }
                          frame #1 {
                            n1099 = Bundle(cluster=w1874, "STATUS"="T-RISE PASS") -> (w1876:T4)  [unwired: 2 in]
                            n1100 = local write "RESULT LAB01-1"(TRUE) -> ()
                            n1101 = local write "DISP LAB01-1"(w1876) -> ()
                          }
                        }
                      }
                      frame False {
                      }
                    }
                  }
                }
              }
              frame #1 {
                # "LAB01-2"
                n1102 = Equal?(x=w1879, y=2) -> (x = y?=w1882:bool)
                n1103 = local read "DISP LAB01-2"() -> (w1884:T4)
                n1104 = Unbundle(w1884) -> ("STATUS"=w1885:string)  [unwired: 2 out]
                n1105 = Equal?(x=w1885, y="RUN") -> (x = y?=w1881:bool)
                n1106 = And(x=w1881, y=w1882) -> (x .and. y?=w1880:bool)
                n1107 = case shown="True" w1880 {
                  tunnel: w1884 -> [_ w1888]
                  tunnel: w1878 -> [_ w1891]
                  frame False {
                  }
                  frame True {
                    n1108 = local read "SET LAB01-2"() -> (w1890:T5)
                    n1109 = local read "TDMS LAB01-2"() -> (w1887:refnum<k34>)
                    n1110 = Unbundle(w1888) -> ("CYCLE"=w1892:dbl)  [unwired: 2 out]
                    n1111 = Unbundle(w1890) -> ("T-RISE mins"=w1889:dbl)  [unwired: 4 out]
                    n1112 = Greater Or Equal?(x=w1892, y=w1891) -> (x >= y?=w1893:bool)
                    n1113 = case shown="True" w1893 {
                      tunnel: w1889 -> [w1896 _]
                      tunnel: w1888 -> [w1895 _]
                      tunnel: w1887 -> [w1894 _]
                      frame True {
                        n1114 = stacked-sequence {
                          tunnel: w1896 -> [w1899 _]
                          tunnel: w1895 -> [_ w1904]
                          tunnel: w1894 -> [w1897 _]
                          frame #0 {
                            n1115 = Build Array("T-RISE") -> (w1901:string[])
                            n1116 = Build Array(w1899) -> (w1900:dbl[])
                            n1117 = TDMS Write(0:w1897, 5:"TEST PASS", 7:w1901, 9:w1900) -> (15:w1903:errorcluster)  [unwired: 2 in, 3 out]
                            n1118 = local write "data file error"(w1903) -> ()
                          }
                          frame #1 {
                            n1119 = Bundle(cluster=w1904, "STATUS"="T-RISE PASS") -> (w1906:T4)  [unwired: 2 in]
                            n1120 = local write "RESULT LAB01-2"(TRUE) -> ()
                            n1121 = local write "DISP LAB01-2"(w1906) -> ()
                          }
                        }
                      }
                      frame False {
                      }
                    }
                  }
                }
              }
              frame #2 {
                # "LAB02-1"
                n1122 = Equal?(x=w1909, y=2) -> (x = y?=w1912:bool)
                n1123 = local read "DISP LAB02-1"() -> (w1914:T4)
                n1124 = Unbundle(w1914) -> ("STATUS"=w1915:string)  [unwired: 2 out]
                n1125 = Equal?(x=w1915, y="RUN") -> (x = y?=w1911:bool)
                n1126 = And(x=w1911, y=w1912) -> (x .and. y?=w1910:bool)
                n1127 = case shown="True" w1910 {
                  tunnel: w1914 -> [_ w1918]
                  tunnel: w1908 -> [_ w1921]
                  frame False {
                  }
                  frame True {
                    n1128 = local read "SET LAB02-1"() -> (w1920:T5)
                    n1129 = local read "TDMS LAB02-1"() -> (w1917:refnum<k34>)
                    n1130 = Unbundle(w1918) -> ("CYCLE"=w1922:dbl)  [unwired: 2 out]
                    n1131 = Unbundle(w1920) -> ("T-RISE mins"=w1919:dbl)  [unwired: 4 out]
                    n1132 = Greater Or Equal?(x=w1922, y=w1921) -> (x >= y?=w1923:bool)
                    n1133 = case shown="True" w1923 {
                      tunnel: w1919 -> [w1926 _]
                      tunnel: w1918 -> [w1925 _]
                      tunnel: w1917 -> [w1924 _]
                      frame True {
                        n1134 = stacked-sequence {
                          tunnel: w1926 -> [w1929 _]
                          tunnel: w1925 -> [_ w1934]
                          tunnel: w1924 -> [w1927 _]
                          frame #0 {
                            n1135 = Build Array("T-RISE") -> (w1931:string[])
                            n1136 = Build Array(w1929) -> (w1930:dbl[])
                            n1137 = TDMS Write(0:w1927, 5:"TEST PASS", 7:w1931, 9:w1930) -> (15:w1933:errorcluster)  [unwired: 2 in, 3 out]
                            n1138 = local write "data file error"(w1933) -> ()
                          }
                          frame #1 {
                            n1139 = Bundle(cluster=w1934, "STATUS"="T-RISE PASS") -> (w1936:T4)  [unwired: 2 in]
                            n1140 = local write "RESULT LAB02-1"(TRUE) -> ()
                            n1141 = local write "DISP LAB02-1"(w1936) -> ()
                          }
                        }
                      }
                      frame False {
                      }
                    }
                  }
                }
              }
              frame #3 {
                # "LAB02-2"
                n1142 = Equal?(x=w1939, y=2) -> (x = y?=w1942:bool)
                n1143 = local read "DISP LAB02-2"() -> (w1944:T4)
                n1144 = Unbundle(w1944) -> ("STATUS"=w1945:string)  [unwired: 2 out]
                n1145 = Equal?(x=w1945, y="RUN") -> (x = y?=w1941:bool)
                n1146 = And(x=w1941, y=w1942) -> (x .and. y?=w1940:bool)
                n1147 = case shown="True" w1940 {
                  tunnel: w1944 -> [_ w1948]
                  tunnel: w1938 -> [_ w1951]
                  frame False {
                  }
                  frame True {
                    n1148 = local read "SET LAB02-2"() -> (w1950:T5)
                    n1149 = local read "TDMS LAB02-2"() -> (w1947:refnum<k34>)
                    n1150 = Unbundle(w1948) -> ("CYCLE"=w1952:dbl)  [unwired: 2 out]
                    n1151 = Unbundle(w1950) -> ("T-RISE mins"=w1949:dbl)  [unwired: 4 out]
                    n1152 = Greater Or Equal?(x=w1952, y=w1951) -> (x >= y?=w1953:bool)
                    n1153 = case shown="True" w1953 {
                      tunnel: w1949 -> [w1956 _]
                      tunnel: w1948 -> [w1955 _]
                      tunnel: w1947 -> [w1954 _]
                      frame True {
                        n1154 = stacked-sequence {
                          tunnel: w1956 -> [w1959 _]
                          tunnel: w1955 -> [_ w1964]
                          tunnel: w1954 -> [w1957 _]
                          frame #0 {
                            n1155 = Build Array("T-RISE") -> (w1961:string[])
                            n1156 = Build Array(w1959) -> (w1960:dbl[])
                            n1157 = TDMS Write(0:w1957, 5:"TEST PASS", 7:w1961, 9:w1960) -> (15:w1963:errorcluster)  [unwired: 2 in, 3 out]
                            n1158 = local write "data file error"(w1963) -> ()
                          }
                          frame #1 {
                            n1159 = Bundle(cluster=w1964, "STATUS"="T-RISE PASS") -> (w1966:T4)  [unwired: 2 in]
                            n1160 = local write "RESULT LAB02-2"(TRUE) -> ()
                            n1161 = local write "DISP LAB02-2"(w1966) -> ()
                          }
                        }
                      }
                      frame False {
                      }
                    }
                  }
                }
              }
              frame #4 {
                # "LAB03-1"
                n1162 = Equal?(x=w1969, y=2) -> (x = y?=w1972:bool)
                n1163 = local read "DISP LAB03-1"() -> (w1974:T4)
                n1164 = Unbundle(w1974) -> ("STATUS"=w1975:string)  [unwired: 2 out]
                n1165 = Equal?(x=w1975, y="RUN") -> (x = y?=w1971:bool)
                n1166 = And(x=w1971, y=w1972) -> (x .and. y?=w1970:bool)
                n1167 = case shown="True" w1970 {
                  tunnel: w1974 -> [_ w1978]
                  tunnel: w1968 -> [_ w1981]
                  frame False {
                  }
                  frame True {
                    n1168 = local read "SET LAB03-1"() -> (w1980:T5)
                    n1169 = local read "TDMS LAB03-1"() -> (w1977:refnum<k34>)
                    n1170 = Unbundle(w1978) -> ("CYCLE"=w1982:dbl)  [unwired: 2 out]
                    n1171 = Unbundle(w1980) -> ("T-RISE mins"=w1979:dbl)  [unwired: 4 out]
                    n1172 = Greater Or Equal?(x=w1982, y=w1981) -> (x >= y?=w1983:bool)
                    n1173 = case shown="True" w1983 {
                      tunnel: w1979 -> [w1986 _]
                      tunnel: w1978 -> [w1985 _]
                      tunnel: w1977 -> [w1984 _]
                      frame True {
                        n1174 = stacked-sequence {
                          tunnel: w1986 -> [w1989 _]
                          tunnel: w1985 -> [_ w1994]
                          tunnel: w1984 -> [w1987 _]
                          frame #0 {
                            n1175 = Build Array("T-RISE") -> (w1991:string[])
                            n1176 = Build Array(w1989) -> (w1990:dbl[])
                            n1177 = TDMS Write(0:w1987, 5:"TEST PASS", 7:w1991, 9:w1990) -> (15:w1993:errorcluster)  [unwired: 2 in, 3 out]
                            n1178 = local write "data file error"(w1993) -> ()
                          }
                          frame #1 {
                            n1179 = Bundle(cluster=w1994, "STATUS"="T-RISE PASS") -> (w1996:T4)  [unwired: 2 in]
                            n1180 = local write "RESULT LAB03-1"(TRUE) -> ()
                            n1181 = local write "DISP LAB03-1"(w1996) -> ()
                          }
                        }
                      }
                      frame False {
                      }
                    }
                  }
                }
              }
              frame #5 {
                # "LAB03-2"
                n1182 = Equal?(x=w1999, y=2) -> (x = y?=w2002:bool)
                n1183 = local read "DISP LAB03-2"() -> (w2004:T4)
                n1184 = Unbundle(w2004) -> ("STATUS"=w2005:string)  [unwired: 2 out]
                n1185 = Equal?(x=w2005, y="RUN") -> (x = y?=w2001:bool)
                n1186 = And(x=w2001, y=w2002) -> (x .and. y?=w2000:bool)
                n1187 = case shown="True" w2000 {
                  tunnel: w2004 -> [_ w2008]
                  tunnel: w1998 -> [_ w2011]
                  frame False {
                  }
                  frame True {
                    n1188 = local read "SET LAB03-2"() -> (w2010:T5)
                    n1189 = local read "TDMS LAB03-2"() -> (w2007:refnum<k34>)
                    n1190 = Unbundle(w2008) -> ("CYCLE"=w2012:dbl)  [unwired: 2 out]
                    n1191 = Unbundle(w2010) -> ("T-RISE mins"=w2009:dbl)  [unwired: 4 out]
                    n1192 = Greater Or Equal?(x=w2012, y=w2011) -> (x >= y?=w2013:bool)
                    n1193 = case shown="True" w2013 {
                      tunnel: w2009 -> [w2016 _]
                      tunnel: w2008 -> [w2015 _]
                      tunnel: w2007 -> [w2014 _]
                      frame True {
                        n1194 = stacked-sequence {
                          tunnel: w2016 -> [w2019 _]
                          tunnel: w2015 -> [_ w2024]
                          tunnel: w2014 -> [w2017 _]
                          frame #0 {
                            n1195 = Build Array("T-RISE") -> (w2021:string[])
                            n1196 = Build Array(w2019) -> (w2020:dbl[])
                            n1197 = TDMS Write(0:w2017, 5:"TEST PASS", 7:w2021, 9:w2020) -> (15:w2023:errorcluster)  [unwired: 2 in, 3 out]
                            n1198 = local write "data file error"(w2023) -> ()
                          }
                          frame #1 {
                            n1199 = Bundle(cluster=w2024, "STATUS"="T-RISE PASS") -> (w2026:T4)  [unwired: 2 in]
                            n1200 = local write "RESULT LAB03-2"(TRUE) -> ()
                            n1201 = local write "DISP LAB03-2"(w2026) -> ()
                          }
                        }
                      }
                      frame False {
                      }
                    }
                  }
                }
              }
              frame #6 {
                # "LAB04-1"
                n1202 = Equal?(x=w2029, y=2) -> (x = y?=w2032:bool)
                n1203 = local read "DISP LAB04-1"() -> (w2034:T4)
                n1204 = Unbundle(w2034) -> ("STATUS"=w2035:string)  [unwired: 2 out]
                n1205 = Equal?(x=w2035, y="RUN") -> (x = y?=w2031:bool)
                n1206 = And(x=w2031, y=w2032) -> (x .and. y?=w2030:bool)
                n1207 = case shown="True" w2030 {
                  tunnel: w2034 -> [_ w2038]
                  tunnel: w2028 -> [_ w2041]
                  frame False {
                  }
                  frame True {
                    n1208 = local read "SET LAB04-1"() -> (w2040:T5)
                    n1209 = local read "TDMS LAB04-1"() -> (w2037:refnum<k34>)
                    n1210 = Unbundle(w2038) -> ("CYCLE"=w2042:dbl)  [unwired: 2 out]
                    n1211 = Unbundle(w2040) -> ("T-RISE mins"=w2039:dbl)  [unwired: 4 out]
                    n1212 = Greater Or Equal?(x=w2042, y=w2041) -> (x >= y?=w2043:bool)
                    n1213 = case shown="True" w2043 {
                      tunnel: w2039 -> [w2046 _]
                      tunnel: w2038 -> [w2045 _]
                      tunnel: w2037 -> [w2044 _]
                      frame True {
                        n1214 = stacked-sequence {
                          tunnel: w2046 -> [w2049 _]
                          tunnel: w2045 -> [_ w2054]
                          tunnel: w2044 -> [w2047 _]
                          frame #0 {
                            n1215 = Build Array("T-RISE") -> (w2051:string[])
                            n1216 = Build Array(w2049) -> (w2050:dbl[])
                            n1217 = TDMS Write(0:w2047, 5:"TEST PASS", 7:w2051, 9:w2050) -> (15:w2053:errorcluster)  [unwired: 2 in, 3 out]
                            n1218 = local write "data file error"(w2053) -> ()
                          }
                          frame #1 {
                            n1219 = Bundle(cluster=w2054, "STATUS"="T-RISE PASS") -> (w2056:T4)  [unwired: 2 in]
                            n1220 = local write "RESULT LAB04-1"(TRUE) -> ()
                            n1221 = local write "DISP LAB04-1"(w2056) -> ()
                          }
                        }
                      }
                      frame False {
                      }
                    }
                  }
                }
              }
              frame #7 {
                # "LAB04-2"
                n1222 = Equal?(x=w2059, y=2) -> (x = y?=w2062:bool)
                n1223 = local read "DISP LAB04-2"() -> (w2064:T4)
                n1224 = Unbundle(w2064) -> ("STATUS"=w2065:string)  [unwired: 2 out]
                n1225 = Equal?(x=w2065, y="RUN") -> (x = y?=w2061:bool)
                n1226 = And(x=w2061, y=w2062) -> (x .and. y?=w2060:bool)
                n1227 = case shown="True" w2060 {
                  tunnel: w2064 -> [_ w2068]
                  tunnel: w2058 -> [_ w2071]
                  frame False {
                  }
                  frame True {
                    n1228 = local read "SET LAB04-2"() -> (w2070:T5)
                    n1229 = local read "TDMS LAB04-2"() -> (w2067:refnum<k34>)
                    n1230 = Unbundle(w2068) -> ("CYCLE"=w2072:dbl)  [unwired: 2 out]
                    n1231 = Unbundle(w2070) -> ("T-RISE mins"=w2069:dbl)  [unwired: 4 out]
                    n1232 = Greater Or Equal?(x=w2072, y=w2071) -> (x >= y?=w2073:bool)
                    n1233 = case shown="True" w2073 {
                      tunnel: w2069 -> [w2076 _]
                      tunnel: w2068 -> [w2075 _]
                      tunnel: w2067 -> [w2074 _]
                      frame True {
                        n1234 = stacked-sequence {
                          tunnel: w2076 -> [w2079 _]
                          tunnel: w2075 -> [_ w2084]
                          tunnel: w2074 -> [w2077 _]
                          frame #0 {
                            n1235 = Build Array("T-RISE") -> (w2081:string[])
                            n1236 = Build Array(w2079) -> (w2080:dbl[])
                            n1237 = TDMS Write(0:w2077, 5:"TEST PASS", 7:w2081, 9:w2080) -> (15:w2083:errorcluster)  [unwired: 2 in, 3 out]
                            n1238 = local write "data file error"(w2083) -> ()
                          }
                          frame #1 {
                            n1239 = Bundle(cluster=w2084, "STATUS"="T-RISE PASS") -> (w2086:T4)  [unwired: 2 in]
                            n1240 = local write "RESULT LAB04-2"(TRUE) -> ()
                            n1241 = local write "DISP LAB04-2"(w2086) -> ()
                          }
                        }
                      }
                      frame False {
                      }
                    }
                  }
                }
              }
              frame #8 {
                # "LAB05-1"
                n1242 = Equal?(x=w2089, y=2) -> (x = y?=w2092:bool)
                n1243 = local read "DISP LAB05-1"() -> (w2094:T4)
                n1244 = Unbundle(w2094) -> ("STATUS"=w2095:string)  [unwired: 2 out]
                n1245 = Equal?(x=w2095, y="RUN") -> (x = y?=w2091:bool)
                n1246 = And(x=w2091, y=w2092) -> (x .and. y?=w2090:bool)
                n1247 = case shown="True" w2090 {
                  tunnel: w2094 -> [_ w2098]
                  tunnel: w2088 -> [_ w2101]
                  frame False {
                  }
                  frame True {
                    n1248 = local read "SET LAB05-1"() -> (w2100:T5)
                    n1249 = local read "TDMS LAB05-1"() -> (w2097:refnum<k34>)
                    n1250 = Unbundle(w2098) -> ("CYCLE"=w2102:dbl)  [unwired: 2 out]
                    n1251 = Unbundle(w2100) -> ("T-RISE mins"=w2099:dbl)  [unwired: 4 out]
                    n1252 = Greater Or Equal?(x=w2102, y=w2101) -> (x >= y?=w2103:bool)
                    n1253 = case shown="True" w2103 {
                      tunnel: w2099 -> [w2106 _]
                      tunnel: w2098 -> [w2105 _]
                      tunnel: w2097 -> [w2104 _]
                      frame True {
                        n1254 = stacked-sequence {
                          tunnel: w2106 -> [w2109 _]
                          tunnel: w2105 -> [_ w2114]
                          tunnel: w2104 -> [w2107 _]
                          frame #0 {
                            n1255 = Build Array("T-RISE") -> (w2111:string[])
                            n1256 = Build Array(w2109) -> (w2110:dbl[])
                            n1257 = TDMS Write(0:w2107, 5:"TEST PASS", 7:w2111, 9:w2110) -> (15:w2113:errorcluster)  [unwired: 2 in, 3 out]
                            n1258 = local write "data file error"(w2113) -> ()
                          }
                          frame #1 {
                            n1259 = Bundle(cluster=w2114, "STATUS"="T-RISE PASS") -> (w2116:T4)  [unwired: 2 in]
                            n1260 = local write "RESULT LAB05-1"(TRUE) -> ()
                            n1261 = local write "DISP LAB05-1"(w2116) -> ()
                          }
                        }
                      }
                      frame False {
                      }
                    }
                  }
                }
              }
              frame #9 {
                # "LAB05-2"
                n1262 = Equal?(x=w2119, y=2) -> (x = y?=w2122:bool)
                n1263 = local read "DISP LAB05-2"() -> (w2124:T4)
                n1264 = Unbundle(w2124) -> ("STATUS"=w2125:string)  [unwired: 2 out]
                n1265 = Equal?(x=w2125, y="RUN") -> (x = y?=w2121:bool)
                n1266 = And(x=w2121, y=w2122) -> (x .and. y?=w2120:bool)
                n1267 = case shown="True" w2120 {
                  tunnel: w2124 -> [_ w2128]
                  tunnel: w2118 -> [_ w2131]
                  frame False {
                  }
                  frame True {
                    n1268 = local read "SET LAB05-2"() -> (w2130:T5)
                    n1269 = local read "TDMS LAB05-2"() -> (w2127:refnum<k34>)
                    n1270 = Unbundle(w2128) -> ("CYCLE"=w2132:dbl)  [unwired: 2 out]
                    n1271 = Unbundle(w2130) -> ("T-RISE mins"=w2129:dbl)  [unwired: 4 out]
                    n1272 = Greater Or Equal?(x=w2132, y=w2131) -> (x >= y?=w2133:bool)
                    n1273 = case shown="True" w2133 {
                      tunnel: w2129 -> [w2136 _]
                      tunnel: w2128 -> [w2135 _]
                      tunnel: w2127 -> [w2134 _]
                      frame True {
                        n1274 = stacked-sequence {
                          tunnel: w2136 -> [w2139 _]
                          tunnel: w2135 -> [_ w2144]
                          tunnel: w2134 -> [w2137 _]
                          frame #0 {
                            n1275 = Build Array("T-RISE") -> (w2141:string[])
                            n1276 = Build Array(w2139) -> (w2140:dbl[])
                            n1277 = TDMS Write(0:w2137, 5:"TEST PASS", 7:w2141, 9:w2140) -> (15:w2143:errorcluster)  [unwired: 2 in, 3 out]
                            n1278 = local write "data file error"(w2143) -> ()
                          }
                          frame #1 {
                            n1279 = Bundle(cluster=w2144, "STATUS"="T-RISE PASS") -> (w2146:T4)  [unwired: 2 in]
                            n1280 = local write "RESULT LAB05-2"(TRUE) -> ()
                            n1281 = local write "DISP LAB05-2"(w2146) -> ()
                          }
                        }
                      }
                      frame False {
                      }
                    }
                  }
                }
              }
            }
          }
          frame #6 {
            # "end test & close test files"
            n1282 = stacked-sequence {
              tunnel: w2157 -> [_ _ _ _ _ _ _ _ _ _]
              tunnel: w2158 -> [_ _ _ _ _ _ _ _ _ _]
              tunnel: w2156 -> [_ _ _ _ _ _ _ _ _ _]
              tunnel: w2155 -> [_ _ _ _ _ _ _ _ _ _]
              tunnel: w2154 -> [_ _ _ _ _ _ _ _ _ _]
              tunnel: w2153 -> [_ _ _ _ _ _ _ _ _ _]
              tunnel: w2152 -> [_ _ _ _ _ _ _ _ _ _]
              tunnel: w2151 -> [_ _ _ _ _ _ _ _ _ _]
              tunnel: w2150 -> [_ _ _ _ _ _ _ _ _ _]
              tunnel: w2149 -> [_ _ _ _ _ _ _ _ _ _]
              frame #0 {
                # "LAB01-1"
                n1283 = local read "DISP LAB01-1"() -> (w2162:T4)
                n1284 = local read "run lab01-1"() -> (w2159:bool)
                n1285 = local read "TDMS LAB01-1"() -> (w2160:refnum<k34>)
                n1286 = Unbundle(w2162) -> ("CYCLE"=w2163:dbl, "STATUS"=w2161:string)  [unwired: 1 out]
                n1287 = case shown="True" w2159 {
                  tunnel: w2163 -> [_ w2167]
                  tunnel: w2162 -> [_ w2166]
                  tunnel: w2161 -> [_ w2165]
                  tunnel: w2160 -> [_ w2164]
                  frame False {
                  }
                  frame True {
                    n1288 = Not Equal?(x=w2165, y="RUN") -> (x != y?=w2168:bool)
                    n1289 = Greater?(x=w2167, y=2.0) -> (0:w2170:bool)
                    n1290 = And(x=w2170, y=w2168) -> (x .and. y?=w2169:bool)
                    n1291 = case shown="True" w2169 {
                      tunnel: w2166 -> [_ w2174]
                      tunnel: w2164 -> [_ w2173]
                      frame False {
                      }
                      frame True {
                        n1292 = stacked-sequence {
                          tunnel: w2174 -> [w2178 _ _]
                          tunnel: w2173 -> [_ w2180 _]
                          frame #0 {
                            w2175 = FALSE
                            n1293 = local write "mail control"("END") -> ()
                            n1294 = Bundle(cluster=w2178) -> (w2177:T4)  [unwired: 3 in]
                            n1295 = local write "DISP LAB01-1"(w2177) -> ()
                            n1296 = local write "O/I  LAB01-1"(w2175) -> ()
                            n1297 = local write "run lab01-1"(w2175) -> ()
                            n1298 = local write "RUN LAB01-1"(w2175) -> ()
                          }
                          frame #1 {
                            n1299 = TDMS Close(11:w2180) -> (0:w2179:errorcluster)  [unwired: 1 in, 1 out]
                            n1300 = local write "data file error"(w2179) -> ()
                          }
                          frame #2 {
                            n1301 = stacked-sequence {
                              tunnel: "LAB01-1" -> [w2183 w2185]
                              frame #0 {
                                n1302 = call "sub vi - defrag tdms v1.vi"("panel id"=w2183) -> ("error out"=w2182:errorcluster)  [unwired: 10 in]
                                n1303 = local write "data file error"(w2182) -> ()
                              }
                              frame #1 {
                                n1304 = call "Save data file to network drive v1.vi"("panel id"=w2185) -> ("network file save error"=w2184:errorcluster)  [unwired: 9 in, 1 out]
                                n1305 = local write "data file error"(w2184) -> ()
                              }
                            }
                          }
                        }
                      }
                    }
                  }
                }
              }
              frame #1 {
                # "LAB01-2"
                n1306 = local read "run lab01-2"() -> (w2186:bool)
                n1307 = case shown="True" w2186 {
                  frame False {
                  }
                  frame True {
                    n1308 = local read "DISP LAB01-2"() -> (w2193:T4)
                    n1309 = local read "TDMS LAB01-2"() -> (w2192:refnum<k34>)
                    n1310 = Unbundle(w2193) -> ("CYCLE"=w2189:dbl, "STATUS"=w2194:string)  [unwired: 1 out]
                    n1311 = Not Equal?(x=w2194, y="RUN") -> (x != y?=w2188:bool)
                    n1312 = Greater?(x=w2189, y=2.0) -> (0:w2190:bool)
                    n1313 = And(x=w2190, y=w2188) -> (x .and. y?=w2187:bool)
                    n1314 = case shown="True" w2187 {
                      tunnel: w2193 -> [_ w2197]
                      tunnel: w2192 -> [_ w2196]
                      frame False {
                      }
                      frame True {
                        n1315 = stacked-sequence {
                          tunnel: w2197 -> [w2200 _ _]
                          tunnel: w2196 -> [_ w2202 _]
                          frame #0 {
                            w2198 = FALSE
                            n1316 = local write "mail control"("END") -> ()
                            n1317 = Bundle(cluster=w2200) -> (w2201:T4)  [unwired: 3 in]
                            n1318 = local write "RUN LAB01-2"(w2198) -> ()
                            n1319 = local write "run lab01-2"(w2198) -> ()
                            n1320 = local write "O/I  LAB01-2"(w2198) -> ()
                            n1321 = local write "DISP LAB01-2"(w2201) -> ()
                          }
                          frame #1 {
                            n1322 = TDMS Close(11:w2202) -> (0:w2203:errorcluster)  [unwired: 1 in, 1 out]
                            n1323 = local write "data file error"(w2203) -> ()
                          }
                          frame #2 {
                            n1324 = stacked-sequence {
                              tunnel: "LAB01-2" -> [w2206 w2208]
                              frame #0 {
                                n1325 = call "sub vi - defrag tdms v1.vi"("panel id"=w2206) -> ("error out"=w2205:errorcluster)  [unwired: 10 in]
                                n1326 = local write "data file error"(w2205) -> ()
                              }
                              frame #1 {
                                n1327 = call "Save data file to network drive v1.vi"("panel id"=w2208) -> ("network file save error"=w2207:errorcluster)  [unwired: 9 in, 1 out]
                                n1328 = local write "data file error"(w2207) -> ()
                              }
                            }
                          }
                        }
                      }
                    }
                  }
                }
              }
              frame #2 {
                # "LAB02-1"
                n1329 = local read "run lab02-1"() -> (w2209:bool)
                n1330 = case shown="True" w2209 {
                  frame False {
                  }
                  frame True {
                    n1331 = local read "DISP LAB02-1"() -> (w2216:T4)
                    n1332 = Unbundle(w2216) -> ("CYCLE"=w2212:dbl, "STATUS"=w2217:string)  [unwired: 1 out]
                    n1333 = local read "TDMS LAB02-1"() -> (w2215:refnum<k34>)
                    n1334 = Not Equal?(x=w2217, y="RUN") -> (x != y?=w2211:bool)
                    n1335 = Greater?(x=w2212, y=2.0) -> (0:w2213:bool)
                    n1336 = And(x=w2213, y=w2211) -> (x .and. y?=w2210:bool)
                    n1337 = case shown="True" w2210 {
                      tunnel: w2216 -> [_ w2220]
                      tunnel: w2215 -> [_ w2219]
                      frame False {
                      }
                      frame True {
                        n1338 = stacked-sequence {
                          tunnel: w2220 -> [w2223 _ _]
                          tunnel: w2219 -> [_ w2225 _]
                          frame #0 {
                            w2221 = FALSE
                            n1339 = local write "mail control"("END") -> ()
                            n1340 = Bundle(cluster=w2223) -> (w2224:T4)  [unwired: 3 in]
                            n1341 = local write "O/I  LAB02-1"(w2221) -> ()
                            n1342 = local write "RUN LAB02-1"(w2221) -> ()
                            n1343 = local write "run lab02-1"(w2221) -> ()
                            n1344 = local write "DISP LAB02-1"(w2224) -> ()
                          }
                          frame #1 {
                            n1345 = TDMS Close(11:w2225) -> (0:w2226:errorcluster)  [unwired: 1 in, 1 out]
                            n1346 = local write "data file error"(w2226) -> ()
                          }
                          frame #2 {
                            n1347 = stacked-sequence {
                              tunnel: "LAB02-1" -> [w2229 w2231]
                              frame #0 {
                                n1348 = call "sub vi - defrag tdms v1.vi"("panel id"=w2229) -> ("error out"=w2228:errorcluster)  [unwired: 10 in]
                                n1349 = local write "data file error"(w2228) -> ()
                              }
                              frame #1 {
                                n1350 = call "Save data file to network drive v1.vi"("panel id"=w2231) -> ("network file save error"=w2230:errorcluster)  [unwired: 9 in, 1 out]
                                n1351 = local write "data file error"(w2230) -> ()
                              }
                            }
                          }
                        }
                      }
                    }
                  }
                }
              }
              frame #3 {
                # "LAB02-2"
                n1352 = local read "run lab02-2"() -> (w2232:bool)
                n1353 = case shown="True" w2232 {
                  frame False {
                  }
                  frame True {
                    n1354 = local read "DISP LAB02-2"() -> (w2239:T4)
                    n1355 = local read "TDMS LAB02-2"() -> (w2238:refnum<k34>)
                    n1356 = Unbundle(w2239) -> ("CYCLE"=w2235:dbl, "STATUS"=w2240:string)  [unwired: 1 out]
                    n1357 = Not Equal?(x=w2240, y="RUN") -> (x != y?=w2234:bool)
                    n1358 = Greater?(x=w2235, y=2.0) -> (0:w2236:bool)
                    n1359 = And(x=w2236, y=w2234) -> (x .and. y?=w2233:bool)
                    n1360 = case shown="True" w2233 {
                      tunnel: w2239 -> [_ w2243]
                      tunnel: w2238 -> [_ w2242]
                      frame False {
                      }
                      frame True {
                        n1361 = stacked-sequence {
                          tunnel: w2243 -> [w2246 _ _]
                          tunnel: w2242 -> [_ w2248 _]
                          frame #0 {
                            w2244 = FALSE
                            n1362 = local write "mail control"("END") -> ()
                            n1363 = Bundle(cluster=w2246) -> (w2247:T4)  [unwired: 3 in]
                            n1364 = local write "O/I  LAB02-2"(w2244) -> ()
                            n1365 = local write "run lab02-2"(w2244) -> ()
                            n1366 = local write "RUN LAB02-2"(w2244) -> ()
                            n1367 = local write "DISP LAB02-2"(w2247) -> ()
                          }
                          frame #1 {
                            n1368 = TDMS Close(11:w2248) -> (0:w2249:errorcluster)  [unwired: 1 in, 1 out]
                            n1369 = local write "data file error"(w2249) -> ()
                          }
                          frame #2 {
                            n1370 = stacked-sequence {
                              tunnel: "LAB02-2" -> [w2252 w2254]
                              frame #0 {
                                n1371 = call "sub vi - defrag tdms v1.vi"("panel id"=w2252) -> ("error out"=w2251:errorcluster)  [unwired: 10 in]
                                n1372 = local write "data file error"(w2251) -> ()
                              }
                              frame #1 {
                                n1373 = call "Save data file to network drive v1.vi"("panel id"=w2254) -> ("network file save error"=w2253:errorcluster)  [unwired: 9 in, 1 out]
                                n1374 = local write "data file error"(w2253) -> ()
                              }
                            }
                          }
                        }
                      }
                    }
                  }
                }
              }
              frame #4 {
                # "LAB03-1"
                n1375 = local read "run lab03-1"() -> (w2255:bool)
                n1376 = case shown="True" w2255 {
                  frame False {
                  }
                  frame True {
                    n1377 = local read "DISP LAB03-1"() -> (w2262:T4)
                    n1378 = local read "TDMS LAB03-1"() -> (w2261:refnum<k34>)
                    n1379 = Unbundle(w2262) -> ("CYCLE"=w2258:dbl, "STATUS"=w2263:string)  [unwired: 1 out]
                    n1380 = Not Equal?(x=w2263, y="RUN") -> (x != y?=w2257:bool)
                    n1381 = Greater?(x=w2258, y=2.0) -> (0:w2259:bool)
                    n1382 = And(x=w2259, y=w2257) -> (x .and. y?=w2256:bool)
                    n1383 = case shown="True" w2256 {
                      tunnel: w2262 -> [_ w2266]
                      tunnel: w2261 -> [_ w2265]
                      frame False {
                      }
                      frame True {
                        n1384 = stacked-sequence {
                          tunnel: w2266 -> [w2269 _ _]
                          tunnel: w2265 -> [_ w2271 _]
                          frame #0 {
                            w2267 = FALSE
                            n1385 = local write "mail control"("END") -> ()
                            n1386 = Bundle(cluster=w2269) -> (w2270:T4)  [unwired: 3 in]
                            n1387 = local write "O/I  LAB03-1"(w2267) -> ()
                            n1388 = local write "run lab03-1"(w2267) -> ()
                            n1389 = local write "RUN LAB03-1"(w2267) -> ()
                            n1390 = local write "DISP LAB03-1"(w2270) -> ()
                          }
                          frame #1 {
                            n1391 = TDMS Close(11:w2271) -> (0:w2272:errorcluster)  [unwired: 1 in, 1 out]
                            n1392 = local write "data file error"(w2272) -> ()
                          }
                          frame #2 {
                            n1393 = stacked-sequence {
                              tunnel: "LAB03-1" -> [w2275 w2277]
                              frame #0 {
                                n1394 = call "sub vi - defrag tdms v1.vi"("panel id"=w2275) -> ("error out"=w2274:errorcluster)  [unwired: 10 in]
                                n1395 = local write "data file error"(w2274) -> ()
                              }
                              frame #1 {
                                n1396 = call "Save data file to network drive v1.vi"("panel id"=w2277) -> ("network file save error"=w2276:errorcluster)  [unwired: 9 in, 1 out]
                                n1397 = local write "data file error"(w2276) -> ()
                              }
                            }
                          }
                        }
                      }
                    }
                  }
                }
              }
              frame #5 {
                # "LAB03-2"
                n1398 = local read "run lab03-2"() -> (w2278:bool)
                n1399 = case shown="True" w2278 {
                  frame False {
                  }
                  frame True {
                    n1400 = local read "DISP LAB03-2"() -> (w2285:T4)
                    n1401 = Unbundle(w2285) -> ("CYCLE"=w2281:dbl, "STATUS"=w2286:string)  [unwired: 1 out]
                    n1402 = local read "TDMS LAB03-2"() -> (w2284:refnum<k34>)
                    n1403 = Not Equal?(x=w2286, y="RUN") -> (x != y?=w2280:bool)
                    n1404 = Greater?(x=w2281, y=2.0) -> (0:w2282:bool)
                    n1405 = And(x=w2282, y=w2280) -> (x .and. y?=w2279:bool)
                    n1406 = case shown="True" w2279 {
                      tunnel: w2285 -> [_ w2289]
                      tunnel: w2284 -> [_ w2288]
                      frame False {
                      }
                      frame True {
                        n1407 = stacked-sequence {
                          tunnel: w2289 -> [w2292 _ _]
                          tunnel: w2288 -> [_ w2294 _]
                          frame #0 {
                            w2290 = FALSE
                            n1408 = local write "mail control"("END") -> ()
                            n1409 = Bundle(cluster=w2292) -> (w2293:T4)  [unwired: 3 in]
                            n1410 = local write "RUN LAB03-2"(w2290) -> ()
                            n1411 = local write "O/I  LAB03-2"(w2290) -> ()
                            n1412 = local write "DISP LAB03-2"(w2293) -> ()
                            n1413 = local write "run lab03-2"(w2290) -> ()
                          }
                          frame #1 {
                            n1414 = TDMS Close(11:w2294) -> (0:w2295:errorcluster)  [unwired: 1 in, 1 out]
                            n1415 = local write "data file error"(w2295) -> ()
                          }
                          frame #2 {
                            n1416 = stacked-sequence {
                              tunnel: "LAB03-2" -> [w2298 w2300]
                              frame #0 {
                                n1417 = call "sub vi - defrag tdms v1.vi"("panel id"=w2298) -> ("error out"=w2297:errorcluster)  [unwired: 10 in]
                                n1418 = local write "data file error"(w2297) -> ()
                              }
                              frame #1 {
                                n1419 = call "Save data file to network drive v1.vi"("panel id"=w2300) -> ("network file save error"=w2299:errorcluster)  [unwired: 9 in, 1 out]
                                n1420 = local write "data file error"(w2299) -> ()
                              }
                            }
                          }
                        }
                      }
                    }
                  }
                }
              }
              frame #6 {
                # "LAB04-1"
                n1421 = local read "run lab04-1"() -> (w2301:bool)
                n1422 = case shown="True" w2301 {
                  frame False {
                  }
                  frame True {
                    n1423 = local read "DISP LAB04-1"() -> (w2308:T4)
                    n1424 = Unbundle(w2308) -> ("CYCLE"=w2304:dbl, "STATUS"=w2309:string)  [unwired: 1 out]
                    n1425 = local read "TDMS LAB04-1"() -> (w2307:refnum<k34>)
                    n1426 = Not Equal?(x=w2309, y="RUN") -> (x != y?=w2303:bool)
                    n1427 = Greater?(x=w2304, y=2.0) -> (0:w2305:bool)
                    n1428 = And(x=w2305, y=w2303) -> (x .and. y?=w2302:bool)
                    n1429 = case shown="True" w2302 {
                      tunnel: w2308 -> [_ w2312]
                      tunnel: w2307 -> [_ w2311]
                      frame False {
                      }
                      frame True {
                        n1430 = stacked-sequence {
                          tunnel: w2312 -> [w2315 _ _]
                          tunnel: w2311 -> [_ w2317 _]
                          frame #0 {
                            w2313 = FALSE
                            n1431 = local write "mail control"("END") -> ()
                            n1432 = Bundle(cluster=w2315) -> (w2316:T4)  [unwired: 3 in]
                            n1433 = local write "RUN LAB04-1"(w2313) -> ()
                            n1434 = local write "O/I  LAB04-1"(w2313) -> ()
                            n1435 = local write "run lab04-1"(w2313) -> ()
                            n1436 = local write "DISP LAB04-1"(w2316) -> ()
                          }
                          frame #1 {
                            n1437 = TDMS Close(11:w2317) -> (0:w2318:errorcluster)  [unwired: 1 in, 1 out]
                            n1438 = local write "data file error"(w2318) -> ()
                          }
                          frame #2 {
                            n1439 = stacked-sequence {
                              tunnel: "LAB04-1" -> [w2321 w2323]
                              frame #0 {
                                n1440 = call "sub vi - defrag tdms v1.vi"("panel id"=w2321) -> ("error out"=w2320:errorcluster)  [unwired: 10 in]
                                n1441 = local write "data file error"(w2320) -> ()
                              }
                              frame #1 {
                                n1442 = call "Save data file to network drive v1.vi"("panel id"=w2323) -> ("network file save error"=w2322:errorcluster)  [unwired: 9 in, 1 out]
                                n1443 = local write "data file error"(w2322) -> ()
                              }
                            }
                          }
                        }
                      }
                    }
                  }
                }
              }
              frame #7 {
                # "LAB04-2"
                n1444 = local read "run lab04-2"() -> (w2324:bool)
                n1445 = case shown="True" w2324 {
                  frame False {
                  }
                  frame True {
                    n1446 = local read "DISP LAB04-2"() -> (w2331:T4)
                    n1447 = Unbundle(w2331) -> ("CYCLE"=w2327:dbl, "STATUS"=w2332:string)  [unwired: 1 out]
                    n1448 = Not Equal?(x=w2332, y="RUN") -> (x != y?=w2326:bool)
                    n1449 = local read "TDMS LAB04-2"() -> (w2330:refnum<k34>)
                    n1450 = Greater?(x=w2327, y=2.0) -> (0:w2328:bool)
                    n1451 = And(x=w2328, y=w2326) -> (x .and. y?=w2325:bool)
                    n1452 = case shown="True" w2325 {
                      tunnel: w2331 -> [_ w2335]
                      tunnel: w2330 -> [_ w2334]
                      frame False {
                      }
                      frame True {
                        n1453 = stacked-sequence {
                          tunnel: w2335 -> [w2338 _ _]
                          tunnel: w2334 -> [_ w2340 _]
                          frame #0 {
                            w2336 = FALSE
                            n1454 = local write "mail control"("END") -> ()
                            n1455 = Bundle(cluster=w2338) -> (w2339:T4)  [unwired: 3 in]
                            n1456 = local write "O/I  LAB04-2"(w2336) -> ()
                            n1457 = local write "RUN LAB04-2"(w2336) -> ()
                            n1458 = local write "run lab04-2"(w2336) -> ()
                            n1459 = local write "DISP LAB04-2"(w2339) -> ()
                          }
                          frame #1 {
                            n1460 = TDMS Close(11:w2340) -> (0:w2341:errorcluster)  [unwired: 1 in, 1 out]
                            n1461 = local write "data file error"(w2341) -> ()
                          }
                          frame #2 {
                            n1462 = stacked-sequence {
                              tunnel: "LAB04-2" -> [w2344 w2346]
                              frame #0 {
                                n1463 = call "sub vi - defrag tdms v1.vi"("panel id"=w2344) -> ("error out"=w2343:errorcluster)  [unwired: 10 in]
                                n1464 = local write "data file error"(w2343) -> ()
                              }
                              frame #1 {
                                n1465 = call "Save data file to network drive v1.vi"("panel id"=w2346) -> ("network file save error"=w2345:errorcluster)  [unwired: 9 in, 1 out]
                                n1466 = local write "data file error"(w2345) -> ()
                              }
                            }
                          }
                        }
                      }
                    }
                  }
                }
              }
              frame #8 {
                # "LAB05-1"
                n1467 = local read "run lab05-1"() -> (w2347:bool)
                n1468 = case shown="True" w2347 {
                  frame False {
                  }
                  frame True {
                    n1469 = local read "DISP LAB05-1"() -> (w2354:T4)
                    n1470 = Unbundle(w2354) -> ("CYCLE"=w2350:dbl, "STATUS"=w2355:string)  [unwired: 1 out]
                    n1471 = Not Equal?(x=w2355, y="RUN") -> (x != y?=w2349:bool)
                    n1472 = local read "TDMS LAB05-1"() -> (w2353:refnum<k34>)
                    n1473 = Greater?(x=w2350, y=2.0) -> (0:w2351:bool)
                    n1474 = And(x=w2351, y=w2349) -> (x .and. y?=w2348:bool)
                    n1475 = case shown="True" w2348 {
                      tunnel: w2354 -> [_ w2358]
                      tunnel: w2353 -> [_ w2357]
                      frame False {
                      }
                      frame True {
                        n1476 = stacked-sequence {
                          tunnel: w2358 -> [w2361 _ _]
                          tunnel: w2357 -> [_ w2363 _]
                          frame #0 {
                            w2359 = FALSE
                            n1477 = local write "mail control"("END") -> ()
                            n1478 = Bundle(cluster=w2361) -> (w2362:T4)  [unwired: 3 in]
                            n1479 = local write "O/I  LAB05-1"(w2359) -> ()
                            n1480 = local write "RUN LAB05-1"(w2359) -> ()
                            n1481 = local write "run lab05-1"(w2359) -> ()
                            n1482 = local write "DISP LAB05-1"(w2362) -> ()
                          }
                          frame #1 {
                            n1483 = TDMS Close(11:w2363) -> (0:w2364:errorcluster)  [unwired: 1 in, 1 out]
                            n1484 = local write "data file error"(w2364) -> ()
                          }
                          frame #2 {
                            n1485 = stacked-sequence {
                              tunnel: "LAB05-1" -> [w2367 w2369]
                              frame #0 {
                                n1486 = call "sub vi - defrag tdms v1.vi"("panel id"=w2367) -> ("error out"=w2366:errorcluster)  [unwired: 10 in]
                                n1487 = local write "data file error"(w2366) -> ()
                              }
                              frame #1 {
                                n1488 = call "Save data file to network drive v1.vi"("panel id"=w2369) -> ("network file save error"=w2368:errorcluster)  [unwired: 9 in, 1 out]
                                n1489 = local write "data file error"(w2368) -> ()
                              }
                            }
                          }
                        }
                      }
                    }
                  }
                }
              }
              frame #9 {
                # "LAB05-2"
                n1490 = local read "run lab05-2"() -> (w2370:bool)
                n1491 = case shown="True" w2370 {
                  frame False {
                  }
                  frame True {
                    n1492 = local read "DISP LAB05-2"() -> (w2377:T4)
                    n1493 = Unbundle(w2377) -> ("CYCLE"=w2373:dbl, "STATUS"=w2378:string)  [unwired: 1 out]
                    n1494 = Not Equal?(x=w2378, y="RUN") -> (x != y?=w2372:bool)
                    n1495 = local read "TDMS LAB05-2"() -> (w2376:refnum<k34>)
                    n1496 = Greater?(x=w2373, y=2.0) -> (0:w2374:bool)
                    n1497 = And(x=w2374, y=w2372) -> (x .and. y?=w2371:bool)
                    n1498 = case shown="True" w2371 {
                      tunnel: w2377 -> [_ w2381]
                      tunnel: w2376 -> [_ w2380]
                      frame False {
                      }
                      frame True {
                        n1499 = stacked-sequence {
                          tunnel: w2381 -> [w2384 _ _]
                          tunnel: w2380 -> [_ w2386 _]
                          frame #0 {
                            w2382 = FALSE
                            n1500 = local write "mail control"("END") -> ()
                            n1501 = Bundle(cluster=w2384) -> (w2385:T4)  [unwired: 3 in]
                            n1502 = local write "RUN LAB05-2"(w2382) -> ()
                            n1503 = local write "O/I  LAB05-2"(w2382) -> ()
                            n1504 = local write "run lab05-2"(w2382) -> ()
                            n1505 = local write "DISP LAB05-2"(w2385) -> ()
                          }
                          frame #1 {
                            n1506 = TDMS Close(11:w2386) -> (0:w2387:errorcluster)  [unwired: 1 in, 1 out]
                            n1507 = local write "data file error"(w2387) -> ()
                          }
                          frame #2 {
                            n1508 = stacked-sequence {
                              tunnel: "LAB05-2" -> [w2390 w2392]
                              frame #0 {
                                n1509 = call "sub vi - defrag tdms v1.vi"("panel id"=w2390) -> ("error out"=w2389:errorcluster)  [unwired: 10 in]
                                n1510 = local write "data file error"(w2389) -> ()
                              }
                              frame #1 {
                                n1511 = call "Save data file to network drive v1.vi"("panel id"=w2392) -> ("network file save error"=w2391:errorcluster)  [unwired: 9 in, 1 out]
                                n1512 = local write "data file error"(w2391) -> ()
                              }
                            }
                          }
                        }
                      }
                    }
                  }
                }
              }
            }
            n1513 = local read "Network Directory"() -> (w2148:path)
            n1514 = global write "Global 1.vi" "Network Drive"(w2148) -> ()
          }
          frame #7 {
            # "disable functions"
            n1515 = stacked-sequence {
              tunnel: w2402 -> [w2416 _ w2472]
              tunnel: w2401 -> [w2411 _ w2471]
              tunnel: w2400 -> [w2410 _ w2470]
              tunnel: w2399 -> [w2408 _ w2469]
              tunnel: w2398 -> [w2409 _ w2468]
              tunnel: w2397 -> [_ w2433 w2467]
              tunnel: w2396 -> [_ w2434 w2466]
              tunnel: w2395 -> [_ w2435 w2465]
              tunnel: w2394 -> [_ w2436 w2464]
              tunnel: w2393 -> [_ w2437 w2463]
              frame #0 {
                n1516 = Select(t=2, s=w2408, f=0) -> (s? t:f=w2404:i32)
                n1517 = Select(t=2, s=w2410, f=0) -> (s? t:f=w2405:i32)
                n1518 = Select(t=2, s=w2409, f=0) -> (s? t:f=w2403:i32)
                n1519 = Select(t=2, s=w2416, f=0) -> (s? t:f=w2407:i32)
                n1520 = Select(t=2, s=w2411, f=0) -> (s? t:f=w2406:i32)
                n1521 = property on="SELECT LAB02-2" class="RadioBtnsControl (strict)"("DisabledEnum"=w2404) -> ()  [unwired: 2 in, 2 out]
                n1522 = property on="SELECT LAB02-1" class="RadioBtnsControl (strict)"("DisabledEnum"=w2405) -> ()  [unwired: 2 in, 2 out]
                n1523 = property on="SELECT LAB03-1" class="RadioBtnsControl (strict)"("DisabledEnum"=w2403) -> ()  [unwired: 2 in, 2 out]
                n1524 = property on="SELECT LAB01-1" class="RadioBtnsControl (strict)"("DisabledEnum"=w2407) -> ()  [unwired: 2 in, 2 out]
                n1525 = property on="SELECT LAB01-2" class="RadioBtnsControl (strict)"("DisabledEnum"=w2406) -> ()  [unwired: 2 in, 2 out]
                n1526 = Not(x=w2416) -> (.not. x?=w2417:bool)
                n1527 = property on="RESULT LAB01-1" class="Bool (strict)"("Visible"=w2417) -> ()  [unwired: 2 in, 2 out]
                n1528 = Not(x=w2411) -> (.not. x?=w2415:bool)
                n1529 = Not(x=w2410) -> (.not. x?=w2414:bool)
                n1530 = Not(x=w2408) -> (.not. x?=w2413:bool)
                n1531 = property on="RESULT LAB01-2" class="Bool (strict)"("Visible"=w2415) -> ()  [unwired: 2 in, 2 out]
                n1532 = Not(x=w2409) -> (.not. x?=w2412:bool)
                n1533 = property on="RESULT LAB02-1" class="Bool (strict)"("Visible"=w2414) -> ()  [unwired: 2 in, 2 out]
                n1534 = property on="RESULT LAB02-2" class="Bool (strict)"("Visible"=w2413) -> ()  [unwired: 2 in, 2 out]
                n1535 = property on="RESULT LAB03-1" class="Bool (strict)"("Visible"=w2412) -> ()  [unwired: 2 in, 2 out]
                n1536 = property on="SET LAB01-1" class="Clust (strict)"("DisabledEnum"=w2407) -> ()  [unwired: 2 in, 2 out]
                n1537 = property on="SET LAB01-2" class="Clust (strict)"("DisabledEnum"=w2406) -> ()  [unwired: 2 in, 2 out]
                n1538 = property on="SET LAB02-1" class="Clust (strict)"("DisabledEnum"=w2405) -> ()  [unwired: 2 in, 2 out]
                n1539 = property on="SET LAB02-2" class="Clust (strict)"("DisabledEnum"=w2404) -> ()  [unwired: 2 in, 2 out]
                n1540 = property on="SET LAB03-1" class="Clust (strict)"("DisabledEnum"=w2403) -> ()  [unwired: 2 in, 2 out]
                n1541 = property on="O/I  LAB01-1" class="Bool (strict)"("DisabledEnum"=w2407) -> ()  [unwired: 2 in, 2 out]
                n1542 = property on="O/I  LAB01-2" class="Bool (strict)"("DisabledEnum"=w2406) -> ()  [unwired: 2 in, 2 out]
                n1543 = property on="O/I  LAB02-1" class="Bool (strict)"("DisabledEnum"=w2405) -> ()  [unwired: 2 in, 2 out]
                n1544 = property on="O/I  LAB02-2" class="Bool (strict)"("DisabledEnum"=w2404) -> ()  [unwired: 2 in, 2 out]
                n1545 = property on="O/I  LAB03-1" class="Bool (strict)"("DisabledEnum"=w2403) -> ()  [unwired: 2 in, 2 out]
              }
              frame #1 {
                n1546 = Select(t=2, s=w2437, f=0) -> (s? t:f=w2428:i32)
                n1547 = Select(t=2, s=w2436, f=0) -> (s? t:f=w2429:i32)
                n1548 = Select(t=2, s=w2433, f=0) -> (s? t:f=w2432:i32)
                n1549 = Select(t=2, s=w2434, f=0) -> (s? t:f=w2431:i32)
                n1550 = Select(t=2, s=w2435, f=0) -> (s? t:f=w2430:i32)
                n1551 = property on="SELECT LAB05-2" class="RadioBtnsControl (strict)"("DisabledEnum"=w2428) -> ()  [unwired: 2 in, 2 out]
                n1552 = property on="SELECT LAB05-1" class="RadioBtnsControl (strict)"("DisabledEnum"=w2429) -> ()  [unwired: 2 in, 2 out]
                n1553 = property on="SELECT LAB03-2" class="RadioBtnsControl (strict)"("DisabledEnum"=w2432) -> ()  [unwired: 2 in, 2 out]
                n1554 = property on="SELECT LAB04-1" class="RadioBtnsControl (strict)"("DisabledEnum"=w2431) -> ()  [unwired: 2 in, 2 out]
                n1555 = property on="SELECT LAB04-2" class="RadioBtnsControl (strict)"("DisabledEnum"=w2430) -> ()  [unwired: 2 in, 2 out]
                n1556 = property on="SET LAB05-2" class="Clust (strict)"("DisabledEnum"=w2428) -> ()  [unwired: 2 in, 2 out]
                n1557 = property on="SET LAB05-1" class="Clust (strict)"("DisabledEnum"=w2429) -> ()  [unwired: 2 in, 2 out]
                n1558 = property on="SET LAB03-2" class="Clust (strict)"("DisabledEnum"=w2432) -> ()  [unwired: 2 in, 2 out]
                n1559 = property on="SET LAB04-1" class="Clust (strict)"("DisabledEnum"=w2431) -> ()  [unwired: 2 in, 2 out]
                n1560 = property on="SET LAB04-2" class="Clust (strict)"("DisabledEnum"=w2430) -> ()  [unwired: 2 in, 2 out]
                n1561 = property on="O/I  LAB05-2" class="Bool (strict)"("DisabledEnum"=w2428) -> ()  [unwired: 2 in, 2 out]
                n1562 = property on="O/I  LAB05-1" class="Bool (strict)"("DisabledEnum"=w2429) -> ()  [unwired: 2 in, 2 out]
                n1563 = property on="O/I  LAB04-1" class="Bool (strict)"("DisabledEnum"=w2431) -> ()  [unwired: 2 in, 2 out]
                n1564 = property on="O/I  LAB04-2" class="Bool (strict)"("DisabledEnum"=w2430) -> ()  [unwired: 2 in, 2 out]
                n1565 = property on="O/I  LAB03-2" class="Bool (strict)"("DisabledEnum"=w2432) -> ()  [unwired: 2 in, 2 out]
                n1566 = Not(x=w2437) -> (.not. x?=w2438:bool)
                n1567 = Not(x=w2436) -> (.not. x?=w2439:bool)
                n1568 = Not(x=w2435) -> (.not. x?=w2440:bool)
                n1569 = property on="RESULT LAB05-2" class="Bool (strict)"("Visible"=w2438) -> ()  [unwired: 2 in, 2 out]
                n1570 = property on="RESULT LAB05-1" class="Bool (strict)"("Visible"=w2439) -> ()  [unwired: 2 in, 2 out]
                n1571 = Not(x=w2434) -> (.not. x?=w2441:bool)
                n1572 = property on="RESULT LAB04-2" class="Bool (strict)"("Visible"=w2440) -> ()  [unwired: 2 in, 2 out]
                n1573 = Not(x=w2433) -> (.not. x?=w2442:bool)
                n1574 = property on="RESULT LAB04-1" class="Bool (strict)"("Visible"=w2441) -> ()  [unwired: 2 in, 2 out]
                n1575 = property on="RESULT LAB03-2" class="Bool (strict)"("Visible"=w2442) -> ()  [unwired: 2 in, 2 out]
              }
              frame #2 {
                # "disable calibrate if any test running"
                n1576 = Or(x=w2464, y=w2463) -> (x .or. y?=w2457:bool)
                n1577 = Or(x=w2466, y=w2465) -> (x .or. y?=w2459:bool)
                n1578 = Or(x=w2470, y=w2469) -> (x .or. y?=w2461:bool)
                n1579 = Or(x=w2468, y=w2467) -> (x .or. y?=w2460:bool)
                n1580 = Or(x=w2472, y=w2471) -> (x .or. y?=w2462:bool)
                n1581 = Or(x=w2460, y=w2459) -> (x .or. y?=w2458:bool)
                n1582 = Or(x=w2462, y=w2461) -> (x .or. y?=w2456:bool)
                n1583 = Or(x=w2458, y=w2457) -> (x .or. y?=w2455:bool)
                n1584 = Or(x=w2456, y=w2455) -> (x .or. y?=w2454:bool)
                n1585 = case shown="True" w2454 {
                  tunnel: [0 2] -> w2453
                  frame False {
                  }
                  frame True {
                  }
                }
                n1586 = property on="JIG TEST" class="Clust (strict)"("DisabledEnum"=w2453) -> ()  [unwired: 2 in, 2 out]
                n1587 = property on="Network Directory" class="Path"("DisabledEnum"=w2453) -> ()  [unwired: 2 in, 2 out]
                n1588 = property on="MAIL SETTINGS" class="Clust (strict)"("DisabledEnum"=w2453) -> ()  [unwired: 2 in, 2 out]
                n1589 = property on="CALIBRATE" class="Bool (strict)"("DisabledEnum"=w2453) -> ()  [unwired: 2 in, 2 out]
                n1590 = property on="ADMIN PAGE" class="Bool (strict)"("DisabledEnum"=w2453) -> ()  [unwired: 2 in, 2 out]
              }
            }
          }
          frame #8 {
            # "drive jigs"
            n1591 = stacked-sequence {
              frame #0 {
                # "jig on"
                n1592 = local read "jig cycle"() -> (w2480:dbl)
                n1593 = property on="JIG TEST" class="Clust (strict)"() -> ("DisabledEnum"=w2477:T14)  [unwired: 2 in, 2 out]
                n1594 = Equal?(x=w2477, y=2) -> (x = y?=w2476:bool)
                n1595 = Equal?(x=w2480, y=0) -> (x = y?=w2478:bool)
                n1596 = And(x=w2478, y=w2476) -> (x .and. y?=w2475:bool)
                n1597 = case shown="True" w2475 {
                  frame False {
                  }
                  frame True {
                    n1598 = local read "run lab01-1"() -> (w2491:bool)
                    n1599 = local read "run lab01-2"() -> (w2490:bool)
                    n1600 = local read "run lab02-1"() -> (w2489:bool)
                    n1601 = local read "run lab02-2"() -> (w2488:bool)
                    n1602 = local read "run lab03-1"() -> (w2487:bool)
                    n1603 = local read "run lab03-2"() -> (w2486:bool)
                    n1604 = local read "run lab04-1"() -> (w2485:bool)
                    n1605 = local read "run lab04-2"() -> (w2484:bool)
                    n1606 = local read "run lab05-1"() -> (w2483:bool)
                    n1607 = local read "run lab05-2"() -> (w2482:bool)
                    n1608 = local write "JIG LAB03-2"(w2486) -> ()
                    n1609 = local write "JIG LAB01-1"(w2491) -> ()
                    n1610 = local write "JIG LAB01-2"(w2490) -> ()
                    n1611 = local write "JIG LAB02-1"(w2489) -> ()
                    n1612 = local write "JIG LAB02-2"(w2488) -> ()
                    n1613 = local write "JIG LAB03-1"(w2487) -> ()
                    n1614 = local write "JIG LAB04-1"(w2485) -> ()
                    n1615 = local write "JIG LAB04-2"(w2484) -> ()
                    n1616 = local write "JIG LAB05-1"(w2483) -> ()
                    n1617 = local write "JIG LAB05-2"(w2482) -> ()
                  }
                }
              }
              frame #1 {
                # "jig off"
                n1618 = local read "jig cycle"() -> (w2498:dbl)
                n1619 = local read "on loops"() -> (w2497:dbl)
                n1620 = property on="JIG TEST" class="Clust (strict)"() -> ("DisabledEnum"=w2496:T14)  [unwired: 2 in, 2 out]
                n1621 = Equal?(x=w2496, y=2) -> (x = y?=w2494:bool)
                n1622 = Equal?(x=w2498, y=w2497) -> (x = y?=w2493:bool)
                n1623 = And(x=w2493, y=w2494) -> (x .and. y?=w2492:bool)
                n1624 = case shown="True" w2492 {
                  frame False {
                  }
                  frame True {
                    w2549 = FALSE
                    w2550 = TRUE
                    w2548 = 2
                    n1625 = local read "SELECT LAB05-2"() -> (w2539:T3)
                    n1626 = local read "SELECT LAB04-2"() -> (w2541:T3)
                    n1627 = local read "SELECT LAB04-1"() -> (w2542:T3)
                    n1628 = local read "SELECT LAB05-1"() -> (w2540:T3)
                    n1629 = local read "SELECT LAB03-2"() -> (w2543:T3)
                    n1630 = local read "SELECT LAB02-1"() -> (w2546:T3)
                    n1631 = local read "SELECT LAB03-1"() -> (w2544:T3)
                    n1632 = local read "SELECT LAB02-2"() -> (w2545:T3)
                    n1633 = local read "SELECT LAB01-2"() -> (w2547:T3)
                    n1634 = local read "run lab05-1"() -> (w2509:bool)
                    n1635 = local read "run lab05-2"() -> (w2508:bool)
                    n1636 = local read "SELECT LAB01-1"() -> (w2551:T3)
                    n1637 = local read "run lab04-2"() -> (w2510:bool)
                    n1638 = local read "run lab04-1"() -> (w2511:bool)
                    n1639 = local read "run lab01-1"() -> (w2527:bool)
                    n1640 = local read "run lab01-2"() -> (w2516:bool)
                    n1641 = local read "run lab03-2"() -> (w2512:bool)
                    n1642 = local read "run lab03-1"() -> (w2513:bool)
                    n1643 = local read "run lab02-1"() -> (w2515:bool)
                    n1644 = local read "run lab02-2"() -> (w2514:bool)
                    n1645 = Equal?(x=w2548, y=w2544) -> (x = y?=w2522:bool)
                    n1646 = Equal?(x=w2548, y=w2543) -> (x = y?=w2521:bool)
                    n1647 = Equal?(x=w2548, y=w2542) -> (x = y?=w2520:bool)
                    n1648 = Equal?(x=w2548, y=w2541) -> (x = y?=w2519:bool)
                    n1649 = Equal?(x=w2548, y=w2540) -> (x = y?=w2518:bool)
                    n1650 = Equal?(x=w2548, y=w2539) -> (x = y?=w2517:bool)
                    n1651 = Equal?(x=w2548, y=w2551) -> (x = y?=w2528:bool)
                    n1652 = Equal?(x=w2548, y=w2546) -> (x = y?=w2524:bool)
                    n1653 = Equal?(x=w2548, y=w2545) -> (x = y?=w2523:bool)
                    n1654 = Equal?(x=w2548, y=w2547) -> (x = y?=w2525:bool)
                    n1655 = And(x=w2519, y=w2510) -> (x .and. y?=w2501:bool)
                    n1656 = And(x=w2522, y=w2513) -> (x .and. y?=w2504:bool)
                    n1657 = And(x=w2520, y=w2511) -> (x .and. y?=w2502:bool)
                    n1658 = And(x=w2517, y=w2508) -> (x .and. y?=w2499:bool)
                    n1659 = And(x=w2523, y=w2514) -> (x .and. y?=w2505:bool)
                    n1660 = And(x=w2521, y=w2512) -> (x .and. y?=w2503:bool)
                    n1661 = And(x=w2518, y=w2509) -> (x .and. y?=w2500:bool)
                    n1662 = And(x=w2525, y=w2516) -> (x .and. y?=w2507:bool)
                    n1663 = And(x=w2528, y=w2527) -> (x .and. y?=w2526:bool)
                    n1664 = And(x=w2524, y=w2515) -> (x .and. y?=w2506:bool)
                    n1665 = Select(t=w2550, s=w2526, f=w2549) -> (s? t:f=w2529:bool)
                    n1666 = Select(t=w2550, s=w2507, f=w2549) -> (s? t:f=w2530:bool)
                    n1667 = Select(t=w2550, s=w2506, f=w2549) -> (s? t:f=w2531:bool)
                    n1668 = Select(t=w2550, s=w2505, f=w2549) -> (s? t:f=w2532:bool)
                    n1669 = Select(t=w2550, s=w2504, f=w2549) -> (s? t:f=w2533:bool)
                    n1670 = Select(t=w2550, s=w2503, f=w2549) -> (s? t:f=w2534:bool)
                    n1671 = Select(t=w2550, s=w2502, f=w2549) -> (s? t:f=w2535:bool)
                    n1672 = Select(t=w2550, s=w2501, f=w2549) -> (s? t:f=w2536:bool)
                    n1673 = Select(t=w2550, s=w2500, f=w2549) -> (s? t:f=w2537:bool)
                    n1674 = Select(t=w2550, s=w2499, f=w2549) -> (s? t:f=w2538:bool)
                    n1675 = local write "JIG LAB03-2"(w2534) -> ()
                    n1676 = local write "JIG LAB02-1"(w2531) -> ()
                    n1677 = local write "JIG LAB02-2"(w2532) -> ()
                    n1678 = local write "JIG LAB01-2"(w2530) -> ()
                    n1679 = local write "JIG LAB03-1"(w2533) -> ()
                    n1680 = local write "JIG LAB01-1"(w2529) -> ()
                    n1681 = local write "JIG LAB05-2"(w2538) -> ()
                    n1682 = local write "JIG LAB04-1"(w2535) -> ()
                    n1683 = local write "JIG LAB05-1"(w2537) -> ()
                    n1684 = local write "JIG LAB04-2"(w2536) -> ()
                  }
                }
              }
            }
          }
          frame #9 {
            # "enable  jig test output if no test busy"
            n1685 = property on="JIG TEST" class="Clust (strict)"() -> ("DisabledEnum"=w2554:T14)  [unwired: 2 in, 2 out]
            n1686 = Equal?(x=w2554, y=0) -> (x = y?=w2552:bool)
            n1687 = case shown="True" w2552 {
              frame False {
              }
              frame True {
                n1688 = local read "JIG TEST"() -> (w2565:T11)
                n1689 = Unbundle(w2565) -> ("LAB01-1"=w2564:bool, "LAB01-2"=w2563:bool, "LAB02-1"=w2562:bool, "LAB02-2"=w2561:bool, "LAB03-1"=w2560:bool, "LAB03-2"=w2559:bool, "LAB04-1"=w2558:bool, "LAB04-2"=w2557:bool, "LAB05-1"=w2556:bool, "LAB05-2"=w2555:bool)
                n1690 = local write "JIG LAB05-1"(w2556) -> ()
                n1691 = local write "JIG LAB05-2"(w2555) -> ()
                n1692 = local write "JIG LAB04-1"(w2558) -> ()
                n1693 = local write "JIG LAB04-2"(w2557) -> ()
                n1694 = local write "JIG LAB03-2"(w2559) -> ()
                n1695 = local write "JIG LAB01-1"(w2564) -> ()
                n1696 = local write "JIG LAB02-1"(w2562) -> ()
                n1697 = local write "JIG LAB03-1"(w2560) -> ()
                n1698 = local write "JIG LAB01-2"(w2563) -> ()
                n1699 = local write "JIG LAB02-2"(w2561) -> ()
              }
            }
          }
          frame #10 {
            # "drive digital output"
            n1700 = local read "O/I  LAB05-2"() -> (w2571:bool)
            n1701 = local read "O/I  LAB05-1"() -> (w2573:bool)
            n1702 = local read "JIG LAB05-2"() -> (w2570:bool)
            n1703 = local read "O/I  LAB04-2"() -> (w2575:bool)
            n1704 = local read "JIG LAB05-1"() -> (w2572:bool)
            n1705 = local read "JIG LAB04-2"() -> (w2574:bool)
            n1706 = local read "O/I  LAB03-1"() -> (w2580:bool)
            n1707 = local read "O/I  LAB04-1"() -> (w2576:bool)
            n1708 = local read "O/I  LAB02-1"() -> (w2584:bool)
            n1709 = local read "O/I  LAB02-2"() -> (w2582:bool)
            n1710 = local read "O/I  LAB03-2"() -> (w2578:bool)
            n1711 = local read "JIG LAB04-1"() -> (w2569:bool)
            n1712 = local read "JIG LAB03-2"() -> (w2577:bool)
            n1713 = local read "O/I  LAB01-2"() -> (w2586:bool)
            n1714 = local read "JIG LAB02-1"() -> (w2583:bool)
            n1715 = local read "JIG LAB02-2"() -> (w2581:bool)
            n1716 = local read "JIG LAB03-1"() -> (w2579:bool)
            n1717 = local read "O/I  LAB01-1"() -> (w2588:bool)
            n1718 = local read "JIG LAB01-2"() -> (w2585:bool)
            n1719 = local read "JIG LAB01-1"() -> (w2587:bool)
            n1720 = Build Array(w2575, w2574, w2573, w2572, w2571, w2570) -> (w2566:bool[])
            n1721 = Build Array(w2581, w2580, w2579, w2578, w2577, w2576, w2569) -> (w2567:bool[])
            n1722 = Build Array(w2588, w2587, w2586, w2585, w2584, w2583, w2582) -> (w2568:bool[])
            n1723 = call "sub vi - Drive Relays All v6.vi"("Array #2"=w2566, "Array #1"=w2567, "Array #0"=w2568) -> ()  [unwired: 8 in, 1 out]
          }
          frame #11 {
            # "get temperature values"
            n1724 = stacked-sequence {
              frame #0 {
                n1725 = local read "Select COM port"() -> (w2591:refnum<visa-resource-name>)
                "COM port" <- w2591
                n1726 = local read "jig cycle"() -> (w2592:dbl)
                n1727 = local read "on loops"() -> (w2595:dbl)
                n1728 = local read "jig cycle"() -> (w2597:dbl)
                n1729 = global write "Global 1.vi" "tmp dly lps"("Temp Delay Lps") -> ()
                n1730 = global write "Global 1.vi" "dly value"("Temp Value") -> ()
                n1731 = Add(x=w2595, y=2) -> (x+y=w2596:dbl)
                n1732 = global write "Global 1.vi" "COM port"(w2591) -> ()
                n1733 = Equal?(x=w2597, y=0) -> (x = y?=w2598:bool)
                n1734 = Equal?(x=w2592, y=w2596) -> (x = y?=w2593:bool)
                n1735 = case shown="True" w2598 {
                  frame False {
                  }
                  frame True {
                    w2610 = FALSE
                    w2611 = TRUE
                    n1736 = local write "TEMP update"(TRUE) -> ()
                    n1737 = call "sub vi - GET ALL TEMP v4.vi"("LA01-EN"=w2611, "LA02-EN"=w2611, "LA03-EN"=w2611, "LA04-EN"=w2610, "LA05-EN"=w2610, "Gen Cal Value"=1.0) -> ("LA01 TEMP"=w2609:T22, "LA02 TEMP"=w2607:T22, "LA03 TEMP"=w2606:T22)  [unwired: 4 in, 3 out]
                    n1738 = local write "LAB03 TEMP"(w2606) -> ()
                    n1739 = local write "LAB02 TEMP"(w2607) -> ()
                    n1740 = local write "LAB01 TEMP"(w2609) -> ()
                  }
                }
                n1741 = case shown="True" w2593 {
                  frame False {
                  }
                  frame True {
                    w2603 = TRUE
                    w2604 = FALSE
                    n1742 = local write "TEMP update"(TRUE) -> ()
                    n1743 = call "sub vi - GET ALL TEMP v4.vi"("LA01-EN"=w2604, "LA02-EN"=w2604, "LA03-EN"=w2604, "LA04-EN"=w2603, "LA05-EN"=w2603, "Gen Cal Value"=1.0) -> ("LA04 TEMP"=w2601:T22, "LA05 TEMP"=w2600:T22)  [unwired: 4 in, 4 out]
                    n1744 = local write "LAB04 TEMP"(w2601) -> ()
                    n1745 = local write "LAB05 TEMP"(w2600) -> ()
                  }
                }
              }
              frame #1 {
                n1746 = local read "LAB01 TEMP"() -> (w2618:T13)
                n1747 = local read "TEMP LA01"() -> (w2619:T10)
                n1748 = local read "CAL LAB01"() -> (w2632:T8)
                n1749 = call "sub vi - temperature delay v2.vi"("temp values IN"=w2619, "temp signals"=w2618) -> ("T2-N"=w2614:dbl, "T2-L"=w2615:dbl, "T1-N"=w2616:dbl, "T1-L"=w2617:dbl, "temp values OUT"=w2613:T23)  [unwired: 5 in]
                n1750 = Unbundle By Name(w2632) -> ("1 (TL) cal"=w2623:dbl, "1 (TN) cal"=w2622:dbl, "2 (TL) cal"=w2621:dbl, "2 (TN) cal"=w2620:dbl)  [unwired: 6 out]
                n1751 = local write "TEMP LA01"(w2613) -> ()
                n1752 = Multiply(x=w2617, y=w2623) -> (x*y=w2629:dbl)
                n1753 = Multiply(x=w2616, y=w2622) -> (x*y=w2628:dbl)
                n1754 = Multiply(x=w2615, y=w2621) -> (x*y=w2625:dbl)
                n1755 = Multiply(x=w2614, y=w2620) -> (x*y=w2624:dbl)
                n1756 = local read "SIG LAB01-2"() -> (w2627:T2)
                n1757 = local read "SIG LAB01-1"() -> (w2631:T2)
                n1758 = Bundle By Name(cluster=w2631, "Tmp Live"=w2629, "Tmp Neut"=w2628) -> (w2630:T2)
                n1759 = Bundle By Name(cluster=w2627, "Tmp Live"=w2625, "Tmp Neut"=w2624) -> (w2626:T2)
                n1760 = local write "SIG LAB01-1"(w2630) -> ()
                n1761 = local write "SIG LAB01-2"(w2626) -> ()
              }
              frame #2 {
                n1762 = local read "LAB02 TEMP"() -> (w2639:T13)
                n1763 = local read "TEMP LA02"() -> (w2638:T10)
                n1764 = local read "CAL LAB02"() -> (w2652:T9)
                n1765 = call "sub vi - temperature delay v2.vi"("temp values IN"=w2638, "temp signals"=w2639) -> ("T2-N"=w2633:dbl, "T2-L"=w2634:dbl, "T1-N"=w2635:dbl, "T1-L"=w2636:dbl, "temp values OUT"=w2637:T23)  [unwired: 5 in]
                n1766 = Unbundle By Name(w2652) -> ("1 (TL) cal"=w2643:dbl, "1 (TN) cal"=w2642:dbl, "2 (TL) cal"=w2641:dbl, "2 (TN) cal"=w2640:dbl)  [unwired: 6 out]
                n1767 = local write "TEMP LA02"(w2637) -> ()
                n1768 = Multiply(x=w2636, y=w2643) -> (x*y=w2649:dbl)
                n1769 = Multiply(x=w2635, y=w2642) -> (x*y=w2648:dbl)
                n1770 = Multiply(x=w2634, y=w2641) -> (x*y=w2645:dbl)
                n1771 = Multiply(x=w2633, y=w2640) -> (x*y=w2644:dbl)
                n1772 = local read "SIG LAB02-2"() -> (w2647:T2)
                n1773 = local read "SIG LAB02-1"() -> (w2651:T2)
                n1774 = Bundle By Name(cluster=w2651, "Tmp Live"=w2649, "Tmp Neut"=w2648) -> (w2650:T2)
                n1775 = Bundle By Name(cluster=w2647, "Tmp Live"=w2645, "Tmp Neut"=w2644) -> (w2646:T2)
                n1776 = local write "SIG LAB02-1"(w2650) -> ()
                n1777 = local write "SIG LAB02-2"(w2646) -> ()
              }
              frame #3 {
                n1778 = local read "TEMP LA03"() -> (w2658:T10)
                n1779 = local read "LAB03 TEMP"() -> (w2659:T13)
                n1780 = local read "CAL LAB03"() -> (w2672:T8)
                n1781 = call "sub vi - temperature delay v2.vi"("temp values IN"=w2658, "temp signals"=w2659) -> ("T2-N"=w2653:dbl, "T2-L"=w2654:dbl, "T1-N"=w2655:dbl, "T1-L"=w2656:dbl, "temp values OUT"=w2657:T23)  [unwired: 5 in]
                n1782 = Unbundle By Name(w2672) -> ("1 (TL) cal"=w2663:dbl, "1 (TN) cal"=w2662:dbl, "2 (TL) cal"=w2661:dbl, "2 (TN) cal"=w2660:dbl)  [unwired: 6 out]
                n1783 = local write "TEMP LA03"(w2657) -> ()
                n1784 = Multiply(x=w2656, y=w2663) -> (x*y=w2669:dbl)
                n1785 = Multiply(x=w2655, y=w2662) -> (x*y=w2668:dbl)
                n1786 = Multiply(x=w2654, y=w2661) -> (x*y=w2665:dbl)
                n1787 = Multiply(x=w2653, y=w2660) -> (x*y=w2664:dbl)
                n1788 = local read "SIG LAB03-2"() -> (w2667:T2)
                n1789 = local read "SIG LAB03-1"() -> (w2671:T2)
                n1790 = Bundle By Name(cluster=w2671, "Tmp Live"=w2669, "Tmp Neut"=w2668) -> (w2670:T2)
                n1791 = Bundle By Name(cluster=w2667, "Tmp Live"=w2665, "Tmp Neut"=w2664) -> (w2666:T2)
                n1792 = local write "SIG LAB03-1"(w2670) -> ()
                n1793 = local write "SIG LAB03-2"(w2666) -> ()
              }
              frame #4 {
                n1794 = local read "LAB04 TEMP"() -> (w2678:T13)
                n1795 = local read "TEMP LA04"() -> (w2679:T10)
                n1796 = local read "CAL LAB04"() -> (w2692:T8)
                n1797 = call "sub vi - temperature delay v2.vi"("temp values IN"=w2679, "temp signals"=w2678) -> ("T2-N"=w2673:dbl, "T2-L"=w2674:dbl, "T1-N"=w2675:dbl, "T1-L"=w2676:dbl, "temp values OUT"=w2677:T23)  [unwired: 5 in]
                n1798 = Unbundle By Name(w2692) -> ("1 (TL) cal"=w2683:dbl, "1 (TN) cal"=w2682:dbl, "2 (TL) cal"=w2681:dbl, "2 (TN) cal"=w2680:dbl)  [unwired: 6 out]
                n1799 = local write "TEMP LA04"(w2677) -> ()
                n1800 = Multiply(x=w2676, y=w2683) -> (x*y=w2689:dbl)
                n1801 = Multiply(x=w2675, y=w2682) -> (x*y=w2688:dbl)
                n1802 = Multiply(x=w2674, y=w2681) -> (x*y=w2685:dbl)
                n1803 = Multiply(x=w2673, y=w2680) -> (x*y=w2684:dbl)
                n1804 = local read "SIG LAB04-2"() -> (w2687:T2)
                n1805 = local read "SIG LAB04-1"() -> (w2691:T2)
                n1806 = Bundle By Name(cluster=w2691, "Tmp Live"=w2689, "Tmp Neut"=w2688) -> (w2690:T2)
                n1807 = Bundle By Name(cluster=w2687, "Tmp Live"=w2685, "Tmp Neut"=w2684) -> (w2686:T2)
                n1808 = local write "SIG LAB04-1"(w2690) -> ()
                n1809 = local write "SIG LAB04-2"(w2686) -> ()
              }
              frame #5 {
                n1810 = local read "LAB05 TEMP"() -> (w2698:T13)
                n1811 = local read "TEMP LA05"() -> (w2699:T10)
                n1812 = local read "CAL LAB05"() -> (w2712:T8)
                n1813 = call "sub vi - temperature delay v2.vi"("temp values IN"=w2699, "temp signals"=w2698) -> ("T2-N"=w2694:dbl, "T2-L"=w2695:dbl, "T1-N"=w2696:dbl, "T1-L"=w2697:dbl, "temp values OUT"=w2693:T23)  [unwired: 5 in]
                n1814 = local write "TEMP LA05"(w2693) -> ()
                n1815 = Unbundle By Name(w2712) -> ("1 (TL) cal"=w2700:dbl, "1 (TN) cal"=w2703:dbl, "2 (TL) cal"=w2702:dbl, "2 (TN) cal"=w2701:dbl)  [unwired: 6 out]
                n1816 = Multiply(x=w2697, y=w2700) -> (x*y=w2709:dbl)
                n1817 = Multiply(x=w2696, y=w2703) -> (x*y=w2708:dbl)
                n1818 = Multiply(x=w2695, y=w2702) -> (x*y=w2705:dbl)
                n1819 = Multiply(x=w2694, y=w2701) -> (x*y=w2704:dbl)
                n1820 = local read "SIG LAB05-2"() -> (w2707:T2)
                n1821 = local read "SIG LAB05-1"() -> (w2711:T2)
                n1822 = Bundle By Name(cluster=w2711, "Tmp Live"=w2709, "Tmp Neut"=w2708) -> (w2710:T2)
                n1823 = Bundle By Name(cluster=w2707, "Tmp Live"=w2705, "Tmp Neut"=w2704) -> (w2706:T2)
                n1824 = local write "SIG LAB05-1"(w2710) -> ()
                n1825 = local write "SIG LAB05-2"(w2706) -> ()
              }
            }
          }
          frame #12 {
            # "get analog values"
            n1826 = local read "on loops"() -> (w2719:dbl)
            n1827 = local read "jig cycle"() -> (w2716:dbl)
            n1828 = Add(x=w2719, y=1) -> (x+y=w2717:dbl)
            n1829 = Equal?(x=w2716, y=1) -> (x = y?=w2714:bool)
            n1830 = Equal?(x=w2716, y=w2717) -> (x = y?=w2715:bool)
            n1831 = Or(x=w2714, y=w2715) -> (x .or. y?=w2713:bool)
            n1832 = case shown="True" w2713 {
              frame False {
              }
              frame True {
                n1833 = call "sub vi - Read Analog All v8.vi"() -> ("Analog loop time"=w2727:dbl, "array GRAPH"=w2726:dynamicdata[], "LAB01"=w2725:T24, "LAB02"=w2724:T25, "LAB03"=w2723:T26, "LAB04"=w2722:T27, "array ERROR"=w2728:errorcluster[], "LAB05"=w2721:T28)  [unwired: 8 in]
                n1834 = stacked-sequence {
                  tunnel: w2728 -> [w2733 _ _ _ _ _]
                  tunnel: w2727 -> [w2732 _ _ _ _ _]
                  tunnel: w2726 -> [w2731 _ _ _ _ _]
                  tunnel: w2725 -> [_ w2778 _ _ _ _]
                  tunnel: w2724 -> [_ _ w2779 _ _ _]
                  tunnel: w2723 -> [_ _ _ w2804 _ _]
                  tunnel: w2722 -> [_ _ _ _ w2827 _]
                  tunnel: w2721 -> [_ _ _ _ _ w2852]
                  frame #0 {
                    n1835 = local write "AI update"(TRUE) -> ()
                    n1836 = global write "Global 1.vi" "RATE(Hz)"("RATE (Hz)") -> ()
                    n1837 = global write "Global 1.vi" "SAMPLES"("SAMPLES") -> ()
                    n1838 = Index Array(array=w2731, index=6) -> (element=→"LAB04-1 (GRAPH)":dynamicdata)
                    n1839 = Index Array(array=w2731, index=7) -> (element=→"LAB04-2 (GRAPH)":dynamicdata)
                    n1840 = Index Array(array=w2731, index=9) -> (element=→"LAB05-2 (GRAPH)":dynamicdata)
                    n1841 = Index Array(array=w2731, index=8) -> (element=→"LAB05-1 (GRAPH)":dynamicdata)
                    n1842 = Index Array(array=w2731, index=5) -> (element=→"LAB03-2 (GRAPH)":dynamicdata)
                    n1843 = Index Array(array=w2731, index=0) -> (element=→"LAB01-1 (GRAPH)":dynamicdata)
                    n1844 = Index Array(array=w2731, index=1) -> (element=→"LAB01-2 (GRAPH)":dynamicdata)
                    n1845 = Index Array(array=w2731, index=2) -> (element=→"LAB02-1 (GRAPH)":dynamicdata)
                    n1846 = Index Array(array=w2731, index=3) -> (element=→"LAB02-2 (GRAPH)":dynamicdata)
                    n1847 = Index Array(array=w2731, index=4) -> (element=→"LAB03-1 (GRAPH)":dynamicdata)
                    "AI loop time" <- w2732
                    "Analog Error Array" <- w2733
                  }
                  frame #1 {
                    n1848 = local read "CAL LAB01"() -> (w2777:T8)
                    n1849 = Unbundle By Name(w2778) -> ("LAB01-1 (A)"=w2776:dbl, "LAB01-1 (V)"=w2775:dbl, "LAB01-1 (PF)"=w2774:dbl, "LAB01-2 (A)"=w2773:dbl, "LAB01-2 (V)"=w2772:dbl, "LAB01-2 (PF)"=w2771:dbl)
                    n1850 = Unbundle By Name(w2777) -> ("1  (A) cal"=w2770:dbl, "1 (V) cal"=w2769:dbl, "1 (PF) cal"=w2768:dbl, "2 (A) cal"=w2767:dbl, "2 (V) cal"=w2766:dbl, "2 (PF) cal"=w2765:dbl)  [unwired: 4 out]
                    n1851 = Multiply(x=w2776, y=w2770) -> (x*y=w2763:dbl)
                    n1852 = Multiply(x=w2775, y=w2769) -> (x*y=w2762:dbl)
                    n1853 = Multiply(x=w2774, y=w2768) -> (x*y=w2761:dbl)
                    n1854 = Multiply(x=w2773, y=w2767) -> (x*y=w2757:dbl)
                    n1855 = Multiply(x=w2772, y=w2766) -> (x*y=w2756:dbl)
                    n1856 = Multiply(x=w2771, y=w2765) -> (x*y=w2755:dbl)
                    n1857 = local read "SIG LAB01-1"() -> (w2764:T2)
                    n1858 = local read "SIG LAB01-2"() -> (w2759:T2)
                    n1859 = Bundle By Name(cluster=w2764, "AMPS"=w2763, "VOLTS"=w2762, "PF"=w2761) -> (w2760:T2)
                    n1860 = Bundle By Name(cluster=w2759, "AMPS"=w2757, "VOLTS"=w2756, "PF"=w2755) -> (w2758:T2)
                    n1861 = local write "SIG LAB01-2"(w2758) -> ()
                    n1862 = local write "SIG LAB01-1"(w2760) -> ()
                  }
                  frame #2 {
                    n1863 = local read "CAL LAB02"() -> (w2802:T9)
                    n1864 = Unbundle By Name(w2779) -> ("LAB02-1 (A)"=w2801:dbl, "LAB02-1 (V)"=w2800:dbl, "LAB02-1 (PF)"=w2799:dbl, "LAB02-2 (A)"=w2798:dbl, "LAB02-2 (V)"=w2797:dbl, "LAB02-2 (PF)"=w2796:dbl)
                    n1865 = Unbundle By Name(w2802) -> ("1 (A) cal"=w2795:dbl, "1 (V) cal"=w2794:dbl, "1 (PF) cal"=w2793:dbl, "2 (A) cal"=w2792:dbl, "2 (V) cal"=w2791:dbl, "2 (PF) cal"=w2790:dbl)  [unwired: 4 out]
                    n1866 = Multiply(x=w2801, y=w2795) -> (x*y=w2788:dbl)
                    n1867 = Multiply(x=w2800, y=w2794) -> (x*y=w2787:dbl)
                    n1868 = Multiply(x=w2799, y=w2793) -> (x*y=w2786:dbl)
                    n1869 = Multiply(x=w2798, y=w2792) -> (x*y=w2782:dbl)
                    n1870 = Multiply(x=w2797, y=w2791) -> (x*y=w2781:dbl)
                    n1871 = Multiply(x=w2796, y=w2790) -> (x*y=w2780:dbl)
                    n1872 = local read "SIG LAB02-1"() -> (w2789:T2)
                    n1873 = local read "SIG LAB02-2"() -> (w2784:T2)
                    n1874 = Bundle By Name(cluster=w2789, "AMPS"=w2788, "VOLTS"=w2787, "PF"=w2786) -> (w2785:T2)
                    n1875 = Bundle By Name(cluster=w2784, "AMPS"=w2782, "VOLTS"=w2781, "PF"=w2780) -> (w2783:T2)
                    n1876 = local write "SIG LAB02-2"(w2783) -> ()
                    n1877 = local write "SIG LAB02-1"(w2785) -> ()
                  }
                  frame #3 {
                    n1878 = local read "CAL LAB03"() -> (w2826:T8)
                    n1879 = Unbundle By Name(w2804) -> ("LAB03-1 (A)"=w2825:dbl, "LAB03-1 (V)"=w2824:dbl, "LAB03-1 (PF)"=w2823:dbl, "LAB03-2 (A)"=w2822:dbl, "LAB03-2 (V)"=w2821:dbl, "LAB03-2 (PF)"=w2820:dbl)
                    n1880 = Unbundle By Name(w2826) -> ("1  (A) cal"=w2819:dbl, "1 (V) cal"=w2818:dbl, "1 (PF) cal"=w2817:dbl, "2 (A) cal"=w2816:dbl, "2 (V) cal"=w2815:dbl, "2 (PF) cal"=w2814:dbl)  [unwired: 4 out]
                    n1881 = Multiply(x=w2825, y=w2819) -> (x*y=w2812:dbl)
                    n1882 = Multiply(x=w2824, y=w2818) -> (x*y=w2803:dbl)
                    n1883 = Multiply(x=w2823, y=w2817) -> (x*y=w2811:dbl)
                    n1884 = Multiply(x=w2822, y=w2816) -> (x*y=w2807:dbl)
                    n1885 = Multiply(x=w2821, y=w2815) -> (x*y=w2806:dbl)
                    n1886 = Multiply(x=w2820, y=w2814) -> (x*y=w2805:dbl)
                    n1887 = local read "SIG LAB03-1"() -> (w2813:T2)
                    n1888 = local read "SIG LAB03-2"() -> (w2809:T2)
                    n1889 = Bundle By Name(cluster=w2813, "AMPS"=w2812, "VOLTS"=w2803, "PF"=w2811) -> (w2810:T2)
                    n1890 = Bundle By Name(cluster=w2809, "AMPS"=w2807, "VOLTS"=w2806, "PF"=w2805) -> (w2808:T2)
                    n1891 = local write "SIG LAB03-2"(w2808) -> ()
                    n1892 = local write "SIG LAB03-1"(w2810) -> ()
                  }
                  frame #4 {
                    n1893 = local read "CAL LAB04"() -> (w2850:T8)
                    n1894 = Unbundle By Name(w2827) -> ("LAB04-1 (A)"=w2849:dbl, "LAB04-1 (V)"=w2848:dbl, "LAB04-1 (PF)"=w2847:dbl, "LAB04-2 (A)"=w2846:dbl, "LAB04-2 (V)"=w2845:dbl, "LAB04-2 (PF)"=w2844:dbl)
                    n1895 = Unbundle By Name(w2850) -> ("1  (A) cal"=w2843:dbl, "1 (V) cal"=w2842:dbl, "1 (PF) cal"=w2841:dbl, "2 (A) cal"=w2840:dbl, "2 (V) cal"=w2839:dbl, "2 (PF) cal"=w2838:dbl)  [unwired: 4 out]
                    n1896 = Multiply(x=w2849, y=w2843) -> (x*y=w2836:dbl)
                    n1897 = Multiply(x=w2848, y=w2842) -> (x*y=w2835:dbl)
                    n1898 = Multiply(x=w2847, y=w2841) -> (x*y=w2834:dbl)
                    n1899 = Multiply(x=w2846, y=w2840) -> (x*y=w2830:dbl)
                    n1900 = Multiply(x=w2845, y=w2839) -> (x*y=w2829:dbl)
                    n1901 = Multiply(x=w2844, y=w2838) -> (x*y=w2828:dbl)
                    n1902 = local read "SIG LAB04-1"() -> (w2837:T2)
                    n1903 = local read "SIG LAB04-2"() -> (w2832:T2)
                    n1904 = Bundle By Name(cluster=w2837, "AMPS"=w2836, "VOLTS"=w2835, "PF"=w2834) -> (w2833:T2)
                    n1905 = Bundle By Name(cluster=w2832, "AMPS"=w2830, "VOLTS"=w2829, "PF"=w2828) -> (w2831:T2)
                    n1906 = local write "SIG LAB04-2"(w2831) -> ()
                    n1907 = local write "SIG LAB04-1"(w2833) -> ()
                  }
                  frame #5 {
                    n1908 = local read "CAL LAB05"() -> (w2874:T8)
                    n1909 = Unbundle By Name(w2852) -> ("LAB05-1 (A)"=w2873:dbl, "LAB05-1 (V)"=w2851:dbl, "LAB05-1 (PF)"=w2872:dbl, "LAB05-2 (A)"=w2871:dbl, "LAB05-2 (V)"=w2870:dbl, "LAB05-2 (PF)"=w2869:dbl)
                    n1910 = Unbundle By Name(w2874) -> ("1  (A) cal"=w2868:dbl, "1 (V) cal"=w2867:dbl, "1 (PF) cal"=w2866:dbl, "2 (A) cal"=w2865:dbl, "2 (V) cal"=w2864:dbl, "2 (PF) cal"=w2863:dbl)  [unwired: 4 out]
                    n1911 = Multiply(x=w2873, y=w2868) -> (x*y=w2861:dbl)
                    n1912 = Multiply(x=w2851, y=w2867) -> (x*y=w2860:dbl)
                    n1913 = Multiply(x=w2872, y=w2866) -> (x*y=w2859:dbl)
                    n1914 = Multiply(x=w2871, y=w2865) -> (x*y=w2855:dbl)
                    n1915 = Multiply(x=w2870, y=w2864) -> (x*y=w2854:dbl)
                    n1916 = Multiply(x=w2869, y=w2863) -> (x*y=w2853:dbl)
                    n1917 = local read "SIG LAB05-1"() -> (w2862:T2)
                    n1918 = local read "SIG LAB05-2"() -> (w2857:T2)
                    n1919 = Bundle By Name(cluster=w2862, "AMPS"=w2861, "VOLTS"=w2860, "PF"=w2859) -> (w2858:T2)
                    n1920 = Bundle By Name(cluster=w2857, "AMPS"=w2855, "VOLTS"=w2854, "PF"=w2853) -> (w2856:T2)
                    n1921 = local write "SIG LAB05-2"(w2856) -> ()
                    n1922 = local write "SIG LAB05-1"(w2858) -> ()
                  }
                }
              }
            }
          }
          frame #13 {
            # "save test data to file"
            n1923 = Get Date/Time In Seconds() -> (seconds since 1Jan1904=w2875:timestamp)
            "File Time Stamp" <- w2875
            n1924 = local read "on loops"() -> (w2894:dbl)
            n1925 = local read "jig cycle"() -> (w2891:dbl)
            n1926 = Format Date/Time String(time format string (%c)="%H:%M%:%S", seconds (now)=w2875) -> (date/time string=w2879:string)  [unwired: 1 in]
            n1927 = Add(x=w2894, y=2) -> (x+y=w2892:dbl)
            n1928 = Build Array(w2879) -> (w2878:string[])
            n1929 = Equal?(x=w2891, y=1) -> (x = y?=w2877:bool)
            n1930 = Equal?(x=w2891, y=w2892) -> (x = y?=w2876:bool)
            n1931 = stacked-sequence {
              tunnel: w2890 -> [w2900 _ _ _ _ _ _ _ _ _]
              tunnel: w2889 -> [_ w2976 _ _ _ _ _ _ _ _]
              tunnel: w2888 -> [_ _ w3056 _ _ _ _ _ _ _]
              tunnel: w2887 -> [_ _ _ w3136 _ _ _ _ _ _]
              tunnel: w2886 -> [_ _ _ _ w3216 _ _ _ _ _]
              tunnel: w2885 -> [_ _ _ _ _ w3296 _ _ _ _]
              tunnel: w2884 -> [_ _ _ _ _ _ w3376 _ _ _]
              tunnel: w2883 -> [_ _ _ _ _ _ _ w3456 _ _]
              tunnel: w2882 -> [_ _ _ _ _ _ _ _ w3536 _]
              tunnel: w2881 -> [_ _ _ _ _ _ _ _ _ w3616]
              tunnel: w2878 -> [w2899 w2980 w3060 w3140 w3220 w3300 w3380 w3460 w3540 w3620]
              tunnel: w2877 -> [w2898 w2979 w3059 w3139 w3219 w3299 w3379 w3459 w3539 w3619]
              tunnel: w2876 -> [w2897 w2978 w3058 w3138 w3218 w3298 w3378 w3458 w3538 w3618]
              tunnel: w2875 -> [w2896 w2977 w3057 w3137 w3217 w3297 w3377 w3457 w3537 w3617]
              frame #0 {
                n1932 = case shown="True" w2900 {
                  tunnel: w2899 -> [_ w2905]
                  tunnel: w2898 -> [_ w2904]
                  tunnel: w2897 -> [_ w2902]
                  tunnel: w2896 -> [_ w2901]
                  frame False {
                  }
                  frame True {
                    n1933 = local read "DISP LAB01-1"() -> (w2906:T4)
                    n1934 = local read "SIG LAB01-1"() -> (w2907:T2)
                    n1935 = local read "ON L01-1"() -> (w2903:cluster{"amps":dbl, "volts":dbl, "pf":dbl})
                    n1936 = Unbundle(w2907) -> ("AMPS"=w2913:dbl, "VOLTS"=w2911:dbl, "PF"=w2910:dbl, "Tmp Live"=w2909:dbl, "Tmp Neut"=w2912:dbl)
                    n1937 = Unbundle(w2906) -> ("CYCLE"=w2908:dbl)  [unwired: 2 out]
                    n1938 = stacked-sequence {
                      tunnel: w2913 -> [w2917 w2936]
                      tunnel: w2912 -> [_ w2935]
                      tunnel: w2911 -> [w2916 w2934]
                      tunnel: w2910 -> [w2915 w2933]
                      tunnel: w2909 -> [_ w2932]
                      tunnel: w2908 -> [_ w2931]
                      tunnel: w2905 -> [_ w2930]
                      tunnel: w2904 -> [w2918 _]
                      tunnel: w2903 -> [w2914 w2928]
                      tunnel: w2902 -> [_ w2929]
                      tunnel: w2901 -> [_ w2924]
                      frame #0 {
                        n1939 = case shown="True" w2918 {
                          tunnel: w2917 -> [_ w2923]
                          tunnel: w2916 -> [_ w2922]
                          tunnel: w2915 -> [_ w2921]
                          tunnel: w2914 -> [_ w2919]
                          frame False {
                          }
                          frame True {
                            n1940 = Bundle(cluster=w2919, "amps"=w2923, "volts"=w2922, "pf"=w2921) -> (w2920:cluster{"amps":dbl, "volts":dbl, "pf":dbl})
                            n1941 = local write "ON L01-1"(w2920) -> ()
                          }
                        }
                      }
                      frame #1 {
                        n1942 = Unbundle(w2928) -> ("amps"=w2927:dbl, "volts"=w2926:dbl, "pf"=w2925:dbl)
                        n1943 = case shown="True" w2929 {
                          tunnel: w2936 -> [_ w2937]
                          tunnel: w2935 -> [_ w2975]
                          tunnel: w2934 -> [_ _]
                          tunnel: w2933 -> [_ _]
                          tunnel: w2932 -> [_ w2974]
                          tunnel: w2931 -> [_ w2973]
                          tunnel: w2930 -> [_ w2941]
                          tunnel: w2927 -> [_ w2938]
                          tunnel: w2926 -> [_ w2970]
                          tunnel: w2925 -> [_ w2969]
                          tunnel: w2924 -> [_ w2939]
                          frame False {
                          }
                          frame True {
                            n1944 = local read "TDMS LAB01-1"() -> (w2972:refnum<k34>)
                            n1945 = Build Array(w2970) -> (w2966:dbl[])
                            n1946 = Build Array(w2969) -> (w2965:dbl[])
                            n1947 = Build Array(w2974) -> (w2964:dbl[])
                            n1948 = Build Array(w2975) -> (w2963:dbl[])
                            n1949 = Build Array(w2938) -> (w2968:dbl[])
                            n1950 = Build Array(w2937) -> (w2967:dbl[])
                            n1951 = Build Array(w2973) -> (w2962:dbl[])
                            n1952 = Build Array("AMPS ON", "AMPS OFF", "VOLTS", "PF", "TEMP Live", "TEMP Neut", "CYCLE") -> (w2946:string[])
                            n1953 = Bundle By Name("Y"=w2968, "t0"=w2939) -> (w2961:waveform(dbl))  [unwired: 1 in]
                            n1954 = Bundle By Name("Y"=w2967, "t0"=w2939) -> (w2960:waveform(dbl))  [unwired: 1 in]
                            n1955 = Bundle By Name("Y"=w2966, "t0"=w2939) -> (w2959:waveform(dbl))  [unwired: 1 in]
                            n1956 = Bundle By Name("Y"=w2965, "t0"=w2939) -> (w2958:waveform(dbl))  [unwired: 1 in]
                            n1957 = Bundle By Name("Y"=w2964, "t0"=w2939) -> (w2957:waveform(dbl))  [unwired: 1 in]
                            n1958 = Bundle By Name("Y"=w2963, "t0"=w2939) -> (w2956:waveform(dbl))  [unwired: 1 in]
                            n1959 = Bundle By Name("Y"=w2962, "t0"=w2939) -> (w2955:waveform(dbl))  [unwired: 1 in]
                            n1960 = Build Array(w2961, w2960, w2959, w2958, w2957, w2956, w2955) -> (w2954:waveform(dbl)[])
                            n1961 = TDMS Write(0:w2972, 5:"TEST VALUES", 7:w2946, 9:w2954) -> (4:w2945:refnum<k34>, 6:w2944:string, 15:w2943:errorcluster)  [unwired: 2 in, 1 out]
                            n1962 = TDMS Write(0:w2945, 5:w2944, 7:"TIME", 9:w2941, 11:w2943) -> (15:w2940:errorcluster)  [unwired: 1 in, 3 out]
                            n1963 = local write "data file error"(w2940) -> ()
                          }
                        }
                      }
                    }
                  }
                }
              }
              frame #1 {
                n1964 = case shown="True" w2976 {
                  tunnel: w2980 -> [_ w2985]
                  tunnel: w2979 -> [_ w2984]
                  tunnel: w2978 -> [_ w2982]
                  tunnel: w2977 -> [_ w2981]
                  frame False {
                  }
                  frame True {
                    n1965 = local read "DISP LAB01-2"() -> (w2986:T4)
                    n1966 = local read "SIG LAB01-2"() -> (w2987:T2)
                    n1967 = local read "ON L01-2"() -> (w2983:cluster{"amps":dbl, "volts":dbl, "pf":dbl})
                    n1968 = Unbundle(w2987) -> ("AMPS"=w2993:dbl, "VOLTS"=w2991:dbl, "PF"=w2990:dbl, "Tmp Live"=w2989:dbl, "Tmp Neut"=w2992:dbl)
                    n1969 = Unbundle(w2986) -> ("CYCLE"=w2988:dbl)  [unwired: 2 out]
                    n1970 = stacked-sequence {
                      tunnel: w2993 -> [w2997 w3016]
                      tunnel: w2992 -> [_ w3015]
                      tunnel: w2991 -> [w2996 w3014]
                      tunnel: w2990 -> [w2995 w3013]
                      tunnel: w2989 -> [_ w3012]
                      tunnel: w2988 -> [_ w3011]
                      tunnel: w2985 -> [_ w3010]
                      tunnel: w2984 -> [w2998 _]
                      tunnel: w2983 -> [w2994 w3008]
                      tunnel: w2982 -> [_ w3009]
                      tunnel: w2981 -> [_ w3004]
                      frame #0 {
                        n1971 = case shown="True" w2998 {
                          tunnel: w2997 -> [_ w3003]
                          tunnel: w2996 -> [_ w3002]
                          tunnel: w2995 -> [_ w3001]
                          tunnel: w2994 -> [_ w2999]
                          frame False {
                          }
                          frame True {
                            n1972 = Bundle(cluster=w2999, "amps"=w3003, "volts"=w3002, "pf"=w3001) -> (w3000:cluster{"amps":dbl, "volts":dbl, "pf":dbl})
                            n1973 = local write "ON L01-2"(w3000) -> ()
                          }
                        }
                      }
                      frame #1 {
                        n1974 = Unbundle(w3008) -> ("amps"=w3007:dbl, "volts"=w3006:dbl, "pf"=w3005:dbl)
                        n1975 = case shown="True" w3009 {
                          tunnel: w3016 -> [_ w3048]
                          tunnel: w3015 -> [_ w3055]
                          tunnel: w3014 -> [_ _]
                          tunnel: w3013 -> [_ _]
                          tunnel: w3012 -> [_ w3054]
                          tunnel: w3011 -> [_ w3053]
                          tunnel: w3010 -> [_ w3018]
                          tunnel: w3007 -> [_ w3050]
                          tunnel: w3006 -> [_ w3049]
                          tunnel: w3005 -> [_ w3047]
                          tunnel: w3004 -> [_ w3039]
                          frame False {
                          }
                          frame True {
                            n1976 = local read "TDMS LAB01-2"() -> (w3052:refnum<k34>)
                            n1977 = Build Array(w3049) -> (w3044:dbl[])
                            n1978 = Build Array(w3047) -> (w3043:dbl[])
                            n1979 = Build Array(w3054) -> (w3042:dbl[])
                            n1980 = Build Array(w3055) -> (w3041:dbl[])
                            n1981 = Build Array(w3050) -> (w3046:dbl[])
                            n1982 = Build Array(w3048) -> (w3045:dbl[])
                            n1983 = Build Array(w3053) -> (w3040:dbl[])
                            n1984 = Build Array("AMPS ON", "AMPS OFF", "VOLTS", "PF", "TEMP Live", "TEMP Neut", "CYCLE") -> (w3023:string[])
                            n1985 = Bundle By Name("Y"=w3046, "t0"=w3039) -> (w3038:waveform(dbl))  [unwired: 1 in]
                            n1986 = Bundle By Name("Y"=w3045, "t0"=w3039) -> (w3037:waveform(dbl))  [unwired: 1 in]
                            n1987 = Bundle By Name("Y"=w3044, "t0"=w3039) -> (w3036:waveform(dbl))  [unwired: 1 in]
                            n1988 = Bundle By Name("Y"=w3043, "t0"=w3039) -> (w3035:waveform(dbl))  [unwired: 1 in]
                            n1989 = Bundle By Name("Y"=w3042, "t0"=w3039) -> (w3034:waveform(dbl))  [unwired: 1 in]
                            n1990 = Bundle By Name("Y"=w3041, "t0"=w3039) -> (w3033:waveform(dbl))  [unwired: 1 in]
                            n1991 = Bundle By Name("Y"=w3040, "t0"=w3039) -> (w3032:waveform(dbl))  [unwired: 1 in]
                            n1992 = Build Array(w3038, w3037, w3036, w3035, w3034, w3033, w3032) -> (w3031:waveform(dbl)[])
                            n1993 = TDMS Write(0:w3052, 5:"TEST VALUES", 7:w3023, 9:w3031) -> (4:w3022:refnum<k34>, 6:w3021:string, 15:w3020:errorcluster)  [unwired: 2 in, 1 out]
                            n1994 = TDMS Write(0:w3022, 5:w3021, 7:"TIME", 9:w3018, 11:w3020) -> (15:w3017:errorcluster)  [unwired: 1 in, 3 out]
                            n1995 = local write "data file error"(w3017) -> ()
                          }
                        }
                      }
                    }
                  }
                }
              }
              frame #2 {
                n1996 = case shown="True" w3056 {
                  tunnel: w3060 -> [_ w3065]
                  tunnel: w3059 -> [_ w3064]
                  tunnel: w3058 -> [_ w3062]
                  tunnel: w3057 -> [_ w3061]
                  frame False {
                  }
                  frame True {
                    n1997 = local read "DISP LAB02-1"() -> (w3066:T4)
                    n1998 = local read "SIG LAB02-1"() -> (w3067:T2)
                    n1999 = local read "ON L02-1"() -> (w3063:cluster{"amps":dbl, "volts":dbl, "pf":dbl})
                    n2000 = Unbundle(w3067) -> ("AMPS"=w3073:dbl, "VOLTS"=w3071:dbl, "PF"=w3070:dbl, "Tmp Live"=w3069:dbl, "Tmp Neut"=w3072:dbl)
                    n2001 = Unbundle(w3066) -> ("CYCLE"=w3068:dbl)  [unwired: 2 out]
                    n2002 = stacked-sequence {
                      tunnel: w3073 -> [w3077 w3096]
                      tunnel: w3072 -> [_ w3095]
                      tunnel: w3071 -> [w3076 w3094]
                      tunnel: w3070 -> [w3075 w3093]
                      tunnel: w3069 -> [_ w3092]
                      tunnel: w3068 -> [_ w3091]
                      tunnel: w3065 -> [_ w3090]
                      tunnel: w3064 -> [w3078 _]
                      tunnel: w3063 -> [w3074 w3088]
                      tunnel: w3062 -> [_ w3089]
                      tunnel: w3061 -> [_ w3084]
                      frame #0 {
                        n2003 = case shown="True" w3078 {
                          tunnel: w3077 -> [_ w3083]
                          tunnel: w3076 -> [_ w3082]
                          tunnel: w3075 -> [_ w3081]
                          tunnel: w3074 -> [_ w3079]
                          frame False {
                          }
                          frame True {
                            n2004 = Bundle(cluster=w3079, "amps"=w3083, "volts"=w3082, "pf"=w3081) -> (w3080:cluster{"amps":dbl, "volts":dbl, "pf":dbl})
                            n2005 = local write "ON L02-1"(w3080) -> ()
                          }
                        }
                      }
                      frame #1 {
                        n2006 = Unbundle(w3088) -> ("amps"=w3087:dbl, "volts"=w3086:dbl, "pf"=w3085:dbl)
                        n2007 = case shown="True" w3089 {
                          tunnel: w3096 -> [_ w3128]
                          tunnel: w3095 -> [_ w3135]
                          tunnel: w3094 -> [_ _]
                          tunnel: w3093 -> [_ _]
                          tunnel: w3092 -> [_ w3134]
                          tunnel: w3091 -> [_ w3133]
                          tunnel: w3090 -> [_ w3098]
                          tunnel: w3087 -> [_ w3130]
                          tunnel: w3086 -> [_ w3129]
                          tunnel: w3085 -> [_ w3127]
                          tunnel: w3084 -> [_ w3119]
                          frame False {
                          }
                          frame True {
                            n2008 = local read "TDMS LAB02-1"() -> (w3132:refnum<k34>)
                            n2009 = Build Array(w3129) -> (w3124:dbl[])
                            n2010 = Build Array(w3127) -> (w3123:dbl[])
                            n2011 = Build Array(w3134) -> (w3122:dbl[])
                            n2012 = Build Array(w3135) -> (w3121:dbl[])
                            n2013 = Build Array(w3130) -> (w3126:dbl[])
                            n2014 = Build Array(w3128) -> (w3125:dbl[])
                            n2015 = Build Array(w3133) -> (w3120:dbl[])
                            n2016 = Build Array("AMPS ON", "AMPS OFF", "VOLTS", "PF", "TEMP Live", "TEMP Neut", "CYCLE") -> (w3103:string[])
                            n2017 = Bundle By Name("Y"=w3126, "t0"=w3119) -> (w3118:waveform(dbl))  [unwired: 1 in]
                            n2018 = Bundle By Name("Y"=w3125, "t0"=w3119) -> (w3117:waveform(dbl))  [unwired: 1 in]
                            n2019 = Bundle By Name("Y"=w3124, "t0"=w3119) -> (w3116:waveform(dbl))  [unwired: 1 in]
                            n2020 = Bundle By Name("Y"=w3123, "t0"=w3119) -> (w3115:waveform(dbl))  [unwired: 1 in]
                            n2021 = Bundle By Name("Y"=w3122, "t0"=w3119) -> (w3114:waveform(dbl))  [unwired: 1 in]
                            n2022 = Bundle By Name("Y"=w3121, "t0"=w3119) -> (w3113:waveform(dbl))  [unwired: 1 in]
                            n2023 = Bundle By Name("Y"=w3120, "t0"=w3119) -> (w3112:waveform(dbl))  [unwired: 1 in]
                            n2024 = Build Array(w3118, w3117, w3116, w3115, w3114, w3113, w3112) -> (w3111:waveform(dbl)[])
                            n2025 = TDMS Write(0:w3132, 5:"TEST VALUES", 7:w3103, 9:w3111) -> (4:w3102:refnum<k34>, 6:w3101:string, 15:w3100:errorcluster)  [unwired: 2 in, 1 out]
                            n2026 = TDMS Write(0:w3102, 5:w3101, 7:"TIME", 9:w3098, 11:w3100) -> (15:w3097:errorcluster)  [unwired: 1 in, 3 out]
                            n2027 = local write "data file error"(w3097) -> ()
                          }
                        }
                      }
                    }
                  }
                }
              }
              frame #3 {
                n2028 = case shown="True" w3136 {
                  tunnel: w3140 -> [_ w3145]
                  tunnel: w3139 -> [_ w3144]
                  tunnel: w3138 -> [_ w3142]
                  tunnel: w3137 -> [_ w3141]
                  frame False {
                  }
                  frame True {
                    n2029 = local read "DISP LAB02-2"() -> (w3146:T4)
                    n2030 = local read "SIG LAB02-2"() -> (w3147:T2)
                    n2031 = local read "ON L02-2"() -> (w3143:cluster{"amps":dbl, "volts":dbl, "pf":dbl})
                    n2032 = Unbundle(w3147) -> ("AMPS"=w3153:dbl, "VOLTS"=w3151:dbl, "PF"=w3150:dbl, "Tmp Live"=w3149:dbl, "Tmp Neut"=w3152:dbl)
                    n2033 = Unbundle(w3146) -> ("CYCLE"=w3148:dbl)  [unwired: 2 out]
                    n2034 = stacked-sequence {
                      tunnel: w3153 -> [w3157 w3176]
                      tunnel: w3152 -> [_ w3175]
                      tunnel: w3151 -> [w3156 w3174]
                      tunnel: w3150 -> [w3155 w3173]
                      tunnel: w3149 -> [_ w3172]
                      tunnel: w3148 -> [_ w3171]
                      tunnel: w3145 -> [_ w3170]
                      tunnel: w3144 -> [w3158 _]
                      tunnel: w3143 -> [w3154 w3168]
                      tunnel: w3142 -> [_ w3169]
                      tunnel: w3141 -> [_ w3164]
                      frame #0 {
                        n2035 = case shown="True" w3158 {
                          tunnel: w3157 -> [_ w3163]
                          tunnel: w3156 -> [_ w3162]
                          tunnel: w3155 -> [_ w3161]
                          tunnel: w3154 -> [_ w3159]
                          frame False {
                          }
                          frame True {
                            n2036 = Bundle(cluster=w3159, "amps"=w3163, "volts"=w3162, "pf"=w3161) -> (w3160:cluster{"amps":dbl, "volts":dbl, "pf":dbl})
                            n2037 = local write "ON L02-2"(w3160) -> ()
                          }
                        }
                      }
                      frame #1 {
                        n2038 = Unbundle(w3168) -> ("amps"=w3167:dbl, "volts"=w3166:dbl, "pf"=w3165:dbl)
                        n2039 = case shown="True" w3169 {
                          tunnel: w3176 -> [_ w3208]
                          tunnel: w3175 -> [_ w3215]
                          tunnel: w3174 -> [_ _]
                          tunnel: w3173 -> [_ _]
                          tunnel: w3172 -> [_ w3214]
                          tunnel: w3171 -> [_ w3213]
                          tunnel: w3170 -> [_ w3178]
                          tunnel: w3167 -> [_ w3210]
                          tunnel: w3166 -> [_ w3209]
                          tunnel: w3165 -> [_ w3207]
                          tunnel: w3164 -> [_ w3199]
                          frame False {
                          }
                          frame True {
                            n2040 = local read "TDMS LAB02-2"() -> (w3212:refnum<k34>)
                            n2041 = Build Array(w3209) -> (w3204:dbl[])
                            n2042 = Build Array(w3207) -> (w3203:dbl[])
                            n2043 = Build Array(w3214) -> (w3202:dbl[])
                            n2044 = Build Array(w3215) -> (w3201:dbl[])
                            n2045 = Build Array(w3210) -> (w3206:dbl[])
                            n2046 = Build Array(w3208) -> (w3205:dbl[])
                            n2047 = Build Array(w3213) -> (w3200:dbl[])
                            n2048 = Build Array("AMPS ON", "AMPS OFF", "VOLTS", "PF", "TEMP Live", "TEMP Neut", "CYCLE") -> (w3183:string[])
                            n2049 = Bundle By Name("Y"=w3206, "t0"=w3199) -> (w3198:waveform(dbl))  [unwired: 1 in]
                            n2050 = Bundle By Name("Y"=w3205, "t0"=w3199) -> (w3197:waveform(dbl))  [unwired: 1 in]
                            n2051 = Bundle By Name("Y"=w3204, "t0"=w3199) -> (w3196:waveform(dbl))  [unwired: 1 in]
                            n2052 = Bundle By Name("Y"=w3203, "t0"=w3199) -> (w3195:waveform(dbl))  [unwired: 1 in]
                            n2053 = Bundle By Name("Y"=w3202, "t0"=w3199) -> (w3194:waveform(dbl))  [unwired: 1 in]
                            n2054 = Bundle By Name("Y"=w3201, "t0"=w3199) -> (w3193:waveform(dbl))  [unwired: 1 in]
                            n2055 = Bundle By Name("Y"=w3200, "t0"=w3199) -> (w3192:waveform(dbl))  [unwired: 1 in]
                            n2056 = Build Array(w3198, w3197, w3196, w3195, w3194, w3193, w3192) -> (w3191:waveform(dbl)[])
                            n2057 = TDMS Write(0:w3212, 5:"TEST VALUES", 7:w3183, 9:w3191) -> (4:w3182:refnum<k34>, 6:w3181:string, 15:w3180:errorcluster)  [unwired: 2 in, 1 out]
                            n2058 = TDMS Write(0:w3182, 5:w3181, 7:"TIME", 9:w3178, 11:w3180) -> (15:w3177:errorcluster)  [unwired: 1 in, 3 out]
                            n2059 = local write "data file error"(w3177) -> ()
                          }
                        }
                      }
                    }
                  }
                }
              }
              frame #4 {
                n2060 = case shown="True" w3216 {
                  tunnel: w3220 -> [_ w3225]
                  tunnel: w3219 -> [_ w3224]
                  tunnel: w3218 -> [_ w3222]
                  tunnel: w3217 -> [_ w3221]
                  frame False {
                  }
                  frame True {
                    n2061 = local read "DISP LAB03-1"() -> (w3226:T4)
                    n2062 = local read "SIG LAB03-1"() -> (w3227:T2)
                    n2063 = local read "ON L03-1"() -> (w3223:cluster{"amps":dbl, "volts":dbl, "pf":dbl})
                    n2064 = Unbundle(w3227) -> ("AMPS"=w3233:dbl, "VOLTS"=w3231:dbl, "PF"=w3230:dbl, "Tmp Live"=w3229:dbl, "Tmp Neut"=w3232:dbl)
                    n2065 = Unbundle(w3226) -> ("CYCLE"=w3228:dbl)  [unwired: 2 out]
                    n2066 = stacked-sequence {
                      tunnel: w3233 -> [w3237 w3256]
                      tunnel: w3232 -> [_ w3255]
                      tunnel: w3231 -> [w3236 w3254]
                      tunnel: w3230 -> [w3235 w3253]
                      tunnel: w3229 -> [_ w3252]
                      tunnel: w3228 -> [_ w3251]
                      tunnel: w3225 -> [_ w3250]
                      tunnel: w3224 -> [w3238 _]
                      tunnel: w3223 -> [w3234 w3248]
                      tunnel: w3222 -> [_ w3249]
                      tunnel: w3221 -> [_ w3244]
                      frame #0 {
                        n2067 = case shown="True" w3238 {
                          tunnel: w3237 -> [_ w3243]
                          tunnel: w3236 -> [_ w3242]
                          tunnel: w3235 -> [_ w3241]
                          tunnel: w3234 -> [_ w3239]
                          frame False {
                          }
                          frame True {
                            n2068 = Bundle(cluster=w3239, "amps"=w3243, "volts"=w3242, "pf"=w3241) -> (w3240:cluster{"amps":dbl, "volts":dbl, "pf":dbl})
                            n2069 = local write "ON L03-1"(w3240) -> ()
                          }
                        }
                      }
                      frame #1 {
                        n2070 = Unbundle(w3248) -> ("amps"=w3247:dbl, "volts"=w3246:dbl, "pf"=w3245:dbl)
                        n2071 = case shown="True" w3249 {
                          tunnel: w3256 -> [_ w3288]
                          tunnel: w3255 -> [_ w3295]
                          tunnel: w3254 -> [_ _]
                          tunnel: w3253 -> [_ _]
                          tunnel: w3252 -> [_ w3294]
                          tunnel: w3251 -> [_ w3293]
                          tunnel: w3250 -> [_ w3258]
                          tunnel: w3247 -> [_ w3290]
                          tunnel: w3246 -> [_ w3289]
                          tunnel: w3245 -> [_ w3287]
                          tunnel: w3244 -> [_ w3279]
                          frame False {
                          }
                          frame True {
                            n2072 = local read "TDMS LAB03-1"() -> (w3292:refnum<k34>)
                            n2073 = Build Array(w3289) -> (w3284:dbl[])
                            n2074 = Build Array(w3287) -> (w3283:dbl[])
                            n2075 = Build Array(w3294) -> (w3282:dbl[])
                            n2076 = Build Array(w3295) -> (w3281:dbl[])
                            n2077 = Build Array(w3290) -> (w3286:dbl[])
                            n2078 = Build Array(w3288) -> (w3285:dbl[])
                            n2079 = Build Array(w3293) -> (w3280:dbl[])
                            n2080 = Build Array("AMPS ON", "AMPS OFF", "VOLTS", "PF", "TEMP Live", "TEMP Neut", "CYCLE") -> (w3263:string[])
                            n2081 = Bundle By Name("Y"=w3286, "t0"=w3279) -> (w3278:waveform(dbl))  [unwired: 1 in]
                            n2082 = Bundle By Name("Y"=w3285, "t0"=w3279) -> (w3277:waveform(dbl))  [unwired: 1 in]
                            n2083 = Bundle By Name("Y"=w3284, "t0"=w3279) -> (w3276:waveform(dbl))  [unwired: 1 in]
                            n2084 = Bundle By Name("Y"=w3283, "t0"=w3279) -> (w3275:waveform(dbl))  [unwired: 1 in]
                            n2085 = Bundle By Name("Y"=w3282, "t0"=w3279) -> (w3274:waveform(dbl))  [unwired: 1 in]
                            n2086 = Bundle By Name("Y"=w3281, "t0"=w3279) -> (w3273:waveform(dbl))  [unwired: 1 in]
                            n2087 = Bundle By Name("Y"=w3280, "t0"=w3279) -> (w3272:waveform(dbl))  [unwired: 1 in]
                            n2088 = Build Array(w3278, w3277, w3276, w3275, w3274, w3273, w3272) -> (w3271:waveform(dbl)[])
                            n2089 = TDMS Write(0:w3292, 5:"TEST VALUES", 7:w3263, 9:w3271) -> (4:w3262:refnum<k34>, 6:w3261:string, 15:w3260:errorcluster)  [unwired: 2 in, 1 out]
                            n2090 = TDMS Write(0:w3262, 5:w3261, 7:"TIME", 9:w3258, 11:w3260) -> (15:w3257:errorcluster)  [unwired: 1 in, 3 out]
                            n2091 = local write "data file error"(w3257) -> ()
                          }
                        }
                      }
                    }
                  }
                }
              }
              frame #5 {
                n2092 = case shown="True" w3296 {
                  tunnel: w3300 -> [_ w3305]
                  tunnel: w3299 -> [_ w3304]
                  tunnel: w3298 -> [_ w3302]
                  tunnel: w3297 -> [_ w3301]
                  frame False {
                  }
                  frame True {
                    n2093 = local read "DISP LAB03-2"() -> (w3306:T4)
                    n2094 = local read "SIG LAB03-2"() -> (w3307:T2)
                    n2095 = local read "ON L03-2"() -> (w3303:cluster{"amps":dbl, "volts":dbl, "pf":dbl})
                    n2096 = Unbundle(w3307) -> ("AMPS"=w3313:dbl, "VOLTS"=w3311:dbl, "PF"=w3310:dbl, "Tmp Live"=w3309:dbl, "Tmp Neut"=w3312:dbl)
                    n2097 = Unbundle(w3306) -> ("CYCLE"=w3308:dbl)  [unwired: 2 out]
                    n2098 = stacked-sequence {
                      tunnel: w3313 -> [w3317 w3336]
                      tunnel: w3312 -> [_ w3335]
                      tunnel: w3311 -> [w3316 w3334]
                      tunnel: w3310 -> [w3315 w3333]
                      tunnel: w3309 -> [_ w3332]
                      tunnel: w3308 -> [_ w3331]
                      tunnel: w3305 -> [_ w3330]
                      tunnel: w3304 -> [w3318 _]
                      tunnel: w3303 -> [w3314 w3328]
                      tunnel: w3302 -> [_ w3329]
                      tunnel: w3301 -> [_ w3324]
                      frame #0 {
                        n2099 = case shown="True" w3318 {
                          tunnel: w3317 -> [_ w3323]
                          tunnel: w3316 -> [_ w3322]
                          tunnel: w3315 -> [_ w3321]
                          tunnel: w3314 -> [_ w3319]
                          frame False {
                          }
                          frame True {
                            n2100 = Bundle(cluster=w3319, "amps"=w3323, "volts"=w3322, "pf"=w3321) -> (w3320:cluster{"amps":dbl, "volts":dbl, "pf":dbl})
                            n2101 = local write "ON L03-2"(w3320) -> ()
                          }
                        }
                      }
                      frame #1 {
                        n2102 = Unbundle(w3328) -> ("amps"=w3327:dbl, "volts"=w3326:dbl, "pf"=w3325:dbl)
                        n2103 = case shown="True" w3329 {
                          tunnel: w3336 -> [_ w3368]
                          tunnel: w3335 -> [_ w3375]
                          tunnel: w3334 -> [_ _]
                          tunnel: w3333 -> [_ _]
                          tunnel: w3332 -> [_ w3374]
                          tunnel: w3331 -> [_ w3373]
                          tunnel: w3330 -> [_ w3338]
                          tunnel: w3327 -> [_ w3370]
                          tunnel: w3326 -> [_ w3369]
                          tunnel: w3325 -> [_ w3367]
                          tunnel: w3324 -> [_ w3359]
                          frame False {
                          }
                          frame True {
                            n2104 = local read "TDMS LAB03-2"() -> (w3372:refnum<k34>)
                            n2105 = Build Array(w3369) -> (w3364:dbl[])
                            n2106 = Build Array(w3367) -> (w3363:dbl[])
                            n2107 = Build Array(w3374) -> (w3362:dbl[])
                            n2108 = Build Array(w3375) -> (w3361:dbl[])
                            n2109 = Build Array(w3370) -> (w3366:dbl[])
                            n2110 = Build Array(w3368) -> (w3365:dbl[])
                            n2111 = Build Array(w3373) -> (w3360:dbl[])
                            n2112 = Build Array("AMPS ON", "AMPS OFF", "VOLTS", "PF", "TEMP Live", "TEMP Neut", "CYCLE") -> (w3343:string[])
                            n2113 = Bundle By Name("Y"=w3366, "t0"=w3359) -> (w3358:waveform(dbl))  [unwired: 1 in]
                            n2114 = Bundle By Name("Y"=w3365, "t0"=w3359) -> (w3357:waveform(dbl))  [unwired: 1 in]
                            n2115 = Bundle By Name("Y"=w3364, "t0"=w3359) -> (w3356:waveform(dbl))  [unwired: 1 in]
                            n2116 = Bundle By Name("Y"=w3363, "t0"=w3359) -> (w3355:waveform(dbl))  [unwired: 1 in]
                            n2117 = Bundle By Name("Y"=w3362, "t0"=w3359) -> (w3354:waveform(dbl))  [unwired: 1 in]
                            n2118 = Bundle By Name("Y"=w3361, "t0"=w3359) -> (w3353:waveform(dbl))  [unwired: 1 in]
                            n2119 = Bundle By Name("Y"=w3360, "t0"=w3359) -> (w3352:waveform(dbl))  [unwired: 1 in]
                            n2120 = Build Array(w3358, w3357, w3356, w3355, w3354, w3353, w3352) -> (w3351:waveform(dbl)[])
                            n2121 = TDMS Write(0:w3372, 5:"TEST VALUES", 7:w3343, 9:w3351) -> (4:w3342:refnum<k34>, 6:w3341:string, 15:w3340:errorcluster)  [unwired: 2 in, 1 out]
                            n2122 = TDMS Write(0:w3342, 5:w3341, 7:"TIME", 9:w3338, 11:w3340) -> (15:w3337:errorcluster)  [unwired: 1 in, 3 out]
                            n2123 = local write "data file error"(w3337) -> ()
                          }
                        }
                      }
                    }
                  }
                }
              }
              frame #6 {
                n2124 = case shown="True" w3376 {
                  tunnel: w3380 -> [_ w3385]
                  tunnel: w3379 -> [_ w3384]
                  tunnel: w3378 -> [_ w3382]
                  tunnel: w3377 -> [_ w3381]
                  frame False {
                  }
                  frame True {
                    n2125 = local read "DISP LAB04-1"() -> (w3386:T4)
                    n2126 = local read "SIG LAB04-1"() -> (w3387:T2)
                    n2127 = local read "ON L04-1"() -> (w3383:cluster{"amps":dbl, "volts":dbl, "pf":dbl})
                    n2128 = Unbundle(w3387) -> ("AMPS"=w3393:dbl, "VOLTS"=w3391:dbl, "PF"=w3390:dbl, "Tmp Live"=w3389:dbl, "Tmp Neut"=w3392:dbl)
                    n2129 = Unbundle(w3386) -> ("CYCLE"=w3388:dbl)  [unwired: 2 out]
                    n2130 = stacked-sequence {
                      tunnel: w3393 -> [w3397 w3416]
                      tunnel: w3392 -> [_ w3415]
                      tunnel: w3391 -> [w3396 w3414]
                      tunnel: w3390 -> [w3395 w3413]
                      tunnel: w3389 -> [_ w3412]
                      tunnel: w3388 -> [_ w3411]
                      tunnel: w3385 -> [_ w3410]
                      tunnel: w3384 -> [w3398 _]
                      tunnel: w3383 -> [w3394 w3408]
                      tunnel: w3382 -> [_ w3409]
                      tunnel: w3381 -> [_ w3404]
                      frame #0 {
                        n2131 = case shown="True" w3398 {
                          tunnel: w3397 -> [_ w3403]
                          tunnel: w3396 -> [_ w3402]
                          tunnel: w3395 -> [_ w3401]
                          tunnel: w3394 -> [_ w3399]
                          frame False {
                          }
                          frame True {
                            n2132 = Bundle(cluster=w3399, "amps"=w3403, "volts"=w3402, "pf"=w3401) -> (w3400:cluster{"amps":dbl, "volts":dbl, "pf":dbl})
                            n2133 = local write "ON L04-1"(w3400) -> ()
                          }
                        }
                      }
                      frame #1 {
                        n2134 = Unbundle(w3408) -> ("amps"=w3407:dbl, "volts"=w3406:dbl, "pf"=w3405:dbl)
                        n2135 = case shown="True" w3409 {
                          tunnel: w3416 -> [_ w3448]
                          tunnel: w3415 -> [_ w3455]
                          tunnel: w3414 -> [_ _]
                          tunnel: w3413 -> [_ _]
                          tunnel: w3412 -> [_ w3454]
                          tunnel: w3411 -> [_ w3453]
                          tunnel: w3410 -> [_ w3418]
                          tunnel: w3407 -> [_ w3450]
                          tunnel: w3406 -> [_ w3449]
                          tunnel: w3405 -> [_ w3447]
                          tunnel: w3404 -> [_ w3439]
                          frame False {
                          }
                          frame True {
                            n2136 = local read "TDMS LAB04-1"() -> (w3452:refnum<k34>)
                            n2137 = Build Array(w3449) -> (w3444:dbl[])
                            n2138 = Build Array(w3447) -> (w3443:dbl[])
                            n2139 = Build Array(w3454) -> (w3442:dbl[])
                            n2140 = Build Array(w3455) -> (w3441:dbl[])
                            n2141 = Build Array(w3450) -> (w3446:dbl[])
                            n2142 = Build Array(w3448) -> (w3445:dbl[])
                            n2143 = Build Array(w3453) -> (w3440:dbl[])
                            n2144 = Build Array("AMPS ON", "AMPS OFF", "VOLTS", "PF", "TEMP Live", "TEMP Neut", "CYCLE") -> (w3423:string[])
                            n2145 = Bundle By Name("Y"=w3446, "t0"=w3439) -> (w3438:waveform(dbl))  [unwired: 1 in]
                            n2146 = Bundle By Name("Y"=w3445, "t0"=w3439) -> (w3437:waveform(dbl))  [unwired: 1 in]
                            n2147 = Bundle By Name("Y"=w3444, "t0"=w3439) -> (w3436:waveform(dbl))  [unwired: 1 in]
                            n2148 = Bundle By Name("Y"=w3443, "t0"=w3439) -> (w3435:waveform(dbl))  [unwired: 1 in]
                            n2149 = Bundle By Name("Y"=w3442, "t0"=w3439) -> (w3434:waveform(dbl))  [unwired: 1 in]
                            n2150 = Bundle By Name("Y"=w3441, "t0"=w3439) -> (w3433:waveform(dbl))  [unwired: 1 in]
                            n2151 = Bundle By Name("Y"=w3440, "t0"=w3439) -> (w3432:waveform(dbl))  [unwired: 1 in]
                            n2152 = Build Array(w3438, w3437, w3436, w3435, w3434, w3433, w3432) -> (w3431:waveform(dbl)[])
                            n2153 = TDMS Write(0:w3452, 5:"TEST VALUES", 7:w3423, 9:w3431) -> (4:w3422:refnum<k34>, 6:w3421:string, 15:w3420:errorcluster)  [unwired: 2 in, 1 out]
                            n2154 = TDMS Write(0:w3422, 5:w3421, 7:"TIME", 9:w3418, 11:w3420) -> (15:w3417:errorcluster)  [unwired: 1 in, 3 out]
                            n2155 = local write "data file error"(w3417) -> ()
                          }
                        }
                      }
                    }
                  }
                }
              }
              frame #7 {
                n2156 = case shown="True" w3456 {
                  tunnel: w3460 -> [_ w3465]
                  tunnel: w3459 -> [_ w3464]
                  tunnel: w3458 -> [_ w3462]
                  tunnel: w3457 -> [_ w3461]
                  frame False {
                  }
                  frame True {
                    n2157 = local read "DISP LAB04-2"() -> (w3466:T4)
                    n2158 = local read "SIG LAB04-2"() -> (w3467:T2)
                    n2159 = local read "ON L04-2"() -> (w3463:cluster{"amps":dbl, "volts":dbl, "pf":dbl})
                    n2160 = Unbundle(w3467) -> ("AMPS"=w3473:dbl, "VOLTS"=w3471:dbl, "PF"=w3470:dbl, "Tmp Live"=w3469:dbl, "Tmp Neut"=w3472:dbl)
                    n2161 = Unbundle(w3466) -> ("CYCLE"=w3468:dbl)  [unwired: 2 out]
                    n2162 = stacked-sequence {
                      tunnel: w3473 -> [w3477 w3496]
                      tunnel: w3472 -> [_ w3495]
                      tunnel: w3471 -> [w3476 w3494]
                      tunnel: w3470 -> [w3475 w3493]
                      tunnel: w3469 -> [_ w3492]
                      tunnel: w3468 -> [_ w3491]
                      tunnel: w3465 -> [_ w3490]
                      tunnel: w3464 -> [w3478 _]
                      tunnel: w3463 -> [w3474 w3488]
                      tunnel: w3462 -> [_ w3489]
                      tunnel: w3461 -> [_ w3484]
                      frame #0 {
                        n2163 = case shown="True" w3478 {
                          tunnel: w3477 -> [_ w3483]
                          tunnel: w3476 -> [_ w3482]
                          tunnel: w3475 -> [_ w3481]
                          tunnel: w3474 -> [_ w3479]
                          frame False {
                          }
                          frame True {
                            n2164 = Bundle(cluster=w3479, "amps"=w3483, "volts"=w3482, "pf"=w3481) -> (w3480:cluster{"amps":dbl, "volts":dbl, "pf":dbl})
                            n2165 = local write "ON L04-2"(w3480) -> ()
                          }
                        }
                      }
                      frame #1 {
                        n2166 = Unbundle(w3488) -> ("amps"=w3487:dbl, "volts"=w3486:dbl, "pf"=w3485:dbl)
                        n2167 = case shown="True" w3489 {
                          tunnel: w3496 -> [_ w3528]
                          tunnel: w3495 -> [_ w3535]
                          tunnel: w3494 -> [_ _]
                          tunnel: w3493 -> [_ _]
                          tunnel: w3492 -> [_ w3534]
                          tunnel: w3491 -> [_ w3533]
                          tunnel: w3490 -> [_ w3498]
                          tunnel: w3487 -> [_ w3530]
                          tunnel: w3486 -> [_ w3529]
                          tunnel: w3485 -> [_ w3527]
                          tunnel: w3484 -> [_ w3519]
                          frame False {
                          }
                          frame True {
                            n2168 = local read "TDMS LAB04-2"() -> (w3532:refnum<k34>)
                            n2169 = Build Array(w3529) -> (w3524:dbl[])
                            n2170 = Build Array(w3527) -> (w3523:dbl[])
                            n2171 = Build Array(w3534) -> (w3522:dbl[])
                            n2172 = Build Array(w3535) -> (w3521:dbl[])
                            n2173 = Build Array(w3530) -> (w3526:dbl[])
                            n2174 = Build Array(w3528) -> (w3525:dbl[])
                            n2175 = Build Array(w3533) -> (w3520:dbl[])
                            n2176 = Build Array("AMPS ON", "AMPS OFF", "VOLTS", "PF", "TEMP Live", "TEMP Neut", "CYCLE") -> (w3503:string[])
                            n2177 = Bundle By Name("Y"=w3526, "t0"=w3519) -> (w3518:waveform(dbl))  [unwired: 1 in]
                            n2178 = Bundle By Name("Y"=w3525, "t0"=w3519) -> (w3517:waveform(dbl))  [unwired: 1 in]
                            n2179 = Bundle By Name("Y"=w3524, "t0"=w3519) -> (w3516:waveform(dbl))  [unwired: 1 in]
                            n2180 = Bundle By Name("Y"=w3523, "t0"=w3519) -> (w3515:waveform(dbl))  [unwired: 1 in]
                            n2181 = Bundle By Name("Y"=w3522, "t0"=w3519) -> (w3514:waveform(dbl))  [unwired: 1 in]
                            n2182 = Bundle By Name("Y"=w3521, "t0"=w3519) -> (w3513:waveform(dbl))  [unwired: 1 in]
                            n2183 = Bundle By Name("Y"=w3520, "t0"=w3519) -> (w3512:waveform(dbl))  [unwired: 1 in]
                            n2184 = Build Array(w3518, w3517, w3516, w3515, w3514, w3513, w3512) -> (w3511:waveform(dbl)[])
                            n2185 = TDMS Write(0:w3532, 5:"TEST VALUES", 7:w3503, 9:w3511) -> (4:w3502:refnum<k34>, 6:w3501:string, 15:w3500:errorcluster)  [unwired: 2 in, 1 out]
                            n2186 = TDMS Write(0:w3502, 5:w3501, 7:"TIME", 9:w3498, 11:w3500) -> (15:w3497:errorcluster)  [unwired: 1 in, 3 out]
                            n2187 = local write "data file error"(w3497) -> ()
                          }
                        }
                      }
                    }
                  }
                }
              }
              frame #8 {
                n2188 = case shown="True" w3536 {
                  tunnel: w3540 -> [_ w3545]
                  tunnel: w3539 -> [_ w3544]
                  tunnel: w3538 -> [_ w3542]
                  tunnel: w3537 -> [_ w3541]
                  frame False {
                  }
                  frame True {
                    n2189 = local read "DISP LAB05-1"() -> (w3546:T4)
                    n2190 = local read "SIG LAB05-1"() -> (w3547:T2)
                    n2191 = local read "ON L05-1"() -> (w3543:cluster{"amps":dbl, "volts":dbl, "pf":dbl})
                    n2192 = Unbundle(w3547) -> ("AMPS"=w3553:dbl, "VOLTS"=w3551:dbl, "PF"=w3550:dbl, "Tmp Live"=w3549:dbl, "Tmp Neut"=w3552:dbl)
                    n2193 = Unbundle(w3546) -> ("CYCLE"=w3548:dbl)  [unwired: 2 out]
                    n2194 = stacked-sequence {
                      tunnel: w3553 -> [w3557 w3576]
                      tunnel: w3552 -> [_ w3575]
                      tunnel: w3551 -> [w3556 w3574]
                      tunnel: w3550 -> [w3555 w3573]
                      tunnel: w3549 -> [_ w3572]
                      tunnel: w3548 -> [_ w3571]
                      tunnel: w3545 -> [_ w3570]
                      tunnel: w3544 -> [w3558 _]
                      tunnel: w3543 -> [w3554 w3568]
                      tunnel: w3542 -> [_ w3569]
                      tunnel: w3541 -> [_ w3564]
                      frame #0 {
                        n2195 = case shown="True" w3558 {
                          tunnel: w3557 -> [_ w3563]
                          tunnel: w3556 -> [_ w3562]
                          tunnel: w3555 -> [_ w3561]
                          tunnel: w3554 -> [_ w3559]
                          frame False {
                          }
                          frame True {
                            n2196 = Bundle(cluster=w3559, "amps"=w3563, "volts"=w3562, "pf"=w3561) -> (w3560:cluster{"amps":dbl, "volts":dbl, "pf":dbl})
                            n2197 = local write "ON L05-1"(w3560) -> ()
                          }
                        }
                      }
                      frame #1 {
                        n2198 = Unbundle(w3568) -> ("amps"=w3567:dbl, "volts"=w3566:dbl, "pf"=w3565:dbl)
                        n2199 = case shown="True" w3569 {
                          tunnel: w3576 -> [_ w3608]
                          tunnel: w3575 -> [_ w3615]
                          tunnel: w3574 -> [_ _]
                          tunnel: w3573 -> [_ _]
                          tunnel: w3572 -> [_ w3614]
                          tunnel: w3571 -> [_ w3613]
                          tunnel: w3570 -> [_ w3578]
                          tunnel: w3567 -> [_ w3610]
                          tunnel: w3566 -> [_ w3609]
                          tunnel: w3565 -> [_ w3607]
                          tunnel: w3564 -> [_ w3599]
                          frame False {
                          }
                          frame True {
                            n2200 = local read "TDMS LAB05-1"() -> (w3612:refnum<k34>)
                            n2201 = Build Array(w3609) -> (w3604:dbl[])
                            n2202 = Build Array(w3607) -> (w3603:dbl[])
                            n2203 = Build Array(w3614) -> (w3602:dbl[])
                            n2204 = Build Array(w3615) -> (w3601:dbl[])
                            n2205 = Build Array(w3610) -> (w3606:dbl[])
                            n2206 = Build Array(w3608) -> (w3605:dbl[])
                            n2207 = Build Array(w3613) -> (w3600:dbl[])
                            n2208 = Build Array("AMPS ON", "AMPS OFF", "VOLTS", "PF", "TEMP Live", "TEMP Neut", "CYCLE") -> (w3583:string[])
                            n2209 = Bundle By Name("Y"=w3606, "t0"=w3599) -> (w3598:waveform(dbl))  [unwired: 1 in]
                            n2210 = Bundle By Name("Y"=w3605, "t0"=w3599) -> (w3597:waveform(dbl))  [unwired: 1 in]
                            n2211 = Bundle By Name("Y"=w3604, "t0"=w3599) -> (w3596:waveform(dbl))  [unwired: 1 in]
                            n2212 = Bundle By Name("Y"=w3603, "t0"=w3599) -> (w3595:waveform(dbl))  [unwired: 1 in]
                            n2213 = Bundle By Name("Y"=w3602, "t0"=w3599) -> (w3594:waveform(dbl))  [unwired: 1 in]
                            n2214 = Bundle By Name("Y"=w3601, "t0"=w3599) -> (w3593:waveform(dbl))  [unwired: 1 in]
                            n2215 = Bundle By Name("Y"=w3600, "t0"=w3599) -> (w3592:waveform(dbl))  [unwired: 1 in]
                            n2216 = Build Array(w3598, w3597, w3596, w3595, w3594, w3593, w3592) -> (w3591:waveform(dbl)[])
                            n2217 = TDMS Write(0:w3612, 5:"TEST VALUES", 7:w3583, 9:w3591) -> (4:w3582:refnum<k34>, 6:w3581:string, 15:w3580:errorcluster)  [unwired: 2 in, 1 out]
                            n2218 = TDMS Write(0:w3582, 5:w3581, 7:"TIME", 9:w3578, 11:w3580) -> (15:w3577:errorcluster)  [unwired: 1 in, 3 out]
                            n2219 = local write "data file error"(w3577) -> ()
                          }
                        }
                      }
                    }
                  }
                }
              }
              frame #9 {
                n2220 = case shown="True" w3616 {
                  tunnel: w3620 -> [_ w3625]
                  tunnel: w3619 -> [_ w3624]
                  tunnel: w3618 -> [_ w3622]
                  tunnel: w3617 -> [_ w3621]
                  frame False {
                  }
                  frame True {
                    n2221 = local read "DISP LAB05-2"() -> (w3626:T4)
                    n2222 = local read "SIG LAB05-2"() -> (w3627:T2)
                    n2223 = local read "ON L05-2"() -> (w3623:cluster{"amps":dbl, "volts":dbl, "pf":dbl})
                    n2224 = Unbundle(w3627) -> ("AMPS"=w3633:dbl, "VOLTS"=w3631:dbl, "PF"=w3630:dbl, "Tmp Live"=w3629:dbl, "Tmp Neut"=w3632:dbl)
                    n2225 = Unbundle(w3626) -> ("CYCLE"=w3628:dbl)  [unwired: 2 out]
                    n2226 = stacked-sequence {
                      tunnel: w3633 -> [w3637 w3656]
                      tunnel: w3632 -> [_ w3655]
                      tunnel: w3631 -> [w3636 w3654]
                      tunnel: w3630 -> [w3635 w3653]
                      tunnel: w3629 -> [_ w3652]
                      tunnel: w3628 -> [_ w3651]
                      tunnel: w3625 -> [_ w3650]
                      tunnel: w3624 -> [w3638 _]
                      tunnel: w3623 -> [w3634 w3648]
                      tunnel: w3622 -> [_ w3649]
                      tunnel: w3621 -> [_ w3644]
                      frame #0 {
                        n2227 = case shown="True" w3638 {
                          tunnel: w3637 -> [_ w3643]
                          tunnel: w3636 -> [_ w3642]
                          tunnel: w3635 -> [_ w3641]
                          tunnel: w3634 -> [_ w3639]
                          frame False {
                          }
                          frame True {
                            n2228 = Bundle(cluster=w3639, "amps"=w3643, "volts"=w3642, "pf"=w3641) -> (w3640:cluster{"amps":dbl, "volts":dbl, "pf":dbl})
                            n2229 = local write "ON L05-2"(w3640) -> ()
                          }
                        }
                      }
                      frame #1 {
                        n2230 = Unbundle(w3648) -> ("amps"=w3647:dbl, "volts"=w3646:dbl, "pf"=w3645:dbl)
                        n2231 = case shown="True" w3649 {
                          tunnel: w3656 -> [_ w3688]
                          tunnel: w3655 -> [_ w3695]
                          tunnel: w3654 -> [_ _]
                          tunnel: w3653 -> [_ _]
                          tunnel: w3652 -> [_ w3694]
                          tunnel: w3651 -> [_ w3693]
                          tunnel: w3650 -> [_ w3658]
                          tunnel: w3647 -> [_ w3690]
                          tunnel: w3646 -> [_ w3689]
                          tunnel: w3645 -> [_ w3687]
                          tunnel: w3644 -> [_ w3679]
                          frame False {
                          }
                          frame True {
                            n2232 = local read "TDMS LAB05-2"() -> (w3692:refnum<k34>)
                            n2233 = Build Array(w3689) -> (w3684:dbl[])
                            n2234 = Build Array(w3687) -> (w3683:dbl[])
                            n2235 = Build Array(w3694) -> (w3682:dbl[])
                            n2236 = Build Array(w3695) -> (w3681:dbl[])
                            n2237 = Build Array(w3690) -> (w3686:dbl[])
                            n2238 = Build Array(w3688) -> (w3685:dbl[])
                            n2239 = Build Array(w3693) -> (w3680:dbl[])
                            n2240 = Build Array("AMPS ON", "AMPS OFF", "VOLTS", "PF", "TEMP Live", "TEMP Neut", "CYCLE") -> (w3663:string[])
                            n2241 = Bundle By Name("Y"=w3686, "t0"=w3679) -> (w3678:waveform(dbl))  [unwired: 1 in]
                            n2242 = Bundle By Name("Y"=w3685, "t0"=w3679) -> (w3677:waveform(dbl))  [unwired: 1 in]
                            n2243 = Bundle By Name("Y"=w3684, "t0"=w3679) -> (w3676:waveform(dbl))  [unwired: 1 in]
                            n2244 = Bundle By Name("Y"=w3683, "t0"=w3679) -> (w3675:waveform(dbl))  [unwired: 1 in]
                            n2245 = Bundle By Name("Y"=w3682, "t0"=w3679) -> (w3674:waveform(dbl))  [unwired: 1 in]
                            n2246 = Bundle By Name("Y"=w3681, "t0"=w3679) -> (w3673:waveform(dbl))  [unwired: 1 in]
                            n2247 = Bundle By Name("Y"=w3680, "t0"=w3679) -> (w3672:waveform(dbl))  [unwired: 1 in]
                            n2248 = Build Array(w3678, w3677, w3676, w3675, w3674, w3673, w3672) -> (w3671:waveform(dbl)[])
                            n2249 = TDMS Write(0:w3692, 5:"TEST VALUES", 7:w3663, 9:w3671) -> (4:w3662:refnum<k34>, 6:w3661:string, 15:w3660:errorcluster)  [unwired: 2 in, 1 out]
                            n2250 = TDMS Write(0:w3662, 5:w3661, 7:"TIME", 9:w3658, 11:w3660) -> (15:w3657:errorcluster)  [unwired: 1 in, 3 out]
                            n2251 = local write "data file error"(w3657) -> ()
                          }
                        }
                      }
                    }
                  }
                }
              }
            }
          }
          frame #14 {
            # "display test values on chart"
            n2252 = case shown="\"OFF CYCLE\"" "Select  Cycle" {
              tunnel: [1 w3701] -> w3696
              frame "ON CYCLE", Default {
              }
              frame "OFF CYCLE" {
                n2253 = local read "on loops"() -> (w3703:dbl)
                n2254 = Add(x=w3703, y=2) -> (x+y=w3701:dbl)
              }
            }
            n2255 = local read "jig cycle"() -> (w3698:dbl)
            n2256 = Equal?(x=w3698, y=w3696) -> (x = y?=w3699:bool)
            n2257 = case shown="True" w3699 {
              frame False {
              }
              frame True {
                n2258 = local read "SIG LAB05-1"() -> (w3745:T2)
                n2259 = local read "SIG LAB04-2"() -> (w3746:T2)
                n2260 = local read "SIG LAB05-2"() -> (w3744:T2)
                n2261 = local read "SIG LAB04-1"() -> (w3747:T2)
                n2262 = local read "SIG LAB03-1"() -> (w3749:T2)
                n2263 = local read "SIG LAB03-2"() -> (w3748:T2)
                n2264 = local read "SIG LAB01-1"() -> (w3753:T2)
                n2265 = local read "SIG LAB02-2"() -> (w3750:T2)
                n2266 = local read "SIG LAB02-1"() -> (w3751:T2)
                n2267 = local read "SIG LAB01-2"() -> (w3752:T2)
                n2268 = Unbundle(w3746) -> ("AMPS"=w3736:dbl, "VOLTS"=w3726:dbl, "Tmp Live"=w3716:dbl, "Tmp Neut"=w3706:dbl)  [unwired: 1 out]
                n2269 = Unbundle(w3745) -> ("AMPS"=w3735:dbl, "VOLTS"=w3725:dbl, "Tmp Live"=w3715:dbl, "Tmp Neut"=w3705:dbl)  [unwired: 1 out]
                n2270 = Unbundle(w3744) -> ("AMPS"=w3734:dbl, "VOLTS"=w3724:dbl, "Tmp Live"=w3714:dbl, "Tmp Neut"=w3704:dbl)  [unwired: 1 out]
                n2271 = Unbundle(w3747) -> ("AMPS"=w3737:dbl, "VOLTS"=w3727:dbl, "Tmp Live"=w3717:dbl, "Tmp Neut"=w3707:dbl)  [unwired: 1 out]
                n2272 = Unbundle(w3748) -> ("AMPS"=w3738:dbl, "VOLTS"=w3728:dbl, "Tmp Live"=w3718:dbl, "Tmp Neut"=w3708:dbl)  [unwired: 1 out]
                n2273 = Unbundle(w3749) -> ("AMPS"=w3739:dbl, "VOLTS"=w3729:dbl, "Tmp Live"=w3719:dbl, "Tmp Neut"=w3709:dbl)  [unwired: 1 out]
                n2274 = Unbundle(w3750) -> ("AMPS"=w3740:dbl, "VOLTS"=w3730:dbl, "Tmp Live"=w3720:dbl, "Tmp Neut"=w3710:dbl)  [unwired: 1 out]
                n2275 = Unbundle(w3751) -> ("AMPS"=w3741:dbl, "VOLTS"=w3731:dbl, "Tmp Live"=w3721:dbl, "Tmp Neut"=w3711:dbl)  [unwired: 1 out]
                n2276 = Unbundle(w3753) -> ("AMPS"=w3743:dbl, "VOLTS"=w3733:dbl, "Tmp Live"=w3723:dbl, "Tmp Neut"=w3713:dbl)  [unwired: 1 out]
                n2277 = Unbundle(w3752) -> ("AMPS"=w3742:dbl, "VOLTS"=w3732:dbl, "Tmp Live"=w3722:dbl, "Tmp Neut"=w3712:dbl)  [unwired: 1 out]
                n2278 = stacked-sequence {
                  tunnel: w3743 -> [w3764 _ _ _]
                  tunnel: w3742 -> [w3763 _ _ _]
                  tunnel: w3741 -> [w3762 _ _ _]
                  tunnel: w3740 -> [w3761 _ _ _]
                  tunnel: w3739 -> [w3760 _ _ _]
                  tunnel: w3738 -> [w3759 _ _ _]
                  tunnel: w3737 -> [w3758 _ _ _]
                  tunnel: w3736 -> [w3757 _ _ _]
                  tunnel: w3735 -> [w3756 _ _ _]
                  tunnel: w3734 -> [w3755 _ _ _]
                  tunnel: w3733 -> [_ w3775 _ _]
                  tunnel: w3732 -> [_ w3774 _ _]
                  tunnel: w3731 -> [_ w3773 _ _]
                  tunnel: w3730 -> [_ w3772 _ _]
                  tunnel: w3729 -> [_ w3771 _ _]
                  tunnel: w3728 -> [_ w3770 _ _]
                  tunnel: w3727 -> [_ w3769 _ _]
                  tunnel: w3726 -> [_ w3768 _ _]
                  tunnel: w3725 -> [_ w3767 _ _]
                  tunnel: w3724 -> [_ w3766 _ _]
                  tunnel: w3723 -> [_ _ w3786 _]
                  tunnel: w3722 -> [_ _ w3785 _]
                  tunnel: w3721 -> [_ _ w3784 _]
                  tunnel: w3720 -> [_ _ w3783 _]
                  tunnel: w3719 -> [_ _ w3782 _]
                  tunnel: w3718 -> [_ _ w3781 _]
                  tunnel: w3717 -> [_ _ w3780 _]
                  tunnel: w3716 -> [_ _ w3779 _]
                  tunnel: w3715 -> [_ _ w3778 _]
                  tunnel: w3714 -> [_ _ w3777 _]
                  tunnel: w3713 -> [_ _ _ w3797]
                  tunnel: w3712 -> [_ _ _ w3796]
                  tunnel: w3711 -> [_ _ _ w3795]
                  tunnel: w3710 -> [_ _ _ w3794]
                  tunnel: w3709 -> [_ _ _ w3793]
                  tunnel: w3708 -> [_ _ _ w3792]
                  tunnel: w3707 -> [_ _ _ w3791]
                  tunnel: w3706 -> [_ _ _ w3790]
                  tunnel: w3705 -> [_ _ _ w3789]
                  tunnel: w3704 -> [_ _ _ w3788]
                  frame #0 {
                    n2279 = Bundle("AMPS"=w3764, "AMPS"=w3763, "AMPS"=w3762, "AMPS"=w3761, "AMPS"=w3760, "AMPS"=w3759, "AMPS"=w3758, "AMPS"=w3757, "AMPS"=w3756, "AMPS"=w3755) -> (→"TEST AMPS CHART":T6)  [unwired: 1 in]
                  }
                  frame #1 {
                    n2280 = Bundle("VOLTS"=w3775, "VOLTS"=w3774, "VOLTS"=w3773, "VOLTS"=w3772, "VOLTS"=w3771, "VOLTS"=w3770, "VOLTS"=w3769, "VOLTS"=w3768, "VOLTS"=w3767, "VOLTS"=w3766) -> (→"TEST VOLTS CHART":T29)  [unwired: 1 in]
                  }
                  frame #2 {
                    n2281 = Bundle("Tmp Live"=w3786, "Tmp Live"=w3785, "Tmp Live"=w3784, "Tmp Live"=w3783, "Tmp Live"=w3782, "Tmp Live"=w3781, "Tmp Live"=w3780, "Tmp Live"=w3779, "Tmp Live"=w3778, "Tmp Live"=w3777) -> (→"TEMPERATURE (L) CHART":T30)  [unwired: 1 in]
                  }
                  frame #3 {
                    n2282 = Bundle("Tmp Neut"=w3797, "Tmp Neut"=w3796, "Tmp Neut"=w3795, "Tmp Neut"=w3794, "Tmp Neut"=w3793, "Tmp Neut"=w3792, "Tmp Neut"=w3791, "Tmp Neut"=w3790, "Tmp Neut"=w3789, "Tmp Neut"=w3788) -> (→"TEMPERATURE (N) CHART":T31)  [unwired: 1 in]
                  }
                }
              }
            }
          }
          frame #15 {
            # "check for amps fail"
            # "check for cycle test & temperature rise fail conditions"
            n2283 = local read "on loops"() -> (w3823:dbl)
            n2284 = local read "jig cycle"() -> (w3820:dbl)
            n2285 = local read "jig cycle"() -> (w3825:dbl)
            n2286 = Add(x=w3823, y=3.0) -> (x+y=w3821:dbl)
            n2287 = Equal?(x=w3820, y=w3821) -> (x = y?=w3816:bool)
            n2288 = Equal?(x=w3825, y=1.0) -> (x = y?=w3818:bool)
            n2289 = stacked-sequence {
              tunnel: w3819 -> [w3828 _ _ _ _ _ _ _ _ _]
              tunnel: w3818 -> [w3829 w3849 w3869 w3889 w3909 w3929 w3949 w3969 w3989 w4009]
              tunnel: w3817 -> [w3826 _ _ _ _ _ _ _ _ _]
              tunnel: w3816 -> [w3827 w3848 w3868 w3888 w3908 w3928 w3948 w3968 w3988 w4008]
              tunnel: w3815 -> [_ w3847 _ _ _ _ _ _ _ _]
              tunnel: w3814 -> [_ w3846 _ _ _ _ _ _ _ _]
              tunnel: w3813 -> [_ _ w3867 _ _ _ _ _ _ _]
              tunnel: w3812 -> [_ _ w3866 _ _ _ _ _ _ _]
              tunnel: w3811 -> [_ _ _ w3887 _ _ _ _ _ _]
              tunnel: w3810 -> [_ _ _ w3886 _ _ _ _ _ _]
              tunnel: w3809 -> [_ _ _ _ w3907 _ _ _ _ _]
              tunnel: w3808 -> [_ _ _ _ w3906 _ _ _ _ _]
              tunnel: w3807 -> [_ _ _ _ _ w3927 _ _ _ _]
              tunnel: w3806 -> [_ _ _ _ _ w3926 _ _ _ _]
              tunnel: w3805 -> [_ _ _ _ _ _ w3947 _ _ _]
              tunnel: w3804 -> [_ _ _ _ _ _ w3946 _ _ _]
              tunnel: w3803 -> [_ _ _ _ _ _ _ w3967 _ _]
              tunnel: w3802 -> [_ _ _ _ _ _ _ w3966 _ _]
              tunnel: w3801 -> [_ _ _ _ _ _ _ _ w3987 _]
              tunnel: w3800 -> [_ _ _ _ _ _ _ _ w3986 _]
              tunnel: w3799 -> [_ _ _ _ _ _ _ _ _ w4007]
              tunnel: w3798 -> [_ _ _ _ _ _ _ _ _ w4006]
              frame #0 {
                # "LAB01-1"
                n2290 = case shown="True" w3826 {
                  tunnel: w3829 -> [_ w3842]
                  tunnel: w3828 -> [_ w3839]
                  tunnel: w3827 -> [_ w3838]
                  frame False {
                  }
                  frame True {
                    n2291 = local read "TEMP START LAB01-1"() -> (w3844:cluster{"TL":dbl, "TN":dbl})
                    n2292 = local read "RESULT LAB01-1"() -> (w3833:bool)
                    n2293 = local read "FAIL LAB01-1"() -> (w3836:cluster{"LO":dbl, "HI":dbl})
                    n2294 = local read "TDMS LAB01-1"() -> (w3843:refnum<k34>)
                    n2295 = local read "SET LAB01-1"() -> (w3840:T5)
                    n2296 = local read "DISP LAB01-1"() -> (w3841:T4)
                    n2297 = local read "SIG LAB01-1"() -> (w3845:T2)
                    n2298 = Bundle("FAIL LAB01-1"=w3836, "SIG LAB01-1"=w3845, "TEMP START LAB01-1"=w3844, "DISP LAB01-1"=w3841, "SET LAB01-1"=w3840, "TDMS LAB01-1"=w3843) -> (w3830:T32)  [unwired: 1 in]
                    n2299 = call "sub vi - cycle&temp fail v6.vi"("Amps Lo?"=w3842, "Input Cluster"=w3830, "SELECT"=w3839, "Amps Hi?"=w3838, "Result In"=w3833) -> ("(FAIL) out"=w3835:cluster{"FAIL LO":dbl, "FAIL HI":dbl}, "(DISP) out"=w3831:T4, "T-RISE"=w3832:cluster{"T-RISE (L)":dbl, "T-RISE (N)":dbl}, "Result Out"=w3834:bool, "file error"=w3837:errorcluster)  [unwired: 10 in]
                    n2300 = local write "TEMP RISE LAB01-1"(w3832) -> ()
                    n2301 = local write "FAIL LAB01-1"(w3835) -> ()
                    n2302 = local write "DISP LAB01-1"(w3831) -> ()
                    n2303 = local write "RESULT LAB01-1"(w3834) -> ()
                    n2304 = local write "data file error"(w3837) -> ()
                  }
                }
              }
              frame #1 {
                # "LAB01-2"
                n2305 = case shown="True" w3847 {
                  tunnel: w3849 -> [_ w3862]
                  tunnel: w3846 -> [_ w3859]
                  tunnel: w3848 -> [_ w3858]
                  frame False {
                  }
                  frame True {
                    n2306 = local read "TEMP START LAB01-2"() -> (w3864:cluster{"TL":dbl, "TN":dbl})
                    n2307 = local read "FAIL LAB01-2"() -> (w3855:cluster{"LO":dbl, "HI":dbl})
                    n2308 = local read "TDMS LAB01-2"() -> (w3863:refnum<k34>)
                    n2309 = local read "SET LAB01-2"() -> (w3860:T5)
                    n2310 = local read "DISP LAB01-2"() -> (w3861:T4)
                    n2311 = local read "RESULT LAB01-2"() -> (w3852:bool)
                    n2312 = local read "SIG LAB01-2"() -> (w3865:T2)
                    n2313 = Bundle("FAIL LAB01-2"=w3855, "SIG LAB01-2"=w3865, "TEMP START LAB01-2"=w3864, "DISP LAB01-2"=w3861, "SET LAB01-2"=w3860, "TDMS LAB01-2"=w3863) -> (w3850:T33)  [unwired: 1 in]
                    n2314 = call "sub vi - cycle&temp fail v6.vi"("Amps Lo?"=w3862, "Input Cluster"=w3850, "SELECT"=w3859, "Amps Hi?"=w3858, "Result In"=w3852) -> ("(FAIL) out"=w3854:cluster{"FAIL LO":dbl, "FAIL HI":dbl}, "(DISP) out"=w3857:T4, "T-RISE"=w3851:cluster{"T-RISE (L)":dbl, "T-RISE (N)":dbl}, "Result Out"=w3853:bool, "file error"=w3856:errorcluster)  [unwired: 10 in]
                    n2315 = local write "TEMP RISE LAB01-2"(w3851) -> ()
                    n2316 = local write "FAIL LAB01-2"(w3854) -> ()
                    n2317 = local write "DISP LAB01-2"(w3857) -> ()
                    n2318 = local write "RESULT LAB01-2"(w3853) -> ()
                    n2319 = local write "data file error"(w3856) -> ()
                  }
                }
              }
              frame #2 {
                # "LAB02-1"
                n2320 = case shown="True" w3867 {
                  tunnel: w3869 -> [_ w3882]
                  tunnel: w3866 -> [_ w3879]
                  tunnel: w3868 -> [_ w3878]
                  frame False {
                  }
                  frame True {
                    n2321 = local read "TEMP START LAB02-1"() -> (w3884:cluster{"TL":dbl, "TN":dbl})
                    n2322 = local read "FAIL LAB02-1"() -> (w3875:cluster{"LO":dbl, "HI":dbl})
                    n2323 = local read "TDMS LAB02-1"() -> (w3883:refnum<k34>)
                    n2324 = local read "SET LAB02-1"() -> (w3880:T5)
                    n2325 = local read "DISP LAB02-1"() -> (w3881:T4)
                    n2326 = local read "SIG LAB02-1"() -> (w3885:T2)
                    n2327 = local read "RESULT LAB02-1"() -> (w3872:bool)
                    n2328 = Bundle("FAIL LAB02-1"=w3875, "SIG LAB02-1"=w3885, "TEMP START LAB02-1"=w3884, "DISP LAB02-1"=w3881, "SET LAB02-1"=w3880, "TDMS LAB02-1"=w3883) -> (w3870:T34)  [unwired: 1 in]
                    n2329 = call "sub vi - cycle&temp fail v6.vi"("Amps Lo?"=w3882, "Input Cluster"=w3870, "SELECT"=w3879, "Amps Hi?"=w3878, "Result In"=w3872) -> ("(FAIL) out"=w3874:cluster{"FAIL LO":dbl, "FAIL HI":dbl}, "(DISP) out"=w3877:T4, "T-RISE"=w3871:cluster{"T-RISE (L)":dbl, "T-RISE (N)":dbl}, "Result Out"=w3873:bool, "file error"=w3876:errorcluster)  [unwired: 10 in]
                    n2330 = local write "TEMP RISE LAB02-1"(w3871) -> ()
                    n2331 = local write "FAIL LAB02-1"(w3874) -> ()
                    n2332 = local write "DISP LAB02-1"(w3877) -> ()
                    n2333 = local write "RESULT LAB02-1"(w3873) -> ()
                    n2334 = local write "data file error"(w3876) -> ()
                  }
                }
              }
              frame #3 {
                # "LAB02-2"
                n2335 = case shown="True" w3887 {
                  tunnel: w3889 -> [_ w3902]
                  tunnel: w3886 -> [_ w3899]
                  tunnel: w3888 -> [_ w3898]
                  frame False {
                  }
                  frame True {
                    n2336 = local read "TEMP START LAB02-2"() -> (w3904:cluster{"TL":dbl, "TN":dbl})
                    n2337 = local read "FAIL LAB02-2"() -> (w3895:cluster{"LO":dbl, "HI":dbl})
                    n2338 = local read "TDMS LAB02-2"() -> (w3903:refnum<k34>)
                    n2339 = local read "SET LAB02-2"() -> (w3900:T5)
                    n2340 = local read "DISP LAB02-2"() -> (w3901:T4)
                    n2341 = local read "SIG LAB02-2"() -> (w3905:T2)
                    n2342 = local read "RESULT LAB02-2"() -> (w3892:bool)
                    n2343 = Bundle("FAIL LAB02-2"=w3895, "SIG LAB02-2"=w3905, "TEMP START LAB02-2"=w3904, "DISP LAB02-2"=w3901, "SET LAB02-2"=w3900, "TDMS LAB02-2"=w3903) -> (w3890:T35)  [unwired: 1 in]
                    n2344 = call "sub vi - cycle&temp fail v6.vi"("Amps Lo?"=w3902, "Input Cluster"=w3890, "SELECT"=w3899, "Amps Hi?"=w3898, "Result In"=w3892) -> ("(FAIL) out"=w3894:cluster{"FAIL LO":dbl, "FAIL HI":dbl}, "(DISP) out"=w3897:T4, "T-RISE"=w3891:cluster{"T-RISE (L)":dbl, "T-RISE (N)":dbl}, "Result Out"=w3893:bool, "file error"=w3896:errorcluster)  [unwired: 10 in]
                    n2345 = local write "TEMP RISE LAB02-2"(w3891) -> ()
                    n2346 = local write "FAIL LAB02-2"(w3894) -> ()
                    n2347 = local write "DISP LAB02-2"(w3897) -> ()
                    n2348 = local write "RESULT LAB02-2"(w3893) -> ()
                    n2349 = local write "data file error"(w3896) -> ()
                  }
                }
              }
              frame #4 {
                # "LAB03-1"
                n2350 = case shown="True" w3907 {
                  tunnel: w3909 -> [_ w3922]
                  tunnel: w3906 -> [_ w3919]
                  tunnel: w3908 -> [_ w3918]
                  frame False {
                  }
                  frame True {
                    n2351 = local read "TEMP START LAB03-1"() -> (w3924:cluster{"TL":dbl, "TN":dbl})
                    n2352 = local read "FAIL LAB03-1"() -> (w3915:cluster{"LO":dbl, "HI":dbl})
                    n2353 = local read "TDMS LAB03-1"() -> (w3923:refnum<k34>)
                    n2354 = local read "SET LAB03-1"() -> (w3920:T5)
                    n2355 = local read "DISP LAB03-1"() -> (w3921:T4)
                    n2356 = local read "SIG LAB03-1"() -> (w3925:T2)
                    n2357 = local read "RESULT LAB03-1"() -> (w3912:bool)
                    n2358 = Bundle("FAIL LAB03-1"=w3915, "SIG LAB03-1"=w3925, "TEMP START LAB03-1"=w3924, "DISP LAB03-1"=w3921, "SET LAB03-1"=w3920, "TDMS LAB03-1"=w3923) -> (w3910:T36)  [unwired: 1 in]
                    n2359 = call "sub vi - cycle&temp fail v6.vi"("Amps Lo?"=w3922, "Input Cluster"=w3910, "SELECT"=w3919, "Amps Hi?"=w3918, "Result In"=w3912) -> ("(FAIL) out"=w3914:cluster{"FAIL LO":dbl, "FAIL HI":dbl}, "(DISP) out"=w3917:T4, "T-RISE"=w3911:cluster{"T-RISE (L)":dbl, "T-RISE (N)":dbl}, "Result Out"=w3913:bool, "file error"=w3916:errorcluster)  [unwired: 10 in]
                    n2360 = local write "TEMP RISE LAB03-1"(w3911) -> ()
                    n2361 = local write "FAIL LAB03-1"(w3914) -> ()
                    n2362 = local write "DISP LAB03-1"(w3917) -> ()
                    n2363 = local write "RESULT LAB03-1"(w3913) -> ()
                    n2364 = local write "data file error"(w3916) -> ()
                  }
                }
              }
              frame #5 {
                # "LAB03-2"
                n2365 = case shown="True" w3927 {
                  tunnel: w3929 -> [_ w3942]
                  tunnel: w3926 -> [_ w3939]
                  tunnel: w3928 -> [_ w3938]
                  frame False {
                  }
                  frame True {
                    n2366 = local read "TEMP START LAB03-2"() -> (w3944:cluster{"TL":dbl, "TN":dbl})
                    n2367 = local read "FAIL LAB03-2"() -> (w3935:cluster{"LO":dbl, "HI":dbl})
                    n2368 = local read "TDMS LAB03-2"() -> (w3943:refnum<k34>)
                    n2369 = local read "SET LAB03-2"() -> (w3940:T5)
                    n2370 = local read "DISP LAB03-2"() -> (w3941:T4)
                    n2371 = local read "RESULT LAB03-2"() -> (w3932:bool)
                    n2372 = local read "SIG LAB03-2"() -> (w3945:T2)
                    n2373 = Bundle("FAIL LAB03-2"=w3935, "SIG LAB03-2"=w3945, "TEMP START LAB03-2"=w3944, "DISP LAB03-2"=w3941, "SET LAB03-2"=w3940, "TDMS LAB03-2"=w3943) -> (w3930:T37)  [unwired: 1 in]
                    n2374 = call "sub vi - cycle&temp fail v6.vi"("Amps Lo?"=w3942, "Input Cluster"=w3930, "SELECT"=w3939, "Amps Hi?"=w3938, "Result In"=w3932) -> ("(FAIL) out"=w3934:cluster{"FAIL LO":dbl, "FAIL HI":dbl}, "(DISP) out"=w3937:T4, "T-RISE"=w3931:cluster{"T-RISE (L)":dbl, "T-RISE (N)":dbl}, "Result Out"=w3933:bool, "file error"=w3936:errorcluster)  [unwired: 10 in]
                    n2375 = local write "FAIL LAB03-2"(w3934) -> ()
                    n2376 = local write "TEMP RISE LAB03-2"(w3931) -> ()
                    n2377 = local write "DISP LAB03-2"(w3937) -> ()
                    n2378 = local write "RESULT LAB03-2"(w3933) -> ()
                    n2379 = local write "data file error"(w3936) -> ()
                  }
                }
              }
              frame #6 {
                # "LAB04-1"
                n2380 = case shown="True" w3947 {
                  tunnel: w3949 -> [_ w3962]
                  tunnel: w3946 -> [_ w3959]
                  tunnel: w3948 -> [_ w3958]
                  frame False {
                  }
                  frame True {
                    n2381 = local read "TEMP START LAB04-1"() -> (w3964:cluster{"TL":dbl, "TN":dbl})
                    n2382 = local read "FAIL LAB04-1"() -> (w3955:cluster{"LO":dbl, "HI":dbl})
                    n2383 = local read "TDMS LAB04-1"() -> (w3963:refnum<k34>)
                    n2384 = local read "SET LAB04-1"() -> (w3960:T5)
                    n2385 = local read "DISP LAB04-1"() -> (w3961:T4)
                    n2386 = local read "SIG LAB04-1"() -> (w3965:T2)
                    n2387 = local read "RESULT LAB04-1"() -> (w3952:bool)
                    n2388 = Bundle("FAIL LAB04-1"=w3955, "SIG LAB04-1"=w3965, "TEMP START LAB04-1"=w3964, "DISP LAB04-1"=w3961, "SET LAB04-1"=w3960, "TDMS LAB04-1"=w3963) -> (w3950:T38)  [unwired: 1 in]
                    n2389 = call "sub vi - cycle&temp fail v6.vi"("Amps Lo?"=w3962, "Input Cluster"=w3950, "SELECT"=w3959, "Amps Hi?"=w3958, "Result In"=w3952) -> ("(FAIL) out"=w3954:cluster{"FAIL LO":dbl, "FAIL HI":dbl}, "(DISP) out"=w3957:T4, "T-RISE"=w3951:cluster{"T-RISE (L)":dbl, "T-RISE (N)":dbl}, "Result Out"=w3953:bool, "file error"=w3956:errorcluster)  [unwired: 10 in]
                    n2390 = local write "TEMP RISE LAB04-1"(w3951) -> ()
                    n2391 = local write "FAIL LAB04-1"(w3954) -> ()
                    n2392 = local write "DISP LAB04-1"(w3957) -> ()
                    n2393 = local write "RESULT LAB04-1"(w3953) -> ()
                    n2394 = local write "data file error"(w3956) -> ()
                  }
                }
              }
              frame #7 {
                # "LAB04-2"
                n2395 = case shown="True" w3967 {
                  tunnel: w3969 -> [_ w3982]
                  tunnel: w3966 -> [_ w3979]
                  tunnel: w3968 -> [_ w3978]
                  frame False {
                  }
                  frame True {
                    n2396 = local read "TEMP START LAB04-2"() -> (w3984:cluster{"TL":dbl, "TN":dbl})
                    n2397 = local read "FAIL LAB04-2"() -> (w3975:cluster{"LO":dbl, "HI":dbl})
                    n2398 = local read "TDMS LAB04-2"() -> (w3983:refnum<k34>)
                    n2399 = local read "SET LAB04-2"() -> (w3980:T5)
                    n2400 = local read "DISP LAB04-2"() -> (w3981:T4)
                    n2401 = local read "SIG LAB04-2"() -> (w3985:T2)
                    n2402 = local read "RESULT LAB04-2"() -> (w3972:bool)
                    n2403 = Bundle("FAIL LAB04-2"=w3975, "SIG LAB04-2"=w3985, "TEMP START LAB04-2"=w3984, "DISP LAB04-2"=w3981, "SET LAB04-2"=w3980, "TDMS LAB04-2"=w3983) -> (w3970:T39)  [unwired: 1 in]
                    n2404 = call "sub vi - cycle&temp fail v6.vi"("Amps Lo?"=w3982, "Input Cluster"=w3970, "SELECT"=w3979, "Amps Hi?"=w3978, "Result In"=w3972) -> ("(FAIL) out"=w3974:cluster{"FAIL LO":dbl, "FAIL HI":dbl}, "(DISP) out"=w3977:T4, "T-RISE"=w3971:cluster{"T-RISE (L)":dbl, "T-RISE (N)":dbl}, "Result Out"=w3973:bool, "file error"=w3976:errorcluster)  [unwired: 10 in]
                    n2405 = local write "TEMP RISE LAB04-2"(w3971) -> ()
                    n2406 = local write "FAIL LAB04-2"(w3974) -> ()
                    n2407 = local write "DISP LAB04-2"(w3977) -> ()
                    n2408 = local write "RESULT LAB04-2"(w3973) -> ()
                    n2409 = local write "data file error"(w3976) -> ()
                  }
                }
              }
              frame #8 {
                # "LAB05-1"
                n2410 = case shown="True" w3987 {
                  tunnel: w3989 -> [_ w4002]
                  tunnel: w3986 -> [_ w3999]
                  tunnel: w3988 -> [_ w3998]
                  frame False {
                  }
                  frame True {
                    n2411 = local read "TEMP START LAB05-1"() -> (w4004:cluster{"TL":dbl, "TN":dbl})
                    n2412 = local read "FAIL LAB05-1"() -> (w3995:cluster{"LO":dbl, "HI":dbl})
                    n2413 = local read "TDMS LAB05-1"() -> (w4003:refnum<k34>)
                    n2414 = local read "SET LAB05-1"() -> (w4000:T5)
                    n2415 = local read "DISP LAB05-1"() -> (w4001:T4)
                    n2416 = local read "SIG LAB05-1"() -> (w4005:T2)
                    n2417 = local read "RESULT LAB05-1"() -> (w3992:bool)
                    n2418 = Bundle("FAIL LAB05-1"=w3995, "SIG LAB05-1"=w4005, "TEMP START LAB05-1"=w4004, "DISP LAB05-1"=w4001, "SET LAB05-1"=w4000, "TDMS LAB05-1"=w4003) -> (w3990:T40)  [unwired: 1 in]
                    n2419 = call "sub vi - cycle&temp fail v6.vi"("Amps Lo?"=w4002, "Input Cluster"=w3990, "SELECT"=w3999, "Amps Hi?"=w3998, "Result In"=w3992) -> ("(FAIL) out"=w3994:cluster{"FAIL LO":dbl, "FAIL HI":dbl}, "(DISP) out"=w3997:T4, "T-RISE"=w3991:cluster{"T-RISE (L)":dbl, "T-RISE (N)":dbl}, "Result Out"=w3993:bool, "file error"=w3996:errorcluster)  [unwired: 10 in]
                    n2420 = local write "TEMP RISE LAB05-1"(w3991) -> ()
                    n2421 = local write "FAIL LAB05-1"(w3994) -> ()
                    n2422 = local write "DISP LAB05-1"(w3997) -> ()
                    n2423 = local write "RESULT LAB05-1"(w3993) -> ()
                    n2424 = local write "data file error"(w3996) -> ()
                  }
                }
              }
              frame #9 {
                # "LAB05-2"
                n2425 = case shown="True" w4007 {
                  tunnel: w4009 -> [_ w4022]
                  tunnel: w4006 -> [_ w4019]
                  tunnel: w4008 -> [_ w4018]
                  frame False {
                  }
                  frame True {
                    n2426 = local read "TEMP START LAB05-2"() -> (w4024:cluster{"TL":dbl, "TN":dbl})
                    n2427 = local read "FAIL LAB05-2"() -> (w4015:cluster{"LO":dbl, "HI":dbl})
                    n2428 = local read "TDMS LAB05-2"() -> (w4023:refnum<k34>)
                    n2429 = local read "SET LAB05-2"() -> (w4020:T5)
                    n2430 = local read "DISP LAB05-2"() -> (w4021:T4)
                    n2431 = local read "SIG LAB05-2"() -> (w4025:T2)
                    n2432 = local read "RESULT LAB05-2"() -> (w4012:bool)
                    n2433 = Bundle("FAIL LAB05-2"=w4015, "SIG LAB05-2"=w4025, "TEMP START LAB05-2"=w4024, "DISP LAB05-2"=w4021, "SET LAB05-2"=w4020, "TDMS LAB05-2"=w4023) -> (w4010:T41)  [unwired: 1 in]
                    n2434 = call "sub vi - cycle&temp fail v6.vi"("Amps Lo?"=w4022, "Input Cluster"=w4010, "SELECT"=w4019, "Amps Hi?"=w4018, "Result In"=w4012) -> ("(FAIL) out"=w4014:cluster{"FAIL LO":dbl, "FAIL HI":dbl}, "(DISP) out"=w4017:T4, "T-RISE"=w4011:cluster{"T-RISE (L)":dbl, "T-RISE (N)":dbl}, "Result Out"=w4013:bool, "file error"=w4016:errorcluster)  [unwired: 10 in]
                    n2435 = local write "TEMP RISE LAB05-2"(w4011) -> ()
                    n2436 = local write "FAIL LAB05-2"(w4014) -> ()
                    n2437 = local write "DISP LAB05-2"(w4017) -> ()
                    n2438 = local write "RESULT LAB05-2"(w4013) -> ()
                    n2439 = local write "data file error"(w4016) -> ()
                  }
                }
              }
            }
          }
          frame #16 {
            # "run calibration routine"
            n2440 = local read "CALIBRATE"() -> (w4026:bool)
            n2441 = case shown="True" w4026 {
              frame False {
              }
              frame True {
                n2442 = stacked-sequence {
                  seq-local: [w4027 _ _] -> [_ w4029 _]
                  frame #0 {
                    n2443 = call "CALIBRATION PASSWORD"() -> ("PASSWORD"=w4027:string)  [unwired: 17 in, 2 out]
                  }
                  frame #1 {
                    n2444 = Equal?(x=w4029, y="7777") -> (x = y?=w4028:bool)
                    n2445 = case shown="True" w4028 {
                      frame False {
                      }
                      frame True {
                        n2446 = stacked-sequence {
                          frame #0 {
                            n2447 = call "sub vi - calibration v1.vi"() -> ()  [unwired: 12 in]
                          }
                          frame #1 {
                            n2448 = call "sub vi - get calibration values v1.vi"() -> ("LAB01 (CAL)"=w4035:T8, "LAB02 (CAL)"=w4034:T9, "LAB03 (CAL)"=w4033:T8, "LAB04 (CAL)"=w4032:T8, "calibration file error out"=w4036:errorcluster, "LAB05 (CAL)"=w4031:T8)  [unwired: 10 in]
                            n2449 = local write "calibration file error out"(w4036) -> ()
                            n2450 = local write "CAL LAB04"(w4032) -> ()
                            n2451 = local write "CAL LAB05"(w4031) -> ()
                            n2452 = local write "CAL LAB01"(w4035) -> ()
                            n2453 = local write "CAL LAB02"(w4034) -> ()
                            n2454 = local write "CAL LAB03"(w4033) -> ()
                          }
                        }
                      }
                    }
                  }
                  frame #2 {
                    n2455 = local write "CALIBRATE"(FALSE) -> ()
                  }
                }
              }
            }
          }
          frame #17 {
            # "save certain settings to file"
            n2456 = String To Path(string="c:\\crabtree\\Set Up\\") -> (path=w4039:path)
            n2457 = Build Path(base path=w4039, name or relative path="settings.bin") -> (appended path=w4041:path)
            n2458 = Build Path(base path=w4039, name or relative path="mail.bin") -> (appended path=w4038:path)
            n2459 = Create Folder(path (use dialog)=w4039) -> (error out=w4044:errorcluster)  [unwired: 2 in, 2 out]
            n2460 = call <vilib>:"Clear Errors.vi"("error in (no error)"=w4044) -> ()  [unwired: 6 in, 1 out]
            n2461 = stacked-sequence {
              seq-local: [w4051 _] -> [_ w4064]
              tunnel: w4041 -> [_ w4065]
              tunnel: w4038 -> [_ w4063]
              frame #0 {
                n2462 = local read "C drive data root dir"() -> (w4050:path)
                n2463 = local read "Select COM port"() -> (w4047:refnum<visa-resource-name>)
                n2464 = local read "Network Directory"() -> (w4056:path)
                n2465 = local read "SET LAB05-2"() -> (w4055:T5)
                n2466 = local read "SET LAB05-1"() -> (w4054:T5)
                n2467 = local read "SET LAB04-2"() -> (w4053:T5)
                n2468 = local read "SET LAB03-2"() -> (w4057:T5)
                n2469 = local read "SET LAB04-1"() -> (w4052:T5)
                n2470 = local read "SET LAB03-1"() -> (w4058:T5)
                n2471 = local read "SET LAB02-2"() -> (w4059:T5)
                n2472 = local read "SET LAB02-1"() -> (w4060:T5)
                n2473 = local read "Temp Delay Lps"() -> (w4046:dbl)
                n2474 = local read "SET LAB01-2"() -> (w4061:T5)
                n2475 = local read "SET LAB01-1"() -> (w4062:T5)
                n2476 = local read "Temp Value"() -> (w4045:dbl)
                n2477 = local read "RATE (Hz)"() -> (w4049:dbl)
                n2478 = local read "SAMPLES"() -> (w4048:dbl)
                n2479 = Bundle("SET LAB01-1"=w4062, "SET LAB01-2"=w4061, "SET LAB02-1"=w4060, "SET LAB02-2"=w4059, "SET LAB03-1"=w4058, "SET LAB03-2"=w4057, "SET LAB04-1"=w4052, "SET LAB04-2"=w4053, "SET LAB05-1"=w4054, "SET LAB05-2"=w4055, "Network Directory"=w4056, "C drive data root dir"=w4050, "RATE (Hz)"=w4049, "SAMPLES"=w4048, "Select COM port"=w4047, "Temp Delay Lps"=w4046, "Temp Value"=w4045) -> (w4051:T20)  [unwired: 1 in]
              }
              frame #1 {
                n2480 = event shown="[1] \"SET LAB01-1\", \"SET LAB01-2\", \"SET LAB02-1\", \"SET LAB02-2\", \"SET LAB03-1\", \"SET LAB03-2\", \"SET LAB04-1\", \"SET LAB04-2\", \"SET LAB05-1\", \"SET LAB05-2\", \"Network Directory\", \"C drive data root dir\", \"RATE (Hz)\", \"SAMPLES\", \"Select COM port\", \"Temp Delay Lps\", \"Temp Value\": Value Change" {
                  selector: _ -> [_ _ _]
                  dyn-events: _ -> [_ _ _]
                  timeout: 10.0 -> [_ _ _]
                  tunnel: w4065 -> [_ w4067 _]
                  tunnel: w4064 -> [_ w4068 _]
                  tunnel: w4063 -> [_ _ w4079]
                  event Timeout {
                    n2481 = event-data() -> ()  [unwired: 1 in, 3 out]
                  }
                  event "SET LAB01-1", "SET LAB01-2", "SET LAB02-1", "SET LAB02-2", "SET LAB03-1", "SET LAB03-2", "SET LAB04-1", "SET LAB04-2", "SET LAB05-1", "SET LAB05-2", "Network Directory", "C drive data root dir", "RATE (Hz)", "SAMPLES", "Select COM port", "Temp Delay Lps", "Temp Value": Value Change {
                    n2482 = event-data() -> ()  [unwired: 1 in, 6 out]
                    n2483 = Open/Create/Replace File(file path (use dialog)=w4067, operation (0:open)=T19."replace or create") -> (refnum out=w4073:refnum<file>, error out=w4072:errorcluster)  [unwired: 4 in, 1 out]
                    n2484 = Write to Binary File(file (use dialog)=w4073, data=w4068, error in=w4072) -> (refnum out=w4071:refnum<file>, error out=w4070:errorcluster)  [unwired: 3 in, 1 out]
                    n2485 = Close File(refnum=w4071, error in=w4070) -> (error out=w4069:errorcluster)  [unwired: 1 out]
                    n2486 = local write "data file error"(w4069) -> ()
                  }
                  event "MAIL SETTINGS.OUT SERVER ADDRESS", "MAIL SETTINGS.FROM ACCOUNT", "MAIL SETTINGS.USER NAME", "MAIL SETTINGS.PASSWORD", "Auto Mail Send", "TO (string):": Value Change {
                    n2487 = event-data() -> ()  [unwired: 1 in, 6 out]
                    n2488 = local read "MAIL SETTINGS"() -> (w4078:T7)
                    n2489 = local read "Auto Mail Send"() -> (w4076:bool)
                    n2490 = local read "TO (string):"() -> (w4075:string)
                    n2491 = Open/Create/Replace File(file path (use dialog)=w4079, operation (0:open)=T19."replace or create") -> (refnum out=w4084:refnum<file>, error out=w4083:errorcluster)  [unwired: 4 in, 1 out]
                    n2492 = Bundle("MAIL SETTINGS"=w4078, "Auto Mail Send"=w4076, "TO (string):"=w4075) -> (w4077:T42)  [unwired: 1 in]
                    n2493 = Write to Binary File(file (use dialog)=w4084, data=w4077, error in=w4083) -> (refnum out=w4082:refnum<file>, error out=w4081:errorcluster)  [unwired: 3 in, 1 out]
                    n2494 = Close File(refnum=w4082, error in=w4081) -> (error out=w4080:errorcluster)  [unwired: 1 out]
                    n2495 = local write "data file error"(w4080) -> ()
                  }
                }
              }
            }
          }
          frame #18 {
            # "mail control"
            n2496 = local read "MAIL SETTINGS"() -> (w4101:T7)
            n2497 = local read "Auto Mail Send"() -> (w4087:bool)
            n2498 = Unbundle(w4101) -> ("OUT SERVER ADDRESS"=w4100:string, "FROM ACCOUNT"=w4099:string, "TEST MAIL"=w4098:bool)  [unwired: 4 out]
            n2499 = stacked-sequence {
              tunnel: "TO (string):" -> [_ w4140]
              tunnel: w4101 -> [w4106 w4139]
              tunnel: w4100 -> [w4105 w4138]
              tunnel: w4099 -> [w4104 w4137]
              tunnel: w4098 -> [w4103 _]
              tunnel: w4087 -> [_ w4136]
              tunnel: w4097 -> [_ w4135]
              tunnel: w4096 -> [_ w4134]
              tunnel: w4095 -> [_ w4133]
              tunnel: w4094 -> [_ w4132]
              tunnel: w4093 -> [_ w4131]
              tunnel: w4092 -> [_ w4130]
              tunnel: w4091 -> [_ w4129]
              tunnel: w4090 -> [_ w4128]
              tunnel: w4089 -> [_ w4127]
              tunnel: w4088 -> [_ w4126]
              tunnel: "TO (string):" -> [w4102 _]
              frame #0 {
                # "mail test"
                n2500 = case shown="True" w4103 {
                  tunnel: w4106 -> [_ w4110]
                  tunnel: w4102 -> [_ w4109]
                  tunnel: w4105 -> [_ w4108]
                  tunnel: w4104 -> [_ w4107]
                  frame False {
                  }
                  frame True {
                    n2501 = stacked-sequence {
                      seq-local: [_ _ w4120 _] -> [_ _ _ w4121]
                      tunnel: w4110 -> [w4113 _ _ w4125]
                      tunnel: w4109 -> [_ _ w4118 _]
                      tunnel: w4108 -> [_ _ w4116 _]
                      tunnel: w4107 -> [_ _ w4117 _]
                      frame #0 {
                        n2502 = Bundle(cluster=w4113, "TEST MAIL STATUS"="TEST START") -> (w4111:T7)  [unwired: 6 in]
                        n2503 = local write "MAIL SETTINGS"(w4111) -> ()
                      }
                      frame #1 {
                        n2504 = Wait (ms)(milliseconds to wait=500) -> ()  [unwired: 1 out]
                      }
                      frame #2 {
                        n2505 = call "sub vi - send mail with attach v5.vi"("TO:"=w4118, "subject"="MAIL TEST FROM LAB PANEL", "from"=w4117, "out going server"=w4116, "message"="TEST MESSAGE") -> ("error out"=w4120:errorcluster)  [unwired: 10 in]
                      }
                      frame #3 {
                        n2506 = Bundle(cluster=w4125, "TEST MAIL"=FALSE, "TEST MAIL STATUS"="TEST END", "mail error"=w4121) -> (w4123:T7)  [unwired: 4 in]
                        n2507 = local write "MAIL SETTINGS"(w4123) -> ()
                      }
                    }
                  }
                }
              }
              frame #1 {
                # "mail report"
                n2508 = stacked-sequence {
                  seq-local: [_ w4205 _ _] -> [_ _ _ w4373]
                  seq-local: [_ _ w4286 _] -> [_ _ _ w4363]
                  seq-local: [w4150 _ _ _] -> [_ w4199 _ _]
                  seq-local: [w4149 _ _ _] -> [_ w4198 _ _]
                  seq-local: [w4147 _ _ _] -> [_ w4196 _ _]
                  seq-local: [w4148 _ _ _] -> [_ w4197 _ _]
                  seq-local: [w4146 _ _ _] -> [_ w4195 _ _]
                  seq-local: [w4145 _ _ _] -> [_ w4190 _ _]
                  seq-local: [w4144 _ _ _] -> [_ w4191 _ _]
                  seq-local: [w4143 _ _ _] -> [_ w4192 _ _]
                  seq-local: [w4142 _ _ _] -> [_ w4193 _ _]
                  seq-local: [w4141 _ _ _] -> [_ w4194 _ _]
                  tunnel: w4140 -> [_ _ _ w4374]
                  tunnel: w4139 -> [_ _ _ w4357]
                  tunnel: w4138 -> [_ _ _ w4371]
                  tunnel: w4137 -> [_ _ _ w4370]
                  tunnel: w4136 -> [w4181 _ _ w4365]
                  tunnel: w4135 -> [_ _ w4316 _]
                  tunnel: w4134 -> [_ _ w4313 _]
                  tunnel: w4133 -> [_ _ w4312 _]
                  tunnel: w4132 -> [_ _ w4311 _]
                  tunnel: w4131 -> [_ _ w4310 _]
                  tunnel: w4130 -> [_ _ w4309 _]
                  tunnel: w4129 -> [_ _ w4308 _]
                  tunnel: w4128 -> [_ _ w4307 _]
                  tunnel: w4127 -> [_ _ w4306 _]
                  tunnel: w4126 -> [_ _ w4305 _]
                  frame #0 {
                    n2509 = case shown="False" w4181 {
                      frame False {
                        n2510 = local write "mail control"("") -> ()
                      }
                      frame True {
                      }
                    }
                    n2511 = local read "SET LAB01-1"() -> (w4180:T5)
                    n2512 = local read "SET LAB01-2"() -> (w4179:T5)
                    n2513 = local read "SET LAB02-1"() -> (w4178:T5)
                    n2514 = local read "SET LAB02-2"() -> (w4177:T5)
                    n2515 = local read "SET LAB03-1"() -> (w4176:T5)
                    n2516 = local read "SET LAB04-1"() -> (w4174:T5)
                    n2517 = local read "SET LAB05-1"() -> (w4172:T5)
                    n2518 = local read "SET LAB03-2"() -> (w4175:T5)
                    n2519 = local read "SET LAB04-2"() -> (w4173:T5)
                    n2520 = local read "SET LAB05-2"() -> (w4171:T5)
                    n2521 = Unbundle(w4176) -> ("DESCRIPTION"=w4156:string)  [unwired: 4 out]
                    n2522 = Unbundle(w4175) -> ("DESCRIPTION"=w4155:string)  [unwired: 4 out]
                    n2523 = Unbundle(w4174) -> ("DESCRIPTION"=w4154:string)  [unwired: 4 out]
                    n2524 = Unbundle(w4171) -> ("DESCRIPTION"=w4151:string)  [unwired: 4 out]
                    n2525 = Unbundle(w4177) -> ("DESCRIPTION"=w4157:string)  [unwired: 4 out]
                    n2526 = Unbundle(w4173) -> ("DESCRIPTION"=w4153:string)  [unwired: 4 out]
                    n2527 = Unbundle(w4180) -> ("DESCRIPTION"=w4169:string)  [unwired: 4 out]
                    n2528 = Unbundle(w4178) -> ("DESCRIPTION"=w4158:string)  [unwired: 4 out]
                    n2529 = Unbundle(w4172) -> ("DESCRIPTION"=w4152:string)  [unwired: 4 out]
                    n2530 = Unbundle(w4179) -> ("DESCRIPTION"=w4159:string)  [unwired: 4 out]
                    n2531 = Concatenate Strings("[LAB05-1/", w4151) -> (w4141:string)
                    n2532 = Concatenate Strings("[LAB05-2/", w4152) -> (w4142:string)
                    n2533 = Concatenate Strings("[LAB04-2/", w4153) -> (w4143:string)
                    n2534 = Concatenate Strings("[LAB03-2/", w4155) -> (w4145:string)
                    n2535 = Concatenate Strings("[LAB04-1/", w4154) -> (w4144:string)
                    n2536 = Concatenate Strings("[LAB03-1/", w4156) -> (w4146:string)
                    n2537 = Concatenate Strings("[LAB01-2/", w4159) -> (w4149:string)
                    n2538 = Concatenate Strings("[LAB02-2/", w4157) -> (w4147:string)
                    n2539 = Concatenate Strings("[LAB01-1/", w4169) -> (w4150:string)
                    n2540 = Concatenate Strings("[LAB02-1/", w4158) -> (w4148:string)
                  }
                  frame #1 {
                    w4203 = "/"
                    w4204 = 2.0
                    n2541 = local read "DISP LAB01-2"() -> (w4284:T4)
                    n2542 = local read "DISP LAB01-1"() -> (w4285:T4)
                    n2543 = local read "DISP LAB02-1"() -> (w4283:T4)
                    n2544 = local read "DISP LAB03-2"() -> (w4280:T4)
                    n2545 = local read "DISP LAB02-2"() -> (w4282:T4)
                    n2546 = local read "DISP LAB03-1"() -> (w4281:T4)
                    n2547 = local read "DISP LAB04-2"() -> (w4278:T4)
                    n2548 = local read "DISP LAB04-1"() -> (w4279:T4)
                    n2549 = local read "DISP LAB05-1"() -> (w4277:T4)
                    n2550 = local read "DISP LAB05-2"() -> (w4276:T4)
                    n2551 = Unbundle(w4284) -> ("CYCLE"=w4268:dbl, "MINS"=w4267:dbl, "STATUS"=w4264:string)
                    n2552 = Unbundle(w4285) -> ("CYCLE"=w4273:dbl, "MINS"=w4272:dbl, "STATUS"=w4269:string)
                    n2553 = Unbundle(w4283) -> ("CYCLE"=w4261:dbl, "MINS"=w4260:dbl, "STATUS"=w4259:string)
                    n2554 = Unbundle(w4280) -> ("CYCLE"=w4248:dbl, "MINS"=w4247:dbl, "STATUS"=w4244:string)
                    n2555 = Unbundle(w4281) -> ("CYCLE"=w4253:dbl, "MINS"=w4252:dbl, "STATUS"=w4249:string)
                    n2556 = Unbundle(w4282) -> ("CYCLE"=w4258:dbl, "MINS"=w4257:dbl, "STATUS"=w4254:string)
                    n2557 = Unbundle(w4279) -> ("CYCLE"=w4243:dbl, "MINS"=w4242:dbl, "STATUS"=w4239:string)
                    n2558 = Unbundle(w4278) -> ("CYCLE"=w4238:dbl, "MINS"=w4237:dbl, "STATUS"=w4234:string)
                    n2559 = Unbundle(w4277) -> ("CYCLE"=w4233:dbl, "MINS"=w4232:dbl, "STATUS"=w4229:string)
                    n2560 = Unbundle(w4276) -> ("CYCLE"=w4275:dbl, "MINS"=w4274:dbl, "STATUS"=w4226:string)
                    n2561 = Number To Decimal String(number=w4261) -> (decimal integer string=w4263:string)  [unwired: 1 in]
                    n2562 = Number To Decimal String(number=w4258) -> (decimal integer string=w4256:string)  [unwired: 1 in]
                    n2563 = Number To Decimal String(number=w4253) -> (decimal integer string=w4251:string)  [unwired: 1 in]
                    n2564 = Number To Decimal String(number=w4268) -> (decimal integer string=w4266:string)  [unwired: 1 in]
                    n2565 = Number To Decimal String(number=w4248) -> (decimal integer string=w4246:string)  [unwired: 1 in]
                    n2566 = Number To Decimal String(number=w4273) -> (decimal integer string=w4271:string)  [unwired: 1 in]
                    n2567 = Number To Decimal String(number=w4275) -> (decimal integer string=w4228:string)  [unwired: 1 in]
                    n2568 = Number To Decimal String(number=w4243) -> (decimal integer string=w4241:string)  [unwired: 1 in]
                    n2569 = Number To Decimal String(number=w4238) -> (decimal integer string=w4236:string)  [unwired: 1 in]
                    n2570 = Number To Decimal String(number=w4233) -> (decimal integer string=w4231:string)  [unwired: 1 in]
                    n2571 = Number To Fractional String(number=w4260, precision (6)=w4204) -> (F-format string=w4262:string)  [unwired: 2 in]
                    n2572 = Number To Fractional String(number=w4247, precision (6)=w4204) -> (F-format string=w4245:string)  [unwired: 2 in]
                    n2573 = Number To Fractional String(number=w4257, precision (6)=w4204) -> (F-format string=w4255:string)  [unwired: 2 in]
                    n2574 = Number To Fractional String(number=w4252, precision (6)=w4204) -> (F-format string=w4250:string)  [unwired: 2 in]
                    n2575 = Number To Fractional String(number=w4237, precision (6)=w4204) -> (F-format string=w4235:string)  [unwired: 2 in]
                    n2576 = Number To Fractional String(number=w4242, precision (6)=w4204) -> (F-format string=w4240:string)  [unwired: 2 in]
                    n2577 = Number To Fractional String(number=w4267, precision (6)=w4204) -> (F-format string=w4265:string)  [unwired: 2 in]
                    n2578 = Number To Fractional String(number=w4232, precision (6)=w4204) -> (F-format string=w4230:string)  [unwired: 2 in]
                    n2579 = Number To Fractional String(number=w4272, precision (6)=w4204) -> (F-format string=w4270:string)  [unwired: 2 in]
                    n2580 = Number To Fractional String(number=w4274, precision (6)=w4204) -> (F-format string=w4227:string)  [unwired: 2 in]
                    n2581 = Concatenate Strings(w4203, w4246, w4203, w4245, w4203, w4244) -> (w4220:string)
                    n2582 = Concatenate Strings(w4203, w4241, w4203, w4240, w4203, w4239) -> (w4219:string)
                    n2583 = Concatenate Strings(w4203, w4236, w4203, w4235, w4203, w4234) -> (w4218:string)
                    n2584 = Concatenate Strings(w4203, w4231, w4203, w4230, w4203, w4229) -> (w4217:string)
                    n2585 = Concatenate Strings(w4203, w4228, w4203, w4227, w4203, w4226) -> (w4216:string)
                    n2586 = Concatenate Strings(w4203, w4271, w4203, w4270, w4203, w4269) -> (w4225:string)
                    n2587 = Concatenate Strings(w4203, w4251, w4203, w4250, w4203, w4249) -> (w4221:string)
                    n2588 = Concatenate Strings(w4203, w4266, w4203, w4265, w4203, w4264) -> (w4224:string)
                    n2589 = Concatenate Strings(w4203, w4263, w4203, w4262, w4203, w4259) -> (w4223:string)
                    n2590 = Concatenate Strings(w4203, w4256, w4203, w4255, w4203, w4254) -> (w4222:string)
                    n2591 = Concatenate Strings("]", "\r") -> (w4200:string)
                    n2592 = Concatenate Strings(w4195, w4221, w4200) -> (w4211:string)
                    n2593 = Concatenate Strings(w4197, w4223, w4200) -> (w4213:string)
                    n2594 = Concatenate Strings(w4196, w4222, w4200) -> (w4212:string)
                    n2595 = Concatenate Strings(w4192, w4218, w4200) -> (w4208:string)
                    n2596 = Concatenate Strings(w4193, w4217, w4200) -> (w4209:string)
                    n2597 = Concatenate Strings(w4191, w4219, w4200) -> (w4207:string)
                    n2598 = Concatenate Strings(w4190, w4220, w4200) -> (w4206:string)
                    n2599 = Concatenate Strings(w4194, w4216, w4200) -> (w4210:string)
                    n2600 = Concatenate Strings(w4198, w4224, w4200) -> (w4214:string)
                    n2601 = Concatenate Strings(w4199, w4225, w4200) -> (w4215:string)
                    n2602 = Concatenate Strings(w4215, w4214, w4213, w4212, w4211, w4206, w4207, w4208, w4209, w4210) -> (w4183:string)
                    n2603 = Concatenate Strings("[PANEL/", "DESC/", "CYCLES/", "MINS/", "STATUS]", "\r", w4183) -> (w4205:string)
                    "MAIL REPORT" <- w4205
                  }
                  frame #2 {
                    w4314 = "END"
                    n2604 = local read "mail control"() -> (w4315:string)
                    n2605 = case shown="False" w4310 {
                      tunnel: w4315 -> [w4339 _]
                      tunnel: w4314 -> [w4338 _]
                      tunnel: [w4337 FALSE] -> w4300
                      frame False {
                        n2606 = Equal?(x=w4339, y=w4338) -> (x = y?=w4337:bool)
                      }
                      frame True {
                      }
                    }
                    n2607 = case shown="False" w4316 {
                      tunnel: w4315 -> [w4355 _]
                      tunnel: w4314 -> [w4354 _]
                      tunnel: [w4353 FALSE] -> w4304
                      frame False {
                        n2608 = Equal?(x=w4355, y=w4354) -> (x = y?=w4353:bool)
                      }
                      frame True {
                      }
                    }
                    n2609 = case shown="False" w4313 {
                      tunnel: w4315 -> [w4351 _]
                      tunnel: w4314 -> [w4350 _]
                      tunnel: [w4349 FALSE] -> w4303
                      frame False {
                        n2610 = Equal?(x=w4351, y=w4350) -> (x = y?=w4349:bool)
                      }
                      frame True {
                      }
                    }
                    n2611 = case shown="False" w4311 {
                      tunnel: w4315 -> [w4343 _]
                      tunnel: w4314 -> [w4342 _]
                      tunnel: [w4341 FALSE] -> w4301
                      frame False {
                        n2612 = Equal?(x=w4343, y=w4342) -> (x = y?=w4341:bool)
                      }
                      frame True {
                      }
                    }
                    n2613 = case shown="False" w4312 {
                      tunnel: w4315 -> [w4347 _]
                      tunnel: w4314 -> [w4346 _]
                      tunnel: [w4345 FALSE] -> w4302
                      frame False {
                        n2614 = Equal?(x=w4347, y=w4346) -> (x = y?=w4345:bool)
                      }
                      frame True {
                      }
                    }
                    n2615 = Or(x=w4302, y=w4301) -> (x .or. y?=w4293:bool)
                    n2616 = Or(x=w4304, y=w4303) -> (x .or. y?=w4294:bool)
                    n2617 = Or(x=w4294, y=w4293) -> (x .or. y?=w4289:bool)
                    n2618 = case shown="False" w4306 {
                      tunnel: w4315 -> [w4323 _]
                      tunnel: w4314 -> [w4322 _]
                      tunnel: [w4321 FALSE] -> w4295
                      frame False {
                        n2619 = Equal?(x=w4323, y=w4322) -> (x = y?=w4321:bool)
                      }
                      frame True {
                      }
                    }
                    n2620 = case shown="False" w4305 {
                      tunnel: w4315 -> [w4319 _]
                      tunnel: w4314 -> [w4318 _]
                      tunnel: [w4317 FALSE] -> w4299
                      frame False {
                        n2621 = Equal?(x=w4319, y=w4318) -> (x = y?=w4317:bool)
                      }
                      frame True {
                      }
                    }
                    n2622 = case shown="False" w4307 {
                      tunnel: w4315 -> [w4327 _]
                      tunnel: w4314 -> [w4326 _]
                      tunnel: [w4325 FALSE] -> w4296
                      frame False {
                        n2623 = Equal?(x=w4327, y=w4326) -> (x = y?=w4325:bool)
                      }
                      frame True {
                      }
                    }
                    n2624 = case shown="False" w4309 {
                      tunnel: w4315 -> [w4335 _]
                      tunnel: w4314 -> [w4334 _]
                      tunnel: [w4333 FALSE] -> w4298
                      frame False {
                        n2625 = Equal?(x=w4335, y=w4334) -> (x = y?=w4333:bool)
                      }
                      frame True {
                      }
                    }
                    n2626 = case shown="False" w4308 {
                      tunnel: w4315 -> [w4331 _]
                      tunnel: w4314 -> [w4330 _]
                      tunnel: [w4329 FALSE] -> w4297
                      frame False {
                        n2627 = Equal?(x=w4331, y=w4330) -> (x = y?=w4329:bool)
                      }
                      frame True {
                      }
                    }
                    n2628 = Or(x=w4298, y=w4297) -> (x .or. y?=w4292:bool)
                    n2629 = Or(x=w4296, y=w4295) -> (x .or. y?=w4291:bool)
                    n2630 = Or(x=w4299, y=w4300) -> (x .or. y?=w4287:bool)
                    n2631 = Or(x=w4292, y=w4291) -> (x .or. y?=w4290:bool)
                    n2632 = Or(x=w4289, y=w4290) -> (x .or. y?=w4288:bool)
                    n2633 = Or(x=w4288, y=w4287) -> (x .or. y?=w4286:bool)
                  }
                  frame #3 {
                    n2634 = local read "on loops"() -> (w4369:dbl)
                    n2635 = local read "jig cycle"() -> (w4366:dbl)
                    n2636 = local read "Send Mail Now"() -> (w4360:bool)
                    n2637 = Add(x=w4369, y=3.0) -> (x+y=w4367:dbl)
                    n2638 = Equal?(x=w4366, y=w4367) -> (x = y?=w4361:bool)
                    n2639 = And(x=w4361, y=w4360) -> (x .and. y?=w4359:bool)
                    n2640 = And(x=w4365, y=w4361) -> (x .and. y?=w4364:bool)
                    n2641 = And(x=w4364, y=w4363) -> (x .and. y?=w4362:bool)
                    n2642 = Or(x=w4362, y=w4359) -> (x .or. y?=w4358:bool)
                    n2643 = case shown="True" w4358 {
                      tunnel: w4374 -> [_ w4380]
                      tunnel: w4373 -> [_ w4379]
                      tunnel: "Lab Panel Test Status" -> [_ w4378]
                      tunnel: w4371 -> [_ w4377]
                      tunnel: w4370 -> [_ w4376]
                      tunnel: w4357 -> [_ w4375]
                      frame False {
                      }
                      frame True {
                        n2644 = stacked-sequence {
                          tunnel: w4380 -> [w4388 _]
                          tunnel: w4379 -> [w4387 _]
                          tunnel: w4378 -> [w4386 _]
                          tunnel: w4377 -> [w4385 _]
                          tunnel: w4376 -> [w4384 _]
                          tunnel: w4375 -> [w4383 _]
                          frame #0 {
                            n2645 = call "sub vi - send mail with attach v5.vi"("TO:"=w4388, "subject"=w4386, "from"=w4384, "out going server"=w4385, "message"=w4387) -> ("error out"=w4382:errorcluster)  [unwired: 10 in]
                            n2646 = Bundle(cluster=w4383, "mail error"=w4382) -> (w4381:T7)  [unwired: 6 in]
                            n2647 = local write "MAIL SETTINGS"(w4381) -> ()
                          }
                          frame #1 {
                            n2648 = local write "mail control"("") -> ()
                            n2649 = local write "Send Mail Now"(FALSE) -> ()
                          }
                        }
                      }
                    }
                  }
                }
              }
            }
          }
        }
        n2650 = node-c288() -> ()  [unwired: 1 in, 1 out]
        "loops" <- w230
        "stop2" <- "stop"
      }
      n2651 = node-c288(w207) -> ()  [unwired: 1 out]
    }
  }
